vi "Old GUI.vi"() -> (0 "Error Out":errorcluster)   [LabVIEW 2019]
doc: "04/01/2021 Cobra Single Head GUI v1.0 \n\nModule Core. This is the main VI for a new module. This module is self contained in that it can run on it's own without any other top level VIs. Alternatively you can call this VI from a top level VI and use it as an actor. By default the front panel will open.\n\nThe module will initialize itself with a default set of values. You can use the Initialize.VI to change those settings. \n\nIf you would like to use the Rendezvous for syncronization call \"Initialize Rendezvous\". Just pass your rendezvous reference into it."
uses:
  GUI.lvlib
  <vilib>/nisyscfg/nisyscfg.lvlib
  9c9f3542-fc6c-43b1-9b30-f65ac35759b3.vi
  Private Controls/Config Data.ctl
  894b418a-eb83-4c03-97c2-0273c02a970a.vi
  Private Controls/Profile Sequence.ctl
  Private Controls/WebDAV states.ctl
  Private Controls/Messaging Actions.ctl
  <resource>/objmgr/ni.dex.rc
  Private Controls/Timer Mode.ctl
  Private Controls/Module Graphs.ctl
  Private Controls/System Graphs.ctl
  <vilib>/Analysis/NI_AALBase.lvlib
  Private Controls/Dial Gauges.ctl
  <vilib>/regexp/Match Regular Expression.xnode
  Private Controls/NSV States.ctl
  Private Controls/Gauge Graphs/Current.ctl
  Private Controls/Gauge Graphs/Superheat.ctl
  Private Controls/Gauge Graphs/Subcooling.ctl
  Private Controls/Gauge Graphs/Compression Ratio.ctl
  Private Controls/Save Log State.ctl
  f9a46cd7-08d2-4a24-acc7-4cd81866ad12.vi
  Private Controls/System Status.ctl
  4a2a642d-dd71-4e25-967e-5de2f7f56389.vi
  f258c684-4f8c-4311-ae87-074b09a61bd4.vi
  3f6ab150-a0d6-495f-8518-fb864465b894.vi
  <vilib>/Analysis/baseanly.llb/Mean (DBL).vi
  Private Controls/Event.ctl
  <vilib>/WebDAVClient/NI_WebDAV.lvlib
  Private Controls/NS New Data.ctl
  <vilib>/NI/STM/SubVIs/MetaDataElement.ctl
  <vilib>/NI/STM/NI STM.lvlib
  <vilib>/NI/STM/TCP/TCP Connection Info.ctl
  Private Controls/Network Data Down_set back.ctl
  Private Controls/Module Status.ctl
  Private Controls/M2 Status.ctl
  Private Controls/Dataset.ctl
  Private Controls/GUI Variables.ctl
panel:
  in  "Only Installable Systems (F)":bool
  in  "Detect Online Systems (T)":bool=TRUE
  out "M1 AC Load V":dbl
  in  "Include Cached Results (all)":u32(ring) caption="Include Cached Results" items=["none"=0, "only if online"=1, "all"=3]
  in  "Device Class":string
  in  "Session in (localhost)":refnum<k21>="localhost"
  in  "IP Override":bool
  out "AI (V)":dbl[](array[numeric])=[150.19890135042343, 151.86605864041528, 0.9899910143543054, 0.13460744672906727, 0.0, 0.0, 0.0, 0.0, 0.0, 0.0, 5.0, 5.0, 1625.0, 0.0, 0.0, 0.0, 0.0, 0.0, 0.0, 0.0, 0.0, 0.0, 0.0, 0.0, 0.0, 0.0, 0.0, 0.0, 0.0]
  in  "Manual IP":string
  out "Stack light states":T1(ring) caption="Stack Light States"
  in  "error in":errorcluster
  in  "Email Test":bool
  out "Feedback 2":u8(ring)=1 caption="PV Feedback" items=["Evap Temp", "Case Temp", "Intec Temp", "TSD  Temp", "Autotune", "Extra"]
  in  "Refresh Button":bool
  out "Network Connection":bool=TRUE
  in  "Menu Ring":u16(ring)=2 items=["192.168.1.10 (NI-sbRIO-9651-01e6940c)", "192.168.1.10 (NI-sbRIO-9651-01e69419)", "192.168.1.201 (Small-Conduit)", "192.168.1.57 (QC-Test)", "192.168.2.8 (DualCobra108)", "192.168.2.95 (ATE-220V-AIN)"]
  out "Compressor":bool
  out "Force(lbf)":dbl=50.0 format="%4.1f"
  out "Package":string="new_chip"
  out "Case Temp":dbl=22.890625 format="%4.1f"
  out "Set Temp":dbl=24.0 format="%4.0f"
  out "data out":T2={"Condensing Pressure"=150.19890135042343, "Suction Pressure"=151.86605864041528, "Bypass steps"=0, "Operating Time"=0.0, "SubCooling"=-3.2655841445138947, "Superheat"=2.2056690828700596, "M1 Superheat"=1.7837896333833214, "M2 Superheat"=-39.78496036661667, "Autotune output"=0.0, "M1 Testing Elapsed Time"=0.0, "M2 Testing Elapsed Time"=0.0, "M1 Valve Control Mode"=0, "System Amps"=0.13460744672906727, "Compressor Run Time"=0.0, "SD card free Space"=31885.0, "Free Memory"=0.0, "M1 Pressure Feedback"=0.0, "M2 Pressure Feedback"=0.0, "Compression Ratio"=0.9899910143543054, "Serial Number"=0.0, "M1 AC Load V"=0.0, "M1 AC Load W"=0.0, "M1 DC Load W"=0.0, "M1 RH"=-26.085277267486106, "RH Threshold"=100.0}
  out "Stop NSV":bool=TRUE
  in  "Tab Control":T3(tab)=enum."Debug"
  in  "M1 Power Drive":bool=TRUE
  in  "Power On-Off":bool
  out "Play/Pause":bool
  out "AC Load":dbl(graph)
  out "M1 Channels":dbl[](array[numeric])=[24.0, 23.120361328125, 22.899678548177082, nan, 0.0] format="%4.1f"
  in  "Thermal Diode Feedback":bool
  out "Main Chart":waveform(dbl)[](graph)=[{"t0"=timestamp(3699375123.743896 s since 1904-01-01), "dt"=1.0, "Y"=[25.0, 25.0, 25.0, 25.0, 25.0, 25.0, 25.0, 25.0, 25.0, 25.0, 25.0, 25.0, 25.0, 25.0, 25.0, 25.0, 25.0, 25.0, 25.0, 25.0, 25.0, 25.0, 25.0, 25.0, 25.0, 25.0, 25.0, 25.0, 25.0, 25.0, 25.0, 25.0, 25.0, 25.0, 25.0, 25.0, 25.0, 25.0, 25.0, 25.0, 25.0, 25.0, 25.0, 25.0, 25.0, 25.0, 25.0, 25.0, 25.0, 25.0, 25.0, 25.0, 25.0, 25.0, 25.0, 25.0, 25.0, 25.0, 25.0, 25.0, 25.0, 25.0, 25.0, 25.0, 25.0, 25.0, 25.0, 25.0, 25.0, 25.0, 25.0, 25.0, 25.0, 25.0, 25.0, 25.0, 25.0, 25.0, 25.0, 25.0, 25.0, 25.0, 25.0, 25.0, 25.0, 25.0, 25.0, 25.0, 25.0, 25.0, 25.0, 25.0, 25.0, 25.0, 25.0, 25.0, 25.0, 25.0, 25.0, 25.0, 25.0, 25.0, 25.0, 25.0, 25.0, 25.0, 25.0, 25.0, 25.0, 25.0, 25.0, 25.0, 25.0, 25.0, 25.0, 25.0, 25.0, 25.0, 25.0, 25.0, 25.0, 25.0, 25.0, 25.0, 25.0, 25.0, 25.0, 25.0, 25.0, 25.0, 25.0, 25.0, 25.0, 25.0, 25.0, 25.0, 25.0, 25.0, 25.0, 25.0, 25.0, 25.0, 25.0, 24.0, 24.0, 24.0, 24.0, 24.0, 24.0, 24.0, 24.0, 24.0, 24.0, 24.0, 24.0, 24.0, 24.0, 24.0, 24.0, 24.0, 24.0, 24.0, 24.0, 24.0, 24.0, 24.0, 24.0, 24.0, 24.0, 24.0, 24.0, 24.0, 24.0, 24.0, 24.0, 24.0, 24.0, 24.0, 24.0, 24.0, 24.0, 24.0, 24.0, 24.0, 24.0, 24.0, 24.0, 24.0, 24.0, 24.0, 24.0, 24.0, 24.0, 24.0, 24.0, 24.0, 24.0, 24.0, 24.0, 24.0, 24.0, 24.0, 24.0, 24.0, 24.0, 24.0, 24.0, 24.0, 24.0, 24.0, 24.0, 24.0, 24.0, 24.0, 24.0, 24.0, 24.0, 24.0, 24.0, 24.0, 24.0, 24.0, 24.0, 24.0, 24.0, 24.0, 24.0, 24.0, 24.0, 24.0, 24.0, 24.0, 24.0, 24.0, 24.0, 24.0, 24.0, 24.0, 24.0, 24.0, 24.0, 24.0, 24.0, 24.0, 24.0, 24.0, 24.0, 24.0, 24.0, 24.0, 24.0, 24.0, 24.0, 24.0, 24.0, 24.0, 24.0, 24.0, 24.0, 24.0, 24.0, 24.0, 24.0, 24.0, 24.0, 24.0, 24.0, 24.0, 24.0, 24.0, 24.0, 24.0, 24.0, 24.0, 24.0, 24.0, 24.0, 24.0, 24.0, 24.0, 24.0, 24.0, 24.0, 24.0, 24.0, 24.0, 24.0, 24.0, 24.0, 24.0, 24.0, 24.0, 24.0, 24.0, 24.0, 24.0, 24.0, 24.0, 24.0, 24.0, 24.0, 24.0, 24.0, 24.0, 24.0, 24.0, 24.0, 24.0, 24.0, 24.0, 24.0, 24.0, 24.0, 24.0, 24.0, 24.0, 24.0, 24.0, 24.0, 24.0, 24.0, 24.0, 24.0, 24.0, 24.0, 24.0, 24.0, 24.0, 24.0, 24.0, 24.0, 24.0, 24.0, 24.0, 24.0, 24.0, 24.0, 24.0, 24.0, 24.0, 24.0, 24.0, 24.0, 24.0, 24.0, 24.0, 24.0, 24.0, 24.0, 24.0, 24.0, 24.0, 24.0, 24.0, 24.0, 24.0, 24.0, 24.0, 24.0, 24.0, 24.0, 24.0, 24.0, 24.0, 24.0, 24.0, 24.0, 24.0, 24.0, 24.0, 24.0, 24.0, 24.0, 24.0, 24.0, 24.0, 24.0, 24.0, 24.0, 24.0, 24.0, 24.0, 24.0, 24.0]}, {"t0"=timestamp(3699375123.743896 s since 1904-01-01), "dt"=1.0, "Y"=array[384 elements]}, {"t0"=timestamp(3699375123.743896 s since 1904-01-01), "dt"=1.0, "Y"=array[384 elements]}, {"t0"=timestamp(3699375123.743896 s since 1904-01-01), "dt"=1.0, "Y"=[nan, nan, nan, nan, nan, nan, nan, nan, nan, nan, nan, nan, nan, nan, nan, nan, nan, nan, nan, nan, nan, nan, nan, nan, nan, nan, nan, nan, nan, nan, nan, nan, nan, nan, nan, nan, nan, nan, nan, nan, nan, nan, nan, nan, nan, nan, nan, nan, nan, nan, nan, nan, nan, nan, nan, nan, nan, nan, nan, nan, nan, nan, nan, nan, nan, nan, nan, nan, nan, nan, nan, nan, nan, nan, nan, nan, nan, nan, nan, nan, nan, nan, nan, nan, nan, nan, nan, nan, nan, nan, nan, nan, nan, nan, nan, nan, nan, nan, nan, nan, nan, nan, nan, nan, nan, nan, nan, nan, nan, nan, nan, nan, nan, nan, nan, nan, nan, nan, nan, nan, nan, nan, nan, nan, nan, nan, nan, nan, nan, nan, nan, nan, nan, nan, nan, nan, nan, nan, nan, nan, nan, nan, nan, nan, nan, nan, nan, nan, nan, nan, nan, nan, nan, nan, nan, nan, nan, nan, nan, nan, nan, nan, nan, nan, nan, nan, nan, nan, nan, nan, nan, nan, nan, nan, nan, nan, nan, nan, nan, nan, nan, nan, nan, nan, nan, nan, nan, nan, nan, nan, nan, nan, nan, nan, nan, nan, nan, nan, nan, nan, nan, nan, nan, nan, nan, nan, nan, nan, nan, nan, nan, nan, nan, nan, nan, nan, nan, nan, nan, nan, nan, nan, nan, nan, nan, nan, nan, nan, nan, nan, nan, nan, nan, nan, nan, nan, nan, nan, nan, nan, nan, nan, nan, nan, nan, nan, nan, nan, nan, nan, nan, nan, nan, nan, nan, nan, nan, nan, nan, nan, nan, nan, nan, nan, nan, nan, nan, nan, nan, nan, nan, nan, nan, nan, nan, nan, nan, nan, nan, nan, nan, nan, nan, nan, nan, nan, nan, nan, nan, nan, nan, nan, nan, nan, nan, nan, nan, nan, nan, nan, nan, nan, nan, nan, nan, nan, nan, nan, nan, nan, nan, nan, nan, nan, nan, nan, nan, nan, nan, nan, nan, nan, nan, nan, nan, nan, nan, nan, nan, nan, nan, nan, nan, nan, nan, nan, nan, nan, nan, nan, nan, nan, nan, nan, nan, nan, nan, nan, nan, nan, nan, nan, nan, nan, nan, nan, nan, nan, nan, nan, nan, nan, nan, nan, nan, nan, nan, nan, nan, nan, nan, nan, nan, nan, nan, nan, nan, nan, nan, nan, nan, nan, nan, nan]}, {"t0"=timestamp(3699375123.743896 s since 1904-01-01), "dt"=1.0, "Y"=[0.0, 0.0, 0.0, 0.0, 0.0, 0.0, 0.0, 0.0, 0.0, 0.0, 0.0, 0.0, 0.0, 0.0, 0.0, 0.0, 0.0, 0.0, 0.0, 0.0, 0.0, 0.0, 0.0, 0.0, 0.0, 0.0, 0.0, 0.0, 0.0, 0.0, 0.0, 0.0, 0.0, 0.0, 0.0, 0.0, 0.0, 0.0, 0.0, 0.0, 0.0, 0.0, 0.0, 0.0, 0.0, 0.0, 0.0, 0.0, 0.0, 0.0, 0.0, 0.0, 0.0, 0.0, 0.0, 0.0, 0.0, 0.0, 0.0, 0.0, 0.0, 0.0, 0.0, 0.0, 0.0, 0.0, 0.0, 0.0, 0.0, 0.0, 0.0, 0.0, 0.0, 0.0, 0.0, 0.0, 0.0, 0.0, 0.0, 0.0, 0.0, 0.0, 0.0, 0.0, 0.0, 0.0, 0.0, 0.0, 0.0, 0.0, 0.0, 0.0, 0.0, 0.0, 0.0, 0.0, 0.0, 0.0, 0.0, 0.0, 0.0, 0.0, 0.0, 0.0, 0.0, 0.0, 0.0, 0.0, 0.0, 0.0, 0.0, 0.0, 0.0, 0.0, 0.0, 0.0, 0.0, 0.0, 0.0, 0.0, 0.0, 0.0, 0.0, 0.0, 0.0, 0.0, 0.0, 0.0, 0.0, 0.0, 0.0, 0.0, 0.0, 0.0, 0.0, 0.0, 0.0, 0.0, 0.0, 0.0, 0.0, 0.0, 0.0, 0.0, 0.0, 0.0, 0.0, 0.0, 0.0, 0.0, 0.0, 0.0, 0.0, 0.0, 0.0, 0.0, 0.0, 0.0, 0.0, 0.0, 0.0, 0.0, 0.0, 0.0, 0.0, 0.0, 0.0, 0.0, 0.0, 0.0, 0.0, 0.0, 0.0, 0.0, 0.0, 0.0, 0.0, 0.0, 0.0, 0.0, 0.0, 0.0, 0.0, 0.0, 0.0, 0.0, 0.0, 0.0, 0.0, 0.0, 0.0, 0.0, 0.0, 0.0, 0.0, 0.0, 0.0, 0.0, 0.0, 0.0, 0.0, 0.0, 0.0, 0.0, 0.0, 0.0, 0.0, 0.0, 0.0, 0.0, 0.0, 0.0, 0.0, 0.0, 0.0, 0.0, 0.0, 0.0, 0.0, 0.0, 0.0, 0.0, 0.0, 0.0, 0.0, 0.0, 0.0, 0.0, 0.0, 0.0, 0.0, 0.0, 0.0, 0.0, 0.0, 0.0, 0.0, 0.0, 0.0, 0.0, 0.0, 0.0, 0.0, 0.0, 0.0, 0.0, 0.0, 0.0, 0.0, 0.0, 0.0, 0.0, 0.0, 0.0, 0.0, 0.0, 0.0, 0.0, 0.0, 0.0, 0.0, 0.0, 0.0, 0.0, 0.0, 0.0, 0.0, 0.0, 0.0, 0.0, 0.0, 0.0, 0.0, 0.0, 0.0, 0.0, 0.0, 0.0, 0.0, 0.0, 0.0, 0.0, 0.0, 0.0, 0.0, 0.0, 0.0, 0.0, 0.0, 0.0, 0.0, 0.0, 0.0, 0.0, 0.0, 0.0, 0.0, 0.0, 0.0, 0.0, 0.0, 0.0, 0.0, 0.0, 0.0, 0.0, 0.0, 0.0, 0.0, 0.0, 0.0, 0.0, 0.0, 0.0, 0.0, 0.0, 0.0, 0.0, 0.0, 0.0, 0.0, 0.0, 0.0, 0.0, 0.0, 0.0, 0.0, 0.0, 0.0, 0.0, 0.0, 0.0, 0.0, 0.0, 0.0, 0.0, 0.0, 0.0, 0.0, 0.0, 0.0, 0.0, 0.0, 0.0, 0.0, 0.0, 0.0, 0.0, 0.0, 0.0, 0.0, 0.0, 0.0, 0.0, 0.0, 0.0, 0.0, 0.0, 0.0, 0.0, 0.0, 0.0, 0.0, 0.0, 0.0, 0.0, 0.0, 0.0, 0.0, 0.0, 0.0, 0.0, 0.0, 0.0, 0.0, 0.0, 0.0, 0.0, 0.0, 0.0, 0.0, 0.0, 0.0, 0.0]}]
  out "WAITING TO REACH SAFE TEMP":bool
  out "PowerDrive":bool
  out "THERMAL HEAD  DISABLED":bool
  out "Bin String":string
  out "M1 Status":T4={"Case Temp"=22.890625, "Evap Temp"=0.0, "Heater %"=0.0, "EEV Steps"=0, "Set Temp"=24.0, "Feedback"=1, "Power Drive"=FALSE, "Piston Volts"=0.0, "Safe Temp"=FALSE, "Power"=FALSE, "Thermal State"=enum."Ramp Up", "Error"=FALSE, "In tollerance"=FALSE, "Head State"=enum."Disabled", "Piston Force"=0.0, "Package"=""} {"Piston Force" format="%#_1f"; "Feedback" items=["Evap Temp", "Case Temp"]; "Case Temp" format="%4.1f"}
  in  "M1 Commands":T5={"M1 Feedback"=1, "M1 Package"=0, "M1 Enable"=FALSE, "M1 Set Temp"=0.0} {"M1 Set Temp" min=-50.0 max=150.0 step=5.0; "M1 Package" items=["new_chip", "AI_chip", "CPU", "GPU", "300", "350", "", "", "", ""]; "M1 Feedback" items=["Evap Temp", "Case Temp", "Intec", "TSD"]}
  out "M1 Humidity":cluster{"M1 RH":dbl, "RH Threshold":dbl}(graph)
  out "Low Side RPM":dbl
  out "High Side RPM":dbl
  out "Thermal State":T6(ring)=enum."Steady State"
  out "System Graphs":T7={"Ambient Temp"=73.76562942564487, "Suction Temp"=73.93437944352627, "Condensor Temp"=74.25781697779894, "Discharge Temp"=75.15781707316637, "Bypass Steps"=72.0}
  out "M1 Temp Graphs":T8={"Case Temp"=22.890625, "Evap Temp"=23.1640625, "Heater Power (%)"=0.0, "EEV Steps"=3.0, "M1 AC Load(W)"=nan} caption="Temp Graphs"
  out "Gauges":T9={"Condensing Pressure(psi)"=150.28798352025635, "Compression Ratio"=0.9904730236494418, "Subcool"=-3.12361344029253, "Superheat"=2.1933731658321847, "Current(A)"=0.13316212224759566, "Suction Pressure(psi)"=151.87493902494265} {"Suction Pressure(psi)" scale=0.0..100.0; "Current(A)" scale=5.0..15.0 scale format="%_1f"; "Superheat" scale=0.0..100.0; "Subcool" scale=-10.0..20.0 scale format="%#4.1f"; "Compression Ratio" scale=0.0..30.0 scale format="%#.0f"; "Condensing Pressure(psi)" scale=150.0..375.0}
  in  "Login":bool
  out "Serial number":dbl
  in  "Config Data Setting":bool
  in  "Packages Setting":bool
  out "Errors":string[](array[string])=["WARN:Low Amps  (21 02 20 18 55)"]
  in  "Email recipeints":string[](array[string])
  in  "Output (Hostname and IP)":u32(ring)=33 items=["Hostname"=16, "Hostname (IP)"=18, "Hostname (MAC)"=19, "IP"=32, "IP (Hostname)"=33, "IP (MAC)"=35, "MAC"=48, "MAC (Hostname)"=49, "MAC (IP)"=50]
  out "Most Recent Error":string
  out "Event log":T14(array[cluster])=[{"Name"="M1 Setpoint Change", "Time Stamp"=timestamp(3697404441.246959 s since 1904-01-01), "Code"="", "Source"="APP:Send Set Temp", "Value"=24.0, "Boolean"=FALSE, "String"="", "Error"=FALSE, "Warning"=TRUE, " Fault"=FALSE}, {"Name"="M1 Set Point", "Time Stamp"=timestamp(3697404441.212613 s since 1904-01-01), "Code"="", "Source"="GUI Event", "Value"=24.0, "Boolean"=FALSE, "String"="", "Error"=FALSE, "Warning"=FALSE, " Fault"=FALSE}, {"Name"="M1 Setpoint Change", "Time Stamp"=timestamp(3697404407.626065 s since 1904-01-01), "Code"="", "Source"="APP:Send Set Temp", "Value"=25.0, "Boolean"=FALSE, "String"="", "Error"=FALSE, "Warning"=TRUE, " Fault"=FALSE}, {"Name"="M1 Set Point", "Time Stamp"=timestamp(3697404407.582319 s since 1904-01-01), "Code"="", "Source"="GUI Event", "Value"=25.0, "Boolean"=FALSE, "String"="", "Error"=FALSE, "Warning"=FALSE, " Fault"=FALSE}, {"Name"="M1 Setpoint Change", "Time Stamp"=timestamp(3697404402.799341 s since 1904-01-01), "Code"="", "Source"="APP:Send Set Temp", "Value"=2.0, "Boolean"=FALSE, "String"="", "Error"=FALSE, "Warning"=TRUE, " Fault"=FALSE}, {"Name"="M1 Set Point", "Time Stamp"=timestamp(3697404402.767277 s since 1904-01-01), "Code"="", "Source"="GUI Event", "Value"=2.0, "Boolean"=FALSE, "String"="", "Error"=FALSE, "Warning"=FALSE, " Fault"=FALSE}, {"Name"="M1 Setpoint Change", "Time Stamp"=timestamp(3697404393.95497 s since 1904-01-01), "Code"="", "Source"="APP:Send Set Temp", "Value"=24.0, "Boolean"=FALSE, "String"="", "Error"=FALSE, "Warning"=TRUE, " Fault"=FALSE}, {"Name"="M1 Set Point", "Time Stamp"=timestamp(3697404393.921568 s since 1904-01-01), "Code"="", "Source"="GUI Event", "Value"=24.0, "Boolean"=FALSE, "String"="", "Error"=FALSE, "Warning"=FALSE, " Fault"=FALSE}, {"Name"="M1 Set Point", "Time Stamp"=timestamp(3697317947.208045 s since 1904-01-01), "Code"="", "Source"="GUI Event", "Value"=0.0, "Boolean"=FALSE, "String"="", "Error"=FALSE, "Warning"=FALSE, " Fault"=FALSE}, {"Name"="M1 Set Point", "Time Stamp"=timestamp(3697317941.377172 s since 1904-01-01), "Code"="", "Source"="GUI Event", "Value"=0.0, "Boolean"=FALSE, "String"="", "Error"=FALSE, "Warning"=FALSE, " Fault"=FALSE}, {"Name"="Bypass Target Change", "Time Stamp"=timestamp(3696722909.311575 s since 1904-01-01), "Code"="", "Source"="Bypass:Get Target", "Value"=110.0, "Boolean"=FALSE, "String"="", "Error"=FALSE, "Warning"=FALSE, " Fault"=FALSE}, {"Name"="PID Bypassed", "Time Stamp"=timestamp(3696722908.895819 s since 1904-01-01), "Code"="", "Source"="APP:Set/Send PID Bypass", "Value"=0.0, "Boolean"=FALSE, "String"="", "Error"=FALSE, "Warning"=FALSE, " Fault"=FALSE}, {"Name"="Read Saved State", "Time Stamp"=timestamp(3696722908.522525 s since 1904-01-01), "Code"="", "Source"="", "Value"=0.0, "Boolean"=FALSE, "String"="", "Error"=FALSE, "Warning"=FALSE, " Fault"=FALSE}, {"Name"="System Power", "Time Stamp"=timestamp(3696722907.909232 s since 1904-01-01), "Code"="", "Source"="GUI Event", "Value"=nan, "Boolean"=FALSE, "String"="", "Error"=FALSE, "Warning"=FALSE, " Fault"=FALSE}, {"Name"="M1 Setpoint Change", "Time Stamp"=timestamp(3696722840.115096 s since 1904-01-01), "Code"="", "Source"="APP:Send Set Temp", "Value"=25.0, "Boolean"=FALSE, "String"="", "Error"=FALSE, "Warning"=TRUE, " Fault"=FALSE}, {"Name"="M1 Set Point", "Time Stamp"=timestamp(3696722840.083527 s since 1904-01-01), "Code"="", "Source"="GUI Event", "Value"=25.0, "Boolean"=FALSE, "String"="", "Error"=FALSE, "Warning"=FALSE, " Fault"=FALSE}, {"Name"="EEV PID Output", "Time Stamp"=timestamp(3696722832.497274 s since 1904-01-01), "Code"="", "Source"="APP:Send EEV PID Out", "Value"=0.0, "Boolean"=FALSE, "String"="Value Change", "Error"=FALSE, "Warning"=FALSE, " Fault"=FALSE}, {"Name"="EEV PID Output", "Time Stamp"=timestamp(3696722545.942951 s since 1904-01-01), "Code"="", "Source"="APP:Send EEV PID Out", "Value"=20.0, "Boolean"=FALSE, "String"="Value Change", "Error"=FALSE, "Warning"=FALSE, " Fault"=FALSE}, {"Name"="EEV PID Output", "Time Stamp"=timestamp(3696722279.730517 s since 1904-01-01), "Code"="", "Source"="APP:Send EEV PID Out", "Value"=0.0, "Boolean"=FALSE, "String"="Value Change", "Error"=FALSE, "Warning"=FALSE, " Fault"=FALSE}, {"Name"="EEV PID Output", "Time Stamp"=timestamp(3696722270.596302 s since 1904-01-01), "Code"="", "Source"="APP:Send EEV PID Out", "Value"=20.0, "Boolean"=FALSE, "String"="Value Change", "Error"=FALSE, "Warning"=FALSE, " Fault"=FALSE}, {"Name"="EEV PID Output", "Time Stamp"=timestamp(3696722184.927274 s since 1904-01-01), "Code"="", "Source"="APP:Send EEV PID Out", "Value"=0.0, "Boolean"=FALSE, "String"="Value Change", "Error"=FALSE, "Warning"=FALSE, " Fault"=FALSE}, {"Name"="EEV PID Output", "Time Stamp"=timestamp(3696722168.565057 s since 1904-01-01), "Code"="", "Source"="APP:Send EEV PID Out", "Value"=20.0, "Boolean"=FALSE, "String"="Value Change", "Error"=FALSE, "Warning"=FALSE, " Fault"=FALSE}, {"Name"="M1 Setpoint Change", "Time Stamp"=timestamp(3696721334.993426 s since 1904-01-01), "Code"="", "Source"="APP:Send Set Temp", "Value"=0.0, "Boolean"=FALSE, "String"="", "Error"=FALSE, "Warning"=TRUE, " Fault"=FALSE}, {"Name"="M1 Set Point", "Time Stamp"=timestamp(3696721334.958938 s since 1904-01-01), "Code"="", "Source"="GUI Event", "Value"=0.0, "Boolean"=FALSE, "String"="", "Error"=FALSE, "Warning"=FALSE, " Fault"=FALSE}, {"Name"="", "Time Stamp"=timestamp(3696721234.772972 s since 1904-01-01), "Code"="", "Source"="MACRO:Piston Down", "Value"=0.0, "Boolean"=FALSE, "String"="", "Error"=FALSE, "Warning"=FALSE, " Fault"=FALSE}, {"Name"="M1 Power Drive", "Time Stamp"=timestamp(3696721234.729546 s since 1904-01-01), "Code"="", "Source"="GUI Event", "Value"=nan, "Boolean"=TRUE, "String"="", "Error"=FALSE, "Warning"=FALSE, " Fault"=FALSE}, {"Name"="", "Time Stamp"=timestamp(3696721230.831664 s since 1904-01-01), "Code"="", "Source"="MACRO:Piston Up", "Value"=0.0, "Boolean"=FALSE, "String"="", "Error"=FALSE, "Warning"=FALSE, " Fault"=FALSE}, {"Name"="M1 Power Drive", "Time Stamp"=timestamp(3696721230.225435 s since 1904-01-01), "Code"="", "Source"="GUI Event", "Value"=nan, "Boolean"=FALSE, "String"="", "Error"=FALSE, "Warning"=FALSE, " Fault"=FALSE}, {"Name"="", "Time Stamp"=timestamp(3696721223.856889 s since 1904-01-01), "Code"="", "Source"="MACRO:Piston Down", "Value"=0.0, "Boolean"=FALSE, "String"="", "Error"=FALSE, "Warning"=FALSE, " Fault"=FALSE}, {"Name"="M1 Power Drive", "Time Stamp"=timestamp(3696721223.821096 s since 1904-01-01), "Code"="", "Source"="GUI Event", "Value"=nan, "Boolean"=TRUE, "String"="", "Error"=FALSE, "Warning"=FALSE, " Fault"=FALSE}, {"Name"="EEV PID Output", "Time Stamp"=timestamp(3696721076.771943 s since 1904-01-01), "Code"="", "Source"="APP:Send EEV PID Out", "Value"=0.0, "Boolean"=FALSE, "String"="Value Change", "Error"=FALSE, "Warning"=FALSE, " Fault"=FALSE}, {"Name"="WARN:Low Amps", "Time Stamp"=timestamp(3696720959.402056 s since 1904-01-01), "Code"="", "Source"="", "Value"=1.0015844, "Boolean"=FALSE, "String"="", "Error"=TRUE, "Warning"=TRUE, " Fault"=FALSE}, {"Name"="Bypass Reset", "Time Stamp"=timestamp(3696720957.49231 s since 1904-01-01), "Code"="", "Source"="Bypass:Reset Bypass", "Value"=0.0, "Boolean"=FALSE, "String"="", "Error"=FALSE, "Warning"=FALSE, " Fault"=FALSE}, {"Name"="Bypass Reset", "Time Stamp"=timestamp(3696720956.315602 s since 1904-01-01), "Code"="", "Source"="Bypass:Reset Bypass", "Value"=0.0, "Boolean"=TRUE, "String"="", "Error"=FALSE, "Warning"=FALSE, " Fault"=FALSE}, {"Name"="Bypass PID Gains Change", "Time Stamp"=timestamp(3696720956.263541 s since 1904-01-01), "Code"="", "Source"="Bypass:Get Gains", "Value"=0.0, "Boolean"=FALSE, "String"="", "Error"=FALSE, "Warning"=FALSE, " Fault"=FALSE}, {"Name"="Bypass Target Change", "Time Stamp"=timestamp(3696720956.211851 s since 1904-01-01), "Code"="", "Source"="Bypass:Get Target", "Value"=3.0, "Boolean"=FALSE, "String"="", "Error"=FALSE, "Warning"=FALSE, " Fault"=FALSE}, {"Name"="Send EEV PID Target", "Time Stamp"=timestamp(3696720955.840866 s since 1904-01-01), "Code"="", "Source"="APP:Send EEV PID Target", "Value"=50.0, "Boolean"=FALSE, "String"="", "Error"=FALSE, "Warning"=FALSE, " Fault"=FALSE}, {"Name"="EEV Target Change", "Time Stamp"=timestamp(3696720955.797327 s since 1904-01-01), "Code"="", "Source"="APP:Get EEV PID Target", "Value"=50.0, "Boolean"=FALSE, "String"="", "Error"=FALSE, "Warning"=FALSE, " Fault"=FALSE}, {"Name"="EEV PID Output", "Time Stamp"=timestamp(3696720955.738594 s since 1904-01-01), "Code"="", "Source"="APP:Send EEV PID Out", "Value"=20.0, "Boolean"=FALSE, "String"="Value Change", "Error"=FALSE, "Warning"=FALSE, " Fault"=FALSE}, {"Name"="PID Bypassed", "Time Stamp"=timestamp(3696720955.567045 s since 1904-01-01), "Code"="", "Source"="APP:Set/Send PID Bypass", "Value"=0.0, "Boolean"=FALSE, "String"="", "Error"=FALSE, "Warning"=FALSE, " Fault"=FALSE}, {"Name"="Create New Datalog File", "Time Stamp"=timestamp(3696720954.995124 s since 1904-01-01), "Code"="", "Source"="", "Value"=0.0, "Boolean"=FALSE, "String"="", "Error"=FALSE, "Warning"=FALSE, " Fault"=FALSE}, {"Name"="Read Saved State", "Time Stamp"=timestamp(3696720954.777131 s since 1904-01-01), "Code"="", "Source"="", "Value"=0.0, "Boolean"=FALSE, "String"="", "Error"=FALSE, "Warning"=FALSE, " Fault"=FALSE}, {"Name"="Compressor Enable", "Time Stamp"=timestamp(3696720954.737832 s since 1904-01-01), "Code"="", "Source"="Save State", "Value"=0.0, "Boolean"=TRUE, "String"="System Settings", "Error"=FALSE, "Warning"=FALSE, " Fault"=FALSE}, {"Name"="System Power", "Time Stamp"=timestamp(3696720953.433398 s since 1904-01-01), "Code"="", "Source"="GUI Event", "Value"=nan, "Boolean"=TRUE, "String"="", "Error"=FALSE, "Warning"=FALSE, " Fault"=FALSE}, {"Name"="Bypass Target Change", "Time Stamp"=timestamp(3696720910.985179 s since 1904-01-01), "Code"="", "Source"="Bypass:Get Target", "Value"=110.0, "Boolean"=FALSE, "String"="", "Error"=FALSE, "Warning"=FALSE, " Fault"=FALSE}, {"Name"="Mains Frequency", "Time Stamp"=timestamp(3696720910.167106 s since 1904-01-01), "Code"="", "Source"="Init System Module", "Value"=221.59026785399922, "Boolean"=FALSE, "String"="", "Error"=FALSE, "Warning"=FALSE, " Fault"=FALSE}, {"Name"="Fan Amps", "Time Stamp"=timestamp(3696720910.135427 s since 1904-01-01), "Code"="", "Source"="Init System Module", "Value"=0.13293173783945855, "Boolean"=FALSE, "String"="", "Error"=FALSE, "Warning"=FALSE, " Fault"=FALSE}, {"Name"="PID Bypassed", "Time Stamp"=timestamp(3696720904.619165 s since 1904-01-01), "Code"="", "Source"="APP:Set/Send PID Bypass", "Value"=0.0, "Boolean"=FALSE, "String"="", "Error"=FALSE, "Warning"=FALSE, " Fault"=FALSE}, {"Name"="Thermal Status Change", "Time Stamp"=timestamp(3696720904.526545 s since 1904-01-01), "Code"="", "Source"="APP:Thermal Status", "Value"=0.0, "Boolean"=FALSE, "String"="", "Error"=FALSE, "Warning"=FALSE, " Fault"=FALSE}, {"Name"="M1 Setpoint Change", "Time Stamp"=timestamp(3696720904.307311 s since 1904-01-01), "Code"="", "Source"="APP:Send Set Temp", "Value"=25.0, "Boolean"=FALSE, "String"="", "Error"=FALSE, "Warning"=TRUE, " Fault"=FALSE}, {"Name"="M1 EEV Check Position", "Time Stamp"=timestamp(3696720904.25734 s since 1904-01-01), "Code"="", "Source"="", "Value"=0.0, "Boolean"=TRUE, "String"="Complete", "Error"=FALSE, "Warning"=FALSE, " Fault"=FALSE}, {"Name"="Bypass Inintialize", "Time Stamp"=timestamp(3696720903.612567 s since 1904-01-01), "Code"="", "Source"="", "Value"=4506.0, "Boolean"=FALSE, "String"="Complete", "Error"=FALSE, "Warning"=FALSE, " Fault"=FALSE}, {"Name"="Config Loaded", "Time Stamp"=timestamp(3696720894.173367 s since 1904-01-01), "Code"="", "Source"="Config Read Initialize", "Value"=0.0, "Boolean"=FALSE, "String"="", "Error"=FALSE, "Warning"=FALSE, " Fault"=FALSE}, {"Name"="Config Read", "Time Stamp"=timestamp(3696720894.13737 s since 1904-01-01), "Code"="Found", "Source"="M2 TSD", "Value"=0.0, "Boolean"=FALSE, "String"="V Offset", "Error"=FALSE, "Warning"=FALSE, " Fault"=FALSE}, {"Name"="Config Read", "Time Stamp"=timestamp(3696720894.101301 s since 1904-01-01), "Code"="Found", "Source"="M2 TSD", "Value"=0.0, "Boolean"=FALSE, "String"="Offset", "Error"=FALSE, "Warning"=FALSE, " Fault"=FALSE}, {"Name"="Config Read", "Time Stamp"=timestamp(3696720894.069511 s since 1904-01-01), "Code"="Found", "Source"="M2 TSD", "Value"=1.0, "Boolean"=FALSE, "String"="Gain", "Error"=FALSE, "Warning"=FALSE, " Fault"=FALSE}, {"Name"="Config Read", "Time Stamp"=timestamp(3696720894.035389 s since 1904-01-01), "Code"="Found", "Source"="M1 TSD", "Value"=0.0, "Boolean"=FALSE, "String"="V Offset", "Error"=FALSE, "Warning"=FALSE, " Fault"=FALSE}, {"Name"="Config Read", "Time Stamp"=timestamp(3696720894.004982 s since 1904-01-01), "Code"="Found", "Source"="M1 TSD", "Value"=0.0, "Boolean"=FALSE, "String"="Offset", "Error"=FALSE, "Warning"=FALSE, " Fault"=FALSE}, {"Name"="Config Read", "Time Stamp"=timestamp(3696720893.957789 s since 1904-01-01), "Code"="Found", "Source"="M1 TSD", "Value"=1.0, "Boolean"=FALSE, "String"="Gain", "Error"=FALSE, "Warning"=FALSE, " Fault"=FALSE}, {"Name"="M1 EEV Check Position", "Time Stamp"=timestamp(3696720893.92009 s since 1904-01-01), "Code"="", "Source"="EEV:Check Position", "Value"=0.0, "Boolean"=FALSE, "String"="", "Error"=FALSE, "Warning"=FALSE, " Fault"=FALSE}, {"Name"="Config Read", "Time Stamp"=timestamp(3696720893.889076 s since 1904-01-01), "Code"="Found", "Source"="M2 T-Case Calibration", "Value"=0.0, "Boolean"=FALSE, "String"="Offset", "Error"=FALSE, "Warning"=FALSE, " Fault"=FALSE}, {"Name"="EEV PID Output", "Time Stamp"=timestamp(3696720893.86316 s since 1904-01-01), "Code"="", "Source"="APP:Send EEV PID Out", "Value"=0.0, "Boolean"=FALSE, "String"="Value Change", "Error"=FALSE, "Warning"=FALSE, " Fault"=FALSE}, {"Name"="Config Read", "Time Stamp"=timestamp(3696720893.831275 s since 1904-01-01), "Code"="Found", "Source"="M2 T-Case Calibration", "Value"=1.0, "Boolean"=FALSE, "String"="Gain", "Error"=FALSE, "Warning"=FALSE, " Fault"=FALSE}, {"Name"="", "Time Stamp"=timestamp(3696720893.797286 s since 1904-01-01), "Code"="", "Source"="EEV:Set Position", "Value"=0.0, "Boolean"=FALSE, "String"="", "Error"=FALSE, "Warning"=FALSE, " Fault"=FALSE}, {"Name"="Config Read", "Time Stamp"=timestamp(3696720893.767191 s since 1904-01-01), "Code"="Found", "Source"="M1 T-Case Calibration", "Value"=0.0, "Boolean"=FALSE, "String"="Offset", "Error"=FALSE, "Warning"=FALSE, " Fault"=FALSE}, {"Name"="", "Time Stamp"=timestamp(3696720893.717819 s since 1904-01-01), "Code"="", "Source"="EEV:Config", "Value"=0.0, "Boolean"=FALSE, "String"="", "Error"=FALSE, "Warning"=FALSE, " Fault"=FALSE}, {"Name"="Config Read", "Time Stamp"=timestamp(3696720893.68612 s since 1904-01-01), "Code"="Found", "Source"="M1 T-Case Calibration", "Value"=1.0, "Boolean"=FALSE, "String"="Gain", "Error"=FALSE, "Warning"=FALSE, " Fault"=FALSE}, {"Name"="Config Read", "Time Stamp"=timestamp(3696720893.653343 s since 1904-01-01), "Code"="Found", "Source"="Heater PID TSD", "Value"=0.066, "Boolean"=FALSE, "String"="Derivative Value", "Error"=FALSE, "Warning"=FALSE, " Fault"=FALSE}, {"Name"="Config Read", "Time Stamp"=timestamp(3696720893.619191 s since 1904-01-01), "Code"="Found", "Source"="Heater PID TSD", "Value"=0.264, "Boolean"=FALSE, "String"="Integral Value", "Error"=FALSE, "Warning"=FALSE, " Fault"=FALSE}, {"Name"="Config Read", "Time Stamp"=timestamp(3696720893.587827 s since 1904-01-01), "Code"="Found", "Source"="Heater PID TSD", "Value"=4.207, "Boolean"=FALSE, "String"="Proportional Value", "Error"=FALSE, "Warning"=FALSE, " Fault"=FALSE}, {"Name"="Config Read", "Time Stamp"=timestamp(3696720893.561761 s since 1904-01-01), "Code"="Found", "Source"="M2 EEV PID", "Value"=0.0, "Boolean"=FALSE, "String"="Gain D", "Error"=FALSE, "Warning"=FALSE, " Fault"=FALSE}, {"Name"="Config Read", "Time Stamp"=timestamp(3696720893.533947 s since 1904-01-01), "Code"="Found", "Source"="M2 EEV PID", "Value"=0.25, "Boolean"=FALSE, "String"="Gain I", "Error"=FALSE, "Warning"=FALSE, " Fault"=FALSE}, {"Name"="Config Read", "Time Stamp"=timestamp(3696720893.499744 s since 1904-01-01), "Code"="Found", "Source"="M2 EEV PID", "Value"=-1.0, "Boolean"=FALSE, "String"="Gain P", "Error"=FALSE, "Warning"=FALSE, " Fault"=FALSE}, {"Name"="Config Read", "Time Stamp"=timestamp(3696720893.453109 s since 1904-01-01), "Code"="Found", "Source"="EEV PID", "Value"=15.0, "Boolean"=FALSE, "String"="M1 Superheat Setpoint ", "Error"=FALSE, "Warning"=FALSE, " Fault"=FALSE}, {"Name"="Config Read", "Time Stamp"=timestamp(3696720893.407586 s since 1904-01-01), "Code"="Found", "Source"="EEV PID", "Value"=0.0, "Boolean"=FALSE, "String"="Output Low", "Error"=FALSE, "Warning"=FALSE, " Fault"=FALSE}, {"Name"="Config Read", "Time Stamp"=timestamp(3696720893.375381 s since 1904-01-01), "Code"="Found", "Source"="EEV PID", "Value"=155.0, "Boolean"=FALSE, "String"="Output Hi", "Error"=FALSE, "Warning"=FALSE, " Fault"=FALSE}, {"Name"="Config Read", "Time Stamp"=timestamp(3696720893.345284 s since 1904-01-01), "Code"="Found", "Source"="EEV PID", "Value"=0.0, "Boolean"=FALSE, "String"="Gain D", "Error"=FALSE, "Warning"=FALSE, " Fault"=FALSE}, {"Name"="Config Read", "Time Stamp"=timestamp(3696720893.313855 s since 1904-01-01), "Code"="Found", "Source"="EEV PID", "Value"=0.6, "Boolean"=FALSE, "String"="Gain I", "Error"=FALSE, "Warning"=FALSE, " Fault"=FALSE}, {"Name"="Config Read", "Time Stamp"=timestamp(3696720893.282199 s since 1904-01-01), "Code"="Found", "Source"="EEV PID", "Value"=-1.0, "Boolean"=FALSE, "String"="Gain P", "Error"=FALSE, "Warning"=FALSE, " Fault"=FALSE}, {"Name"="Config Read", "Time Stamp"=timestamp(3696720893.253151 s since 1904-01-01), "Code"="Found", "Source"="EEV PID", "Value"=10.0, "Boolean"=FALSE, "String"="Dissabled Target", "Error"=FALSE, "Warning"=FALSE, " Fault"=FALSE}, {"Name"="Config Read", "Time Stamp"=timestamp(3696720893.203999 s since 1904-01-01), "Code"="Found", "Source"="EEV PID", "Value"=30.0, "Boolean"=FALSE, "String"="SS Steps", "Error"=FALSE, "Warning"=FALSE, " Fault"=FALSE}, {"Name"="Config Read", "Time Stamp"=timestamp(3696720893.175068 s since 1904-01-01), "Code"="Found", "Source"="EEV PID", "Value"=60.0, "Boolean"=FALSE, "String"="RD Steps", "Error"=FALSE, "Warning"=FALSE, " Fault"=FALSE}, {"Name"="Config Read", "Time Stamp"=timestamp(3696720893.143394 s since 1904-01-01), "Code"="Found", "Source"="EEV PID", "Value"=20.0, "Boolean"=FALSE, "String"="RU Steps", "Error"=FALSE, "Warning"=FALSE, " Fault"=FALSE}, {"Name"="Config Read", "Time Stamp"=timestamp(3696720893.112236 s since 1904-01-01), "Code"="Found", "Source"="EEV PID", "Value"=85.0, "Boolean"=FALSE, "String"="EBB Steps Closed", "Error"=FALSE, "Warning"=FALSE, " Fault"=FALSE}, {"Name"="Config Read", "Time Stamp"=timestamp(3696720893.081919 s since 1904-01-01), "Code"="Found", "Source"="EEV PID", "Value"=70.0, "Boolean"=FALSE, "String"="EBB Steps Open", "Error"=FALSE, "Warning"=FALSE, " Fault"=FALSE}, {"Name"="Config Read", "Time Stamp"=timestamp(3696720893.055853 s since 1904-01-01), "Code"="Found", "Source"="EEV PID", "Value"=2.0, "Boolean"=FALSE, "String"="EBB Tol", "Error"=FALSE, "Warning"=FALSE, " Fault"=FALSE}, {"Name"="Config Read", "Time Stamp"=timestamp(3696720893.027455 s since 1904-01-01), "Code"="Found", "Source"="EEV PID", "Value"=-60.0, "Boolean"=FALSE, "String"="EBB TH", "Error"=FALSE, "Warning"=FALSE, " Fault"=FALSE}, {"Name"="Config Read", "Time Stamp"=timestamp(3696720892.999011 s since 1904-01-01), "Code"="Found", "Source"="EEV PID", "Value"=50.0, "Boolean"=FALSE, "String"="SS Target", "Error"=FALSE, "Warning"=FALSE, " Fault"=FALSE}, {"Name"="Config Read", "Time Stamp"=timestamp(3696720892.955559 s since 1904-01-01), "Code"="Found", "Source"="EEV PID", "Value"=50.0, "Boolean"=FALSE, "String"="RD Target", "Error"=FALSE, "Warning"=FALSE, " Fault"=FALSE}, {"Name"="Config Read", "Time Stamp"=timestamp(3696720892.927444 s since 1904-01-01), "Code"="Found", "Source"="EEV PID", "Value"=50.0, "Boolean"=FALSE, "String"="RU Target", "Error"=FALSE, "Warning"=FALSE, " Fault"=FALSE}, {"Name"="Config Read", "Time Stamp"=timestamp(3696720892.898945 s since 1904-01-01), "Code"="Found", "Source"="Temp TH", "Value"=3.0, "Boolean"=FALSE, "String"="SS Tol", "Error"=FALSE, "Warning"=FALSE, " Fault"=FALSE}, {"Name"="Config Read", "Time Stamp"=timestamp(3696720892.865717 s since 1904-01-01), "Code"="Found", "Source"="Temp TH", "Value"=10.0, "Boolean"=FALSE, "String"="Ramp-SS Delta T", "Error"=FALSE, "Warning"=FALSE, " Fault"=FALSE}, {"Name"="Config Read", "Time Stamp"=timestamp(3696720892.839071 s since 1904-01-01), "Code"="Found", "Source"="Temp TH", "Value"=10.0, "Boolean"=FALSE, "String"="Ramp Delta T", "Error"=FALSE, "Warning"=FALSE, " Fault"=FALSE}, {"Name"="Config Read", "Time Stamp"=timestamp(3696720892.80532 s since 1904-01-01), "Code"="Found", "Source"="Temp TH", "Value"=75.0, "Boolean"=FALSE, "String"="Pedestal Delta T", "Error"=FALSE, "Warning"=FALSE, " Fault"=FALSE}, {"Name"="Config Read", "Time Stamp"=timestamp(3696720892.777417 s since 1904-01-01), "Code"="Found", "Source"="Set Point Range", "Value"=-50.0, "Boolean"=FALSE, "String"="Min", "Error"=FALSE, "Warning"=FALSE, " Fault"=FALSE}, {"Name"="Config Read", "Time Stamp"=timestamp(3696720892.75149 s since 1904-01-01), "Code"="Found", "Source"="Set Point Range", "Value"=150.0, "Boolean"=FALSE, "String"="Max", "Error"=FALSE, "Warning"=FALSE, " Fault"=FALSE}, {"Name"="Config Read", "Time Stamp"=timestamp(3696720892.705211 s since 1904-01-01), "Code"="Found", "Source"="CryoMode PID Gains", "Value"=0.0, "Boolean"=FALSE, "String"="Derivative Value", "Error"=FALSE, "Warning"=FALSE, " Fault"=FALSE}, {"Name"="Config Read", "Time Stamp"=timestamp(3696720892.676571 s since 1904-01-01), "Code"="Found", "Source"="CryoMode PID Gains", "Value"=0.5, "Boolean"=FALSE, "String"="Integral Value", "Error"=FALSE, "Warning"=FALSE, " Fault"=FALSE}, {"Name"="Config Read", "Time Stamp"=timestamp(3696720892.651484 s since 1904-01-01), "Code"="Found", "Source"="CryoMode PID Gains", "Value"=-1.0, "Boolean"=FALSE, "String"="Proportional Value", "Error"=FALSE, "Warning"=FALSE, " Fault"=FALSE}, {"Name"="Config Read", "Time Stamp"=timestamp(3696720892.623679 s since 1904-01-01), "Code"="Found", "Source"="M2 Heater PID", "Value"=0.0, "Boolean"=FALSE, "String"="Derivative Value", "Error"=FALSE, "Warning"=FALSE, " Fault"=FALSE}, {"Name"="Config Read", "Time Stamp"=timestamp(3696720892.593471 s since 1904-01-01), "Code"="Found", "Source"="M2 Heater PID", "Value"=0.2, "Boolean"=FALSE, "String"="Integral Value", "Error"=FALSE, "Warning"=FALSE, " Fault"=FALSE}, {"Name"="Config Read", "Time Stamp"=timestamp(3696720892.559162 s since 1904-01-01), "Code"="Found", "Source"="M2 Heater PID", "Value"=8.0, "Boolean"=FALSE, "String"="Proportional Value", "Error"=FALSE, "Warning"=FALSE, " Fault"=FALSE}, {"Name"="Config Read", "Time Stamp"=timestamp(3696720892.53134 s since 1904-01-01), "Code"="Found", "Source"="Heater PID", "Value"=0.066, "Boolean"=FALSE, "String"="Derivative Value", "Error"=FALSE, "Warning"=FALSE, " Fault"=FALSE}, {"Name"="Config Read", "Time Stamp"=timestamp(3696720892.502409 s since 1904-01-01), "Code"="Found", "Source"="Heater PID", "Value"=0.264, "Boolean"=FALSE, "String"="Integral Value", "Error"=FALSE, "Warning"=FALSE, " Fault"=FALSE}, {"Name"="Config Read", "Time Stamp"=timestamp(3696720892.465166 s since 1904-01-01), "Code"="Found", "Source"="Heater PID", "Value"=2.207, "Boolean"=FALSE, "String"="Proportional Value", "Error"=FALSE, "Warning"=FALSE, " Fault"=FALSE}, {"Name"="Config Read", "Time Stamp"=timestamp(3696720892.433118 s since 1904-01-01), "Code"="Found", "Source"="Piston Settings", "Value"=500.0, "Boolean"=FALSE, "String"="Pressure Ramp Delay (ms)", "Error"=FALSE, "Warning"=FALSE, " Fault"=FALSE}, {"Name"="Config Read", "Time Stamp"=timestamp(3696720892.393472 s since 1904-01-01), "Code"="Found", "Source"="Piston Settings", "Value"=5000.0, "Boolean"=FALSE, "String"="Delay (ms)", "Error"=FALSE, "Warning"=FALSE, " Fault"=FALSE}, {"Name"="Config Read", "Time Stamp"=timestamp(3696720892.364299 s since 1904-01-01), "Code"="Found", "Source"="Piston Settings", "Value"=51.0, "Boolean"=FALSE, "String"="Piston Diameter (mm)", "Error"=FALSE, "Warning"=FALSE, " Fault"=FALSE}, {"Name"="Config Read", "Time Stamp"=timestamp(3696720892.337039 s since 1904-01-01), "Code"="Found", "Source"="Piston Settings", "Value"=0.4, "Boolean"=FALSE, "String"="Up Force", "Error"=FALSE, "Warning"=FALSE, " Fault"=FALSE}, {"Name"="Config Read", "Time Stamp"=timestamp(3696720892.309436 s since 1904-01-01), "Code"="Found", "Source"="Piston Settings", "Value"=0.4, "Boolean"=FALSE, "String"="Transition Force", "Error"=FALSE, "Warning"=FALSE, " Fault"=FALSE}, {"Name"="Config Read", "Time Stamp"=timestamp(3696720892.282026 s since 1904-01-01), "Code"="Found", "Source"="Piston Settings", "Value"=0.1488, "Boolean"=FALSE, "String"="Forces Intercept", "Error"=FALSE, "Warning"=FALSE, " Fault"=FALSE}, {"Name"="Config Read", "Time Stamp"=timestamp(3696720892.254328 s since 1904-01-01), "Code"="Found", "Source"="Piston Settings", "Value"=0.0127, "Boolean"=FALSE, "String"="Forces Slope", "Error"=FALSE, "Warning"=FALSE, " Fault"=FALSE}, {"Name"="Config Read", "Time Stamp"=timestamp(3696720892.208177 s since 1904-01-01), "Code"="Found", "Source"="Bypass PID", "Value"=0.0, "Boolean"=FALSE, "String"="Derivative Value", "Error"=FALSE, "Warning"=FALSE, " Fault"=FALSE}, {"Name"="Config Read", "Time Stamp"=timestamp(3696720892.181363 s since 1904-01-01), "Code"="Found", "Source"="Bypass PID", "Value"=0.8, "Boolean"=FALSE, "String"="Integral Value", "Error"=FALSE, "Warning"=FALSE, " Fault"=FALSE}, {"Name"="Config Read", "Time Stamp"=timestamp(3696720892.154298 s since 1904-01-01), "Code"="Found", "Source"="Bypass PID", "Value"=1.5, "Boolean"=FALSE, "String"="Proportional Value", "Error"=FALSE, "Warning"=FALSE, " Fault"=FALSE}, {"Name"="Config Value Read", "Time Stamp"=timestamp(3696720892.12076 s since 1904-01-01), "Code"="", "Source"="", "Value"=0.0, "Boolean"=TRUE, "String"="Cascade", "Error"=FALSE, "Warning"=FALSE, " Fault"=FALSE}, {"Name"="Config Value Read", "Time Stamp"=timestamp(3696720892.098045 s since 1904-01-01), "Code"="", "Source"="", "Value"=0.0, "Boolean"=TRUE, "String"="220V", "Error"=FALSE, "Warning"=FALSE, " Fault"=FALSE}, {"Name"="M1 EEV Check Position", "Time Stamp"=timestamp(3696720892.075967 s since 1904-01-01), "Code"="", "Source"="", "Value"=0.0, "Boolean"=TRUE, "String"="Complete", "Error"=FALSE, "Warning"=FALSE, " Fault"=FALSE}, {"Name"="Config Value Read", "Time Stamp"=timestamp(3696720892.053395 s since 1904-01-01), "Code"="", "Source"="", "Value"=0.0, "Boolean"=TRUE, "String"="Shuttle", "Error"=FALSE, "Warning"=FALSE, " Fault"=FALSE}, {"Name"="Config Value Read", "Time Stamp"=timestamp(3696720892.032653 s since 1904-01-01), "Code"="", "Source"="", "Value"=0.0, "Boolean"=TRUE, "String"="Handler", "Error"=FALSE, "Warning"=FALSE, " Fault"=FALSE}, {"Name"="Config Value Read", "Time Stamp"=timestamp(3696720892.012066 s since 1904-01-01), "Code"="", "Source"="", "Value"=0.0, "Boolean"=TRUE, "String"="Production", "Error"=FALSE, "Warning"=FALSE, " Fault"=FALSE}, {"Name"="Config Value Read", "Time Stamp"=timestamp(3696720891.98133 s since 1904-01-01), "Code"="", "Source"="", "Value"=0.0, "Boolean"=TRUE, "String"="Benchtop", "Error"=FALSE, "Warning"=FALSE, " Fault"=FALSE}, {"Name"="Config Value Read", "Time Stamp"=timestamp(3696720891.933658 s since 1904-01-01), "Code"="", "Source"="", "Value"=0.0, "Boolean"=TRUE, "String"="ATE", "Error"=FALSE, "Warning"=FALSE, " Fault"=FALSE}, {"Name"="Config Value Read", "Time Stamp"=timestamp(3696720891.891371 s since 1904-01-01), "Code"="", "Source"="", "Value"=0.0, "Boolean"=TRUE, "String"="HandClamp", "Error"=FALSE, "Warning"=FALSE, " Fault"=FALSE}, {"Name"="Config Value Read", "Time Stamp"=timestamp(3696720891.860102 s since 1904-01-01), "Code"="", "Source"="", "Value"=0.0, "Boolean"=TRUE, "String"="Sensors", "Error"=FALSE, "Warning"=FALSE, " Fault"=FALSE}, {"Name"="Config Value Read", "Time Stamp"=timestamp(3696720891.828709 s since 1904-01-01), "Code"="", "Source"="", "Value"=0.0, "Boolean"=TRUE, "String"="Purge", "Error"=FALSE, "Warning"=FALSE, " Fault"=FALSE}, {"Name"="Config Value Read", "Time Stamp"=timestamp(3696720891.791521 s since 1904-01-01), "Code"="", "Source"="", "Value"=0.0, "Boolean"=TRUE, "String"="Autostartup", "Error"=FALSE, "Warning"=FALSE, " Fault"=FALSE}, {"Name"="Config Value Read", "Time Stamp"=timestamp(3696720891.764417 s since 1904-01-01), "Code"="", "Source"="", "Value"=0.0, "Boolean"=TRUE, "String"="FTC200", "Error"=FALSE, "Warning"=FALSE, " Fault"=FALSE}, {"Name"="M1 EEV Check Position", "Time Stamp"=timestamp(3696720891.738071 s since 1904-01-01), "Code"="", "Source"="EEV:Check Position", "Value"=0.0, "Boolean"=FALSE, "String"="", "Error"=FALSE, "Warning"=FALSE, " Fault"=FALSE}, {"Name"="Config Value Read", "Time Stamp"=timestamp(3696720891.704925 s since 1904-01-01), "Code"="", "Source"="", "Value"=0.0, "Boolean"=TRUE, "String"="60Hz Power", "Error"=FALSE, "Warning"=FALSE, " Fault"=FALSE}, {"Name"="EEV PID Output", "Time Stamp"=timestamp(3696720891.667846 s since 1904-01-01), "Code"="", "Source"="APP:Send EEV PID Out", "Value"=2000.0, "Boolean"=FALSE, "String"="Value Change", "Error"=FALSE, "Warning"=FALSE, " Fault"=FALSE}, {"Name"="", "Time Stamp"=timestamp(3696720891.638331 s since 1904-01-01), "Code"="", "Source"="EEV:Set Position", "Value"=0.0, "Boolean"=TRUE, "String"="", "Error"=FALSE, "Warning"=FALSE, " Fault"=FALSE}, {"Name"="EEV:Set V", "Time Stamp"=timestamp(3696720891.590639 s since 1904-01-01), "Code"="", "Source"="", "Value"=0.0, "Boolean"=FALSE, "String"="", "Error"=FALSE, "Warning"=FALSE, " Fault"=FALSE}, {"Name"="New Extra Settings Loaded", "Time Stamp"=timestamp(3696720891.568061 s since 1904-01-01), "Code"="", "Source"="", "Value"=0.0, "Boolean"=FALSE, "String"="", "Error"=FALSE, "Warning"=FALSE, " Fault"=FALSE}, {"Name"="", "Time Stamp"=timestamp(3696720891.534483 s since 1904-01-01), "Code"="", "Source"="EEV:Config", "Value"=0.0, "Boolean"=FALSE, "String"="", "Error"=FALSE, "Warning"=FALSE, " Fault"=FALSE}, {"Name"="EMO Not Detected", "Time Stamp"=timestamp(3696720891.500666 s since 1904-01-01), "Code"="", "Source"="", "Value"=0.0, "Boolean"=FALSE, "String"="", "Error"=FALSE, "Warning"=FALSE, " Fault"=FALSE}, {"Name"="Read Compressor Minutes", "Time Stamp"=timestamp(3696720891.434006 s since 1904-01-01), "Code"="", "Source"="", "Value"=2930.0, "Boolean"=TRUE, "String"="PASS", "Error"=FALSE, "Warning"=FALSE, " Fault"=FALSE}, {"Name"="High Pressure Switch Detected", "Time Stamp"=timestamp(3696720891.405424 s since 1904-01-01), "Code"="", "Source"="SYS:Initialize", "Value"=0.0, "Boolean"=TRUE, "String"="", "Error"=FALSE, "Warning"=FALSE, " Fault"=FALSE}, {"Name"="Odometer Loaded", "Time Stamp"=timestamp(3696720891.303544 s since 1904-01-01), "Code"="", "Source"="", "Value"=0.0, "Boolean"=FALSE, "String"="", "Error"=FALSE, "Warning"=FALSE, " Fault"=FALSE}, {"Name"="Read Saved State", "Time Stamp"=timestamp(3696720891.269036 s since 1904-01-01), "Code"="", "Source"="", "Value"=0.0, "Boolean"=FALSE, "String"="", "Error"=FALSE, "Warning"=FALSE, " Fault"=FALSE}, {"Name"="FPGA Load Complete", "Time Stamp"=timestamp(3696720891.241224 s since 1904-01-01), "Code"="", "Source"="Init FPGA IO.vi", "Value"=0.0, "Boolean"=FALSE, "String"="", "Error"=FALSE, "Warning"=FALSE, " Fault"=FALSE}, {"Name"="Pressure Test", "Time Stamp"=timestamp(3696720889.221135 s since 1904-01-01), "Code"="", "Source"="Init FPGA IO 2.0.vi", "Value"=0.0, "Boolean"=FALSE, "String"="FAIL", "Error"=FALSE, "Warning"=TRUE, " Fault"=FALSE}, {"Name"="Stop LCD", "Time Stamp"=timestamp(3696720883.988151 s since 1904-01-01), "Code"="", "Source"="Init FPGA IO.vi", "Value"=11.0, "Boolean"=FALSE, "String"="", "Error"=FALSE, "Warning"=FALSE, " Fault"=FALSE}, {"Name"="wait", "Time Stamp"=timestamp(3696720882.969395 s since 1904-01-01), "Code"="", "Source"="Init FPGA IO.vi", "Value"=10.0, "Boolean"=FALSE, "String"="", "Error"=FALSE, "Warning"=FALSE, " Fault"=FALSE}, {"Name"="IP Address", "Time Stamp"=timestamp(3696720881.931437 s since 1904-01-01), "Code"="", "Source"="Init FPGA IO.vi", "Value"=12.0, "Boolean"=FALSE, "String"="þQ", "Error"=FALSE, "Warning"=FALSE, " Fault"=FALSE}, {"Name"="wait", "Time Stamp"=timestamp(3696720880.464476 s since 1904-01-01), "Code"="", "Source"="Init FPGA IO.vi", "Value"=10.0, "Boolean"=FALSE, "String"="", "Error"=FALSE, "Warning"=FALSE, " Fault"=FALSE}, {"Name"="Rev Display", "Time Stamp"=timestamp(3696720879.446471 s since 1904-01-01), "Code"="", "Source"="Init FPGA IO.vi", "Value"=9.0, "Boolean"=FALSE, "String"="Ver: CC 21.2.18.0", "Error"=FALSE, "Warning"=FALSE, " Fault"=FALSE}, {"Name"="wait", "Time Stamp"=timestamp(3696720879.359947 s since 1904-01-01), "Code"="", "Source"="Init FPGA IO.vi", "Value"=10.0, "Boolean"=FALSE, "String"="", "Error"=FALSE, "Warning"=FALSE, " Fault"=FALSE}, {"Name"="Chroma Display", "Time Stamp"=timestamp(3696720878.342291 s since 1904-01-01), "Code"="", "Source"="Init FPGA IO.vi", "Value"=8.0, "Boolean"=FALSE, "String"="Chroma ATE", "Error"=FALSE, "Warning"=FALSE, " Fault"=FALSE}, {"Name"="wait", "Time Stamp"=timestamp(3696720878.2478 s since 1904-01-01), "Code"="", "Source"="Init FPGA IO.vi", "Value"=10.0, "Boolean"=FALSE, "String"="", "Error"=FALSE, "Warning"=FALSE, " Fault"=FALSE}, {"Name"="Clear LCD Text", "Time Stamp"=timestamp(3696720877.219357 s since 1904-01-01), "Code"="", "Source"="Init FPGA IO.vi", "Value"=0.0, "Boolean"=FALSE, "String"="", "Error"=FALSE, "Warning"=FALSE, " Fault"=FALSE}, {"Name"="Mains Frequency", "Time Stamp"=timestamp(3696720877.149534 s since 1904-01-01), "Code"="", "Source"="Init FPGA", "Value"=194.7629520614688, "Boolean"=FALSE, "String"="", "Error"=FALSE, "Warning"=FALSE, " Fault"=FALSE}, {"Name"="Fan Amps", "Time Stamp"=timestamp(3696720877.132159 s since 1904-01-01), "Code"="", "Source"="Init FPGA", "Value"=0.10758788061792209, "Boolean"=FALSE, "String"="", "Error"=FALSE, "Warning"=FALSE, " Fault"=FALSE}, {"Name"="BootLoad", "Time Stamp"=timestamp(3696720866.1065 s since 1904-01-01), "Code"="", "Source"="Init FPGA IO.vi", "Value"=0.0, "Boolean"=FALSE, "String"="", "Error"=FALSE, "Warning"=FALSE, " Fault"=FALSE}, {"Name"="Extra Settings Loaded", "Time Stamp"=timestamp(3696720865.294767 s since 1904-01-01), "Code"="", "Source"="", "Value"=0.0, "Boolean"=FALSE, "String"="", "Error"=FALSE, "Warning"=FALSE, " Fault"=FALSE}, {"Name"="M1 Heater Specs", "Time Stamp"=timestamp(3696720865.276621 s since 1904-01-01), "Code"="", "Source"="Extra Settings", "Value"=0.0, "Boolean"=TRUE, "String"="", "Error"=FALSE, "Warning"=FALSE, " Fault"=FALSE}, {"Name"="Shuttle", "Time Stamp"=timestamp(3696720865.259777 s since 1904-01-01), "Code"="", "Source"="Extra Settings", "Value"=0.0, "Boolean"=TRUE, "String"="", "Error"=FALSE, "Warning"=FALSE, " Fault"=FALSE}, {"Name"="Housing Heater", "Time Stamp"=timestamp(3696720865.242604 s since 1904-01-01), "Code"="", "Source"="Extra Settings", "Value"=0.0, "Boolean"=TRUE, "String"="", "Error"=FALSE, "Warning"=FALSE, " Fault"=FALSE}, {"Name"="Warmup ", "Time Stamp"=timestamp(3696720865.225249 s since 1904-01-01), "Code"="", "Source"="Extra Settings", "Value"=0.0, "Boolean"=FALSE, "String"="", "Error"=FALSE, "Warning"=TRUE, " Fault"=FALSE}, {"Name"="Warmup ", "Time Stamp"=timestamp(3696720865.206102 s since 1904-01-01), "Code"="", "Source"="Extra Settings", "Value"=0.0, "Boolean"=FALSE, "String"="", "Error"=FALSE, "Warning"=TRUE, " Fault"=FALSE}, {"Name"="TSD ", "Time Stamp"=timestamp(3696720865.189469 s since 1904-01-01), "Code"="", "Source"="Extra Settings", "Value"=0.0, "Boolean"=FALSE, "String"="", "Error"=FALSE, "Warning"=FALSE, " Fault"=FALSE}, {"Name"="Flow Curve", "Time Stamp"=timestamp(3696720865.163189 s since 1904-01-01), "Code"="", "Source"="Extra Settings", "Value"=0.0, "Boolean"=FALSE, "String"="", "Error"=FALSE, "Warning"=TRUE, " Fault"=FALSE}, {"Name"="Heads Disabled", "Time Stamp"=timestamp(3696720865.145402 s since 1904-01-01), "Code"="", "Source"="Extra Settings", "Value"=0.0, "Boolean"=TRUE, "String"="", "Error"=FALSE, "Warning"=FALSE, " Fault"=FALSE}, {"Name"="Low Superheat", "Time Stamp"=timestamp(3696720865.128817 s since 1904-01-01), "Code"="", "Source"="Extra Settings", "Value"=0.0, "Boolean"=TRUE, "String"="", "Error"=FALSE, "Warning"=FALSE, " Fault"=FALSE}, {"Name"="High Superheat", "Time Stamp"=timestamp(3696720865.111942 s since 1904-01-01), "Code"="", "Source"="Extra Settings", "Value"=0.0, "Boolean"=TRUE, "String"="", "Error"=FALSE, "Warning"=FALSE, " Fault"=FALSE}, {"Name"="High Subcooling", "Time Stamp"=timestamp(3696720865.093904 s since 1904-01-01), "Code"="", "Source"="Extra Settings", "Value"=0.0, "Boolean"=TRUE, "String"="", "Error"=FALSE, "Warning"=FALSE, " Fault"=FALSE}, {"Name"="Low Subcooling", "Time Stamp"=timestamp(3696720865.077746 s since 1904-01-01), "Code"="", "Source"="Extra Settings", "Value"=0.0, "Boolean"=TRUE, "String"="", "Error"=FALSE, "Warning"=FALSE, " Fault"=FALSE}, {"Name"="Water Sensor", "Time Stamp"=timestamp(3696720865.061704 s since 1904-01-01), "Code"="", "Source"="Extra Settings", "Value"=0.0, "Boolean"=TRUE, "String"="", "Error"=FALSE, "Warning"=FALSE, " Fault"=FALSE}, {"Name"="Flow Sensor", "Time Stamp"=timestamp(3696720865.045559 s since 1904-01-01), "Code"="", "Source"="Extra Settings", "Value"=0.0, "Boolean"=TRUE, "String"="", "Error"=FALSE, "Warning"=FALSE, " Fault"=FALSE}, {"Name"="High Amperage", "Time Stamp"=timestamp(3696720865.029495 s since 1904-01-01), "Code"="", "Source"="Extra Settings", "Value"=0.0, "Boolean"=TRUE, "String"="", "Error"=FALSE, "Warning"=FALSE, " Fault"=FALSE}, {"Name"="Low Amperage", "Time Stamp"=timestamp(3696720865.013499 s since 1904-01-01), "Code"="", "Source"="Extra Settings", "Value"=0.0, "Boolean"=TRUE, "String"="", "Error"=FALSE, "Warning"=FALSE, " Fault"=FALSE}, {"Name"="Relative Humidity", "Time Stamp"=timestamp(3696720864.997521 s since 1904-01-01), "Code"="", "Source"="Extra Settings", "Value"=0.0, "Boolean"=TRUE, "String"="", "Error"=FALSE, "Warning"=FALSE, " Fault"=FALSE}, {"Name"="Warnings/Faults 1", "Time Stamp"=timestamp(3696720864.950962 s since 1904-01-01), "Code"="", "Source"="Extra Settings 3", "Value"=0.0, "Boolean"=TRUE, "String"="", "Error"=FALSE, "Warning"=FALSE, " Fault"=FALSE}, {"Name"="SuperHeat Settings", "Time Stamp"=timestamp(3696720864.933577 s since 1904-01-01), "Code"="", "Source"="Extra Settings 3", "Value"=0.0, "Boolean"=TRUE, "String"="", "Error"=FALSE, "Warning"=FALSE, " Fault"=FALSE}, {"Name"="Read System Settings", "Time Stamp"=timestamp(3696720864.914497 s since 1904-01-01), "Code"="", "Source"="Read Extra Settings", "Value"=0.0, "Boolean"=FALSE, "String"="", "Error"=FALSE, "Warning"=TRUE, " Fault"=FALSE}, {"Name"="Config Loaded", "Time Stamp"=timestamp(3696720864.86972 s since 1904-01-01), "Code"="", "Source"="Config Read Initialize", "Value"=0.0, "Boolean"=FALSE, "String"="", "Error"=FALSE, "Warning"=FALSE, " Fault"=FALSE}, {"Name"="Config Read", "Time Stamp"=timestamp(3696720864.85342 s since 1904-01-01), "Code"="Found", "Source"="M2 TSD", "Value"=0.0, "Boolean"=FALSE, "String"="V Offset", "Error"=FALSE, "Warning"=FALSE, " Fault"=FALSE}, {"Name"="Config Read", "Time Stamp"=timestamp(3696720864.837514 s since 1904-01-01), "Code"="Found", "Source"="M2 TSD", "Value"=0.0, "Boolean"=FALSE, "String"="Offset", "Error"=FALSE, "Warning"=FALSE, " Fault"=FALSE}, {"Name"="Config Read", "Time Stamp"=timestamp(3696720864.821681 s since 1904-01-01), "Code"="Found", "Source"="M2 TSD", "Value"=1.0, "Boolean"=FALSE, "String"="Gain", "Error"=FALSE, "Warning"=FALSE, " Fault"=FALSE}, {"Name"="Config Read", "Time Stamp"=timestamp(3696720864.804834 s since 1904-01-01), "Code"="Found", "Source"="M1 TSD", "Value"=0.0, "Boolean"=FALSE, "String"="V Offset", "Error"=FALSE, "Warning"=FALSE, " Fault"=FALSE}, {"Name"="Config Read", "Time Stamp"=timestamp(3696720864.789486 s since 1904-01-01), "Code"="Found", "Source"="M1 TSD", "Value"=0.0, "Boolean"=FALSE, "String"="Offset", "Error"=FALSE, "Warning"=FALSE, " Fault"=FALSE}, {"Name"="Config Read", "Time Stamp"=timestamp(3696720864.774412 s since 1904-01-01), "Code"="Found", "Source"="M1 TSD", "Value"=1.0, "Boolean"=FALSE, "String"="Gain", "Error"=FALSE, "Warning"=FALSE, " Fault"=FALSE}, {"Name"="Config Read", "Time Stamp"=timestamp(3696720864.759064 s since 1904-01-01), "Code"="Found", "Source"="M2 T-Case Calibration", "Value"=0.0, "Boolean"=FALSE, "String"="Offset", "Error"=FALSE, "Warning"=FALSE, " Fault"=FALSE}, {"Name"="Config Read", "Time Stamp"=timestamp(3696720864.74409 s since 1904-01-01), "Code"="Found", "Source"="M2 T-Case Calibration", "Value"=1.0, "Boolean"=FALSE, "String"="Gain", "Error"=FALSE, "Warning"=FALSE, " Fault"=FALSE}, {"Name"="Config Read", "Time Stamp"=timestamp(3696720864.729025 s since 1904-01-01), "Code"="Found", "Source"="M1 T-Case Calibration", "Value"=0.0, "Boolean"=FALSE, "String"="Offset", "Error"=FALSE, "Warning"=FALSE, " Fault"=FALSE}, {"Name"="Config Read", "Time Stamp"=timestamp(3696720864.714051 s since 1904-01-01), "Code"="Found", "Source"="M1 T-Case Calibration", "Value"=1.0, "Boolean"=FALSE, "String"="Gain", "Error"=FALSE, "Warning"=FALSE, " Fault"=FALSE}, {"Name"="Config Read", "Time Stamp"=timestamp(3696720864.699277 s since 1904-01-01), "Code"="Found", "Source"="Heater PID TSD", "Value"=0.066, "Boolean"=FALSE, "String"="Derivative Value", "Error"=FALSE, "Warning"=FALSE, " Fault"=FALSE}, {"Name"="Config Read", "Time Stamp"=timestamp(3696720864.683881 s since 1904-01-01), "Code"="Found", "Source"="Heater PID TSD", "Value"=0.264, "Boolean"=FALSE, "String"="Integral Value", "Error"=FALSE, "Warning"=FALSE, " Fault"=FALSE}, {"Name"="Config Read", "Time Stamp"=timestamp(3696720864.660618 s since 1904-01-01), "Code"="Found", "Source"="Heater PID TSD", "Value"=4.207, "Boolean"=FALSE, "String"="Proportional Value", "Error"=FALSE, "Warning"=FALSE, " Fault"=FALSE}, {"Name"="Config Read", "Time Stamp"=timestamp(3696720864.644996 s since 1904-01-01), "Code"="Found", "Source"="M2 EEV PID", "Value"=0.0, "Boolean"=FALSE, "String"="Gain D", "Error"=FALSE, "Warning"=FALSE, " Fault"=FALSE}, {"Name"="Config Read", "Time Stamp"=timestamp(3696720864.630353 s since 1904-01-01), "Code"="Found", "Source"="M2 EEV PID", "Value"=0.25, "Boolean"=FALSE, "String"="Gain I", "Error"=FALSE, "Warning"=FALSE, " Fault"=FALSE}, {"Name"="Config Read", "Time Stamp"=timestamp(3696720864.615385 s since 1904-01-01), "Code"="Found", "Source"="M2 EEV PID", "Value"=-1.0, "Boolean"=FALSE, "String"="Gain P", "Error"=FALSE, "Warning"=FALSE, " Fault"=FALSE}, {"Name"="Config Read", "Time Stamp"=timestamp(3696720864.600925 s since 1904-01-01), "Code"="Found", "Source"="EEV PID", "Value"=15.0, "Boolean"=FALSE, "String"="M1 Superheat Setpoint ", "Error"=FALSE, "Warning"=FALSE, " Fault"=FALSE}, {"Name"="Config Read", "Time Stamp"=timestamp(3696720864.572165 s since 1904-01-01), "Code"="Found", "Source"="EEV PID", "Value"=155.0, "Boolean"=FALSE, "String"="Output Hi", "Error"=FALSE, "Warning"=FALSE, " Fault"=FALSE}, {"Name"="Config Read", "Time Stamp"=timestamp(3696720864.557516 s since 1904-01-01), "Code"="Found", "Source"="EEV PID", "Value"=0.0, "Boolean"=FALSE, "String"="Gain D", "Error"=FALSE, "Warning"=FALSE, " Fault"=FALSE}, {"Name"="Config Read", "Time Stamp"=timestamp(3696720864.541891 s since 1904-01-01), "Code"="Found", "Source"="EEV PID", "Value"=0.6, "Boolean"=FALSE, "String"="Gain I", "Error"=FALSE, "Warning"=FALSE, " Fault"=FALSE}, {"Name"="Config Read", "Time Stamp"=timestamp(3696720864.517088 s since 1904-01-01), "Code"="Found", "Source"="EEV PID", "Value"=-1.0, "Boolean"=FALSE, "String"="Gain P", "Error"=FALSE, "Warning"=FALSE, " Fault"=FALSE}, {"Name"="Config Read", "Time Stamp"=timestamp(3696720864.502005 s since 1904-01-01), "Code"="Found", "Source"="EEV PID", "Value"=10.0, "Boolean"=FALSE, "String"="Dissabled Target", "Error"=FALSE, "Warning"=FALSE, " Fault"=FALSE}, {"Name"="Config Read", "Time Stamp"=timestamp(3696720864.486235 s since 1904-01-01), "Code"="Found", "Source"="EEV PID", "Value"=30.0, "Boolean"=FALSE, "String"="SS Steps", "Error"=FALSE, "Warning"=FALSE, " Fault"=FALSE}, {"Name"="Config Read", "Time Stamp"=timestamp(3696720864.470571 s since 1904-01-01), "Code"="Found", "Source"="EEV PID", "Value"=60.0, "Boolean"=FALSE, "String"="RD Steps", "Error"=FALSE, "Warning"=FALSE, " Fault"=FALSE}, {"Name"="Config Read", "Time Stamp"=timestamp(3696720864.454592 s since 1904-01-01), "Code"="Found", "Source"="EEV PID", "Value"=20.0, "Boolean"=FALSE, "String"="RU Steps", "Error"=FALSE, "Warning"=FALSE, " Fault"=FALSE}, {"Name"="Config Read", "Time Stamp"=timestamp(3696720864.438853 s since 1904-01-01), "Code"="Found", "Source"="EEV PID", "Value"=85.0, "Boolean"=FALSE, "String"="EBB Steps Closed", "Error"=FALSE, "Warning"=FALSE, " Fault"=FALSE}, {"Name"="Config Read", "Time Stamp"=timestamp(3696720864.423674 s since 1904-01-01), "Code"="Found", "Source"="EEV PID", "Value"=70.0, "Boolean"=FALSE, "String"="EBB Steps Open", "Error"=FALSE, "Warning"=FALSE, " Fault"=FALSE}, {"Name"="Config Read", "Time Stamp"=timestamp(3696720864.399453 s since 1904-01-01), "Code"="Found", "Source"="EEV PID", "Value"=2.0, "Boolean"=FALSE, "String"="EBB Tol", "Error"=FALSE, "Warning"=FALSE, " Fault"=FALSE}, {"Name"="Config Read", "Time Stamp"=timestamp(3696720864.379651 s since 1904-01-01), "Code"="Found", "Source"="EEV PID", "Value"=-60.0, "Boolean"=FALSE, "String"="EBB TH", "Error"=FALSE, "Warning"=FALSE, " Fault"=FALSE}, {"Name"="Config Read", "Time Stamp"=timestamp(3696720864.364313 s since 1904-01-01), "Code"="Found", "Source"="EEV PID", "Value"=50.0, "Boolean"=FALSE, "String"="SS Target", "Error"=FALSE, "Warning"=FALSE, " Fault"=FALSE}, {"Name"="Config Read", "Time Stamp"=timestamp(3696720864.339973 s since 1904-01-01), "Code"="Found", "Source"="EEV PID", "Value"=50.0, "Boolean"=FALSE, "String"="RD Target", "Error"=FALSE, "Warning"=FALSE, " Fault"=FALSE}, {"Name"="Config Read", "Time Stamp"=timestamp(3696720864.320472 s since 1904-01-01), "Code"="Found", "Source"="EEV PID", "Value"=50.0, "Boolean"=FALSE, "String"="RU Target", "Error"=FALSE, "Warning"=FALSE, " Fault"=FALSE}, {"Name"="Config Read", "Time Stamp"=timestamp(3696720864.299976 s since 1904-01-01), "Code"="Found", "Source"="Temp TH", "Value"=3.0, "Boolean"=FALSE, "String"="SS Tol", "Error"=FALSE, "Warning"=FALSE, " Fault"=FALSE}, {"Name"="Config Read", "Time Stamp"=timestamp(3696720864.274729 s since 1904-01-01), "Code"="Found", "Source"="Temp TH", "Value"=10.0, "Boolean"=FALSE, "String"="Ramp-SS Delta T", "Error"=FALSE, "Warning"=FALSE, " Fault"=FALSE}, {"Name"="Config Read", "Time Stamp"=timestamp(3696720864.259622 s since 1904-01-01), "Code"="Found", "Source"="Temp TH", "Value"=10.0, "Boolean"=FALSE, "String"="Ramp Delta T", "Error"=FALSE, "Warning"=FALSE, " Fault"=FALSE}, {"Name"="Config Read", "Time Stamp"=timestamp(3696720864.243791 s since 1904-01-01), "Code"="Found", "Source"="Temp TH", "Value"=75.0, "Boolean"=FALSE, "String"="Pedestal Delta T", "Error"=FALSE, "Warning"=FALSE, " Fault"=FALSE}, {"Name"="Config Read", "Time Stamp"=timestamp(3696720864.227674 s since 1904-01-01), "Code"="Found", "Source"="Set Point Range", "Value"=-50.0, "Boolean"=FALSE, "String"="Min", "Error"=FALSE, "Warning"=FALSE, " Fault"=FALSE}, {"Name"="Config Read", "Time Stamp"=timestamp(3696720864.211801 s since 1904-01-01), "Code"="Found", "Source"="Set Point Range", "Value"=150.0, "Boolean"=FALSE, "String"="Max", "Error"=FALSE, "Warning"=FALSE, " Fault"=FALSE}, {"Name"="Config Read", "Time Stamp"=timestamp(3696720864.196179 s since 1904-01-01), "Code"="Found", "Source"="CryoMode PID Gains", "Value"=0.0, "Boolean"=FALSE, "String"="Derivative Value", "Error"=FALSE, "Warning"=FALSE, " Fault"=FALSE}, {"Name"="Config Read", "Time Stamp"=timestamp(3696720864.161114 s since 1904-01-01), "Code"="Found", "Source"="CryoMode PID Gains", "Value"=0.5, "Boolean"=FALSE, "String"="Integral Value", "Error"=FALSE, "Warning"=FALSE, " Fault"=FALSE}, {"Name"="Config Read", "Time Stamp"=timestamp(3696720864.144419 s since 1904-01-01), "Code"="Found", "Source"="CryoMode PID Gains", "Value"=-1.0, "Boolean"=FALSE, "String"="Proportional Value", "Error"=FALSE, "Warning"=FALSE, " Fault"=FALSE}, {"Name"="Config Read", "Time Stamp"=timestamp(3696720864.115454 s since 1904-01-01), "Code"="Found", "Source"="M2 Heater PID", "Value"=0.2, "Boolean"=FALSE, "String"="Integral Value", "Error"=FALSE, "Warning"=FALSE, " Fault"=FALSE}, {"Name"="Config Read", "Time Stamp"=timestamp(3696720864.101321 s since 1904-01-01), "Code"="Found", "Source"="M2 Heater PID", "Value"=8.0, "Boolean"=FALSE, "String"="Proportional Value", "Error"=FALSE, "Warning"=FALSE, " Fault"=FALSE}, {"Name"="Config Read", "Time Stamp"=timestamp(3696720864.08568 s since 1904-01-01), "Code"="Found", "Source"="Heater PID", "Value"=0.066, "Boolean"=FALSE, "String"="Derivative Value", "Error"=FALSE, "Warning"=FALSE, " Fault"=FALSE}, {"Name"="Config Read", "Time Stamp"=timestamp(3696720864.070752 s since 1904-01-01), "Code"="Found", "Source"="Heater PID", "Value"=0.264, "Boolean"=FALSE, "String"="Integral Value", "Error"=FALSE, "Warning"=FALSE, " Fault"=FALSE}, {"Name"="Config Read", "Time Stamp"=timestamp(3696720864.053531 s since 1904-01-01), "Code"="Found", "Source"="Heater PID", "Value"=2.207, "Boolean"=FALSE, "String"="Proportional Value", "Error"=FALSE, "Warning"=FALSE, " Fault"=FALSE}, {"Name"="Config Read", "Time Stamp"=timestamp(3696720864.033635 s since 1904-01-01), "Code"="Found", "Source"="Piston Settings", "Value"=500.0, "Boolean"=FALSE, "String"="Pressure Ramp Delay (ms)", "Error"=FALSE, "Warning"=FALSE, " Fault"=FALSE}, {"Name"="Config Read", "Time Stamp"=timestamp(3696720864.018886 s since 1904-01-01), "Code"="Found", "Source"="Piston Settings", "Value"=5000.0, "Boolean"=FALSE, "String"="Delay (ms)", "Error"=FALSE, "Warning"=FALSE, " Fault"=FALSE}, {"Name"="Config Read", "Time Stamp"=timestamp(3696720864.001322 s since 1904-01-01), "Code"="Found", "Source"="Piston Settings", "Value"=51.0, "Boolean"=FALSE, "String"="Piston Diameter (mm)", "Error"=FALSE, "Warning"=FALSE, " Fault"=FALSE}, {"Name"="Config Read", "Time Stamp"=timestamp(3696720863.987963 s since 1904-01-01), "Code"="Found", "Source"="Piston Settings", "Value"=0.4, "Boolean"=FALSE, "String"="Up Force", "Error"=FALSE, "Warning"=FALSE, " Fault"=FALSE}, {"Name"="Config Read", "Time Stamp"=timestamp(3696720863.974054 s since 1904-01-01), "Code"="Found", "Source"="Piston Settings", "Value"=0.4, "Boolean"=FALSE, "String"="Transition Force", "Error"=FALSE, "Warning"=FALSE, " Fault"=FALSE}, {"Name"="Config Read", "Time Stamp"=timestamp(3696720863.960834 s since 1904-01-01), "Code"="Found", "Source"="Piston Settings", "Value"=0.1488, "Boolean"=FALSE, "String"="Forces Intercept", "Error"=FALSE, "Warning"=FALSE, " Fault"=FALSE}, {"Name"="Config Read", "Time Stamp"=timestamp(3696720863.942831 s since 1904-01-01), "Code"="Found", "Source"="Piston Settings", "Value"=0.0127, "Boolean"=FALSE, "String"="Forces Slope", "Error"=FALSE, "Warning"=FALSE, " Fault"=FALSE}, {"Name"="Config Read", "Time Stamp"=timestamp(3696720863.92748 s since 1904-01-01), "Code"="Found", "Source"="Bypass PID", "Value"=0.0, "Boolean"=FALSE, "String"="Derivative Value", "Error"=FALSE, "Warning"=FALSE, " Fault"=FALSE}, {"Name"="Config Read", "Time Stamp"=timestamp(3696720863.90886 s since 1904-01-01), "Code"="Found", "Source"="Bypass PID", "Value"=0.8, "Boolean"=FALSE, "String"="Integral Value", "Error"=FALSE, "Warning"=FALSE, " Fault"=FALSE}, {"Name"="Config Read", "Time Stamp"=timestamp(3696720863.887577 s since 1904-01-01), "Code"="Found", "Source"="Bypass PID", "Value"=1.5, "Boolean"=FALSE, "String"="Proportional Value", "Error"=FALSE, "Warning"=FALSE, " Fault"=FALSE}, {"Name"="Config Value Read", "Time Stamp"=timestamp(3696720863.871581 s since 1904-01-01), "Code"="", "Source"="", "Value"=0.0, "Boolean"=TRUE, "String"="Cascade", "Error"=FALSE, "Warning"=FALSE, " Fault"=FALSE}, {"Name"="Config Value Read", "Time Stamp"=timestamp(3696720863.855367 s since 1904-01-01), "Code"="", "Source"="", "Value"=0.0, "Boolean"=TRUE, "String"="220V", "Error"=FALSE, "Warning"=FALSE, " Fault"=FALSE}, {"Name"="Config Value Read", "Time Stamp"=timestamp(3696720863.840719 s since 1904-01-01), "Code"="", "Source"="", "Value"=0.0, "Boolean"=TRUE, "String"="Shuttle", "Error"=FALSE, "Warning"=FALSE, " Fault"=FALSE}, {"Name"="Config Value Read", "Time Stamp"=timestamp(3696720863.826449 s since 1904-01-01), "Code"="", "Source"="", "Value"=0.0, "Boolean"=TRUE, "String"="Handler", "Error"=FALSE, "Warning"=FALSE, " Fault"=FALSE}, {"Name"="Config Value Read", "Time Stamp"=timestamp(3696720863.812976 s since 1904-01-01), "Code"="", "Source"="", "Value"=0.0, "Boolean"=TRUE, "String"="Production", "Error"=FALSE, "Warning"=FALSE, " Fault"=FALSE}, {"Name"="Config Value Read", "Time Stamp"=timestamp(3696720863.79902 s since 1904-01-01), "Code"="", "Source"="", "Value"=0.0, "Boolean"=TRUE, "String"="Benchtop", "Error"=FALSE, "Warning"=FALSE, " Fault"=FALSE}, {"Name"="Config Value Read", "Time Stamp"=timestamp(3696720863.785258 s since 1904-01-01), "Code"="", "Source"="", "Value"=0.0, "Boolean"=TRUE, "String"="ATE", "Error"=FALSE, "Warning"=FALSE, " Fault"=FALSE}, {"Name"="Config Value Read", "Time Stamp"=timestamp(3696720863.77207 s since 1904-01-01), "Code"="", "Source"="", "Value"=0.0, "Boolean"=TRUE, "String"="HandClamp", "Error"=FALSE, "Warning"=FALSE, " Fault"=FALSE}, {"Name"="Config Value Read", "Time Stamp"=timestamp(3696720863.758603 s since 1904-01-01), "Code"="", "Source"="", "Value"=0.0, "Boolean"=TRUE, "String"="Sensors", "Error"=FALSE, "Warning"=FALSE, " Fault"=FALSE}, {"Name"="Config Value Read", "Time Stamp"=timestamp(3696720863.745397 s since 1904-01-01), "Code"="", "Source"="", "Value"=0.0, "Boolean"=TRUE, "String"="Purge", "Error"=FALSE, "Warning"=FALSE, " Fault"=FALSE}, {"Name"="Config Value Read", "Time Stamp"=timestamp(3696720863.729613 s since 1904-01-01), "Code"="", "Source"="", "Value"=0.0, "Boolean"=TRUE, "String"="Autostartup", "Error"=FALSE, "Warning"=FALSE, " Fault"=FALSE}, {"Name"="Config Value Read", "Time Stamp"=timestamp(3696720863.703458 s since 1904-01-01), "Code"="", "Source"="", "Value"=0.0, "Boolean"=TRUE, "String"="FTC200", "Error"=FALSE, "Warning"=FALSE, " Fault"=FALSE}, {"Name"="Config Loaded", "Time Stamp"=timestamp(3694477265.920138 s since 1904-01-01), "Code"="", "Source"="Config Read Initialize", "Value"=0.0, "Boolean"=FALSE, "String"="", "Error"=FALSE, "Warning"=FALSE, " Fault"=FALSE}, {"Name"="Config Read", "Time Stamp"=timestamp(3694477265.889239 s since 1904-01-01), "Code"="Found", "Source"="M2 TSD", "Value"=0.0, "Boolean"=FALSE, "String"="V Offset", "Error"=FALSE, "Warning"=FALSE, " Fault"=FALSE}, {"Name"="Config Read", "Time Stamp"=timestamp(3694477265.864218 s since 1904-01-01), "Code"="Found", "Source"="M2 TSD", "Value"=0.0, "Boolean"=FALSE, "String"="Offset", "Error"=FALSE, "Warning"=FALSE, " Fault"=FALSE}, {"Name"="Config Read", "Time Stamp"=timestamp(3694477265.817427 s since 1904-01-01), "Code"="Found", "Source"="M2 TSD", "Value"=1.0, "Boolean"=FALSE, "String"="Gain", "Error"=FALSE, "Warning"=FALSE, " Fault"=FALSE}, {"Name"="Config Read", "Time Stamp"=timestamp(3694477265.797822 s since 1904-01-01), "Code"="Found", "Source"="M1 TSD", "Value"=0.0, "Boolean"=FALSE, "String"="V Offset", "Error"=FALSE, "Warning"=FALSE, " Fault"=FALSE}, {"Name"="Config Read", "Time Stamp"=timestamp(3694477265.770337 s since 1904-01-01), "Code"="Found", "Source"="M1 TSD", "Value"=0.0, "Boolean"=FALSE, "String"="Offset", "Error"=FALSE, "Warning"=FALSE, " Fault"=FALSE}, {"Name"="Config Read", "Time Stamp"=timestamp(3694477265.740245 s since 1904-01-01), "Code"="Found", "Source"="M1 TSD", "Value"=1.0, "Boolean"=FALSE, "String"="Gain", "Error"=FALSE, "Warning"=FALSE, " Fault"=FALSE}, {"Name"="Config Read", "Time Stamp"=timestamp(3694477265.712941 s since 1904-01-01), "Code"="Found", "Source"="M2 T-Case Calibration", "Value"=0.0, "Boolean"=FALSE, "String"="Offset", "Error"=FALSE, "Warning"=FALSE, " Fault"=FALSE}, {"Name"="Config Read", "Time Stamp"=timestamp(3694477265.673546 s since 1904-01-01), "Code"="Found", "Source"="M1 T-Case Calibration", "Value"=0.0, "Boolean"=FALSE, "String"="Offset", "Error"=FALSE, "Warning"=FALSE, " Fault"=FALSE}, {"Name"="Config Read", "Time Stamp"=timestamp(3694477265.65254 s since 1904-01-01), "Code"="Found", "Source"="M1 T-Case Calibration", "Value"=1.0, "Boolean"=FALSE, "String"="Gain", "Error"=FALSE, "Warning"=FALSE, " Fault"=FALSE}, {"Name"="Config Read", "Time Stamp"=timestamp(3694477265.634211 s since 1904-01-01), "Code"="Found", "Source"="Heater PID TSD", "Value"=0.066, "Boolean"=FALSE, "String"="Derivative Value", "Error"=FALSE, "Warning"=FALSE, " Fault"=FALSE}, {"Name"="Config Read", "Time Stamp"=timestamp(3694477265.611758 s since 1904-01-01), "Code"="Found", "Source"="Heater PID TSD", "Value"=0.264, "Boolean"=FALSE, "String"="Integral Value", "Error"=FALSE, "Warning"=FALSE, " Fault"=FALSE}, {"Name"="Config Read", "Time Stamp"=timestamp(3694477265.585176 s since 1904-01-01), "Code"="Found", "Source"="Heater PID TSD", "Value"=4.207, "Boolean"=FALSE, "String"="Proportional Value", "Error"=FALSE, "Warning"=FALSE, " Fault"=FALSE}, {"Name"="Config Read", "Time Stamp"=timestamp(3694477265.555232 s since 1904-01-01), "Code"="Found", "Source"="M2 EEV PID", "Value"=0.0, "Boolean"=FALSE, "String"="Gain D", "Error"=FALSE, "Warning"=FALSE, " Fault"=FALSE}, {"Name"="Config Read", "Time Stamp"=timestamp(3694477265.536428 s since 1904-01-01), "Code"="Found", "Source"="M2 EEV PID", "Value"=0.25, "Boolean"=FALSE, "String"="Gain I", "Error"=FALSE, "Warning"=FALSE, " Fault"=FALSE}, {"Name"="Config Read", "Time Stamp"=timestamp(3694477265.512113 s since 1904-01-01), "Code"="Found", "Source"="M2 EEV PID", "Value"=-1.0, "Boolean"=FALSE, "String"="Gain P", "Error"=FALSE, "Warning"=FALSE, " Fault"=FALSE}, {"Name"="Config Read", "Time Stamp"=timestamp(3694477265.489148 s since 1904-01-01), "Code"="Found", "Source"="EEV PID", "Value"=15.0, "Boolean"=FALSE, "String"="M1 Superheat Setpoint ", "Error"=FALSE, "Warning"=FALSE, " Fault"=FALSE}, {"Name"="Config Read", "Time Stamp"=timestamp(3694477265.466779 s since 1904-01-01), "Code"="Found", "Source"="EEV PID", "Value"=0.0, "Boolean"=FALSE, "String"="Output Low", "Error"=FALSE, "Warning"=FALSE, " Fault"=FALSE}, {"Name"="Config Read", "Time Stamp"=timestamp(3694477265.445265 s since 1904-01-01), "Code"="Found", "Source"="EEV PID", "Value"=100.0, "Boolean"=FALSE, "String"="Output Hi", "Error"=FALSE, "Warning"=FALSE, " Fault"=FALSE}, {"Name"="Config Read", "Time Stamp"=timestamp(3694477265.416888 s since 1904-01-01), "Code"="Found", "Source"="EEV PID", "Value"=0.0, "Boolean"=FALSE, "String"="Gain D", "Error"=FALSE, "Warning"=FALSE, " Fault"=FALSE}, {"Name"="Config Read", "Time Stamp"=timestamp(3694477265.386231 s since 1904-01-01), "Code"="Found", "Source"="EEV PID", "Value"=0.5, "Boolean"=FALSE, "String"="Gain I", "Error"=FALSE, "Warning"=FALSE, " Fault"=FALSE}, {"Name"="Config Read", "Time Stamp"=timestamp(3694477265.342894 s since 1904-01-01), "Code"="Found", "Source"="EEV PID", "Value"=-1.0, "Boolean"=FALSE, "String"="Gain P", "Error"=FALSE, "Warning"=FALSE, " Fault"=FALSE}, {"Name"="Config Read", "Time Stamp"=timestamp(3694477265.327449 s since 1904-01-01), "Code"="Found", "Source"="EEV PID", "Value"=10.0, "Boolean"=FALSE, "String"="Dissabled Target", "Error"=FALSE, "Warning"=FALSE, " Fault"=FALSE}, {"Name"="Config Read", "Time Stamp"=timestamp(3694477265.292958 s since 1904-01-01), "Code"="Found", "Source"="EEV PID", "Value"=30.0, "Boolean"=FALSE, "String"="SS Steps", "Error"=FALSE, "Warning"=FALSE, " Fault"=FALSE}, {"Name"="Config Read", "Time Stamp"=timestamp(3694477265.272951 s since 1904-01-01), "Code"="Found", "Source"="EEV PID", "Value"=60.0, "Boolean"=FALSE, "String"="RD Steps", "Error"=FALSE, "Warning"=FALSE, " Fault"=FALSE}, {"Name"="Config Read", "Time Stamp"=timestamp(3694477265.253278 s since 1904-01-01), "Code"="Found", "Source"="EEV PID", "Value"=20.0, "Boolean"=FALSE, "String"="RU Steps", "Error"=FALSE, "Warning"=FALSE, " Fault"=FALSE}, {"Name"="Config Read", "Time Stamp"=timestamp(3694477265.235414 s since 1904-01-01), "Code"="Found", "Source"="EEV PID", "Value"=85.0, "Boolean"=FALSE, "String"="EBB Steps Closed", "Error"=FALSE, "Warning"=FALSE, " Fault"=FALSE}, {"Name"="Config Read", "Time Stamp"=timestamp(3694477265.219115 s since 1904-01-01), "Code"="Found", "Source"="EEV PID", "Value"=70.0, "Boolean"=FALSE, "String"="EBB Steps Open", "Error"=FALSE, "Warning"=FALSE, " Fault"=FALSE}, {"Name"="Config Read", "Time Stamp"=timestamp(3694477265.204931 s since 1904-01-01), "Code"="Found", "Source"="EEV PID", "Value"=2.0, "Boolean"=FALSE, "String"="EBB Tol", "Error"=FALSE, "Warning"=FALSE, " Fault"=FALSE}, {"Name"="Config Read", "Time Stamp"=timestamp(3694477265.19095 s since 1904-01-01), "Code"="Found", "Source"="EEV PID", "Value"=-60.0, "Boolean"=FALSE, "String"="EBB TH", "Error"=FALSE, "Warning"=FALSE, " Fault"=FALSE}, {"Name"="Config Read", "Time Stamp"=timestamp(3694477265.159413 s since 1904-01-01), "Code"="Found", "Source"="EEV PID", "Value"=50.0, "Boolean"=FALSE, "String"="RD Target", "Error"=FALSE, "Warning"=FALSE, " Fault"=FALSE}, {"Name"="Config Read", "Time Stamp"=timestamp(3694477265.142987 s since 1904-01-01), "Code"="Found", "Source"="EEV PID", "Value"=50.0, "Boolean"=FALSE, "String"="RU Target", "Error"=FALSE, "Warning"=FALSE, " Fault"=FALSE}, {"Name"="Config Read", "Time Stamp"=timestamp(3694477265.128078 s since 1904-01-01), "Code"="Found", "Source"="Temp TH", "Value"=3.0, "Boolean"=FALSE, "String"="SS Tol", "Error"=FALSE, "Warning"=FALSE, " Fault"=FALSE}, {"Name"="Config Read", "Time Stamp"=timestamp(3694477265.11145 s since 1904-01-01), "Code"="Found", "Source"="Temp TH", "Value"=10.0, "Boolean"=FALSE, "String"="Ramp-SS Delta T", "Error"=FALSE, "Warning"=FALSE, " Fault"=FALSE}, {"Name"="Config Read", "Time Stamp"=timestamp(3694477265.096049 s since 1904-01-01), "Code"="Found", "Source"="Temp TH", "Value"=10.0, "Boolean"=FALSE, "String"="Ramp Delta T", "Error"=FALSE, "Warning"=FALSE, " Fault"=FALSE}, {"Name"="Config Read", "Time Stamp"=timestamp(3694477265.081999 s since 1904-01-01), "Code"="Found", "Source"="Temp TH", "Value"=50.0, "Boolean"=FALSE, "String"="Pedestal Delta T", "Error"=FALSE, "Warning"=FALSE, " Fault"=FALSE}, {"Name"="Config Read", "Time Stamp"=timestamp(3694477265.056017 s since 1904-01-01), "Code"="Found", "Source"="Set Point Range", "Value"=-50.0, "Boolean"=FALSE, "String"="Min", "Error"=FALSE, "Warning"=FALSE, " Fault"=FALSE}, {"Name"="Config Read", "Time Stamp"=timestamp(3694477265.03829 s since 1904-01-01), "Code"="Found", "Source"="Set Point Range", "Value"=150.0, "Boolean"=FALSE, "String"="Max", "Error"=FALSE, "Warning"=FALSE, " Fault"=FALSE}, {"Name"="Config Read", "Time Stamp"=timestamp(3694477265.026133 s since 1904-01-01), "Code"="Found", "Source"="CryoMode PID Gains", "Value"=0.0, "Boolean"=FALSE, "String"="Derivative Value", "Error"=FALSE, "Warning"=FALSE, " Fault"=FALSE}, {"Name"="Config Read", "Time Stamp"=timestamp(3694477264.994502 s since 1904-01-01), "Code"="Found", "Source"="CryoMode PID Gains", "Value"=-1.0, "Boolean"=FALSE, "String"="Proportional Value", "Error"=FALSE, "Warning"=FALSE, " Fault"=FALSE}, {"Name"="Config Read", "Time Stamp"=timestamp(3694477264.964372 s since 1904-01-01), "Code"="Found", "Source"="M2 Heater PID", "Value"=0.2, "Boolean"=FALSE, "String"="Integral Value", "Error"=FALSE, "Warning"=FALSE, " Fault"=FALSE}, {"Name"="Config Read", "Time Stamp"=timestamp(3694477264.949709 s since 1904-01-01), "Code"="Found", "Source"="M2 Heater PID", "Value"=8.0, "Boolean"=FALSE, "String"="Proportional Value", "Error"=FALSE, "Warning"=FALSE, " Fault"=FALSE}, {"Name"="Config Read", "Time Stamp"=timestamp(3694477264.922364 s since 1904-01-01), "Code"="Found", "Source"="Heater PID", "Value"=0.264, "Boolean"=FALSE, "String"="Integral Value", "Error"=FALSE, "Warning"=FALSE, " Fault"=FALSE}, {"Name"="Config Read", "Time Stamp"=timestamp(3694477264.887045 s since 1904-01-01), "Code"="Found", "Source"="Piston Settings", "Value"=500.0, "Boolean"=FALSE, "String"="Pressure Ramp Delay (ms)", "Error"=FALSE, "Warning"=FALSE, " Fault"=FALSE}, {"Name"="Config Read", "Time Stamp"=timestamp(3694477264.871098 s since 1904-01-01), "Code"="Found", "Source"="Piston Settings", "Value"=5000.0, "Boolean"=FALSE, "String"="Delay (ms)", "Error"=FALSE, "Warning"=FALSE, " Fault"=FALSE}, {"Name"="Config Read", "Time Stamp"=timestamp(3694477264.854315 s since 1904-01-01), "Code"="Found", "Source"="Piston Settings", "Value"=51.0, "Boolean"=FALSE, "String"="Piston Diameter (mm)", "Error"=FALSE, "Warning"=FALSE, " Fault"=FALSE}, {"Name"="Config Read", "Time Stamp"=timestamp(3694477264.842293 s since 1904-01-01), "Code"="Found", "Source"="Piston Settings", "Value"=0.4, "Boolean"=FALSE, "String"="Up Force", "Error"=FALSE, "Warning"=FALSE, " Fault"=FALSE}, {"Name"="Config Read", "Time Stamp"=timestamp(3694477264.827921 s since 1904-01-01), "Code"="Found", "Source"="Piston Settings", "Value"=0.4, "Boolean"=FALSE, "String"="Transition Force", "Error"=FALSE, "Warning"=FALSE, " Fault"=FALSE}, {"Name"="Config Read", "Time Stamp"=timestamp(3694477264.811732 s since 1904-01-01), "Code"="Found", "Source"="Piston Settings", "Value"=0.1488, "Boolean"=FALSE, "String"="Forces Intercept", "Error"=FALSE, "Warning"=FALSE, " Fault"=FALSE}, {"Name"="Config Read", "Time Stamp"=timestamp(3694477264.789925 s since 1904-01-01), "Code"="Found", "Source"="Piston Settings", "Value"=0.0127, "Boolean"=FALSE, "String"="Forces Slope", "Error"=FALSE, "Warning"=FALSE, " Fault"=FALSE}, {"Name"="Config Read", "Time Stamp"=timestamp(3694477264.769342 s since 1904-01-01), "Code"="Found", "Source"="Bypass PID", "Value"=0.0, "Boolean"=FALSE, "String"="Derivative Value", "Error"=FALSE, "Warning"=FALSE, " Fault"=FALSE}, {"Name"="Config Read", "Time Stamp"=timestamp(3694477264.754113 s since 1904-01-01), "Code"="Found", "Source"="Bypass PID", "Value"=0.8, "Boolean"=FALSE, "String"="Integral Value", "Error"=FALSE, "Warning"=FALSE, " Fault"=FALSE}, {"Name"="Config Read", "Time Stamp"=timestamp(3694477264.741082 s since 1904-01-01), "Code"="Found", "Source"="Bypass PID", "Value"=1.5, "Boolean"=FALSE, "String"="Proportional Value", "Error"=FALSE, "Warning"=FALSE, " Fault"=FALSE}, {"Name"="Config Value Read", "Time Stamp"=timestamp(3694477264.726964 s since 1904-01-01), "Code"="", "Source"="", "Value"=0.0, "Boolean"=TRUE, "String"="Cascade", "Error"=FALSE, "Warning"=FALSE, " Fault"=FALSE}, {"Name"="Config Value Read", "Time Stamp"=timestamp(3694477264.696314 s since 1904-01-01), "Code"="", "Source"="", "Value"=0.0, "Boolean"=TRUE, "String"="Shuttle", "Error"=FALSE, "Warning"=FALSE, " Fault"=FALSE}, {"Name"="Config Value Read", "Time Stamp"=timestamp(3694477264.683843 s since 1904-01-01), "Code"="", "Source"="", "Value"=0.0, "Boolean"=TRUE, "String"="Handler", "Error"=FALSE, "Warning"=FALSE, " Fault"=FALSE}, {"Name"="Config Value Read", "Time Stamp"=timestamp(3694477264.658508 s since 1904-01-01), "Code"="", "Source"="", "Value"=0.0, "Boolean"=TRUE, "String"="Benchtop", "Error"=FALSE, "Warning"=FALSE, " Fault"=FALSE}, {"Name"="Config Value Read", "Time Stamp"=timestamp(3694477264.645271 s since 1904-01-01), "Code"="", "Source"="", "Value"=0.0, "Boolean"=TRUE, "String"="ATE", "Error"=FALSE, "Warning"=FALSE, " Fault"=FALSE}, {"Name"="Config Value Read", "Time Stamp"=timestamp(3694477264.620864 s since 1904-01-01), "Code"="", "Source"="", "Value"=0.0, "Boolean"=TRUE, "String"="Sensors", "Error"=FALSE, "Warning"=FALSE, " Fault"=FALSE}, {"Name"="Config Value Read", "Time Stamp"=timestamp(3694477264.605268 s since 1904-01-01), "Code"="", "Source"="", "Value"=0.0, "Boolean"=TRUE, "String"="Purge", "Error"=FALSE, "Warning"=FALSE, " Fault"=FALSE}, {"Name"="Config Value Read", "Time Stamp"=timestamp(3694477264.591463 s since 1904-01-01), "Code"="", "Source"="", "Value"=0.0, "Boolean"=TRUE, "String"="Autostartup", "Error"=FALSE, "Warning"=FALSE, " Fault"=FALSE}, {"Name"="Config Value Read", "Time Stamp"=timestamp(3694477264.578332 s since 1904-01-01), "Code"="", "Source"="", "Value"=0.0, "Boolean"=TRUE, "String"="FTC200", "Error"=FALSE, "Warning"=FALSE, " Fault"=FALSE}, {"Name"="Config Value Read", "Time Stamp"=timestamp(3694477264.566156 s since 1904-01-01), "Code"="", "Source"="", "Value"=0.0, "Boolean"=TRUE, "String"="60Hz Power", "Error"=FALSE, "Warning"=FALSE, " Fault"=FALSE}, {"Name"="All Values Found", "Time Stamp"=timestamp(3694477264.52556 s since 1904-01-01), "Code"="", "Source"="Write Config", "Value"=0.0, "Boolean"=FALSE, "String"="FAIL", "Error"=TRUE, "Warning"=TRUE, " Fault"=FALSE}, {"Name"="Set Point Range", "Time Stamp"=timestamp(3694477264.499372 s since 1904-01-01), "Code"="", "Source"="", "Value"=-50.0, "Boolean"=TRUE, "String"="Min", "Error"=FALSE, "Warning"=FALSE, " Fault"=FALSE}, {"Name"="Set Point Range", "Time Stamp"=timestamp(3694477264.488088 s since 1904-01-01), "Code"="", "Source"="", "Value"=150.0, "Boolean"=TRUE, "String"="Max", "Error"=FALSE, "Warning"=FALSE, " Fault"=FALSE}, {"Name"="Write To Config", "Time Stamp"=timestamp(3694477264.467938 s since 1904-01-01), "Code"="", "Source"="", "Value"=0.0, "Boolean"=TRUE, "String"="", "Error"=FALSE, "Warning"=FALSE, " Fault"=FALSE}, {"Name"="Write To Config", "Time Stamp"=timestamp(3694477264.451984 s since 1904-01-01), "Code"="", "Source"="", "Value"=0.0, "Boolean"=FALSE, "String"="", "Error"=FALSE, "Warning"=FALSE, " Fault"=FALSE}, {"Name"="New Config Data", "Time Stamp"=timestamp(3694477264.126112 s since 1904-01-01), "Code"="", "Source"="GUI Event", "Value"=nan, "Boolean"=TRUE, "String"="", "Error"=FALSE, "Warning"=FALSE, " Fault"=FALSE}, {"Name"="PID Bypassed", "Time Stamp"=timestamp(3694476879.804472 s since 1904-01-01), "Code"="", "Source"="APP:Set/Send PID Bypass", "Value"=0.0, "Boolean"=FALSE, "String"="", "Error"=FALSE, "Warning"=FALSE, " Fault"=FALSE}, {"Name"="Read Saved State", "Time Stamp"=timestamp(3694476879.481245 s since 1904-01-01), "Code"="", "Source"="", "Value"=0.0, "Boolean"=FALSE, "String"="", "Error"=FALSE, "Warning"=FALSE, " Fault"=FALSE}, {"Name"="Bypass Target Change", "Time Stamp"=timestamp(3694476879.273275 s since 1904-01-01), "Code"="", "Source"="Bypass:Get Target", "Value"=110.0, "Boolean"=FALSE, "String"="", "Error"=FALSE, "Warning"=FALSE, " Fault"=FALSE}, {"Name"="FAULT:High Discharge Pressure", "Time Stamp"=timestamp(3694476878.275028 s since 1904-01-01), "Code"="", "Source"="", "Value"=1.0001793333333333, "Boolean"=FALSE, "String"="", "Error"=FALSE, "Warning"=FALSE, " Fault"=TRUE}, {"Name"="Bypass Reset", "Time Stamp"=timestamp(3694476870.703684 s since 1904-01-01), "Code"="", "Source"="Bypass:Reset Bypass", "Value"=0.0, "Boolean"=TRUE, "String"="", "Error"=FALSE, "Warning"=FALSE, " Fault"=FALSE}, {"Name"="WARN:High Suction Temp", "Time Stamp"=timestamp(3694476862.262302 s since 1904-01-01), "Code"="", "Source"="", "Value"=1.0018069, "Boolean"=FALSE, "String"="", "Error"=TRUE, "Warning"=TRUE, " Fault"=FALSE}, {"Name"="Bypass Reset", "Time Stamp"=timestamp(3694476854.516428 s since 1904-01-01), "Code"="", "Source"="Bypass:Reset Bypass", "Value"=0.0, "Boolean"=FALSE, "String"="", "Error"=FALSE, "Warning"=FALSE, " Fault"=FALSE}, {"Name"="Bypass Target Change", "Time Stamp"=timestamp(3694476854.414283 s since 1904-01-01), "Code"="", "Source"="Bypass:Get Target", "Value"=5.0, "Boolean"=FALSE, "String"="", "Error"=FALSE, "Warning"=FALSE, " Fault"=FALSE}, {"Name"="PID Bypassed", "Time Stamp"=timestamp(3694476853.772397 s since 1904-01-01), "Code"="", "Source"="APP:Set/Send PID Bypass", "Value"=0.0, "Boolean"=FALSE, "String"="", "Error"=FALSE, "Warning"=FALSE, " Fault"=FALSE}, {"Name"="Create New Datalog File", "Time Stamp"=timestamp(3694476853.177307 s since 1904-01-01), "Code"="", "Source"="", "Value"=0.0, "Boolean"=FALSE, "String"="", "Error"=FALSE, "Warning"=FALSE, " Fault"=FALSE}, {"Name"="Read Saved State", "Time Stamp"=timestamp(3694476853.071121 s since 1904-01-01), "Code"="", "Source"="", "Value"=0.0, "Boolean"=FALSE, "String"="", "Error"=FALSE, "Warning"=FALSE, " Fault"=FALSE}, {"Name"="Compressor Enable", "Time Stamp"=timestamp(3694476853.05346 s since 1904-01-01), "Code"="", "Source"="Save State", "Value"=0.0, "Boolean"=TRUE, "String"="System Settings", "Error"=FALSE, "Warning"=FALSE, " Fault"=FALSE}, {"Name"="System Power", "Time Stamp"=timestamp(3694476852.047049 s since 1904-01-01), "Code"="", "Source"="GUI Event", "Value"=nan, "Boolean"=TRUE, "String"="", "Error"=FALSE, "Warning"=FALSE, " Fault"=FALSE}, {"Name"="Config Loaded", "Time Stamp"=timestamp(3694476819.482151 s since 1904-01-01), "Code"="", "Source"="Config Read Initialize", "Value"=0.0, "Boolean"=FALSE, "String"="", "Error"=FALSE, "Warning"=FALSE, " Fault"=FALSE}, {"Name"="Config Read", "Time Stamp"=timestamp(3694476819.469165 s since 1904-01-01), "Code"="Found", "Source"="M2 TSD", "Value"=0.0, "Boolean"=FALSE, "String"="V Offset", "Error"=FALSE, "Warning"=FALSE, " Fault"=FALSE}, {"Name"="Config Read", "Time Stamp"=timestamp(3694476819.459801 s since 1904-01-01), "Code"="Found", "Source"="M2 TSD", "Value"=0.0, "Boolean"=FALSE, "String"="Offset", "Error"=FALSE, "Warning"=FALSE, " Fault"=FALSE}, {"Name"="Config Read", "Time Stamp"=timestamp(3694476819.440094 s since 1904-01-01), "Code"="Found", "Source"="M2 TSD", "Value"=1.0, "Boolean"=FALSE, "String"="Gain", "Error"=FALSE, "Warning"=FALSE, " Fault"=FALSE}, {"Name"="Config Read", "Time Stamp"=timestamp(3694476819.415377 s since 1904-01-01), "Code"="Found", "Source"="M1 TSD", "Value"=0.0, "Boolean"=FALSE, "String"="Offset", "Error"=FALSE, "Warning"=FALSE, " Fault"=FALSE}, {"Name"="Config Read", "Time Stamp"=timestamp(3694476819.394966 s since 1904-01-01), "Code"="Found", "Source"="M2 T-Case Calibration", "Value"=0.0, "Boolean"=FALSE, "String"="Offset", "Error"=FALSE, "Warning"=FALSE, " Fault"=FALSE}, {"Name"="Config Read", "Time Stamp"=timestamp(3694476819.384983 s since 1904-01-01), "Code"="Found", "Source"="M2 T-Case Calibration", "Value"=1.0, "Boolean"=FALSE, "String"="Gain", "Error"=FALSE, "Warning"=FALSE, " Fault"=FALSE}, {"Name"="Config Read", "Time Stamp"=timestamp(3694476819.375701 s since 1904-01-01), "Code"="Found", "Source"="M1 T-Case Calibration", "Value"=0.0, "Boolean"=FALSE, "String"="Offset", "Error"=FALSE, "Warning"=FALSE, " Fault"=FALSE}, {"Name"="Config Read", "Time Stamp"=timestamp(3694476819.357495 s since 1904-01-01), "Code"="Found", "Source"="Heater PID TSD", "Value"=0.066, "Boolean"=FALSE, "String"="Derivative Value", "Error"=FALSE, "Warning"=FALSE, " Fault"=FALSE}, {"Name"="Config Read", "Time Stamp"=timestamp(3694476819.346424 s since 1904-01-01), "Code"="Found", "Source"="Heater PID TSD", "Value"=0.264, "Boolean"=FALSE, "String"="Integral Value", "Error"=FALSE, "Warning"=FALSE, " Fault"=FALSE}, {"Name"="Config Read", "Time Stamp"=timestamp(3694476819.32352 s since 1904-01-01), "Code"="Found", "Source"="M2 EEV PID", "Value"=0.0, "Boolean"=FALSE, "String"="Gain D", "Error"=FALSE, "Warning"=FALSE, " Fault"=FALSE}, {"Name"="Config Read", "Time Stamp"=timestamp(3694476819.297595 s since 1904-01-01), "Code"="Found", "Source"="M2 EEV PID", "Value"=-1.0, "Boolean"=FALSE, "String"="Gain P", "Error"=FALSE, "Warning"=FALSE, " Fault"=FALSE}, {"Name"="Config Read", "Time Stamp"=timestamp(3694476819.267418 s since 1904-01-01), "Code"="Found", "Source"="EEV PID", "Value"=100.0, "Boolean"=FALSE, "String"="Output Hi", "Error"=FALSE, "Warning"=FALSE, " Fault"=FALSE}, {"Name"="Config Read", "Time Stamp"=timestamp(3694476819.246136 s since 1904-01-01), "Code"="Found", "Source"="EEV PID", "Value"=0.5, "Boolean"=FALSE, "String"="Gain I", "Error"=FALSE, "Warning"=FALSE, " Fault"=FALSE}, {"Name"="Config Read", "Time Stamp"=timestamp(3694476819.214889 s since 1904-01-01), "Code"="Found", "Source"="EEV PID", "Value"=30.0, "Boolean"=FALSE, "String"="SS Steps", "Error"=FALSE, "Warning"=FALSE, " Fault"=FALSE}, {"Name"="Config Read", "Time Stamp"=timestamp(3694476819.176973 s since 1904-01-01), "Code"="Found", "Source"="EEV PID", "Value"=85.0, "Boolean"=FALSE, "String"="EBB Steps Closed", "Error"=FALSE, "Warning"=FALSE, " Fault"=FALSE}, {"Name"="Config Read", "Time Stamp"=timestamp(3694476819.164415 s since 1904-01-01), "Code"="Found", "Source"="EEV PID", "Value"=70.0, "Boolean"=FALSE, "String"="EBB Steps Open", "Error"=FALSE, "Warning"=FALSE, " Fault"=FALSE}, {"Name"="Config Read", "Time Stamp"=timestamp(3694476819.136318 s since 1904-01-01), "Code"="Found", "Source"="EEV PID", "Value"=50.0, "Boolean"=FALSE, "String"="SS Target", "Error"=FALSE, "Warning"=FALSE, " Fault"=FALSE}, {"Name"="Config Read", "Time Stamp"=timestamp(3694476819.10687 s since 1904-01-01), "Code"="Found", "Source"="Temp TH", "Value"=3.0, "Boolean"=FALSE, "String"="SS Tol", "Error"=FALSE, "Warning"=FALSE, " Fault"=FALSE}, {"Name"="Config Read", "Time Stamp"=timestamp(3694476819.077254 s since 1904-01-01), "Code"="Found", "Source"="Temp TH", "Value"=50.0, "Boolean"=FALSE, "String"="Pedestal Delta T", "Error"=FALSE, "Warning"=FALSE, " Fault"=FALSE}, {"Name"="Config Read", "Time Stamp"=timestamp(3694476819.044423 s since 1904-01-01), "Code"="Found", "Source"="CryoMode PID Gains", "Value"=0.0, "Boolean"=FALSE, "String"="Derivative Value", "Error"=FALSE, "Warning"=FALSE, " Fault"=FALSE}, {"Name"="Config Read", "Time Stamp"=timestamp(3694476819.017483 s since 1904-01-01), "Code"="Found", "Source"="M2 Heater PID", "Value"=0.0, "Boolean"=FALSE, "String"="Derivative Value", "Error"=FALSE, "Warning"=FALSE, " Fault"=FALSE}, {"Name"="Config Read", "Time Stamp"=timestamp(3694476818.989686 s since 1904-01-01), "Code"="Found", "Source"="Heater PID", "Value"=0.0, "Boolean"=FALSE, "String"="Derivative Value", "Error"=FALSE, "Warning"=FALSE, " Fault"=FALSE}, {"Name"="Config Read", "Time Stamp"=timestamp(3694476818.949451 s since 1904-01-01), "Code"="Found", "Source"="Piston Settings", "Value"=500.0, "Boolean"=FALSE, "String"="Pressure Ramp Delay (ms)", "Error"=FALSE, "Warning"=FALSE, " Fault"=FALSE}, {"Name"="Config Read", "Time Stamp"=timestamp(3694476818.924137 s since 1904-01-01), "Code"="Found", "Source"="Piston Settings", "Value"=51.0, "Boolean"=FALSE, "String"="Piston Diameter (mm)", "Error"=FALSE, "Warning"=FALSE, " Fault"=FALSE}, {"Name"="Config Read", "Time Stamp"=timestamp(3694476818.885518 s since 1904-01-01), "Code"="Found", "Source"="Piston Settings", "Value"=0.1488, "Boolean"=FALSE, "String"="Forces Intercept", "Error"=FALSE, "Warning"=FALSE, " Fault"=FALSE}, {"Name"="Config Read", "Time Stamp"=timestamp(3694476818.851494 s since 1904-01-01), "Code"="Found", "Source"="Bypass PID", "Value"=0.0, "Boolean"=FALSE, "String"="Derivative Value", "Error"=FALSE, "Warning"=FALSE, " Fault"=FALSE}, {"Name"="Config Read", "Time Stamp"=timestamp(3694476818.812029 s since 1904-01-01), "Code"="Found", "Source"="Bypass PID", "Value"=1.5, "Boolean"=FALSE, "String"="Proportional Value", "Error"=FALSE, "Warning"=FALSE, " Fault"=FALSE}, {"Name"="Config Value Read", "Time Stamp"=timestamp(3694476818.768437 s since 1904-01-01), "Code"="", "Source"="", "Value"=0.0, "Boolean"=TRUE, "String"="Shuttle", "Error"=FALSE, "Warning"=FALSE, " Fault"=FALSE}, {"Name"="Config Value Read", "Time Stamp"=timestamp(3694476818.722092 s since 1904-01-01), "Code"="", "Source"="", "Value"=0.0, "Boolean"=TRUE, "String"="Benchtop", "Error"=FALSE, "Warning"=FALSE, " Fault"=FALSE}, {"Name"="Config Value Read", "Time Stamp"=timestamp(3694476818.683504 s since 1904-01-01), "Code"="", "Source"="", "Value"=0.0, "Boolean"=TRUE, "String"="Sensors", "Error"=FALSE, "Warning"=FALSE, " Fault"=FALSE}, {"Name"="Config Value Read", "Time Stamp"=timestamp(3694476818.645664 s since 1904-01-01), "Code"="", "Source"="", "Value"=0.0, "Boolean"=TRUE, "String"="FTC200", "Error"=FALSE, "Warning"=FALSE, " Fault"=FALSE}, {"Name"="All Values Found", "Time Stamp"=timestamp(3694476818.409025 s since 1904-01-01), "Code"="", "Source"="Write Config", "Value"=0.0, "Boolean"=FALSE, "String"="FAIL", "Error"=TRUE, "Warning"=TRUE, " Fault"=FALSE}, {"Name"="Set Point Range", "Time Stamp"=timestamp(3694476818.37513 s since 1904-01-01), "Code"="", "Source"="", "Value"=-50.0, "Boolean"=TRUE, "String"="Min", "Error"=FALSE, "Warning"=FALSE, " Fault"=FALSE}, {"Name"="Write To Config", "Time Stamp"=timestamp(3694476818.345342 s since 1904-01-01), "Code"="", "Source"="", "Value"=0.0, "Boolean"=TRUE, "String"="", "Error"=FALSE, "Warning"=FALSE, " Fault"=FALSE}, {"Name"="New Config Data", "Time Stamp"=timestamp(3694476817.62503 s since 1904-01-01), "Code"="", "Source"="GUI Event", "Value"=nan, "Boolean"=TRUE, "String"="", "Error"=FALSE, "Warning"=FALSE, " Fault"=FALSE}, {"Name"="Bypass Target Change", "Time Stamp"=timestamp(3694476692.418108 s since 1904-01-01), "Code"="", "Source"="Bypass:Get Target", "Value"=110.0, "Boolean"=FALSE, "String"="", "Error"=FALSE, "Warning"=FALSE, " Fault"=FALSE}, {"Name"="PID Bypassed", "Time Stamp"=timestamp(3694476691.986481 s since 1904-01-01), "Code"="", "Source"="APP:Set/Send PID Bypass", "Value"=0.0, "Boolean"=FALSE, "String"="", "Error"=FALSE, "Warning"=FALSE, " Fault"=FALSE}, {"Name"="Read Saved State", "Time Stamp"=timestamp(3694476691.616353 s since 1904-01-01), "Code"="", "Source"="", "Value"=0.0, "Boolean"=FALSE, "String"="", "Error"=FALSE, "Warning"=FALSE, " Fault"=FALSE}, {"Name"="System Power", "Time Stamp"=timestamp(3694476690.708352 s since 1904-01-01), "Code"="", "Source"="GUI Event", "Value"=nan, "Boolean"=FALSE, "String"="", "Error"=FALSE, "Warning"=FALSE, " Fault"=FALSE}, {"Name"="WARN:High Discharge Pressure", "Time Stamp"=timestamp(3694476671.084012 s since 1904-01-01), "Code"="", "Source"="", "Value"=1.0008514666666666, "Boolean"=FALSE, "String"="", "Error"=TRUE, "Warning"=TRUE, " Fault"=FALSE}, {"Name"="WARN:High Suction Temp", "Time Stamp"=timestamp(3694476669.080513 s since 1904-01-01), "Code"="", "Source"="", "Value"=1.0009536, "Boolean"=FALSE, "String"="", "Error"=TRUE, "Warning"=TRUE, " Fault"=FALSE}, {"Name"="Bypass Reset", "Time Stamp"=timestamp(3694476604.235173 s since 1904-01-01), "Code"="", "Source"="Bypass:Reset Bypass", "Value"=0.0, "Boolean"=TRUE, "String"="", "Error"=FALSE, "Warning"=FALSE, " Fault"=FALSE}, {"Name"="WARN:High Suction Temp", "Time Stamp"=timestamp(3694476595.015898 s since 1904-01-01), "Code"="", "Source"="", "Value"=1.0013314, "Boolean"=FALSE, "String"="", "Error"=TRUE, "Warning"=TRUE, " Fault"=FALSE}, {"Name"="Bypass Reset", "Time Stamp"=timestamp(3694476587.883497 s since 1904-01-01), "Code"="", "Source"="Bypass:Reset Bypass", "Value"=0.0, "Boolean"=FALSE, "String"="", "Error"=FALSE, "Warning"=FALSE, " Fault"=FALSE}, {"Name"="Bypass Reset", "Time Stamp"=timestamp(3694476586.763591 s since 1904-01-01), "Code"="", "Source"="Bypass:Reset Bypass", "Value"=0.0, "Boolean"=TRUE, "String"="", "Error"=FALSE, "Warning"=FALSE, " Fault"=FALSE}, {"Name"="Bypass PID Gains Change", "Time Stamp"=timestamp(3694476586.713091 s since 1904-01-01), "Code"="", "Source"="Bypass:Get Gains", "Value"=0.0, "Boolean"=FALSE, "String"="", "Error"=FALSE, "Warning"=FALSE, " Fault"=FALSE}, {"Name"="Bypass Target Change", "Time Stamp"=timestamp(3694476586.663417 s since 1904-01-01), "Code"="", "Source"="Bypass:Get Target", "Value"=5.0, "Boolean"=FALSE, "String"="", "Error"=FALSE, "Warning"=FALSE, " Fault"=FALSE}, {"Name"="Send EEV PID Target", "Time Stamp"=timestamp(3694476586.194424 s since 1904-01-01), "Code"="", "Source"="APP:Send EEV PID Target", "Value"=50.0, "Boolean"=FALSE, "String"="", "Error"=FALSE, "Warning"=FALSE, " Fault"=FALSE}, {"Name"="PID Bypassed", "Time Stamp"=timestamp(3694476586.03578 s since 1904-01-01), "Code"="", "Source"="APP:Set/Send PID Bypass", "Value"=0.0, "Boolean"=FALSE, "String"="", "Error"=FALSE, "Warning"=FALSE, " Fault"=FALSE}, {"Name"="Create New Datalog File", "Time Stamp"=timestamp(3694476585.423562 s since 1904-01-01), "Code"="", "Source"="", "Value"=0.0, "Boolean"=FALSE, "String"="", "Error"=FALSE, "Warning"=FALSE, " Fault"=FALSE}, {"Name"="Read Saved State", "Time Stamp"=timestamp(3694476585.225987 s since 1904-01-01), "Code"="", "Source"="", "Value"=0.0, "Boolean"=FALSE, "String"="", "Error"=FALSE, "Warning"=FALSE, " Fault"=FALSE}, {"Name"="System Power", "Time Stamp"=timestamp(3694476584.159032 s since 1904-01-01), "Code"="", "Source"="GUI Event", "Value"=nan, "Boolean"=TRUE, "String"="", "Error"=FALSE, "Warning"=FALSE, " Fault"=FALSE}, {"Name"="Bypass Target Change", "Time Stamp"=timestamp(3694475779.11214 s since 1904-01-01), "Code"="", "Source"="Bypass:Get Target", "Value"=110.0, "Boolean"=FALSE, "String"="", "Error"=FALSE, "Warning"=FALSE, " Fault"=FALSE}, {"Name"="Mains Frequency", "Time Stamp"=timestamp(3694475778.309163 s since 1904-01-01), "Code"="", "Source"="Init System Module", "Value"=222.87822823027352, "Boolean"=FALSE, "String"="", "Error"=FALSE, "Warning"=FALSE, " Fault"=FALSE}, {"Name"="PID Bypassed", "Time Stamp"=timestamp(3694475774.850349 s since 1904-01-01), "Code"="", "Source"="APP:Set/Send PID Bypass", "Value"=0.0, "Boolean"=FALSE, "String"="", "Error"=FALSE, "Warning"=FALSE, " Fault"=FALSE}, {"Name"="M1 Setpoint Change", "Time Stamp"=timestamp(3694475774.709515 s since 1904-01-01), "Code"="", "Source"="APP:Send Set Temp", "Value"=25.0, "Boolean"=FALSE, "String"="", "Error"=FALSE, "Warning"=TRUE, " Fault"=FALSE}, {"Name"="Bypass Inintialize", "Time Stamp"=timestamp(3694475774.61621 s since 1904-01-01), "Code"="", "Source"="", "Value"=4366.0, "Boolean"=FALSE, "String"="Complete", "Error"=FALSE, "Warning"=FALSE, " Fault"=FALSE}, {"Name"="M1 EEV Check Position", "Time Stamp"=timestamp(3694475764.392521 s since 1904-01-01), "Code"="", "Source"="EEV:Check Position", "Value"=0.0, "Boolean"=FALSE, "String"="", "Error"=FALSE, "Warning"=FALSE, " Fault"=FALSE}, {"Name"="", "Time Stamp"=timestamp(3694475764.353422 s since 1904-01-01), "Code"="", "Source"="EEV:Config", "Value"=0.0, "Boolean"=FALSE, "String"="", "Error"=FALSE, "Warning"=FALSE, " Fault"=FALSE}, {"Name"="Config Loaded", "Time Stamp"=timestamp(3694475762.994369 s since 1904-01-01), "Code"="", "Source"="Config Read Initialize", "Value"=0.0, "Boolean"=FALSE, "String"="", "Error"=FALSE, "Warning"=FALSE, " Fault"=FALSE}, {"Name"="Config Read", "Time Stamp"=timestamp(3694475762.988522 s since 1904-01-01), "Code"="Found", "Source"="M2 TSD", "Value"=0.0, "Boolean"=FALSE, "String"="V Offset", "Error"=FALSE, "Warning"=FALSE, " Fault"=FALSE}, {"Name"="Config Read", "Time Stamp"=timestamp(3694475762.97171 s since 1904-01-01), "Code"="Found", "Source"="M1 TSD", "Value"=0.0, "Boolean"=FALSE, "String"="V Offset", "Error"=FALSE, "Warning"=FALSE, " Fault"=FALSE}, {"Name"="Config Read", "Time Stamp"=timestamp(3694475762.953515 s since 1904-01-01), "Code"="Found", "Source"="M2 T-Case Calibration", "Value"=1.0, "Boolean"=FALSE, "String"="Gain", "Error"=FALSE, "Warning"=FALSE, " Fault"=FALSE}, {"Name"="Config Read", "Time Stamp"=timestamp(3694475762.930652 s since 1904-01-01), "Code"="Found", "Source"="Heater PID TSD", "Value"=0.264, "Boolean"=FALSE, "String"="Integral Value", "Error"=FALSE, "Warning"=FALSE, " Fault"=FALSE}, {"Name"="Config Read", "Time Stamp"=timestamp(3694475762.908836 s since 1904-01-01), "Code"="Found", "Source"="M2 EEV PID", "Value"=-1.0, "Boolean"=FALSE, "String"="Gain P", "Error"=FALSE, "Warning"=FALSE, " Fault"=FALSE}, {"Name"="Config Read", "Time Stamp"=timestamp(3694475762.889528 s since 1904-01-01), "Code"="Found", "Source"="EEV PID", "Value"=100.0, "Boolean"=FALSE, "String"="Output Hi", "Error"=FALSE, "Warning"=FALSE, " Fault"=FALSE}, {"Name"="Config Read", "Time Stamp"=timestamp(3694475762.856183 s since 1904-01-01), "Code"="Found", "Source"="EEV PID", "Value"=10.0, "Boolean"=FALSE, "String"="Dissabled Target", "Error"=FALSE, "Warning"=FALSE, " Fault"=FALSE}, {"Name"="Config Read", "Time Stamp"=timestamp(3694475762.827818 s since 1904-01-01), "Code"="Found", "Source"="EEV PID", "Value"=20.0, "Boolean"=FALSE, "String"="RU Steps", "Error"=FALSE, "Warning"=FALSE, " Fault"=FALSE}, {"Name"="Config Read", "Time Stamp"=timestamp(3694475762.792605 s since 1904-01-01), "Code"="Found", "Source"="EEV PID", "Value"=2.0, "Boolean"=FALSE, "String"="EBB Tol", "Error"=FALSE, "Warning"=FALSE, " Fault"=FALSE}, {"Name"="Config Read", "Time Stamp"=timestamp(3694475762.762856 s since 1904-01-01), "Code"="Found", "Source"="Temp TH", "Value"=3.0, "Boolean"=FALSE, "String"="SS Tol", "Error"=FALSE, "Warning"=FALSE, " Fault"=FALSE}, {"Name"="Config Read", "Time Stamp"=timestamp(3694475762.739489 s since 1904-01-01), "Code"="Found", "Source"="Set Point Range", "Value"=-50.0, "Boolean"=FALSE, "String"="Min", "Error"=FALSE, "Warning"=FALSE, " Fault"=FALSE}, {"Name"="Config Read", "Time Stamp"=timestamp(3694475762.706976 s since 1904-01-01), "Code"="Found", "Source"="CryoMode PID Gains", "Value"=-1.0, "Boolean"=FALSE, "String"="Proportional Value", "Error"=FALSE, "Warning"=FALSE, " Fault"=FALSE}, {"Name"="Config Read", "Time Stamp"=timestamp(3694475762.69231 s since 1904-01-01), "Code"="Found", "Source"="M2 Heater PID", "Value"=8.0, "Boolean"=FALSE, "String"="Proportional Value", "Error"=FALSE, "Warning"=FALSE, " Fault"=FALSE}, {"Name"="Config Read", "Time Stamp"=timestamp(3694475762.677565 s since 1904-01-01), "Code"="Found", "Source"="Heater PID", "Value"=8.207, "Boolean"=FALSE, "String"="Proportional Value", "Error"=FALSE, "Warning"=FALSE, " Fault"=FALSE}, {"Name"="Config Read", "Time Stamp"=timestamp(3694475762.650954 s since 1904-01-01), "Code"="Found", "Source"="Piston Settings", "Value"=0.4, "Boolean"=FALSE, "String"="Up Force", "Error"=FALSE, "Warning"=FALSE, " Fault"=FALSE}, {"Name"="Config Read", "Time Stamp"=timestamp(3694475762.61453 s since 1904-01-01), "Code"="Found", "Source"="Bypass PID", "Value"=0.0, "Boolean"=FALSE, "String"="Derivative Value", "Error"=FALSE, "Warning"=FALSE, " Fault"=FALSE}, {"Name"="Config Value Read", "Time Stamp"=timestamp(3694475762.587557 s since 1904-01-01), "Code"="", "Source"="", "Value"=0.0, "Boolean"=TRUE, "String"="Shuttle", "Error"=FALSE, "Warning"=FALSE, " Fault"=FALSE}, {"Name"="Config Value Read", "Time Stamp"=timestamp(3694475762.559864 s since 1904-01-01), "Code"="", "Source"="", "Value"=0.0, "Boolean"=TRUE, "String"="HandClamp", "Error"=FALSE, "Warning"=FALSE, " Fault"=FALSE}, {"Name"="Config Value Read", "Time Stamp"=timestamp(3694475762.539021 s since 1904-01-01), "Code"="", "Source"="", "Value"=0.0, "Boolean"=TRUE, "String"="FTC200", "Error"=FALSE, "Warning"=FALSE, " Fault"=FALSE}, {"Name"="Read Saved State", "Time Stamp"=timestamp(3694475762.483209 s since 1904-01-01), "Code"="", "Source"="", "Value"=0.0, "Boolean"=FALSE, "String"="", "Error"=FALSE, "Warning"=FALSE, " Fault"=FALSE}, {"Name"="EMO Not Detected", "Time Stamp"=timestamp(3694475762.363976 s since 1904-01-01), "Code"="", "Source"="", "Value"=0.0, "Boolean"=FALSE, "String"="", "Error"=FALSE, "Warning"=FALSE, " Fault"=FALSE}, {"Name"="EEV:Set V", "Time Stamp"=timestamp(3694475762.33968 s since 1904-01-01), "Code"="", "Source"="", "Value"=0.0, "Boolean"=FALSE, "String"="", "Error"=FALSE, "Warning"=FALSE, " Fault"=FALSE}, {"Name"="Odometer Loaded", "Time Stamp"=timestamp(3694475762.303858 s since 1904-01-01), "Code"="", "Source"="", "Value"=0.0, "Boolean"=FALSE, "String"="", "Error"=FALSE, "Warning"=FALSE, " Fault"=FALSE}, {"Name"="FPGA Load Complete", "Time Stamp"=timestamp(3694475762.250984 s since 1904-01-01), "Code"="", "Source"="Init FPGA IO.vi", "Value"=0.0, "Boolean"=FALSE, "String"="", "Error"=FALSE, "Warning"=FALSE, " Fault"=FALSE}, {"Name"="Pressure Test", "Time Stamp"=timestamp(3694475760.247373 s since 1904-01-01), "Code"="", "Source"="Init FPGA IO 2.0.vi", "Value"=0.0, "Boolean"=FALSE, "String"="FAIL", "Error"=FALSE, "Warning"=TRUE, " Fault"=FALSE}, {"Name"="Stop LCD", "Time Stamp"=timestamp(3694475755.024133 s since 1904-01-01), "Code"="", "Source"="Init FPGA IO.vi", "Value"=11.0, "Boolean"=FALSE, "String"="", "Error"=FALSE, "Warning"=FALSE, " Fault"=FALSE}, {"Name"="wait", "Time Stamp"=timestamp(3694475754.021457 s since 1904-01-01), "Code"="", "Source"="Init FPGA IO.vi", "Value"=10.0, "Boolean"=FALSE, "String"="", "Error"=FALSE, "Warning"=FALSE, " Fault"=FALSE}, {"Name"="IP Address", "Time Stamp"=timestamp(3694475753.017004 s since 1904-01-01), "Code"="", "Source"="Init FPGA IO.vi", "Value"=12.0, "Boolean"=FALSE, "String"="þQ", "Error"=FALSE, "Warning"=FALSE, " Fault"=FALSE}, {"Name"="wait", "Time Stamp"=timestamp(3694475751.488638 s since 1904-01-01), "Code"="", "Source"="Init FPGA IO.vi", "Value"=10.0, "Boolean"=FALSE, "String"="", "Error"=FALSE, "Warning"=FALSE, " Fault"=FALSE}, {"Name"="Rev Display", "Time Stamp"=timestamp(3694475750.486358 s since 1904-01-01), "Code"="", "Source"="Init FPGA IO.vi", "Value"=9.0, "Boolean"=FALSE, "String"="Ver: CC 21.2.18.0", "Error"=FALSE, "Warning"=FALSE, " Fault"=FALSE}, {"Name"="wait", "Time Stamp"=timestamp(3694475750.438828 s since 1904-01-01), "Code"="", "Source"="Init FPGA IO.vi", "Value"=10.0, "Boolean"=FALSE, "String"="", "Error"=FALSE, "Warning"=FALSE, " Fault"=FALSE}, {"Name"="Chroma Display", "Time Stamp"=timestamp(3694475749.436896 s since 1904-01-01), "Code"="", "Source"="Init FPGA IO.vi", "Value"=8.0, "Boolean"=FALSE, "String"="Chroma ATE", "Error"=FALSE, "Warning"=FALSE, " Fault"=FALSE}, {"Name"="wait", "Time Stamp"=timestamp(3694475749.380093 s since 1904-01-01), "Code"="", "Source"="Init FPGA IO.vi", "Value"=10.0, "Boolean"=FALSE, "String"="", "Error"=FALSE, "Warning"=FALSE, " Fault"=FALSE}, {"Name"="Clear LCD Text", "Time Stamp"=timestamp(3694475748.377216 s since 1904-01-01), "Code"="", "Source"="Init FPGA IO.vi", "Value"=0.0, "Boolean"=FALSE, "String"="", "Error"=FALSE, "Warning"=FALSE, " Fault"=FALSE}, {"Name"="Mains Frequency", "Time Stamp"=timestamp(3694475748.302044 s since 1904-01-01), "Code"="", "Source"="Init FPGA", "Value"=199.09466455673416, "Boolean"=FALSE, "String"="", "Error"=FALSE, "Warning"=FALSE, " Fault"=FALSE}, {"Name"="BootLoad", "Time Stamp"=timestamp(3694475736.292084 s since 1904-01-01), "Code"="", "Source"="Init FPGA IO.vi", "Value"=0.0, "Boolean"=FALSE, "String"="", "Error"=FALSE, "Warning"=FALSE, " Fault"=FALSE}, {"Name"="Extra Settings Loaded", "Time Stamp"=timestamp(3694475735.407776 s since 1904-01-01), "Code"="", "Source"="", "Value"=0.0, "Boolean"=FALSE, "String"="", "Error"=FALSE, "Warning"=FALSE, " Fault"=FALSE}, {"Name"="Warmup ", "Time Stamp"=timestamp(3694475735.377503 s since 1904-01-01), "Code"="", "Source"="Extra Settings", "Value"=0.0, "Boolean"=FALSE, "String"="", "Error"=FALSE, "Warning"=TRUE, " Fault"=FALSE}, {"Name"="Heads Disabled", "Time Stamp"=timestamp(3694475735.35234 s since 1904-01-01), "Code"="", "Source"="Extra Settings", "Value"=0.0, "Boolean"=TRUE, "String"="", "Error"=FALSE, "Warning"=FALSE, " Fault"=FALSE}, {"Name"="Relative Humidity", "Time Stamp"=timestamp(3694475735.320859 s since 1904-01-01), "Code"="", "Source"="Extra Settings", "Value"=0.0, "Boolean"=TRUE, "String"="", "Error"=FALSE, "Warning"=FALSE, " Fault"=FALSE}, {"Name"="Warnings/Faults 1", "Time Stamp"=timestamp(3694475735.28331 s since 1904-01-01), "Code"="", "Source"="Extra Settings 3", "Value"=0.0, "Boolean"=TRUE, "String"="", "Error"=FALSE, "Warning"=FALSE, " Fault"=FALSE}, {"Name"="Read System Settings", "Time Stamp"=timestamp(3694475735.258281 s since 1904-01-01), "Code"="", "Source"="Read Extra Settings", "Value"=0.0, "Boolean"=FALSE, "String"="", "Error"=FALSE, "Warning"=TRUE, " Fault"=FALSE}, {"Name"="Config Loaded", "Time Stamp"=timestamp(3694475735.212652 s since 1904-01-01), "Code"="", "Source"="Config Read Initialize", "Value"=0.0, "Boolean"=FALSE, "String"="", "Error"=FALSE, "Warning"=FALSE, " Fault"=FALSE}, {"Name"="Config Read", "Time Stamp"=timestamp(3694475735.193427 s since 1904-01-01), "Code"="Found", "Source"="M2 T-Case Calibration", "Value"=1.0, "Boolean"=FALSE, "String"="Gain", "Error"=FALSE, "Warning"=FALSE, " Fault"=FALSE}, {"Name"="Config Read", "Time Stamp"=timestamp(3694475735.166672 s since 1904-01-01), "Code"="Found", "Source"="EEV PID", "Value"=100.0, "Boolean"=FALSE, "String"="Output Hi", "Error"=FALSE, "Warning"=FALSE, " Fault"=FALSE}, {"Name"="Config Read", "Time Stamp"=timestamp(3694475735.142093 s since 1904-01-01), "Code"="Found", "Source"="EEV PID", "Value"=50.0, "Boolean"=FALSE, "String"="SS Target", "Error"=FALSE, "Warning"=FALSE, " Fault"=FALSE}, {"Name"="Config Read", "Time Stamp"=timestamp(3694475735.119063 s since 1904-01-01), "Code"="Found", "Source"="M2 Heater PID", "Value"=0.0, "Boolean"=FALSE, "String"="Derivative Value", "Error"=FALSE, "Warning"=FALSE, " Fault"=FALSE}, {"Name"="Config Read", "Time Stamp"=timestamp(3694475735.103096 s since 1904-01-01), "Code"="Found", "Source"="Piston Settings", "Value"=500.0, "Boolean"=FALSE, "String"="Pressure Ramp Delay (ms)", "Error"=FALSE, "Warning"=FALSE, " Fault"=FALSE}, {"Name"="Config Value Read", "Time Stamp"=timestamp(3694475735.080325 s since 1904-01-01), "Code"="", "Source"="", "Value"=0.0, "Boolean"=TRUE, "String"="220V", "Error"=FALSE, "Warning"=FALSE, " Fault"=FALSE}] {"Value" format="%4.1f"; "Time Stamp" format="%<%x %.3X>T"}
  in  "Average Graph":bool
  in  "Pattern Directory":bool=TRUE
  in  "Change TSD":bool
  in  "Graph Temp Unit":bool
  out "M1 Valve Output":dbl(knob)=3.0777211191686598 scale=0.0..100.0
  out "M1 Buffer":dbl(slide)=0.999999999999999 scale=-4.0..4.0
  in  "Cascade Compressor controls":T15 {"Manual Low Stage frequency" min=40.0 max=150.0 step=1.0; "Manual High stage frequency" min=50.0 max=150.0 step=1.0}
  out "Shared Variable Address":string="//192.168.1.49/300"
  out "Detected Systems":string[](array[string])=["192.168.1.109 (NI-sbRIO-9651-Test)", "192.168.1.201 (Small-Conduit)", "192.168.1.49 (SeaCobra)", "192.168.2.15 (KingCobra115)", "192.168.2.16 (KingCobra116)", "192.168.2.5 (Gen3-DualHead)"]
  out "Data Rx Timestamp":timestamp=timestamp(3697404466.410487 s since 1904-01-01)
  out "Errors":string[](array[string])=["WARN:Low Amps  (21 02 20 18 55)"]
  out "Connected IP":string="192.168.1.49"
  out "TCP commands":string[](array[string])=["SOM STATUS()\r\n", "Wed 27 Jan 2021 09:30:06 PM PST"]
  out "bootup time":timestamp
  in  "SV Update Rate":i32=100
  out "CPU%":dbl=34.618222900110524 format="%#.1g"
  out "Free Memory (MB)":dbl=31.884
  out "Compressor Hours":dbl=49.38333333333333 format="%#.1f"
  out "SD card free Space":dbl=31885.0 format="%#.1p"
  out "M1 Superheat":dbl=1.7837896333833214 format="%#.1f"
  out "M1 Testing Elapsed Time":dbl format="%<%H:%M:%S>t"
  out "TSD Data":T16={"TSD Millivolts"=nan, "X factor"=1.0, "Offset"=0.0, "TSD Temp"=nan, "TSD Feedback"=FALSE, "TSD Max"=150.0, "TSD Min"=-60.0}
  in  "Autoscale graph":bool
  in  "Checkbox":bool
  in  "Checkbox 2":bool
  in  "M1 Heater output":dbl caption="M1 Heater PWM"
  in  "M1 EEV Manual":u16 caption="M1 EEV Manual control"
  out "TCP Connections":T17(array[cluster])=[{"port "=1300, "remote address"="", "Connection timeout ms"=100, "Waiting for connection"=TRUE, "Waiting for Command"=FALSE, "timeout ms"=5000}, {"port "=1100, "remote address"="", "Connection timeout ms"=100, "Waiting for connection"=TRUE, "Waiting for Command"=FALSE, "timeout ms"=-1}, {"port "=1000, "remote address"="", "Connection timeout ms"=100, "Waiting for connection"=TRUE, "Waiting for Command"=FALSE, "timeout ms"=60000}, {"port "=1001, "remote address"="", "Connection timeout ms"=100, "Waiting for connection"=TRUE, "Waiting for Command"=FALSE, "timeout ms"=60000}, {"port "=2100, "remote address"="", "Connection timeout ms"=100, "Waiting for connection"=FALSE, "Waiting for Command"=FALSE, "timeout ms"=-1}, {"port "=2001, "remote address"="", "Connection timeout ms"=100, "Waiting for connection"=FALSE, "Waiting for Command"=FALSE, "timeout ms"=60000}, {"port "=2000, "remote address"="", "Connection timeout ms"=100, "Waiting for connection"=FALSE, "Waiting for Command"=FALSE, "timeout ms"=5000}]
  out "M1 Head State":enum16{"Disabled", "Run", "Error"}(ring)
  out "GUI Version":string=" Cobra Single Head GUI V1.0\n\nModule Core.  This is the main VI for a new module. This module is self contained in that it can run on it's own without any other top level VIs. Alternatively you can call this VI from a top level VI and use it as an actor. By default the front panel will open.\n\nThe module will initialize itself with a default set of values. You can use the Initialize.VI to change those settings.  \n\nIf you would like to use the Rendezvous for syncronization call \"Initialize Rendezvous\". Just pass your rendezvous reference into it. \n" caption="Cobra GUI Version :"
  out "System Status":T18={"Power On Off"=FALSE, "Compressor Temp"=75.15781707316637, "Condensor Temp"=74.25781697779894, "Suction Temp"=73.93437944352627, "Ambient Temp"=73.76562942564487, "Sleep"=TRUE, "System Status"=enum."Sleep", "M1 Actuated"=FALSE, "Sleep Timer"=-1.0, "M1 Bin"={"Bin String"="", "Bin Color"=enum."White"}, "SW Version"="SW Version:CC 21.2.18.0"} {"Sleep Timer" format="%.1f"}
  in  "Command":string="VOLTAGE:AC 0"
  out "Response":string
  in  "Custom Command":bool caption="Send"
  in  "Boot Time out(s)":u32=4
  out "Boot Time(s)":u32=8
  in  "Y-axis range":dbl=5.0
  out "Infinite Profile":string caption="Infinite Cycle"
  out "Profile Time":dbl=4.911899089813232 caption="Time(sec)" format="%<%H:%M:%S>t"
  out "M1 Profile Channels":dbl[](array[numeric])=[24.0, 23.120361328125, 22.899678548177082, nan, 0.0] format="%#.1f"
  in  "Channels":T19(array[cluster])=[{"Channel Name"="M1 Setpoint", "Color Box"=0, "Run"=FALSE, "Axis"=1, "Unit"="°C"}, {"Channel Name"="M1 Case Temp", "Color Box"=16860, "Run"=FALSE, "Axis"=1, "Unit"="°C"}, {"Channel Name"="M1 Evap Temp", "Color Box"=16768042, "Run"=FALSE, "Axis"=1, "Unit"="°C"}, {"Channel Name"="M1 TSD", "Color Box"=11809792, "Run"=FALSE, "Axis"=1, "Unit"="°C"}, {"Channel Name"="M1 AC Load", "Color Box"=6618880, "Run"=FALSE, "Axis"=0, "Unit"="W"}] {"Axis" items=["Y1", "Y2"]}
  out "Profile Chart":waveform(dbl)[](graph)=[{"t0"=timestamp(3699375123.743896 s since 1904-01-01), "dt"=1.0, "Y"=[25.0, 25.0, 25.0, 25.0, 25.0, 25.0, 25.0, 25.0, 25.0, 25.0, 25.0, 25.0, 25.0, 25.0, 25.0, 25.0, 25.0, 25.0, 25.0, 25.0, 25.0, 25.0, 25.0, 25.0, 25.0, 25.0, 25.0, 25.0, 25.0, 25.0, 25.0, 25.0, 25.0, 25.0, 25.0, 25.0, 25.0, 25.0, 25.0, 25.0, 25.0, 25.0, 25.0, 25.0, 25.0, 25.0, 25.0, 25.0, 25.0, 25.0, 25.0, 25.0, 25.0, 25.0, 25.0, 25.0, 25.0, 25.0, 25.0, 25.0, 25.0, 25.0, 25.0, 25.0, 25.0, 25.0, 25.0, 25.0, 25.0, 25.0, 25.0, 25.0, 25.0, 25.0, 25.0, 25.0, 25.0, 25.0, 25.0, 25.0, 25.0, 25.0, 25.0, 25.0, 25.0, 25.0, 25.0, 25.0, 25.0, 25.0, 25.0, 25.0, 25.0, 25.0, 25.0, 25.0, 25.0, 25.0, 25.0, 25.0, 25.0, 25.0, 25.0, 25.0, 25.0, 25.0, 25.0, 25.0, 25.0, 25.0, 25.0, 25.0, 25.0, 25.0, 25.0, 25.0, 25.0, 25.0, 25.0, 25.0, 25.0, 25.0, 25.0, 25.0, 25.0, 25.0, 25.0, 25.0, 25.0, 25.0, 25.0, 25.0, 25.0, 25.0, 25.0, 25.0, 25.0, 25.0, 25.0, 25.0, 25.0, 25.0, 25.0, 24.0, 24.0, 24.0, 24.0, 24.0, 24.0, 24.0, 24.0, 24.0, 24.0, 24.0, 24.0, 24.0, 24.0, 24.0, 24.0, 24.0, 24.0, 24.0, 24.0, 24.0, 24.0, 24.0, 24.0, 24.0, 24.0, 24.0, 24.0, 24.0, 24.0, 24.0, 24.0, 24.0, 24.0, 24.0, 24.0, 24.0, 24.0, 24.0, 24.0, 24.0, 24.0, 24.0, 24.0, 24.0, 24.0, 24.0, 24.0, 24.0, 24.0, 24.0, 24.0, 24.0, 24.0, 24.0, 24.0, 24.0, 24.0, 24.0, 24.0, 24.0, 24.0, 24.0, 24.0, 24.0, 24.0, 24.0, 24.0, 24.0, 24.0, 24.0, 24.0, 24.0, 24.0, 24.0, 24.0, 24.0, 24.0, 24.0, 24.0, 24.0, 24.0, 24.0, 24.0, 24.0, 24.0, 24.0, 24.0, 24.0, 24.0, 24.0, 24.0, 24.0, 24.0, 24.0, 24.0, 24.0, 24.0, 24.0, 24.0, 24.0, 24.0, 24.0, 24.0, 24.0, 24.0, 24.0, 24.0, 24.0, 24.0, 24.0, 24.0, 24.0, 24.0, 24.0, 24.0, 24.0, 24.0, 24.0, 24.0, 24.0, 24.0, 24.0, 24.0, 24.0, 24.0, 24.0, 24.0, 24.0, 24.0, 24.0, 24.0, 24.0, 24.0, 24.0, 24.0, 24.0, 24.0, 24.0, 24.0, 24.0, 24.0, 24.0, 24.0, 24.0, 24.0, 24.0, 24.0, 24.0, 24.0, 24.0, 24.0, 24.0, 24.0, 24.0, 24.0, 24.0, 24.0, 24.0, 24.0, 24.0, 24.0, 24.0, 24.0, 24.0, 24.0, 24.0, 24.0, 24.0, 24.0, 24.0, 24.0, 24.0, 24.0, 24.0, 24.0, 24.0, 24.0, 24.0, 24.0, 24.0, 24.0, 24.0, 24.0, 24.0, 24.0, 24.0, 24.0, 24.0, 24.0, 24.0, 24.0, 24.0, 24.0, 24.0, 24.0, 24.0, 24.0, 24.0, 24.0, 24.0, 24.0, 24.0, 24.0, 24.0, 24.0, 24.0, 24.0, 24.0, 24.0, 24.0, 24.0, 24.0, 24.0, 24.0, 24.0, 24.0, 24.0, 24.0, 24.0, 24.0, 24.0, 24.0, 24.0, 24.0, 24.0, 24.0, 24.0, 24.0, 24.0, 24.0, 24.0, 24.0, 24.0, 24.0, 24.0, 24.0, 24.0, 24.0, 24.0, 24.0]}, {"t0"=timestamp(3699375123.743896 s since 1904-01-01), "dt"=1.0, "Y"=array[384 elements]}, {"t0"=timestamp(3699375123.743896 s since 1904-01-01), "dt"=1.0, "Y"=array[384 elements]}, {"t0"=timestamp(3699375123.743896 s since 1904-01-01), "dt"=1.0, "Y"=[nan, nan, nan, nan, nan, nan, nan, nan, nan, nan, nan, nan, nan, nan, nan, nan, nan, nan, nan, nan, nan, nan, nan, nan, nan, nan, nan, nan, nan, nan, nan, nan, nan, nan, nan, nan, nan, nan, nan, nan, nan, nan, nan, nan, nan, nan, nan, nan, nan, nan, nan, nan, nan, nan, nan, nan, nan, nan, nan, nan, nan, nan, nan, nan, nan, nan, nan, nan, nan, nan, nan, nan, nan, nan, nan, nan, nan, nan, nan, nan, nan, nan, nan, nan, nan, nan, nan, nan, nan, nan, nan, nan, nan, nan, nan, nan, nan, nan, nan, nan, nan, nan, nan, nan, nan, nan, nan, nan, nan, nan, nan, nan, nan, nan, nan, nan, nan, nan, nan, nan, nan, nan, nan, nan, nan, nan, nan, nan, nan, nan, nan, nan, nan, nan, nan, nan, nan, nan, nan, nan, nan, nan, nan, nan, nan, nan, nan, nan, nan, nan, nan, nan, nan, nan, nan, nan, nan, nan, nan, nan, nan, nan, nan, nan, nan, nan, nan, nan, nan, nan, nan, nan, nan, nan, nan, nan, nan, nan, nan, nan, nan, nan, nan, nan, nan, nan, nan, nan, nan, nan, nan, nan, nan, nan, nan, nan, nan, nan, nan, nan, nan, nan, nan, nan, nan, nan, nan, nan, nan, nan, nan, nan, nan, nan, nan, nan, nan, nan, nan, nan, nan, nan, nan, nan, nan, nan, nan, nan, nan, nan, nan, nan, nan, nan, nan, nan, nan, nan, nan, nan, nan, nan, nan, nan, nan, nan, nan, nan, nan, nan, nan, nan, nan, nan, nan, nan, nan, nan, nan, nan, nan, nan, nan, nan, nan, nan, nan, nan, nan, nan, nan, nan, nan, nan, nan, nan, nan, nan, nan, nan, nan, nan, nan, nan, nan, nan, nan, nan, nan, nan, nan, nan, nan, nan, nan, nan, nan, nan, nan, nan, nan, nan, nan, nan, nan, nan, nan, nan, nan, nan, nan, nan, nan, nan, nan, nan, nan, nan, nan, nan, nan, nan, nan, nan, nan, nan, nan, nan, nan, nan, nan, nan, nan, nan, nan, nan, nan, nan, nan, nan, nan, nan, nan, nan, nan, nan, nan, nan, nan, nan, nan, nan, nan, nan, nan, nan, nan, nan, nan, nan, nan, nan, nan, nan, nan, nan, nan, nan, nan, nan, nan, nan, nan, nan, nan, nan, nan, nan, nan, nan, nan, nan, nan, nan]}, {"t0"=timestamp(3699375123.743896 s since 1904-01-01), "dt"=1.0, "Y"=[0.0, 0.0, 0.0, 0.0, 0.0, 0.0, 0.0, 0.0, 0.0, 0.0, 0.0, 0.0, 0.0, 0.0, 0.0, 0.0, 0.0, 0.0, 0.0, 0.0, 0.0, 0.0, 0.0, 0.0, 0.0, 0.0, 0.0, 0.0, 0.0, 0.0, 0.0, 0.0, 0.0, 0.0, 0.0, 0.0, 0.0, 0.0, 0.0, 0.0, 0.0, 0.0, 0.0, 0.0, 0.0, 0.0, 0.0, 0.0, 0.0, 0.0, 0.0, 0.0, 0.0, 0.0, 0.0, 0.0, 0.0, 0.0, 0.0, 0.0, 0.0, 0.0, 0.0, 0.0, 0.0, 0.0, 0.0, 0.0, 0.0, 0.0, 0.0, 0.0, 0.0, 0.0, 0.0, 0.0, 0.0, 0.0, 0.0, 0.0, 0.0, 0.0, 0.0, 0.0, 0.0, 0.0, 0.0, 0.0, 0.0, 0.0, 0.0, 0.0, 0.0, 0.0, 0.0, 0.0, 0.0, 0.0, 0.0, 0.0, 0.0, 0.0, 0.0, 0.0, 0.0, 0.0, 0.0, 0.0, 0.0, 0.0, 0.0, 0.0, 0.0, 0.0, 0.0, 0.0, 0.0, 0.0, 0.0, 0.0, 0.0, 0.0, 0.0, 0.0, 0.0, 0.0, 0.0, 0.0, 0.0, 0.0, 0.0, 0.0, 0.0, 0.0, 0.0, 0.0, 0.0, 0.0, 0.0, 0.0, 0.0, 0.0, 0.0, 0.0, 0.0, 0.0, 0.0, 0.0, 0.0, 0.0, 0.0, 0.0, 0.0, 0.0, 0.0, 0.0, 0.0, 0.0, 0.0, 0.0, 0.0, 0.0, 0.0, 0.0, 0.0, 0.0, 0.0, 0.0, 0.0, 0.0, 0.0, 0.0, 0.0, 0.0, 0.0, 0.0, 0.0, 0.0, 0.0, 0.0, 0.0, 0.0, 0.0, 0.0, 0.0, 0.0, 0.0, 0.0, 0.0, 0.0, 0.0, 0.0, 0.0, 0.0, 0.0, 0.0, 0.0, 0.0, 0.0, 0.0, 0.0, 0.0, 0.0, 0.0, 0.0, 0.0, 0.0, 0.0, 0.0, 0.0, 0.0, 0.0, 0.0, 0.0, 0.0, 0.0, 0.0, 0.0, 0.0, 0.0, 0.0, 0.0, 0.0, 0.0, 0.0, 0.0, 0.0, 0.0, 0.0, 0.0, 0.0, 0.0, 0.0, 0.0, 0.0, 0.0, 0.0, 0.0, 0.0, 0.0, 0.0, 0.0, 0.0, 0.0, 0.0, 0.0, 0.0, 0.0, 0.0, 0.0, 0.0, 0.0, 0.0, 0.0, 0.0, 0.0, 0.0, 0.0, 0.0, 0.0, 0.0, 0.0, 0.0, 0.0, 0.0, 0.0, 0.0, 0.0, 0.0, 0.0, 0.0, 0.0, 0.0, 0.0, 0.0, 0.0, 0.0, 0.0, 0.0, 0.0, 0.0, 0.0, 0.0, 0.0, 0.0, 0.0, 0.0, 0.0, 0.0, 0.0, 0.0, 0.0, 0.0, 0.0, 0.0, 0.0, 0.0, 0.0, 0.0, 0.0, 0.0, 0.0, 0.0, 0.0, 0.0, 0.0, 0.0, 0.0, 0.0, 0.0, 0.0, 0.0, 0.0, 0.0, 0.0, 0.0, 0.0, 0.0, 0.0, 0.0, 0.0, 0.0, 0.0, 0.0, 0.0, 0.0, 0.0, 0.0, 0.0, 0.0, 0.0, 0.0, 0.0, 0.0, 0.0, 0.0, 0.0, 0.0, 0.0, 0.0, 0.0, 0.0, 0.0, 0.0, 0.0, 0.0, 0.0, 0.0, 0.0, 0.0, 0.0, 0.0, 0.0, 0.0, 0.0, 0.0, 0.0, 0.0, 0.0, 0.0, 0.0, 0.0, 0.0, 0.0, 0.0, 0.0, 0.0, 0.0, 0.0, 0.0, 0.0, 0.0, 0.0, 0.0, 0.0, 0.0, 0.0, 0.0, 0.0, 0.0, 0.0, 0.0, 0.0, 0.0]}]
  in  "Reset Profile":bool
  in  "Stop Profile":bool
  in  "Start Profile":bool
  in  "Profile Info":T20 {"dt" format="%<%H:%M:%S>t"; "Duration" format="%<%H:%M:%S>t"}
  out "Temp Pattern":waveform(dbl)(graph)
  out "Nv Power":waveform(dbl)[](graph)=[{"t0"=timestamp(3699375123.7807975 s since 1904-01-01), "dt"=1.0, "Y"=[5.0]}, {"t0"=timestamp(3699375123.7807975 s since 1904-01-01), "dt"=1.0, "Y"=[5.0]}, {"t0"=timestamp(3699375123.7807975 s since 1904-01-01), "dt"=1.0, "Y"=[1625.0]}]
  out "Nv Voltage":dbl=5.0
  out "Nv Current":dbl=5.0
  out "Cycle":i32=1
  in  "Iteration No":i32=2 caption="Head Load(W)"
  out "Infinite Test":string caption="Infinite Cycle"
  in  "Reset Test":bool
  in  "Stop Test":bool
  in  "Start Test":bool
  in  "Serial Port":string(combo)="COM5" caption="Default Pattern Folder"
  in  "Power":bool caption="Test/Stop"
  in  "Power Seq":T21=[{"Duration"=0, "Head Load(W)"=0, "Name"="Step1"}, {"Duration"=10, "Head Load(W)"=0, "Name"="Step2"}, {"Duration"=10, "Head Load(W)"=0, "Name"="Step3"}, {"Duration"=20, "Head Load(W)"=0, "Name"="Step4"}, {"Duration"=20, "Head Load(W)"=0, "Name"="Step5"}, {"Duration"=30, "Head Load(W)"=0, "Name"="Step6"}, {"Duration"=30, "Head Load(W)"=0, "Name"="Step7"}, {"Duration"=40, "Head Load(W)"=0, "Name"="Step8"}, {"Duration"=40, "Head Load(W)"=0, "Name"="Step9"}, {"Duration"=50, "Head Load(W)"=0, "Name"="Step10"}]
  in  "Pattern File":string(combo)="S1.ini" caption="Default Pattern Folder"
  in  "Seq Controls":T22
  out "Time":dbl caption="Time(sec)" format="%<%H:%M:%S>t"
  out "TTV Power":dbl=nan format="%.1g"
  out "Test Graph":dbl[](graph)
  out "Step":string
  # "AC PS Serial Protocol"
  # "AC Power Supply"
  # "on"
  # "W"
  # "Step"
  # "Duration"
  # "Heat Load(W)"
  # "off"
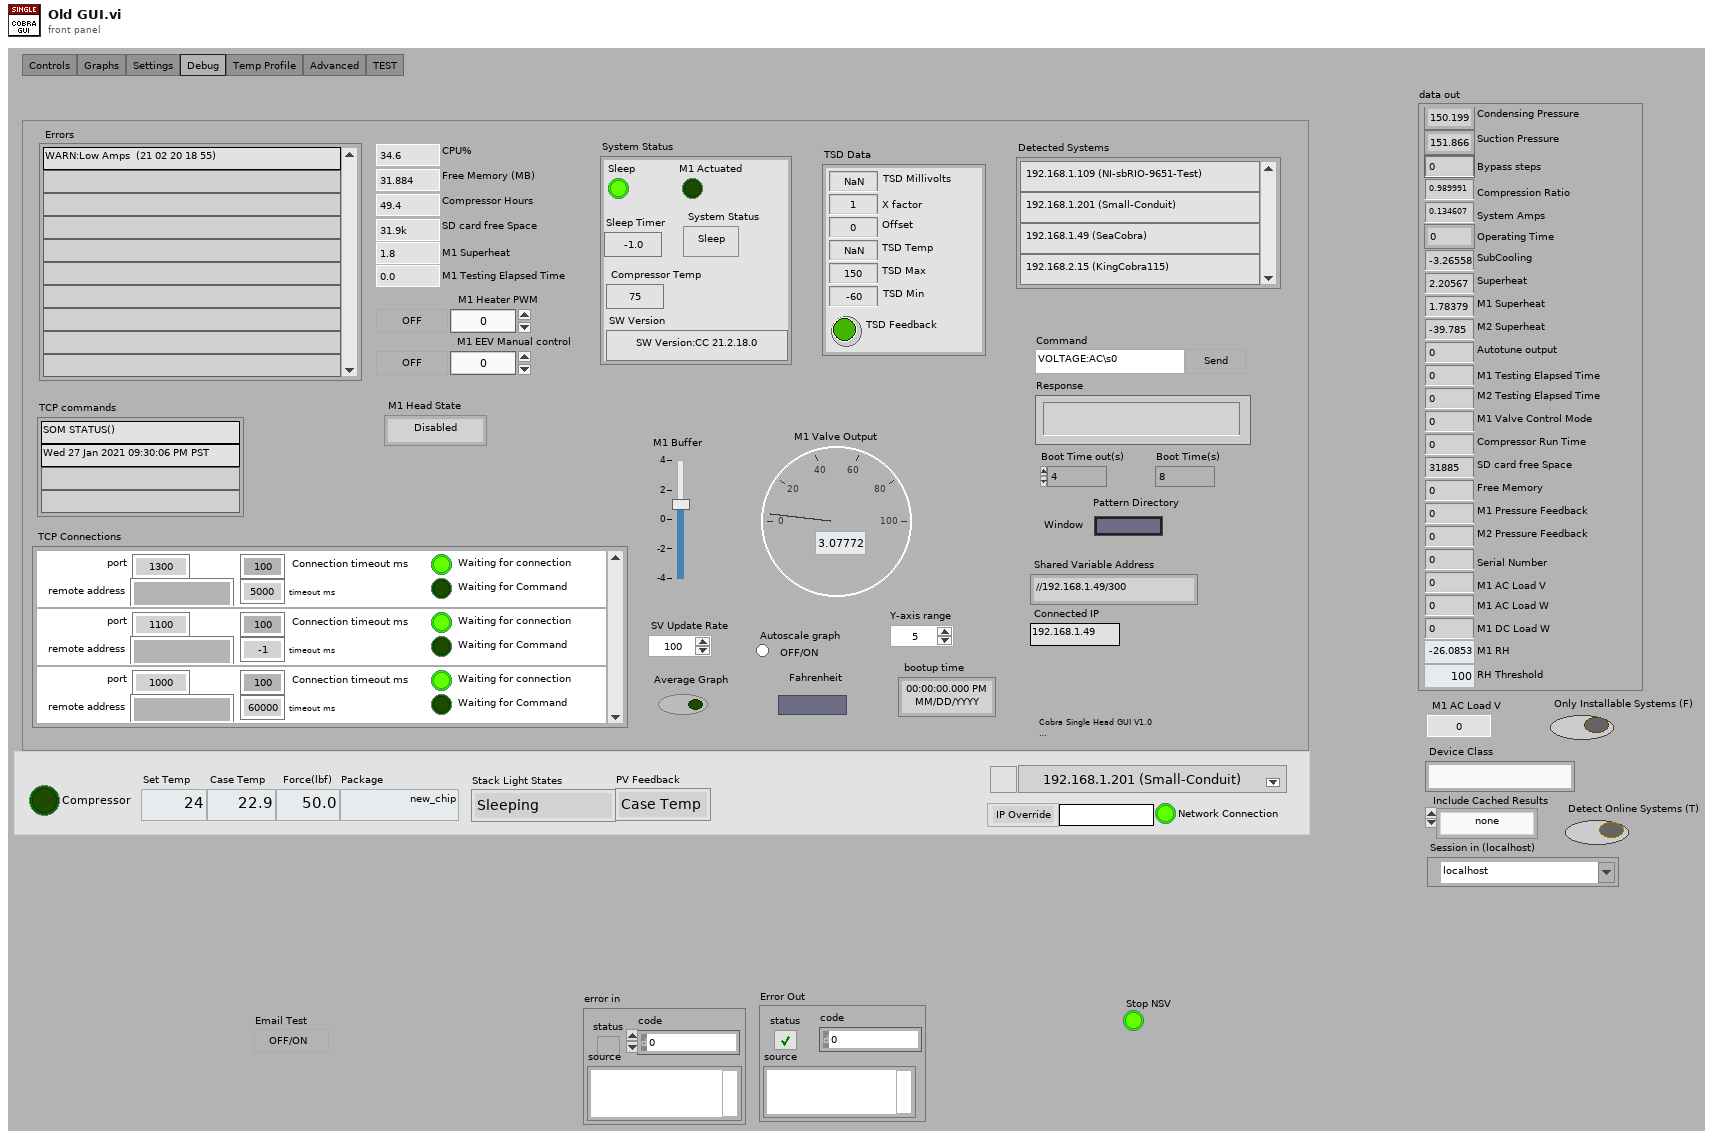
[diagram p1: front panel]
types:
  T1 = enum16{"Sleeping", "Warming up", "Ready", "Testing", "Restless", "Idle", "Sleeping Fault", "warning"}
  T2 = cluster{"Condensing Pressure":dbl, "Suction Pressure":dbl, "Bypass steps":u16, "Operating Time":dbl, "SubCooling":dbl, "Superheat":dbl, "M1 Superheat":dbl, "M2 Superheat":dbl, "Autotune output":dbl, "M1 Testing Elapsed Time":dbl, "M2 Testing Elapsed Time":dbl, "M1 Valve Control Mode":u8, "System Amps":dbl, "Compressor Run Time":dbl, "SD card free Space":dbl, "Free Memory":dbl, "M1 Pressure Feedback":dbl, "M2 Pressure Feedback":dbl, "Compression Ratio":dbl, "Serial Number":dbl, "M1 AC Load V":dbl, "M1 AC Load W":dbl, "M1 DC Load W":dbl, "M1 RH":dbl, "RH Threshold":dbl}
  T3 = enum32{"Controls", "Graphs", "Settings", "Debug", "Temp Profile", "Advanced", "TEST"}
  T4 = cluster{"Case Temp":dbl, "Evap Temp":dbl, "Heater %":dbl, "EEV Steps":u32, "Set Temp":dbl, "Feedback":u8, "Power Drive":bool, "Piston Volts":dbl, "Safe Temp":bool, "Power":bool, "Thermal State":enum16{"Ramp Up", "Ramp Down", "Steady State", "Ebb and Flow"}, "Error":bool, "In tollerance":bool, "Head State":enum16{"Disabled", "Run", "Error"}, "Piston Force":dbl, "Package":string}
  T5 = cluster{"M1 Feedback":u16, "M1 Package":u16, "M1 Enable":bool, "M1 Set Temp":dbl}
  T6 = enum16{"Ramp Up", "Ramp Down", "Steady State", "Ebb and Flow", "Up", "Under Load", "Cryo Mode"}
  T7 = typedef "GUI.lvlib/System Graphs.ctl" = cluster{"Ambient Temp":dbl, "Suction Temp":dbl, "Condensor Temp":dbl, "Discharge Temp":dbl, "Bypass Steps":dbl}
  T8 = typedef "GUI.lvlib/Module Graphs.ctl" = cluster{"Case Temp":dbl, "Evap Temp":dbl, "Heater Power (%)":dbl, "EEV Steps":dbl, "M1 AC Load(W)":dbl}
  T9 = typedef "GUI.lvlib/Dial Gauges.ctl" = cluster{"Condensing Pressure(psi)":dbl, "Compression Ratio":T10, "Subcool":T11, "Superheat":T12, "Current(A)":T13, "Suction Pressure(psi)":dbl}
  T10 = typedef "GUI.lvlib/Compression Ratio.ctl" = dbl
  T11 = typedef "GUI.lvlib/Subcooling.ctl" = dbl
  T12 = typedef "GUI.lvlib/Superheat.ctl" = dbl
  T13 = typedef "GUI.lvlib/Current.ctl" = dbl
  T14 = cluster{"Name":string, "Time Stamp":timestamp, "Code":string, "Source":string, "Value":dbl, "Boolean":bool, "String":string, "Error":bool, "Warning":bool, " Fault":bool}[]
  T15 = cluster{"High Stage manual speed control":bool, "Manual High stage frequency":dbl, "Low Stage manual speed control":bool, "Manual Low Stage frequency":dbl}
  T16 = cluster{"TSD Millivolts":dbl, "X factor":dbl, "Offset":dbl, "TSD Temp":dbl, "TSD Feedback":bool, "TSD Max":dbl, "TSD Min":dbl}
  T17 = cluster{"port ":u16, "remote address":string, "Connection timeout ms":i32, "Waiting for connection":bool, "Waiting for Command":bool, "timeout ms":i32}[]
  T18 = cluster{"Power On Off":bool, "Compressor Temp":dbl, "Condensor Temp":dbl, "Suction Temp":dbl, "Ambient Temp":dbl, "Sleep":bool, "System Status":enum16{"Sleep", "Run"}, "M1 Actuated":bool, "Sleep Timer":dbl, "M1 Bin":cluster{"Bin String":string, "Bin Color":enum16{"Black", "White", "Red", "Green", "Blue", "Cyan", "Amber"}}, "SW Version":string}
  T19 = cluster{"Channel Name":string, "Color Box":u32, "Run":bool, "Axis":u32, "Unit":string}[]
  T20 = cluster{"Start Temp":dbl, "End Temp":dbl, "Duration":dbl, "dt":dbl, "Iteration":i32}
  T21 = typedef "GUI.lvlib/Profile Sequence.ctl" = cluster{"Duration":i32, "Head Load(W)":u32, "Name":string}[]
  T22 = cluster{"Refresh Seq":bool, "Save Seq":bool, "Delete Seq":bool, "Clear Seq":bool}
  T23 = typedef "GUI.lvlib/NSV States.ctl" = enum16{"Init", "Run", "Exit"}
  T24 = typedef "GUI.lvlib/GUI Variables.ctl" = cluster{"Core":cluster{"Current VI":refnum<vi>, "Close Panel on Exit?":bool, "VI Name":string, "VI Path":path}, "Log?":bool, "Current Case":string, "Shared Variable Address":string, "reader endpoint":refnum<k21>, "writer endpoint":refnum<k21>, "Detected Systems":string[], "IP Address":string, "Network Connection":bool, "URI Directory":string, "File list in SoM":string[], "System State":enum16{"Idle", "Running"}, "TTV Test":cluster{"Power Seq":T21, "PS Connection":bool, "OutputState":bool, "Step":i32, "Current Cycle":i32}, "Profile":cluster{"Profile Temp":bool, "Current Cycle":i32}, "M1 History Temps":dbl[][], "M2 History Temps":dbl[][], "M1 Bootup":bool, "M2 Bootup":bool, "Network Data Down":T25, "Event Log":T27[], "Login":bool, "Connected System":string, "TCP connection info":T28, "TCP Connection":bool, "Dataset":T30}
  T25 = typedef "GUI.lvlib/Network Data Down_set back.ctl" = cluster{"M1 Commands":cluster{"Set Temp":dbl, "Power Drive":bool, "Feedback":u8, "Package":u16, "Enable":bool}, "M2 Commands":cluster{"Set Temp":dbl, "Power Drive":bool, "Feedback":u8, "Package ":u16, "Enable":bool}, "Config Data":cluster{"Packages":cluster{"DUT Force lbf":cluster{" 0":u32, " 1":u32, " 2":u32, "3":u32, "4":u32, "5":u32, " 6":u32, "7":u32, "8":u32, "9":u32}, "DUT Names":cluster{"0":string, "1":string, "2":string, "3":string, "4":string, "5":string, "6":string, "7":string, "8":string, "9":string}}, "Heater PID":cluster{"P":dbl, "I":dbl, "D":dbl}, "Piston Settings":cluster{"Forces Slope":dbl, "Forces Intercept":dbl, "Transition Force":dbl, "Up Force":dbl, "Diameter (mm)":dbl, "Delay (ms)":dbl, "Pressure Ramp Delay (ms)":dbl}, "Safe Temps":cluster{"Minimum":i32, "Enabled":bool, "Maximum":i32}, "System Settings":cluster{"Number of Heads":i32, "60Hz Power":bool, "FTC200":bool, "AutoStartup":bool, "Purge":bool, "Sensors":bool, "HandClamp":bool, "ATE":bool, "Benchtop":bool, "Production":bool, "Refrigerant":enum16{"r404a", "r507", "r508", "r410a", "r134a"}, "Handler":bool, "Shuttle":bool, "220V":bool, "Cascade":bool, "Suction Sensor":enum16{"YCQB02H01", "YCQB02L01", "Carel"}, "Discharge Sensor":enum16{"YCQB05H01", "YCQB05L01", "Carel"}}, "Stepper Settings ":cluster{"Microstepping":enum16{"Full", "Half", "Quarter", "1/16th"}, "Velocity":u8}, "Set Point Range":cluster{"Max":dbl, "Min":dbl}, "Pedestal Check DeltaT":dbl, "Ramp Delta T":dbl, "Ramp-SS Threshold":dbl, "SS Tolerance":dbl, "EEV PID":cluster{"Ramp Up Target":dbl, "Ramp Down Target":dbl, "Steady State Target":dbl, "Output":cluster{"Max":dbl, "Min":dbl}, "EBB and Flow Temp TH":dbl, "Cryomode EEV Max":dbl, "Valve minimum opening ":dbl, "Ramp Up EEV Steps":dbl, "Ramp Down EEV Steps":dbl, "SS EEV Steps Reset":dbl, "EBB and Flow Tol":dbl, "Gains":cluster{"P":dbl, "I":dbl, "D":dbl}, "Dissabled Target":dbl, "CryoMode Gains":cluster{"P":dbl, "I":dbl, "D":dbl}, "M1 SuperHeat Setpoint":dbl, "M2 Gains":cluster{"P":dbl, "I":dbl, "D":dbl}, "Flow Curve":enum16{""}}, "Sleep Timeout":dbl, "Bypass Values":cluster{"Bypass Valve":bool, "Flow Curve":enum16{"0", "1"}, "Output":cluster{"Max":u32, "Min":u32}, "Feedback":enum16{"Temperature", "Pressure", "Superheat", "Pressure 2.0"}, "Cyth Bypass":bool, "PID":cluster{"P":dbl, "I":dbl, "D":dbl}, "Pressure setpoint":i16, "Cryo Temp":i16, "Superheat Setpoint":i16, "Cryo Setpoint":i16}, "Default Temp":dbl, "InTEC":cluster{"Enabled":bool, "IP":string, "Port":u16}, "M1 TSD":cluster{"Gain":dbl, "Offset":dbl, "V Offset ":dbl}, "M2 TSD":cluster{"Gain":dbl, "Offset":dbl, "V Offset ":dbl}, "M1 T-Case Calibration":cluster{"Gain":dbl, "Offset":dbl}, "M2 T-Case Calibration":cluster{"Gain":dbl, "Offset":dbl}, "Heater PID TSD":cluster{"P":dbl, "I":dbl, "D":dbl}, "M2 Heater PID":cluster{"P":dbl, "I":dbl, "D":dbl}}, "System Power On Off":bool, "New Data":T26, "Stop RT":bool}
  T26 = typedef "GUI.lvlib/NS New Data.ctl" = enum16{"M1 Set Point", "M1 Power Drive", "M1 Feedback", "M1 Package", "M1 Enable", "M2 Set Point", "M2 Power Drive", "M2 Feedback", "M2 Package", "M2 Enable", "System Power", "Config Data", "Stop RT"}
  T27 = typedef "GUI.lvlib/Event.ctl" = cluster{"Name":string, "Time Stamp":timestamp, "Code":i32, "Source":string, "Value":string, "Boolean":bool, "Description":string, "Error":bool, "Warning":bool, " Fault":bool}
  T28 = typedef "NI STM.lvlib/TCP Connection Info.ctl" = cluster{"connection ID":refnum<k5>, "meta data":T29[]}
  T29 = typedef "NI STM.lvlib/MetaDataElement.ctl" = string
  T30 = typedef "GUI.lvlib/Dataset.ctl" = cluster{"System Status":T31, "M1 Status":T32, "M2 Status":T33, "Config Data":T34}
  T31 = typedef "GUI.lvlib/System Status.ctl" = cluster{"Power On Off":bool, "Discharge Temp":dbl, "Liquid Temp":dbl, "Suction Temp":dbl, "Ambient Temp":dbl, "Sleep":bool, "System Status":u16, "M1 Actuated":bool, "M2 Actuated":bool, "Sleep Timer":dbl, "M1 Bin":cluster{"Bin String":string, "Bin Color":u16}, "M2 Bin":cluster{"Bin String":string, "Bin Color":u16}, "Discharge Pressure":dbl, "Suction Pressure":dbl, "Compression Ratio":dbl, "Compressor Amps":dbl, "Compressor Hours":dbl, "Bypass Steps":u16, "SubCooling":dbl, "SuperHeat":dbl, "Serial Number":string, "EMO detected":bool, "EMO Tripped":bool, "Thermal cutoff":bool, "Thermal cutoff 2":bool, "High Pressure switch":bool, "Running Time":timestamp, "SOM Status":cluster{"Boot Up Time":timestamp, "Software Version":string, "CPU Usage":dbl, "Memory Available":dbl, "SD card free space":dbl, "SOM Storage":dbl}, "Cascade Extra":cluster{"Discharge Temp High Side":dbl, "Suction Temp High Side":dbl, "Liquid Temp High side":dbl, "Discharge Pressure 2":dbl, "Suction Pressure 2":dbl, "Low Side RPM":dbl, "High Side RPM":dbl}}
  T32 = typedef "GUI.lvlib/Module Status.ctl" = cluster{"Case Temp":dbl, "Evap Temp":dbl, "Heater %":dbl, "EEV Steps":u32, "Set Temp":dbl, "Feedback":u8, "Power Drive":bool, "Piston Volts":dbl, "Safe Temp":bool, "Power":bool, "Thermal State":u16, "Error":bool, "In tollerance":bool, "Head State":u16, "Piston Force":dbl, "Package":string, "Dynamic SV":dbl, "PV":dbl, "TSD Temp":dbl, "DC Load Watts":dbl, "AC Load Watts":dbl, "Intec Feedback":dbl}
  T33 = typedef "GUI.lvlib/M2 Status.ctl" = cluster{"Case Temp":dbl, "Evap Temp":dbl, "Heater %":dbl, "EEV Steps":u32, "Set Temp":dbl, "Feedback":u8, "Power Drive":bool, "Piston Volts":dbl, "Safe Temp":bool, "Power":bool, "Thermal State":u16, "Error":bool, "In tollerance":bool, "Head State":u16, "Piston Force":dbl, "Package":string, "PV":dbl, "Dynamic SV":dbl, "TSD":dbl, "AC Load Watts":dbl}
  T34 = typedef "GUI.lvlib/Config Data.ctl" = cluster{"Packages":cluster{"DUT Force lbf":cluster{" 0":u32, " 1":u32, " 2":u32, "3":u32, "4":u32, "5":u32, " 6":u32, "7":u32, "8":u32, "9":u32}, "DUT Names":cluster{"0":string, "1":string, "2":string, "3":string, "4":string, "5":string, "6":string, "7":string, "8":string, "9":string}}, "Heater PID":cluster{"P":dbl, "I":dbl, "D":dbl}, "Piston Settings":cluster{"Forces Slope":dbl, "Forces Intercept":dbl, "Transition Force":dbl, "Up Force":dbl, "Diameter (mm)":dbl, "Delay (ms)":dbl, "Pressure Ramp Delay (ms)":dbl}, "Safe Temps":cluster{"Minimum":i32, "Enabled":bool, "Maximum":i32}, "System Settings":cluster{"Number of Heads":i32, "60Hz Power":bool, "FTC200":bool, "AutoStartup":bool, "Purge":bool, "Sensors":bool, "HandClamp":bool, "ATE":bool, "Benchtop":bool, "Production":bool, "Refrigerant":u16, "Handler":bool, "Shuttle":bool, "220V":bool, "Cascade":bool, "Suction Sensor":u16, "Discharge Sensor":u16}, "Stepper Settings ":cluster{"Microstepping":u16, "Velocity":u8}, "Set Point Range":cluster{"Max":dbl, "Min":dbl}, "Pedestal Check DeltaT":dbl, "Ramp Delta T":dbl, "Ramp-SS Threshold":dbl, "SS Tolerance":dbl, "EEV PID":cluster{"Ramp Up Target":dbl, "Ramp Down Target":dbl, "Steady State Target":dbl, "Output":cluster{"Max":dbl, "Min":dbl}, "EBB and Flow Temp TH":dbl, "Cryomode EEV Max":dbl, "Valve minimum opening ":dbl, "Ramp Up EEV Steps":dbl, "Ramp Down EEV Steps":dbl, "SS EEV Steps Reset":dbl, "EBB and Flow Tol":dbl, "Gains":cluster{"P":dbl, "I":dbl, "D":dbl}, "Dissabled Target":dbl, "CryoMode Gains":cluster{"P":dbl, "I":dbl, "D":dbl}, "M1 SuperHeat Setpoint":dbl, "M2 Gains":cluster{"P":dbl, "I":dbl, "D":dbl}, "Flow Curve":u16}, "Sleep Timeout":dbl, "Bypass Values":cluster{"Bypass Valve":bool, "Flow Curve":u16, "Output":cluster{"Max":u32, "Min":u32}, "Feedback":u16, "Cyth Bypass":bool, "PID":cluster{"P":dbl, "I":dbl, "D":dbl}, "Pressure setpoint":i16, "Cryo Temp":i16, "Superheat Setpoint":i16, "Cryo Setpoint":i16}, "Default Temp":dbl, "InTEC":cluster{"Enabled":bool, "IP":string, "Port":u16}, "M1 TSD":cluster{"Gain":dbl, "Offset":dbl, "V Offset ":dbl}, "M2 TSD":cluster{"Gain":dbl, "Offset":dbl, "V Offset ":dbl}, "M1 T-Case Calibration":cluster{"Gain":dbl, "Offset":dbl}, "M2 T-Case Calibration":cluster{"Gain":dbl, "Offset":dbl}, "Heater PID TSD":cluster{"P":dbl, "I":dbl, "D":dbl}, "M2 Heater PID":cluster{"P":dbl, "I":dbl, "D":dbl}}
  T35 = typedef "GUI.lvlib/Messaging Actions.ctl" = enum16{"Create", "Get", "Destroy"}
  T36 = enum8{"Enabled", "Disabled", "Disabled and Grayed Out"}
  T37 = typedef "GUI.lvlib/Save Log State.ctl" = enum16{"Idle", "Init", "Write", "Exit"}
  T38 = enum32{"Invalid", "Standard", "Closed", "Hidden", "Minimized", "Maximized"}
  T39 = enum32{"Page Enabled", "Page Disabled", "Page Disabled & Grayed"}
  T40 = cluster{"Set Temp":dbl, "Power Drive":bool, "Feedback":u8, "Package":u16, "Enable":bool}
  T41 = typedef "GUI.lvlib/WebDAV states.ctl" = enum16{"Open Sess", "Refresh Dir", "Create Dir", "Upload", "Download", "Delete", "Close Sess"}
  T42 = cluster{"baud rate":u32, "data bits":u16, "parity":enum16{"None", "Odd", "Even", "Mark", "Space"}, "stop bits":u16, "flow control":u16}
  T43 = typedef "GUI.lvlib/Timer Mode.ctl" = enum16{"Start Timer", "Read Time", "Pause", "Resume"}
  T44 = enum16{"Start Timer", "Read Time", "Pause", "Resume"}
  T45 = cluster{"Current VI":refnum<vi>, "Close Panel on Exit?":bool, "VI Name":string, "VI Path":path}
  T46 = cluster{"0":string, "1":string, "2":string, "3":string, "4":string, "5":string, "6":string, "7":string, "8":string, "9":string}
  T47 = enum16{"M1 Set Point", "M1 Power Drive", "M1 Feedback", "M1 Package", "M1 Enable", "M2 Set Point", "M2 Power Drive", "M2 Feedback", "M2 Package", "M2 Enable", "System Power", "Config Data", "Stop RT"}
  T48 = typedef "NI_WebDAV.lvlib/SessionHandle.ctl" = refnum<k1>
  T49 = typedef "NI_WebDAV.lvlib/FileInfo.ctl" = cluster{"type":string, "size":u64, "last modification":timestamp, "display name":string, "uri":string}
  T50 = cluster{"DUT Force lbf":cluster{" 0":u32, " 1":u32, " 2":u32, "3":u32, "4":u32, "5":u32, " 6":u32, "7":u32, "8":u32, "9":u32}, "DUT Names":cluster{"0":string, "1":string, "2":string, "3":string, "4":string, "5":string, "6":string, "7":string, "8":string, "9":string}}
  T51 = cluster{"Force - pounds":cluster{" 0":u32, " 1":u32, " 2":u32, "3":u32, "4":u32, "5":u32, " 6":u32, "7":u32, "8":u32, "9":u32}, "DUT Names":cluster{"0":string, "1":string, "2":string, "3":string, "4":string, "5":string, "6":string, "7":string, "8":string, "9":string}}
  T52 = enum16{"Left Button", "Center Button", "Right Button", "Window Close"}
  T53 = typedef "Power Sequence.ctl" = cluster{"Duration":i32, "Head Load(W)":u32, "Name":string}[]
  T54 = cluster{"Duration":i32, "Head Load(W)":u32, "Name":string}
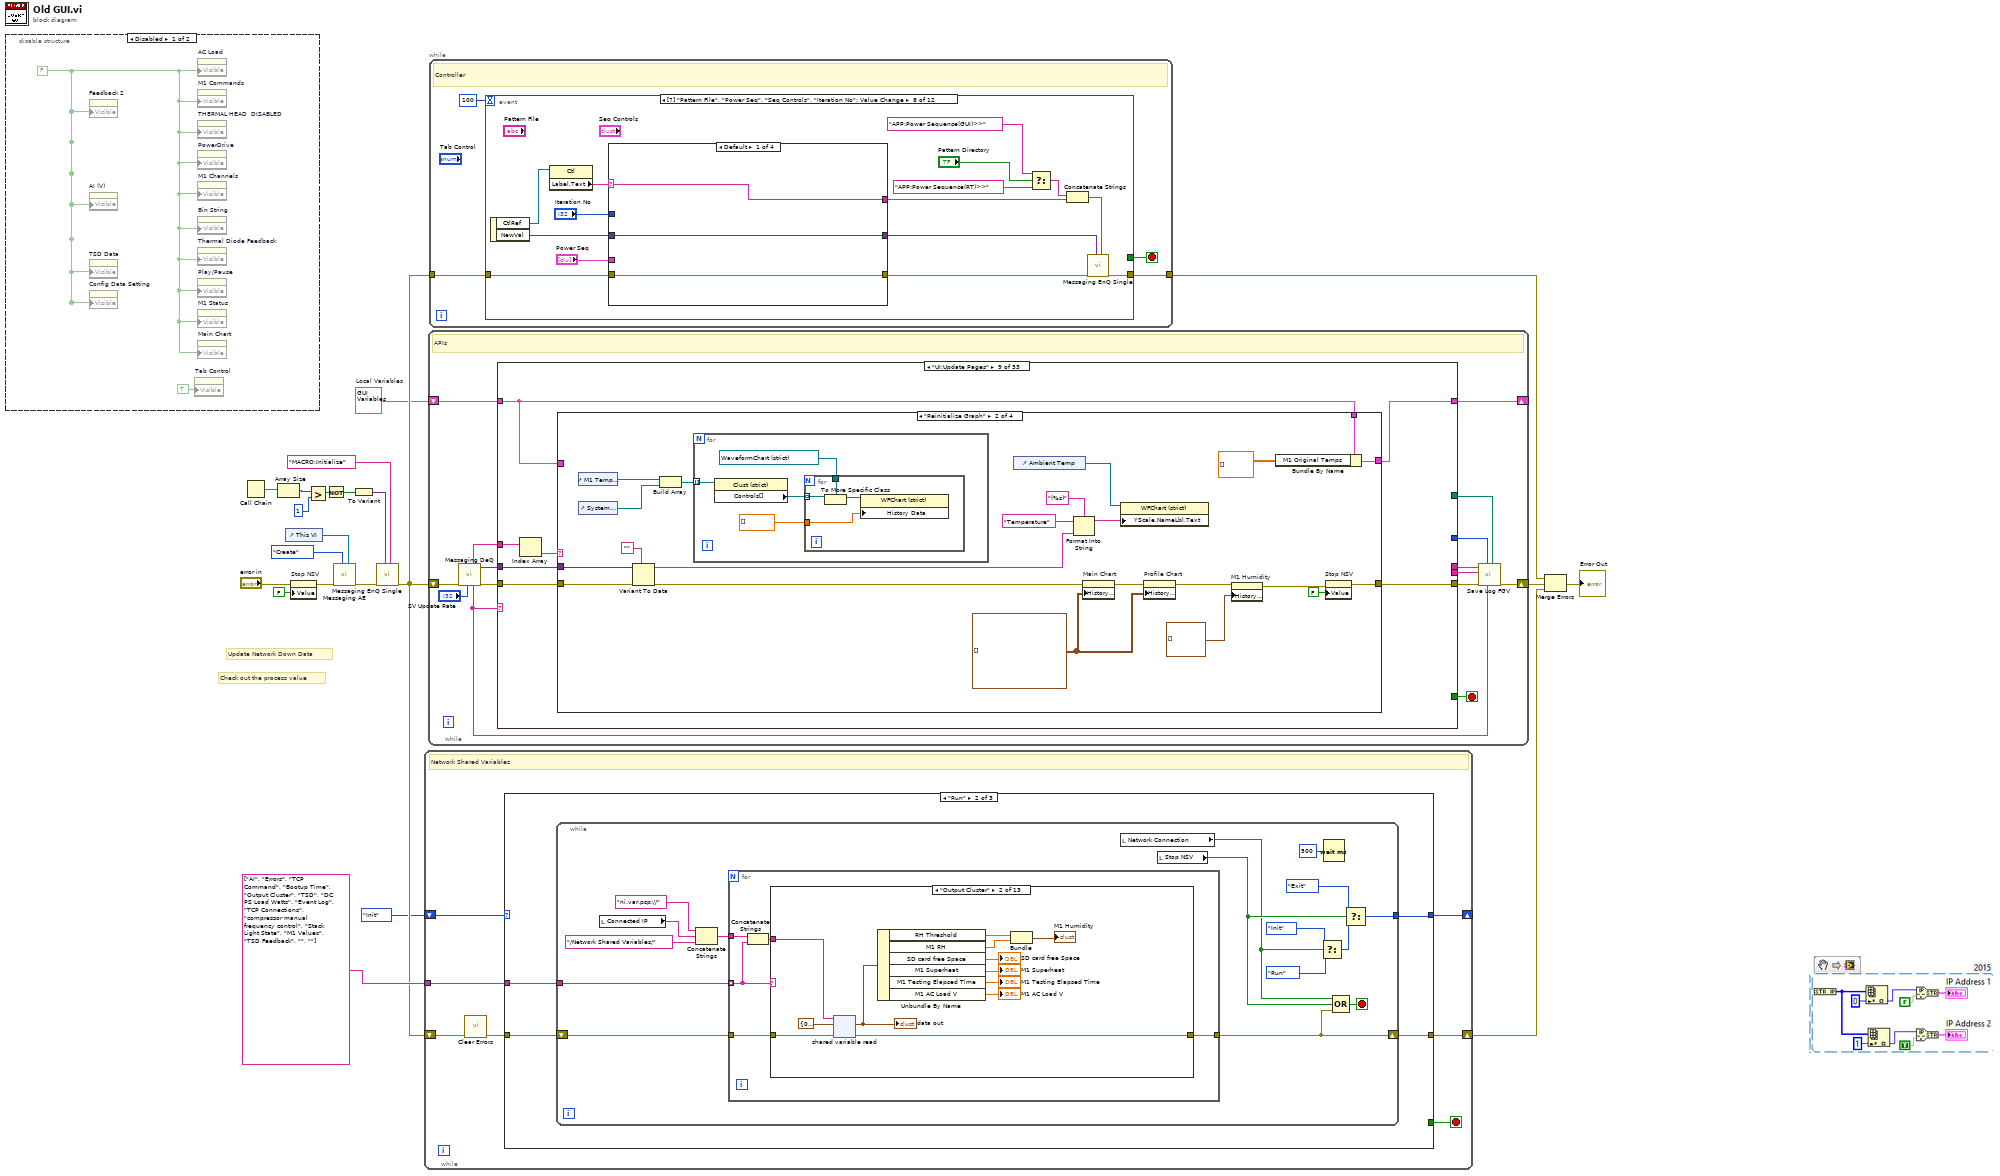
[diagram p0: block diagram]
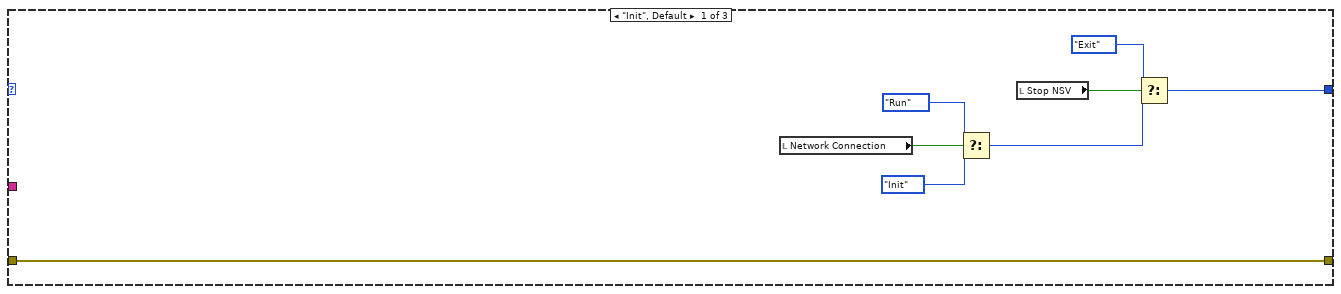
[diagram p3: hidden frame]
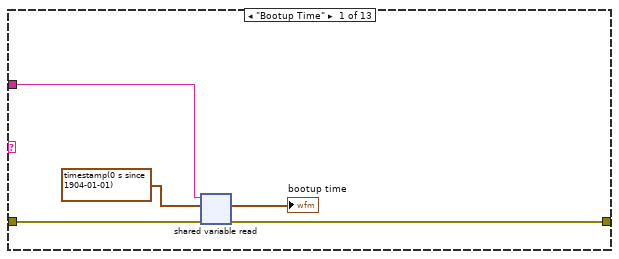
[diagram p4: hidden frame]
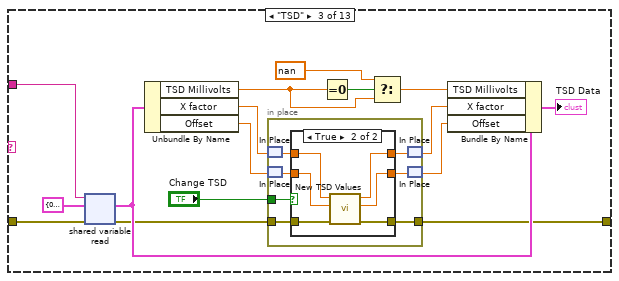
[diagram p5: hidden frame]
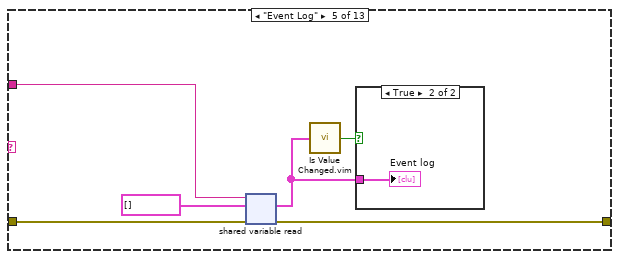
[diagram p8: hidden frame]
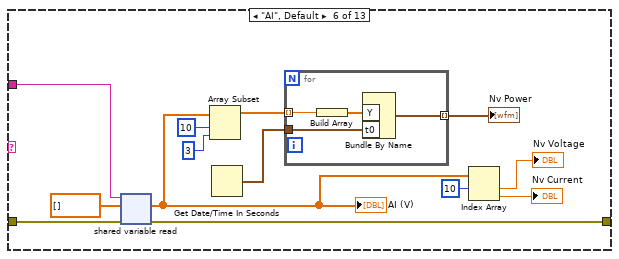
[diagram p10: hidden frame]
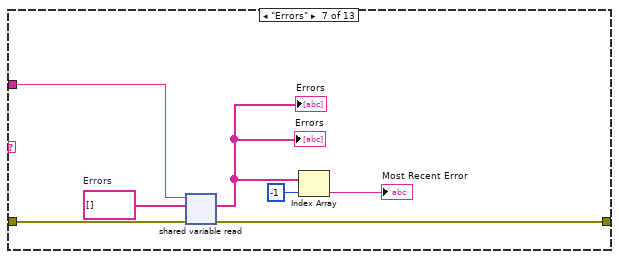
[diagram p11: hidden frame]
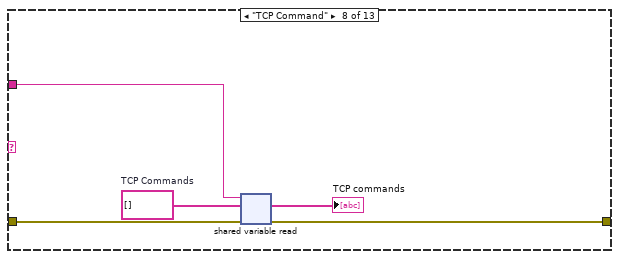
[diagram p12: hidden frame]
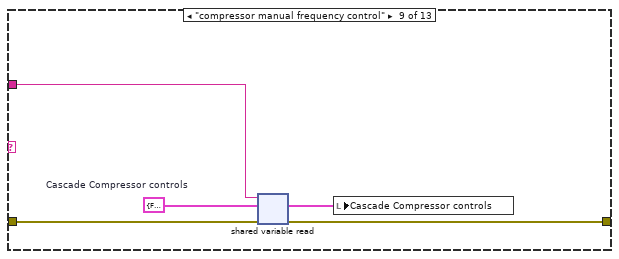
[diagram p13: hidden frame]
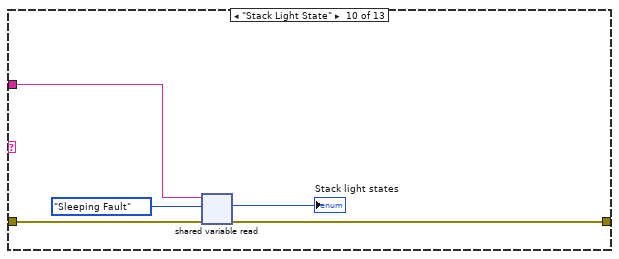
[diagram p14: hidden frame]
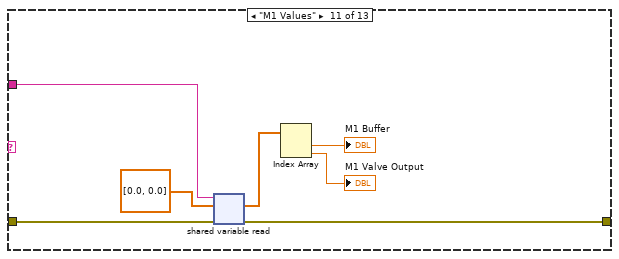
[diagram p15: hidden frame]
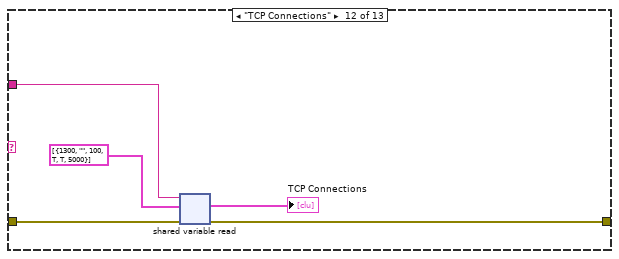
[diagram p16: hidden frame]
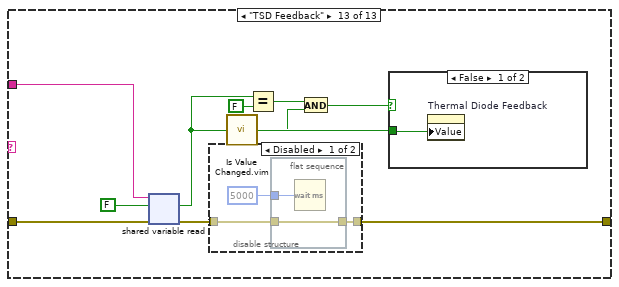
[diagram p17: hidden frame]
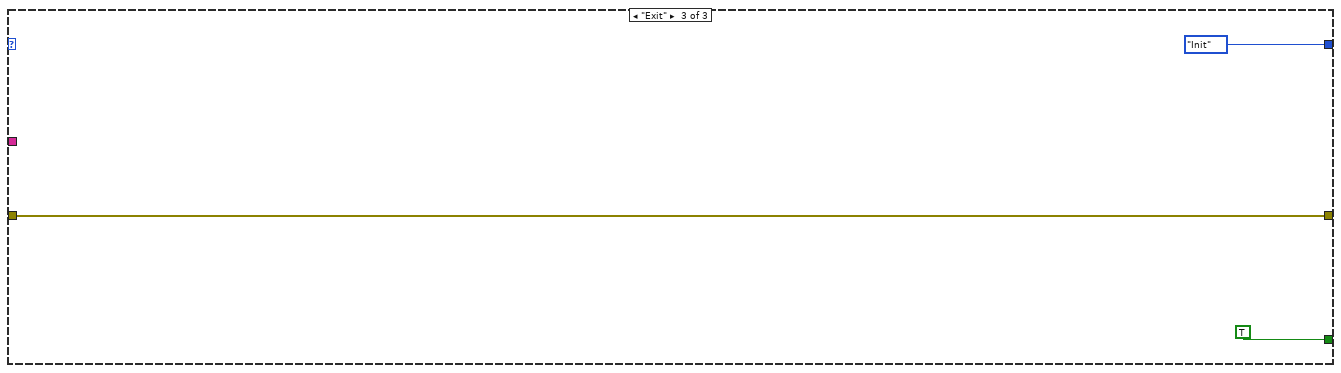
[diagram p20: hidden frame]
diagram:
  w6 = T24 {"Core"={"Current VI"=refnum, "Close Panel on Exit?"=FALSE, "VI Name"="", "VI Path"=path ""}, "Log?"=FALSE, "Current Case"="", "Shared Variable Address"="", "reader endpoint"="", "writer endpoint"="", "Detected Systems"=[], "IP Address"="", "Network Connection"=FALSE, "URI Directory"="", "File list in SoM"=[], "System State"=enum."Idle", "TTV Test"={"Power Seq"=[], "PS Connection"=FALSE, "OutputState"=FALSE, "Step"=0, "Current Cycle"=0}, "Profile"={"Profile Temp"=FALSE, "Current Cycle"=0}, "M1 History Temps"=[], "M2 History Temps"=[], "M1 Bootup"=FALSE, "M2 Bootup"=FALSE, "Network Data Down"={"M1 Commands"={"Set Temp"=20.0, "Power Drive"=FALSE, "Feedback"=1, "Package"=0, "Enable"=FALSE}, "M2 Commands"={"Set Temp"=20.0, "Power Drive"=FALSE, "Feedback"=1, "Package "=0, "Enable"=FALSE}, "Config Data"={"Packages"={"DUT Force lbf"={" 0"=0, " 1"=0, " 2"=0, "3"=0, "4"=0, "5"=0, " 6"=0, "7"=0, "8"=0, "9"=0}, "DUT Names"={"0"="", "1"="", "2"="", "3"="", "4"="", "5"="", "6"="", "7"="", "8"="", "9"=""}}, "Heater PID"={"P"=0.0, "I"=0.0, "D"=0.0}, "Piston Settings"={"Forces Slope"=0.0, "Forces Intercept"=0.0, "Transition Force"=0.0, "Up Force"=0.0, "Diameter (mm)"=0.0, "Delay (ms)"=0.0, "Pressure Ramp Delay (ms)"=0.0}, "Safe Temps"={"Minimum"=17, "Enabled"=TRUE, "Maximum"=95}, "System Settings"={"Number of Heads"=0, "60Hz Power"=TRUE, "FTC200"=TRUE, "AutoStartup"=FALSE, "Purge"=TRUE, "Sensors"=TRUE, "HandClamp"=TRUE, "ATE"=TRUE, "Benchtop"=TRUE, "Production"=TRUE, "Refrigerant"=enum."r404a", "Handler"=TRUE, "Shuttle"=TRUE, "220V"=FALSE, "Cascade"=FALSE, "Suction Sensor"=enum."YCQB02H01", "Discharge Sensor"=enum."YCQB05H01"}, "Stepper Settings "={"Microstepping"=enum."Full", "Velocity"=8}, "Set Point Range"={"Max"=0.0, "Min"=0.0}, "Pedestal Check DeltaT"=0.0, "Ramp Delta T"=0.0, "Ramp-SS Threshold"=0.0, "SS Tolerance"=0.0, "EEV PID"={"Ramp Up Target"=0.0, "Ramp Down Target"=0.0, "Steady State Target"=0.0, "Output"={"Max"=0.0, "Min"=0.0}, "EBB and Flow Temp TH"=0.0, "Cryomode EEV Max"=0.0, "Valve minimum opening "=0.0, "Ramp Up EEV Steps"=0.0, "Ramp Down EEV Steps"=0.0, "SS EEV Steps Reset"=0.0, "EBB and Flow Tol"=0.0, "Gains"={"P"=0.0, "I"=0.0, "D"=0.0}, "Dissabled Target"=0.0, "CryoMode Gains"={"P"=0.0, "I"=0.0, "D"=0.0}, "M1 SuperHeat Setpoint"=0.0, "M2 Gains"={"P"=0.0, "I"=0.0, "D"=0.0}, "Flow Curve"=enum.""}, "Sleep Timeout"=0.0, "Bypass Values"={"Bypass Valve"=TRUE, "Flow Curve"=enum."0", "Output"={"Max"=0, "Min"=0}, "Feedback"=enum."Temperature", "Cyth Bypass"=TRUE, "PID"={"P"=0.0, "I"=0.0, "D"=0.0}, "Pressure setpoint"=0, "Cryo Temp"=0, "Superheat Setpoint"=0, "Cryo Setpoint"=0}, "Default Temp"=0.0, "InTEC"={"Enabled"=FALSE, "IP"="192.168.1.100", "Port"=5000}, "M1 TSD"={"Gain"=0.0, "Offset"=0.0, "V Offset "=0.0}, "M2 TSD"={"Gain"=0.0, "Offset"=0.0, "V Offset "=0.0}, "M1 T-Case Calibration"={"Gain"=0.0, "Offset"=0.0}, "M2 T-Case Calibration"={"Gain"=0.0, "Offset"=0.0}, "Heater PID TSD"={"P"=0.0, "I"=0.0, "D"=0.0}, "M2 Heater PID"={"P"=0.0, "I"=0.0, "D"=0.0}}, "System Power On Off"=FALSE, "New Data"=enum."M1 Set Point", "Stop RT"=FALSE}, "Event Log"=[], "Login"=FALSE, "Connected System"="", "TCP connection info"={"connection ID"=refnum, "meta data"=[]}, "TCP Connection"=FALSE, "Dataset"={"System Status"={"Power On Off"=FALSE, "Discharge Temp"=0.0, "Liquid Temp"=0.0, "Suction Temp"=0.0, "Ambient Temp"=0.0, "Sleep"=FALSE, "System Status"=0, "M1 Actuated"=FALSE, "M2 Actuated"=FALSE, "Sleep Timer"=0.0, "M1 Bin"={"Bin String"="", "Bin Color"=1}, "M2 Bin"={"Bin String"="", "Bin Color"=1}, "Discharge Pressure"=0.0, "Suction Pressure"=0.0, "Compression Ratio"=0.0, "Compressor Amps"=0.0, "Compressor Hours"=0.0, "Bypass Steps"=0, "SubCooling"=0.0, "SuperHeat"=0.0, "Serial Number"="", "EMO detected"=FALSE, "EMO Tripped"=FALSE, "Thermal cutoff"=FALSE, "Thermal cutoff 2"=FALSE, "High Pressure switch"=FALSE, "Running Time"=timestamp(0 s since 1904-01-01), "SOM Status"={"Boot Up Time"=timestamp(0 s since 1904-01-01), "Software Version"="", "CPU Usage"=0.0, "Memory Available"=0.0, "SD card free space"=0.0, "SOM Storage"=0.0}, "Cascade Extra"={"Discharge Temp High Side"=0.0, "Suction Temp High Side"=0.0, "Liquid Temp High side"=0.0, "Discharge Pressure 2"=0.0, "Suction Pressure 2"=0.0, "Low Side RPM"=0.0, "High Side RPM"=0.0}}, "M1 Status"={"Case Temp"=0.0, "Evap Temp"=0.0, "Heater %"=0.0, "EEV Steps"=0, "Set Temp"=0.0, "Feedback"=0, "Power Drive"=FALSE, "Piston Volts"=0.0, "Safe Temp"=FALSE, "Power"=FALSE, "Thermal State"=0, "Error"=FALSE, "In tollerance"=FALSE, "Head State"=0, "Piston Force"=0.0, "Package"="", "Dynamic SV"=0.0, "PV"=0.0, "TSD Temp"=0.0, "DC Load Watts"=0.0, "AC Load Watts"=0.0, "Intec Feedback"=0.0}, "M2 Status"={"Case Temp"=0.0, "Evap Temp"=0.0, "Heater %"=0.0, "EEV Steps"=0, "Set Temp"=0.0, "Feedback"=0, "Power Drive"=FALSE, "Piston Volts"=0.0, "Safe Temp"=FALSE, "Power"=FALSE, "Thermal State"=0, "Error"=FALSE, "In tollerance"=FALSE, "Head State"=0, "Piston Force"=0.0, "Package"="", "PV"=0.0, "Dynamic SV"=0.0, "TSD"=0.0, "AC Load Watts"=0.0}, "Config Data"={"Packages"={"DUT Force lbf"={" 0"=0, " 1"=0, " 2"=0, "3"=0, "4"=0, "5"=0, " 6"=0, "7"=0, "8"=0, "9"=0}, "DUT Names"={"0"="", "1"="", "2"="", "3"="", "4"="", "5"="", "6"="", "7"="", "8"="", "9"=""}}, "Heater PID"={"P"=0.0, "I"=0.0, "D"=0.0}, "Piston Settings"={"Forces Slope"=0.0, "Forces Intercept"=0.0, "Transition Force"=0.0, "Up Force"=0.0, "Diameter (mm)"=0.0, "Delay (ms)"=0.0, "Pressure Ramp Delay (ms)"=0.0}, "Safe Temps"={"Minimum"=17, "Enabled"=TRUE, "Maximum"=95}, "System Settings"={"Number of Heads"=0, "60Hz Power"=TRUE, "FTC200"=TRUE, "AutoStartup"=FALSE, "Purge"=TRUE, "Sensors"=TRUE, "HandClamp"=TRUE, "ATE"=TRUE, "Benchtop"=TRUE, "Production"=TRUE, "Refrigerant"=0, "Handler"=TRUE, "Shuttle"=TRUE, "220V"=FALSE, "Cascade"=FALSE, "Suction Sensor"=0, "Discharge Sensor"=0}, "Stepper Settings "={"Microstepping"=0, "Velocity"=8}, "Set Point Range"={"Max"=0.0, "Min"=0.0}, "Pedestal Check DeltaT"=0.0, "Ramp Delta T"=0.0, "Ramp-SS Threshold"=0.0, "SS Tolerance"=0.0, "EEV PID"={"Ramp Up Target"=0.0, "Ramp Down Target"=0.0, "Steady State Target"=0.0, "Output"={"Max"=0.0, "Min"=0.0}, "EBB and Flow Temp TH"=0.0, "Cryomode EEV Max"=0.0, "Valve minimum opening "=0.0, "Ramp Up EEV Steps"=0.0, "Ramp Down EEV Steps"=0.0, "SS EEV Steps Reset"=0.0, "EBB and Flow Tol"=0.0, "Gains"={"P"=0.0, "I"=0.0, "D"=0.0}, "Dissabled Target"=0.0, "CryoMode Gains"={"P"=0.0, "I"=0.0, "D"=0.0}, "M1 SuperHeat Setpoint"=0.0, "M2 Gains"={"P"=0.0, "I"=0.0, "D"=0.0}, "Flow Curve"=0}, "Sleep Timeout"=0.0, "Bypass Values"={"Bypass Valve"=TRUE, "Flow Curve"=0, "Output"={"Max"=0, "Min"=0}, "Feedback"=0, "Cyth Bypass"=TRUE, "PID"={"P"=0.0, "I"=0.0, "D"=0.0}, "Pressure setpoint"=0, "Cryo Temp"=0, "Superheat Setpoint"=0, "Cryo Setpoint"=0}, "Default Temp"=0.0, "InTEC"={"Enabled"=FALSE, "IP"="192.168.1.100", "Port"=5000}, "M1 TSD"={"Gain"=0.0, "Offset"=0.0, "V Offset "=0.0}, "M2 TSD"={"Gain"=0.0, "Offset"=0.0, "V Offset "=0.0}, "M1 T-Case Calibration"={"Gain"=0.0, "Offset"=0.0}, "M2 T-Case Calibration"={"Gain"=0.0, "Offset"=0.0}, "Heater PID TSD"={"P"=0.0, "I"=0.0, "D"=0.0}, "M2 Heater PID"={"P"=0.0, "I"=0.0, "D"=0.0}}}}  # Local Variables
  # "Update Network Down Data"
  # "Check out the process value"
  n1 = disable-structure shown="Disabled" {
    frame Disabled {
      w22 = FALSE
      n2 = property on="Feedback 2" class="Ring (strict)"("Visible"=w22) -> ()  [unwired: 2 in, 2 out]
      n3 = property on="AI (V)" class="Arr (strict)"("Visible"=w22) -> ()  [unwired: 2 in, 2 out]
      n4 = property on="TSD Data" class="Clust (strict)"("Visible"=w22) -> ()  [unwired: 2 in, 2 out]
      n5 = property on="Config Data Setting" class="Bool"("Visible"=w22) -> ()  [unwired: 2 in, 2 out]
      n6 = property on="Tab Control" class="TabCtl (strict)"("Visible"=TRUE) -> ()  [unwired: 2 in, 2 out]
      n7 = property on="AC Load" class="WFChart (strict)"("Visible"=w22) -> ()  [unwired: 2 in, 2 out]
      n8 = property on="M1 Commands" class="Clust (strict)"("Visible"=w22) -> ()  [unwired: 2 in, 2 out]
      n9 = property on="THERMAL HEAD  DISABLED" class="Bool"("Visible"=w22) -> ()  [unwired: 2 in, 2 out]
      n10 = property on="PowerDrive" class="Bool"("Visible"=w22) -> ()  [unwired: 2 in, 2 out]
      n11 = property on="M1 Channels" class="Arr (strict)"("Visible"=w22) -> ()  [unwired: 2 in, 2 out]
      n12 = property on="Bin String" class="Str"("Visible"=w22) -> ()  [unwired: 2 in, 2 out]
      n13 = property on="Thermal Diode Feedback" class="Bool (strict)"("Visible"=w22) -> ()  [unwired: 2 in, 2 out]
      n14 = property on="Play/Pause" class="Bool"("Visible"=w22) -> ()  [unwired: 2 in, 2 out]
      n15 = property on="M1 Status" class="Clust (strict)"("Visible"=w22) -> ()  [unwired: 2 in, 2 out]
      n16 = property on="Main Chart" class="WFChart (strict)"("Visible"=w22) -> ()  [unwired: 2 in, 2 out]
    }
    frame Enabled {
    }
  }
  n17 = Call Chain() -> (call chain=w14:string[])
  n18 = Array Size(array=w14) -> (size(s)=w11:i32)
  n19 = control-ref of="This VI"() -> (w15:refnum<vi>)
  n20 = property on="Stop NSV" class="Bool (strict)"(error in="error in", "Value"=FALSE ("kill")) -> (error out=w2:errorcluster)  [unwired: 1 in, 1 out]
  n21 = Greater?(x=w11, y=1) -> (0:w12:bool)
  n22 = Not(x=w12) -> (.not. x?=w8:bool)
  n23 = call "Messaging AE.vi"("VI Refnum"=w15, "Action"=Messaging_Actions."Create", "Error In"=w2) -> ("Error Out"=w9:errorcluster)  [unwired: 7 in, 1 out]
  n24 = To Variant(anything=w8) -> (Variant=w16:variant)
  n25 = call "Messaging EnQ Single.vi"("Command"="MACRO:Initialize", "Data"=w16, "error in (no error)"=w9) -> ("error out"=w7:errorcluster)  [unwired: 8 in]
  n26 = while {
    shift-right: [w29] -> w5
    shift-left: w7 -> [w30]
    tunnel: string[] ["AI", "Errors", "TCP Command", "Bootup Time", "Output Cluster", "TSD", "DC PS Load Watts", "Event Log", "TCP Connections", "compressor manual frequency control", "Stack Light State", "M1 Values", "TSD Feedback", "", ""] -> [w27]
    shift-right: [w26] -> _
    shift-left: NSV_States."Init" ("NSV States") -> [w24]
    stop <- w25 stop-if-true
    # "Network Shared Variables"
    n27 = call <vilib>:"Clear Errors.vi"("error in (no error)"=w30) -> ("error out"=w28:errorcluster)  [unwired: 5 in, 1 out]
    n28 = case shown="\"Run\"" w24 {
      tunnel: [w31 w42 w189] -> w29
      tunnel: w28 -> [w31 w41 w189]
      tunnel: w27 -> [_ w40 _]
      tunnel: [w34 w39 NSV_States."Init" ("NSV States")] -> w26
      tunnel: [_ _ TRUE] -> w25
      frame "Init", Default {
        n29 = local read "Network Connection"() -> (w33:bool)
        n30 = Select(t=NSV_States."Run" ("NSV States"), s=w33, f=NSV_States."Init" ("NSV States")) -> (s? t:f=w36:T23)
        n31 = local read "Stop NSV"() -> (w32:bool)
        n32 = Select(t=NSV_States."Exit" ("NSV States"), s=w32, f=w36) -> (s? t:f=w34:T23)
      }
      frame "Run" {
        n33 = while {
          tunnel: w40 -> [w57]
          shift-right: [w45] -> w42
          shift-left: w41 -> [w58]
          tunnel: [w52] -> w39
          stop <- w51 stop-if-true
          n34 = local read "Connected IP"() -> (w47:string)
          n35 = Concatenate Strings("ni.var.psp://", w47, "/Network Shared Variables/") -> (w46:string)
          n36 = for {
            tunnel: w58 -> [w61]
            tunnel: [w62] -> w45
            tunnel: w57 -> [w60] mode=indexing
            tunnel: w46 -> [w59]
            n37 = Concatenate Strings(w59, w60) -> (w63:string)
            n38 = case shown="\"Output Cluster\"" w60 {
              tunnel: w61 -> [w68 w80 w96 w113 w119 w133 w144 w149 w154 w159 w166 w171 w174]
              tunnel: [w65 w77 w81 w113 w118 w132 w142 w147 w153 w157 w165 w170 w172] -> w62
              tunnel: w63 -> [w66 w79 w95 _ w117 w131 w143 w148 w151 w158 w164 w169 w176]
              frame "Bootup Time" {
                n39 = shared-variable-read(w66, w68, timestamp(0 s since 1904-01-01)) -> (w65:errorcluster, →"bootup time":timestamp)  [unwired: 2 out]
              }
              frame "Output Cluster" {
                # "Read the RT Information to debug GUI"
                n40 = shared-variable-read(w79, w80, T2 {"Condensing Pressure"=0.0, "Suction Pressure"=0.0, "Bypass steps"=0, "Operating Time"=0.0, "SubCooling"=0.0, "Superheat"=0.0, "M1 Superheat"=0.0, "M2 Superheat"=0.0, "Autotune output"=0.0, "M1 Testing Elapsed Time"=0.0, "M2 Testing Elapsed Time"=0.0, "M1 Valve Control Mode"=0, "System Amps"=0.0, "Compressor Run Time"=0.0, "SD card free Space"=0.0, "Free Memory"=0.0, "M1 Pressure Feedback"=0.0, "M2 Pressure Feedback"=0.0, "Compression Ratio"=0.0, "Serial Number"=0.0, "M1 AC Load V"=0.0, "M1 AC Load W"=0.0, "M1 DC Load W"=0.0, "M1 RH"=0.0, "RH Threshold"=0.0} ("output cluster")) -> (w77:errorcluster, w76:T2)  [unwired: 2 out]
                "data out" <- w76
                n41 = Unbundle By Name(w76) -> ("RH Threshold"=w70:dbl, "M1 RH"=w71:dbl, "SD card free Space"=→"SD card free Space":dbl, "M1 Superheat"=→"M1 Superheat":dbl, "M1 Testing Elapsed Time"=→"M1 Testing Elapsed Time":dbl, "M1 AC Load V"=→"M1 AC Load V":dbl)
                n42 = Bundle("RH Threshold"=w70, "M1 RH"=w71) -> (→"M1 Humidity":cluster{"RH Threshold":dbl, "M1 RH":dbl})  [unwired: 1 in]
              }
              frame "TSD" {
                n43 = shared-variable-read(w95, w96, T16 {"TSD Millivolts"=0.0, "X factor"=0.0, "Offset"=0.0, "TSD Temp"=0.0, "TSD Feedback"=FALSE, "TSD Max"=0.0, "TSD Min"=0.0} ("TSD Data")) -> (w82:errorcluster, w91:T16)  [unwired: 2 out]
                n44 = Unbundle By Name(w91) -> ("TSD Millivolts"=w93:dbl, "X factor"=w87:dbl, "Offset"=w86:dbl)
                n45 = in-place {
                  in-place-border: "Change TSD" -> [w103]
                  in-place-border: w82 -> [w98]
                  in-place-border: [w97] -> w81
                  n46 = in-place-match #1(w87) -> (w102:dbl)
                  n47 = in-place-match #2(w86) -> (w100:dbl)
                  n48 = case shown="True" w103 {
                    tunnel: w102 -> [w106 w112]
                    tunnel: [w106 w110] -> w101
                    tunnel: w100 -> [w105 w111]
                    tunnel: [w105 w109] -> w99
                    tunnel: w98 -> [w104 w108]
                    tunnel: [w104 w107] -> w97
                    frame False {
                    }
                    frame True {
                      n49 = call "New TSD Values.vi"("Error In"=w108, "Offset"=w111, "X factor"=w112) -> ("Error Out"=w107:errorcluster, "Offset out"=w109:dbl, "X factor out"=w110:dbl)  [unwired: 6 in]
                    }
                  }
                  n50 = in-place-match #1(w101) -> (w85:dbl)
                  n51 = in-place-match #2(w99) -> (w84:dbl)
                }
                n52 = Equal To 0?(x=w93) -> (x = 0?=w92:bool)
                n53 = Select(t=nan, s=w92, f=w93) -> (s? t:f=w90:dbl)
                n54 = Bundle By Name(cluster=w91, "TSD Millivolts"=w90, "X factor"=w85, "Offset"=w84) -> (→"TSD Data":T16)
              }
              frame "DC PS Load Watts" {
                # "We dont use DC power Supply Anymore, now the TTV uses AC programmable power supply.  It tells the cobra exaclty how many watts the TTV is producing"
                # "This is for testing and datalogging purpose"
              }
              frame "Event Log" {
                n55 = shared-variable-read(w117, w119, T14 [] ("Event Log")) -> (w118:errorcluster, w114:T14)  [unwired: 2 out]
                n56 = call "Is Value Changed.vim"("value"=w114) -> ("changed or first call?"=w115:bool)
                n57 = case shown="True" w115 {
                  tunnel: w114 -> [_ w120]
                  frame False {
                  }
                  frame True {
                    "Event log" <- w120
                  }
                }
              }
              frame "AI", Default {
                # "Analog Inputs"
                n58 = shared-variable-read(w131, w133, dbl[] [] ("AI (V) 2")) -> (w132:errorcluster, w124:dbl[])  [unwired: 2 out]
                "AI (V)" <- w124
                n59 = Array Subset(array=w124, index=10, length=3) -> (w128:dbl[])
                n60 = Get Date/Time In Seconds() -> (seconds since 1Jan1904=w129:timestamp)
                n61 = for {
                  tunnel: w128 -> [w136] mode=indexing
                  tunnel: w129 -> [w137]
                  tunnel: [w134] -> w125 mode=indexing
                  n62 = Build Array(w136) -> (w135:dbl[])
                  n63 = Bundle By Name("Y"=w135, "t0"=w137) -> (w134:waveform(dbl))  [unwired: 1 in]
                }
                "Nv Power" <- w125
                n64 = Index Array(array=w124, index #1=10 ("index")) -> (element #1=→"Nv Voltage":dbl, element #2=→"Nv Current":dbl)  [unwired: 1 in]
              }
              frame "Errors" {
                w141 = string[] []  # Errors
                n65 = shared-variable-read(w143, w144, w141) -> (w142:errorcluster, w140:string[])  [unwired: 2 out]
                "Errors" <- w140
                "Errors" <- w140
                n66 = Index Array(array=w140, index=-1) -> (element=→"Most Recent Error":string)
              }
              frame "TCP Command" {
                w146 = string[] []  # TCP Commands
                # "The list of ports with connection status"
                n67 = shared-variable-read(w148, w149, w146) -> (w147:errorcluster, →"TCP commands":string[])  [unwired: 2 out]
              }
              frame "compressor manual frequency control" {
                w152 = T15 {"High Stage manual speed control"=FALSE, "Manual High stage frequency"=0.0, "Low Stage manual speed control"=FALSE, "Manual Low Stage frequency"=0.0}  # Cascade Compressor controls
                # "king cobra compressor RPM"
                n68 = shared-variable-read(w151, w154, w152) -> (w153:errorcluster, w150:T15)  [unwired: 2 out]
                n69 = local write "Cascade Compressor controls"(w150) -> ()
              }
              frame "Stack Light State" {
                # "Monitoring RT Status"
                n70 = shared-variable-read(w158, w159, T1."Sleeping Fault" ("Stack light states")) -> (w157:errorcluster, →"Stack light states":T1)  [unwired: 2 out]
              }
              frame "M1 Values" {
                # "Array that includes EEV PID Output"
                n71 = shared-variable-read(w164, w166, dbl[] [0.0, 0.0]) -> (w165:errorcluster, w162:dbl[])  [unwired: 2 out]
                n72 = Index Array(array=w162) -> (element #1=→"M1 Buffer":dbl, element #2=→"M1 Valve Output":dbl)  [unwired: 2 in]
              }
              frame "TCP Connections" {
                n73 = shared-variable-read(w169, w171, T17 [{"port "=1300, "remote address"="", "Connection timeout ms"=100, "Waiting for connection"=TRUE, "Waiting for Command"=TRUE, "timeout ms"=5000}] ("TCP Connections")) -> (w170:errorcluster, →"TCP Connections":T17)  [unwired: 2 out]
              }
              frame "TSD Feedback" {
                n74 = shared-variable-read(w176, w174, FALSE ("data type")) -> (w173:errorcluster, w180:bool)  [unwired: 2 out]
                n75 = disable-structure shown="Disabled" {
                  disable-tunnel: w173 -> [w184 _]
                  disable-tunnel: [w183 _] -> w172
                  frame Disabled {
                    n76 = flat-sequence {
                      tunnel: w184 -> [w186]
                      tunnel: [w186] -> w183
                      tunnel: u32 5000 ("milliseconds to wait") -> [w185]
                      frame #0 {
                        n77 = Wait (ms)(milliseconds to wait=w185) -> ()  [unwired: 1 out]
                      }
                    }
                  }
                  frame Enabled {
                  }
                }
                n78 = call "Is Value Changed.vim"("value"=w180) -> ("changed or first call?"=w179:bool)
                n79 = Equal?(x=w180, y=FALSE) -> (x = y?=w181:bool)
                n80 = And(x=w181, y=w179) -> (x .and. y?=w175:bool)
                n81 = case shown="False" w175 {
                  tunnel: w180 -> [w187 _]
                  frame False {
                    n82 = property on="Thermal Diode Feedback" class="Bool (strict)"("Value"=w187) -> ()  [unwired: 2 in, 2 out]
                  }
                  frame True {
                  }
                }
              }
            }
          }
          n83 = local read "Network Connection"() -> (w43:bool)
          n84 = local read "Stop NSV"() -> (w44:bool)
          n85 = Select(t=NSV_States."Init" ("NSV States"), s=w43, f=NSV_States."Run" ("NSV States")) -> (s? t:f=w56:T23)
          n86 = Wait (ms)(milliseconds to wait=u32 500) -> ()  [unwired: 1 out]
          n87 = Compound Arithmetic op=OR(w43, w44, w45) -> (w51:bool)
          n88 = Select(t=NSV_States."Exit" ("NSV States"), s=w44, f=w56) -> (s? t:f=w52:T23)
        }
      }
      frame "Exit" {
      }
    }
  }
  n89 = while {
    shift-right: [w196] -> w20
    shift-left: w7 -> [w204]
    shift-right: [w202] -> _
    shift-left: w6 -> [w200]
    stop <- w205 stop-if-true
    # "APIs"
    n90 = call "Messaging DeQ.vi"("Time out"="SV Update Rate", "Error In"=w204) -> ("error out"=w203:errorcluster, "Data"=w199:variant, "Command"=w194:string, "[String Data]"=w198:string[])  [unwired: 6 in]
    n91 = case shown="\"UI:Update Pages\"" w194 {
      selector: w194 -> [w207 _ _ _ _ w289 _ _ _ _ _ _ _ _ _ _ _ _ _ _ w847 _ _ _ _ _ _ _ _ _ _ _ _]
      tunnel: w203 -> [w209 w239 w261 w268 w276 w293 w298 w300 w337 w444 w644 w661 w713 w729 w750 w760 w777 w785 w805 w824 w855 w867 w906 w1032 w1104 w1112 w1135 w1139 w1142 w1178 w1329 w1505 w1816]
      tunnel: [w208 w230 w258 w268 w276 w286 w298 w308 w335 w443 w644 w661 w713 w717 w746 w759 w777 w781 w796 w811 w851 w868 w913 w1030 w1104 w1119 w1134 w1139 w1150 w1179 w1335 w1502 w1810] -> w197
      tunnel: [_ _ _ _ _ TRUE _ _ _ _ _ _ _ _ _ _ _ _ _ _ _ _ _ _ _ _ _ _ _ _ _ _ _] -> w205
      tunnel: [w206 w236 w259 w267 w272 w294 w297 w304 w331 w442 w650 w662 w712 w733 w747 w775 w776 w783 w803 w836 w849 w871 w902 w1037 w1103 w1113 w1137 w1138 w1149 w1171 w1334 w1503 w1814] -> w202
      tunnel: w200 -> [w206 w236 w259 w267 w279 w294 w297 w305 w332 w441 w649 w662 w712 w733 w747 w775 w776 w784 w801 w821 w849 w861 w903 w1037 w1103 w1115 w1137 w1138 w1149 w1170 w1334 w1501 w1808]
      tunnel: w198 -> [_ _ _ _ _ _ _ w307 w334 _ _ _ _ _ _ _ _ _ _ _ _ _ w917 w1034 _ _ _ _ w1148 w1182 w1338 w1507 w1812]
      tunnel: w199 -> [_ _ _ _ _ _ _ _ w336 _ _ _ _ w727 w753 _ _ _ w804 _ _ _ w904 w1031 _ _ _ _ _ w1180 w1336 w1504 w1815]
      tunnel: [_ _ _ _ Save_Log_State."Init" ("State") Save_Log_State."Exit" ("State") _ _ _ _ _ _ _ _ Save_Log_State."Write" ("State") _ _ _ _ w810 w846 _ Save_Log_State."Write" ("State") _ _ _ _ _ w1140 _ _ w1500 w1806] -> w195
      tunnel: [_ _ _ _ w271 _ _ _ _ _ _ _ _ _ _ _ _ _ _ _ _ _ _ _ _ _ _ _ _ _ _ _ _] -> w193
      tunnel: [_ _ _ _ "Start Cobra GUI" ("name or relative path") _ _ _ _ _ _ _ _ _ _ _ _ _ _ w809 w845 _ w907 _ _ _ _ _ _ _ _ _ w1805] -> w192
      tunnel: [_ _ _ _ w269 _ _ _ _ _ _ _ _ _ _ _ _ _ _ _ _ _ _ _ _ _ _ _ _ _ _ _ _] -> w191
      frame Default {
        # "This case will only get called if there is no case that matches the incoming string.  A blank will do nothing, otherwise a popup will display what was sent."
        n92 = Unbundle By Name(w206) -> ("Core.VI Name"=w210:string)
        n93 = Empty String/Path?(string/path=w207) -> (empty?=w211:bool)
        n94 = case shown="False" w211 {
          tunnel: [w219 w226] -> w208
          tunnel: w209 -> [w212 w226]
          tunnel: w207 -> [w214 _]
          tunnel: w210 -> [w213 _]
          frame False {
            n95 = Format Into String(format string="Invalid Case:\n%s\nIn a VI named:\n%s", w214, w213) -> (resulting string=w216:string)  [unwired: 2 in, 1 out]
            n96 = Two Button Dialog(message=w216, 1:"Flush Q" ("T button name (\"OK\")"), 2:"Continue" ("T button name (\"OK\")")) -> (T button?=w220:bool)
            n97 = case shown="True" w220 {
              tunnel: w212 -> [w221 w224]
              tunnel: [w221 w225] -> w219
              frame False {
              }
              frame True {
                n98 = call "Messaging AE.vi"("Error In"=w224) -> ("Error Out"=w223:errorcluster, "queue out"=w222:refnum<queue>)  [unwired: 9 in]
                n99 = Flush Queue(queue=w222, error in (no error)=w223) -> (error out=w225:errorcluster)  [unwired: 2 out]
              }
            }
          }
          frame True {
          }
        }
      }
      frame "Idle" {
        # "Do something when in Idle State"
        n100 = call "Messaging EnQ Multiline String.vi"("Command(s)"="NS:Read\nUI:Update\nUI:Update Network Down Data\nUI:Visibility", "error in (no error)"=w239) -> ("error out"=w237:errorcluster)  [unwired: 9 in]
        n101 = Unbundle By Name(w236) -> ("TTV Test.OutputState"=w228:bool)
        n102 = case shown="True" w228 {
          tunnel: w237 -> [w251 w257]
          tunnel: [w251 w256] -> w229
          tunnel: [T36."Enabled" ("Disabled") T36."Disabled and Grayed Out" ("Disabled")] -> w231
          frame False {
          }
          frame True {
            n103 = Concatenate Strings("APP:TTV Test>>" ("Command(s)"), "Read TTV power" ("Command(s)")) -> (w252:string)
            n104 = call "Messaging EnQ Single.vi"("Command"=w252, "error in (no error)"=w257) -> ("error out"=w256:errorcluster)  [unwired: 9 in]
          }
        }
        n105 = control-ref of="Serial Port"() -> (w227:refnum<vi>)
        n106 = control-ref of="Power"() -> (w234:refnum<vi>)
        n107 = Build Array(w227, w234) -> (w233:refnum<vi>[])
        n108 = Unbundle By Name(w236) -> ("Profile.Profile Temp"=w235:bool)
        n109 = for {
          tunnel: w233 -> [w243] mode=indexing
          tunnel: w229 -> [w242]
          tunnel: [w241] -> w232
          tunnel: w231 -> [w240]
          n110 = property class="Ctl"(reference=w243, error in=w242, "DisabledEnum"=w240) -> (error out=w241:errorcluster)  [unwired: 1 out]
        }
        n111 = case shown="True" w235 {
          tunnel: w232 -> [w244 w249]
          tunnel: [w244 w248] -> w230
          frame False {
          }
          frame True {
            n112 = Concatenate Strings("APP:Temp Profile>>" ("Command"), "Read Temp" ("Command")) -> (w245:string)
            n113 = call "Messaging EnQ Single.vi"("Command"=w245, "error in (no error)"=w249) -> ("error out"=w248:errorcluster)  [unwired: 9 in]
          }
        }
      }
      frame "ERROR" {
        # "Process local ERRORs."
        n114 = Unbundle By Name(w261) -> ("code"=w260:i32)
        n115 = case shown="Default" w260 {
          tunnel: [errorcluster {"status"=FALSE, "code"=0, "source"=""} ("error out") w263] -> w258
          frame Default {
          }
          frame -314004 {
            # "Occurred due to Network Stream Connection and Can not make Reader and Writer Endpoint"
            n116 = disable-structure shown="Disabled" {
              disable-tunnel: [w264 _] -> w263
              frame Disabled {
                # "Retry to connect to RT"
                n117 = call "Messaging EnQ Single.vi"("Command"="NS:Open Connection", "@Front?"=TRUE) -> ("error out"=w264:errorcluster)  [unwired: 9 in]
              }
              frame Enabled {
              }
            }
          }
        }
      }
      frame "-----------System-----------" {
        # "Command Format:\nCAT:Command>>Data1,Data2,DataN"
        # "SYSTEM is used for things that directly effect this module"
      }
      frame "SYS:Initialize" {
        w285 = T45 {"Current VI"=refnum, "Close Panel on Exit?"=FALSE, "VI Name"="", "VI Path"=path ""}  # Core
        # "Initialize the system"
        n118 = control-ref of="This VI"() -> (w284:refnum<vi>)
        n119 = property class="VI"(reference=w284, "Front Panel.Title"="Cobra Single Head GUI" ("Front Panel Window:Title")) -> (reference out=w283:refnum<vi>, "Name"=w282:string, "Path"=w278:path)  [unwired: 1 in, 1 out]
        n120 = Bundle By Name(cluster=w285, "Current VI"=w283, "VI Name"=w282, "VI Path"=w278) -> (w281:T45)
        n121 = Bundle By Name(cluster=w279, "Core"=w281) -> (w272:T24)
        n122 = Unbundle By Name(w272) -> ("Core.VI Path"=w275:path, "Core.VI Name"=w271:string)
        n123 = Strip Path(path=w275) -> (stripped path=w274:path)  [unwired: 1 out]
        n124 = Build Path(base path=w274, name or relative path="Log") -> (appended path=w269:path)
      }
      frame "SYS:Exit" {
        # "Exits this loop and destroys the Queue.  The top loop will exit because the Queue no longer exists."
        n125 = call "Save Log FGV.vi"("Case"=w289, "State"=Save_Log_State."Write", "Error In"=w293) -> ("Error Out"=w292:errorcluster)  [unwired: 8 in]
        n126 = call "Messaging AE.vi"("Action"=Messaging_Actions."Destroy", "Error In"=w292) -> ("Error Out"=w287:errorcluster)  [unwired: 8 in, 1 out]
        n127 = property on="Stop NSV" class="Bool (strict)"(error in=w287, "Value"=TRUE ("Stop NSV")) -> (error out=w286:errorcluster)  [unwired: 1 in, 1 out]
      }
      frame "-----User Interface-----" {
        # "UI is used for things that will change the UI.,"
      }
      frame "UI:Front Panel State" {
        # "Open or Close front penl"
        n128 = Index Array(array=w307) -> (element=w306:string)  [unwired: 1 in]
        n129 = Unbundle By Name(w305) -> ("Core.Current VI"=w302:refnum<vi>)
        n130 = property class="VI"(reference=w302) -> (reference out=w303:refnum<vi>, "Front Panel.Open"=w301:bool)  [unwired: 1 in, 1 out]
        n131 = case shown="\"Close\"" w306 {
          tunnel: w300 -> [w310 w321]
          tunnel: [w313 w324] -> w308
          tunnel: w303 -> [w312 w322]
          tunnel: w301 -> [w311 w323]
          tunnel: [FALSE ("Core.Close Panel on Exit?") w320] -> w299
          frame "Open", Default {
            n132 = case shown="True" w311 {
              tunnel: [w315 w319] -> w313
              tunnel: w310 -> [w314 w319]
              tunnel: w312 -> [w316 _]
              frame False {
                n133 = invoke class="VI" method="FP.Open"(reference=w316, error in=w314, "Activate"=TRUE, "State"=T38."Standard") -> (error out=w315:errorcluster)  [unwired: 1 in, 4 out]
              }
              frame True {
              }
            }
          }
          frame "Close" {
            n134 = case shown="False" w323 {
              tunnel: [w326 w330] -> w324
              tunnel: w322 -> [_ w329]
              tunnel: w321 -> [w326 w328]
              tunnel: [FALSE ("Core.Close Panel on Exit?") TRUE ("Core.Close Panel on Exit?")] -> w320
              frame False {
              }
              frame True {
                n135 = invoke class="VI" method="FP.Close"(reference=w329, error in=w328) -> (error out=w330:errorcluster)  [unwired: 1 in, 2 out]
              }
            }
          }
        }
        n136 = Bundle By Name(cluster=w305, "Core.Close Panel on Exit?"=w299) -> (w304:T24)
      }
      frame "UI:Update Pages" {
        n137 = Index Array(array=w334) -> (element=w333:string)  [unwired: 1 in]
        n138 = case shown="\"Reinitialize Graph\"" w333 {
          tunnel: w337 -> [w351 w386 w411 w430]
          tunnel: w336 -> [w350 w385 _ w429]
          tunnel: [w346 w375 w402 w425] -> w335
          tunnel: w332 -> [_ _ w401 _]
          tunnel: w332 -> [w338 w374 w399 w424]
          tunnel: [w338 w372 w399 w424] -> w331
          frame "Enable Pages", Default {
            n139 = control-ref of="Tab Control"() -> (w342:refnum<vi>)
            n140 = Variant To Data(error in=w351, type=cluster{"Page array":i32[], "Enable":bool} {"Page array"=[], "Enable"=FALSE} ("output cluster"), Variant=w350) -> (data=w345:cluster{"Page array":i32[], "Enable":bool}, error out=w339:errorcluster)
            n141 = Unbundle By Name(w345) -> ("Page array"=w343:i32[], "Enable"=w340:bool)
            n142 = property class="TabCtl (strict)"(reference=w342) -> ("Pages"=w349:refnum<vi>[])  [unwired: 1 in, 2 out]
            n143 = case shown="False" w340 {
              tunnel: [T39."Page Disabled & Grayed" ("Page Enabled State") T39."Page Enabled" ("Page Enabled State")] -> w347
              tunnel: [w360 w366] -> w348
              tunnel: w349 -> [w357 w367]
              tunnel: w343 -> [_ w364]
              tunnel: w342 -> [w356 _]
              frame False {
                n144 = Array Subset(array=w357, index=3, length=4) -> (w360:refnum<vi>[])
                n145 = property class="TabCtl (strict)"(reference=w356, "Value"=T3."Controls") -> ()  [unwired: 1 in, 2 out]
              }
              frame True {
                n146 = Array Size(array=w364) -> (size(s)=w365:i32)
                n147 = Index Array(array=w364) -> (element=w363:i32)  [unwired: 1 in]
                n148 = Array Subset(array=w367, index=w363, length=w365) -> (w366:refnum<vi>[])
              }
            }
            n149 = property on="Config Data Setting" class="Bool"(error in=w339, "Visible"=w340) -> (error out=w341:errorcluster)  [unwired: 1 in, 1 out]
            n150 = for {
              tunnel: w348 -> [w352] mode=indexing
              tunnel: w347 -> [w355]
              tunnel: [w354] -> w346
              tunnel: w341 -> [w353]
              n151 = property class="Page"(reference=w352, error in=w353, "PageEnb"=w355) -> (error out=w354:errorcluster)  [unwired: 1 out]
            }
          }
          frame "Reinitialize Graph" {
            w376 = waveform(dbl)[][] [] ("History Data")
            n152 = control-ref of="M1 Temp Graphs"() -> (w390:refnum<vi>)
            n153 = control-ref of="System Graphs"() -> (w389:refnum<vi>)
            n154 = Variant To Data(error in=w386, type="", Variant=w385) -> (data=w381:string, error out=w378:errorcluster)
            n155 = Build Array(w390, w389) -> (w379:refnum<vi>[])
            n156 = for {
              tunnel: w379 -> [w391] mode=indexing
              n157 = property class="Clust (strict)"(reference=w391) -> ("Controls[]"=w393:refnum<vi>[])  [unwired: 1 in, 2 out]
              n158 = for {
                tunnel: w393 -> [w398] mode=indexing
                tunnel: refnum<vi> refnum ("M1 Heater Power (%)") -> [w396]
                tunnel: dbl[] [] ("History Data") -> [w395]
                n159 = To More Specific Class(target class=w396, reference=w398) -> (specific class reference=w397:refnum<vi>)  [unwired: 1 in, 1 out]
                n160 = property class="WFChart (strict)"(reference=w397, "History Data"=w395) -> ()  [unwired: 1 in, 2 out]
              }
            }
            n161 = control-ref of="Ambient Temp"() -> (w380:refnum<vi>)
            n162 = Format Into String(format string="(%s)", initial string="Temperature" ("Command"), w381) -> (resulting string=w383:string)  [unwired: 1 in, 1 out]
            n163 = property on="Main Chart" class="WFChart (strict)"(error in=w378, "History Data"=w376) -> (error out=w377:errorcluster)  [unwired: 1 in, 1 out]
            n164 = property class="WFChart (strict)"(reference=w380, "YScale.NameLbl.Text"=w383) -> ()  [unwired: 1 in, 2 out]
            n165 = property on="Profile Chart" class="WFChart (strict)"(error in=w377, "History Data"=w376) -> (error out=w371:errorcluster)  [unwired: 1 in, 1 out]
            n166 = property on="M1 Humidity" class="WFChart (strict)"(error in=w371, "History Data"=cluster{"M1 RH":dbl, "RH Threshold":dbl}[] []) -> (error out=w370:errorcluster)  [unwired: 1 in, 1 out]
            n167 = Bundle By Name(cluster=w374, "M1 Original Temps"=dbl[][] []) -> (w372:T24)
            n168 = property on="Stop NSV" class="Bool (strict)"(error in=w370, "Value"=FALSE ("kill")) -> (error out=w375:errorcluster)  [unwired: 1 in, 1 out]
          }
          frame "Initialize Test" {
            n169 = Unbundle By Name(w401) -> ("Core.VI Path"=w400:path)
            n170 = Strip Path(path=w400) -> (stripped path=w417:path)  [unwired: 1 out]
            n171 = Build Path(base path=w417, name or relative path="Power Pattern Configuration") -> (appended path=w415:path)
            n172 = call <vilib>:"Check if File or Folder Exists.vi"("error in (no error)"=w411, "path"=w415) -> ("error out"=w414:errorcluster, "file or folder exists?"=w412:bool, "dup path"=w413:path)  [unwired: 7 in]
            n173 = case shown="False" w412 {
              tunnel: w413 -> [w421 w422]
              tunnel: w414 -> [w420 w423]
              tunnel: [w419 w423] -> w410
              tunnel: [w418 w422] -> w408
              frame False {
                n174 = Create Folder(path (use dialog)=w421, error in=w420) -> (created path=w418:path, error out=w419:errorcluster)  [unwired: 1 in, 1 out]
              }
              frame True {
              }
            }
            n175 = List Folder(path=w408, error in=w410) -> (filenames=w407:string[], error out=w409:errorcluster)  [unwired: 2 in, 2 out]
            n176 = Index Array(array=w407, index=0) -> (element=w406:string)
            n177 = property on="Pattern File" class="CmbBox"(error in=w409, "Strings[]"=w407, "Val(Sgnl)"=w406) -> (error out=w403:errorcluster)  [unwired: 1 in, 1 out]
            n178 = property on="Power" class="Bool (strict)"(error in=w403, "Val(Sgnl)"=FALSE ("Power")) -> (error out=w402:errorcluster)  [unwired: 1 in, 1 out]
          }
          frame "Channels" {
            n179 = Variant To Data(error in=w430, type=T19 [] ("NewVal"), Variant=w429) -> (data=w426:T19, error out=w425:errorcluster)
            n180 = control-ref of="Profile Chart"() -> (w428:refnum<vi>)
            n181 = for {
              tunnel: w428 -> [w434]
              tunnel: w426 -> [w433] mode=indexing
              i -> [w432]
              n182 = Unbundle By Name(w433) -> ("Axis"=w439:u32, "Color Box"=w438:u32, "Run"=w437:bool, "Channel Name"=w431:string)
              n183 = To Unsigned Long Integer(number=w432) -> (unsigned 32bit integer=w435:u32)
              n184 = To Unsigned Long Integer(number=w439) -> (unsigned 32bit integer=w440:u32)
              n185 = property class="WFChart (strict)"(reference=w434, "Plot.YScaleIdx"=w440, "Plot.Plot Color"=w438, "Plot.Visible?"=w437, "Plot.Plot Name"=w431, "Plot.Line Width"=u8 2, "Active Plot"=w435) -> ()  [unwired: 1 in, 2 out]
            }
          }
        }
      }
      frame "UI:Update" {
        n186 = stacked-sequence {
          tunnel: w441 -> [w446 w471 w495 w517 w569 w583 w635]
          tunnel: w444 -> [_ _ _ _ w566 _ _]
          tunnel: [_ _ _ _ w566 _ _] -> w443
          tunnel: w441 -> [_ _ _ w521 _ _ _]
          tunnel: [_ _ _ w520 _ _ _] -> w442
          frame #0 {
            n187 = Unbundle By Name(w446) -> ("Dataset.System Status"=w445:T31)
            n188 = Unbundle By Name(w445) -> ("SOM Status.CPU Usage"=→"CPU%":dbl, "Compressor Hours"=→"Compressor Hours":dbl, "Serial Number"=w464:string, "Cascade Extra.High Side RPM"=w459:dbl, "Cascade Extra.Low Side RPM"=w461:dbl, "SOM Status.SD card free space"=w456:dbl)
            n189 = Unbundle By Name(w445) -> ("Compression Ratio"=w453:dbl, "Compressor Amps"=w452:dbl, "Discharge Pressure"=w451:dbl, "Suction Pressure"=w450:dbl, "SubCooling"=w449:dbl, "SuperHeat"=w448:dbl)
            n190 = Bundle By Name(cluster=T9 {"Condensing Pressure(psi)"=0.0, "Compression Ratio"=0.0, "Subcool"=0.0, "Superheat"=0.0, "Current(A)"=0.0, "Suction Pressure(psi)"=0.0} ("Gauges"), "Compression Ratio"=w453, "Current(A)"=w452, "Condensing Pressure(psi)"=w451, "Suction Pressure(psi)"=w450, "Subcool"=w449, "Superheat"=w448) -> (→"Gauges":T9)
            n191 = Divide(x=w456, y=1000.0) -> (x/y=→"Free Memory (MB)":dbl)
            n192 = Decimal String To Number(string=w464) -> (number=→"Serial number":i32)  [unwired: 2 in, 1 out]
            n193 = Round To Nearest(number=w461) -> (nearest integer value=→"Low Side RPM":dbl)
            n194 = Round To Nearest(number=w459) -> (nearest integer value=→"High Side RPM":dbl)
            n195 = Unbundle By Name(w445) -> ("Power On Off"=→"Play/Pause" →"Compressor":bool)
          }
          frame #1 {
            n196 = Unbundle By Name(w471) -> ("Dataset.M1 Status"=w479:T32, "Dataset.M1 Status.Thermal State"=→"Thermal State":u16, "Dataset.M1 Status.Power Drive"=→"PowerDrive":bool, "Dataset.Config Data.Set Point Range"=w481:cluster{"Max":dbl, "Min":dbl})
            n197 = Unbundle By Name(w471) -> ("Dataset.System Status.M1 Bin.Bin String"=→"Bin String":string, "Dataset.System Status.M1 Bin.Bin Color"=w469:u16)
            n198 = Unbundle By Name(w479) -> ("AC Load Watts"=→"AC Load":dbl, "Case Temp"=w480:dbl, "Set Temp"=w478:dbl, "Power Drive"=w477:bool, "Feedback"=w475:u8)
            "Feedback 2" <- w475
            n199 = case shown="1" w469 {
              tunnel: [u32 14342874 u32 16777215 u32 16712704 u32 56399 u32 1185791 u32 2818010 u32 15701504] -> w472
              frame 0, Default {
              }
              frame 1 {
              }
              frame 2 {
              }
              frame 3 {
              }
              frame 4 {
              }
              frame 5 {
              }
              frame 6 {
              }
            }
            n200 = Unbundle By Name(w481) -> ("Max"=w468:dbl, "Min"=w467:dbl)
            n201 = property on="Bin String" class="Str"("Text.BGColor"=w472) -> ()  [unwired: 2 in, 2 out]
            n202 = Bundle By Name(cluster=T4 {"Case Temp"=0.0, "Evap Temp"=0.0, "Heater %"=0.0, "EEV Steps"=0, "Set Temp"=0.0, "Feedback"=0, "Power Drive"=FALSE, "Piston Volts"=0.0, "Safe Temp"=FALSE, "Power"=FALSE, "Thermal State"=enum."Ramp Up", "Error"=FALSE, "In tollerance"=FALSE, "Head State"=enum."Disabled", "Piston Force"=0.0, "Package"=""} ("M1 Status"), "Case Temp"=w480, "Set Temp"=w478, "Power Drive"=w477, "Feedback"=w475) -> (→"M1 Status":T4)
            n203 = property on="M1 Set Temp" class="DigNum (strict)"("Maximum"=w468, "Minimum"=w467) -> ()  [unwired: 2 in, 2 out]
          }
          frame #2 {
            # "#Jung 1/6/2021"
            n204 = Unbundle By Name(w495) -> ("Core.Current VI"=w494:refnum<vi>)
            n205 = Unbundle By Name(w495) -> ("Dataset.M1 Status.Head State"=→"M1 Head State":u16, "Dataset.System Status.Power On Off"=w509:bool, "Dataset.System Status.Discharge Temp"=w507:dbl, "Dataset.System Status.Liquid Temp"=w506:dbl, "Dataset.System Status.Suction Temp"=w505:dbl, "Dataset.System Status.Ambient Temp"=w504:dbl, "Dataset.System Status.Sleep"=w503:bool, "Dataset.System Status.System Status"=w502:u16, "Dataset.System Status.M1 Actuated"=w501:bool, "Dataset.System Status.Sleep Timer"=w500:dbl, "Dataset.System Status.M1 Bin"=w499:cluster{"Bin String":string, "Bin Color":u16}, "Dataset.System Status.SOM Status.Software Version"=w497:string)
            n206 = property class="VI"(reference=w494) -> ("Description"=w492:string)  [unwired: 1 in, 2 out]
            n207 = Format Into String(format string=" %s\\n", w492) -> (resulting string=→"GUI Version":string)  [unwired: 2 in, 1 out]
            n208 = Bundle By Name(cluster=T18 {"Power On Off"=FALSE, "Compressor Temp"=0.0, "Condensor Temp"=0.0, "Suction Temp"=0.0, "Ambient Temp"=0.0, "Sleep"=FALSE, "System Status"=enum."Sleep", "M1 Actuated"=FALSE, "Sleep Timer"=0.0, "M1 Bin"={"Bin String"="", "Bin Color"=enum."White"}, "SW Version"=""} ("System Status 2"), "Power On Off"=w509, "Compressor Temp"=w507, "Condensor Temp"=w506, "Suction Temp"=w505, "Ambient Temp"=w504, "Sleep"=w503, "System Status"=w502, "M1 Actuated"=w501, "Sleep Timer"=w500, "M1 Bin"=w499, "SW Version"=w497) -> (→"System Status":T18)
          }
          frame #3 {
            n209 = Unbundle By Name(w517) -> ("Dataset.M1 Status"=w526:T32)
            n210 = Unbundle By Name(w526) -> ("Evap Temp"=w522:dbl, "Case Temp"=w516:dbl, "TSD Temp"=w519:dbl, "DC Load Watts"=w518:dbl, "Set Temp"=w510:dbl)
            n211 = Build Array(w522, w516, w519, w518) -> (w512:dbl[])
            n212 = case shown="True" "Average Graph" {
              tunnel: w521 -> [w530 w544]
              tunnel: [w530 w553] -> w520
              tunnel: w517 -> [_ w551]
              tunnel: w512 -> [w532 w548]
              tunnel: w510 -> [w531 w547]
              tunnel: [w528 w545] -> w514
              frame False {
                n213 = Insert Into Array(array=w532, index=0, new element=w531) -> (w527:dbl[])
                n214 = Get Date/Time In Seconds() -> (seconds since 1Jan1904=w529:timestamp)
                n215 = for {
                  tunnel: w529 -> [w537]
                  tunnel: [w536] -> w528 mode=indexing
                  tunnel: w527 -> [w535] mode=indexing
                  n216 = Build Array(w535) -> (w534:dbl[])
                  n217 = Bundle By Name("Y"=w534, "t0"=w537) -> (w536:waveform(dbl))  [unwired: 1 in]
                }
              }
              frame True {
                n218 = Unbundle By Name(w551) -> ("M1 Original Temps"=w552:dbl[][])
                n219 = Build Array (concatenate)(w552, w548) -> (w543:dbl[][])
                n220 = Transpose 2D Array(2D array=w543) -> (transposed array=w540:dbl[][])
                n221 = Array Subset(array=w540, index (row)=0 ("index"), length (row)=1000 ("index")) -> (w539:dbl[][])  [unwired: 2 in]
                n222 = for {
                  tunnel: w539 -> [w559] mode=indexing
                  tunnel: [w558] -> w550 mode=indexing
                  n223 = call-poly <vilib>:"Mean.vi"("X"=w559) -> ("mean"=w558:dbl)  [unwired: 1 out]
                }
                n224 = Insert Into Array(array=w550, index=0, new element=w547) -> (w538:dbl[])
                n225 = Get Date/Time In Seconds() -> (seconds since 1Jan1904=w546:timestamp)
                n226 = for {
                  tunnel: w538 -> [w555] mode=indexing
                  tunnel: w546 -> [w557]
                  tunnel: [w556] -> w545 mode=indexing
                  n227 = Build Array(w555) -> (w554:dbl[])
                  n228 = Bundle By Name("Y"=w554, "t0"=w557) -> (w556:waveform(dbl))  [unwired: 1 in]
                }
                n229 = Bundle By Name(cluster=w544, "M1 Original Temps"=w543) -> (w553:T24)
              }
            }
            "Main Chart" <- w514
            "Profile Chart" <- w514
            n230 = Insert Into Array(array=w512, index=0, new element=w510) -> (→"M1 Channels" →"M1 Profile Channels":dbl[])
            n231 = Array Max & Min(array=w512) -> (max value=w525:dbl, min value=w524:dbl)  [unwired: 2 out]
            n232 = case shown="True" "Autoscale graph" {
              tunnel: w525 -> [_ w560]
              tunnel: w524 -> [_ w561]
              frame False {
              }
              frame True {
                n233 = Add(x=w560, y="Y-axis range") -> (x+y=w563:dbl)
                n234 = Subtract(x=w561, y="Y-axis range") -> (x-y=w564:dbl)
                n235 = property on="Main Chart" class="WFChart (strict)"("YScale.Maximum"=w563, "YScale.Minimum"=w564, "YScale.ScaleFit"=u8 0 ("Y Scale.Scale Fit")) -> ()  [unwired: 2 in, 2 out]
              }
            }
          }
          frame #4 {
            n236 = Unbundle By Name(w569) -> ("Dataset.System Status.Serial Number"=w572:string)
            n237 = local read "Errors"() -> (w575:string[])
            n238 = Array Size(array=w575) -> (size(s)=w578:i32)
            n239 = Index Array(array=w575, index=w578) -> (element=w574:string)
            n240 = Concatenate Strings("Cobra Warning: Serial number", w572, w574) -> (w573:string)
            n241 = call "Is Value Changed.vim"("value"="Email Test") -> ("changed or first call?"=w577:bool)
            n242 = And(x="Email Test", y=w577) -> (x .and. y?=w568:bool)
            n243 = case shown="True" w568 {
              tunnel: "Email recipeints" -> [_ w581]
              tunnel: "Testing" ("Subject") -> [_ w580]
              tunnel: w573 -> [_ w579]
              frame False {
              }
              frame True {
                n244 = call "Send Email to Multiple.vi"("Message"=w579, "Subject"=w580, "To:"=w581) -> ()  [unwired: 9 in]
              }
            }
          }
          frame #5 {
            # "Display module and sytem graphs on Graph tab"
            n245 = Unbundle By Name(w583) -> ("Dataset.M1 Status.Case Temp"=w587:dbl, "Dataset.M1 Status.Evap Temp"=w588:dbl, "Dataset.M1 Status.Heater %"=w589:dbl, "Dataset.M1 Status.EEV Steps"=w585:u32)
            n246 = To Double Precision Float(number=w585) -> (double precision float=w586:dbl)
            n247 = Unbundle By Name(w583) -> ("Dataset.System Status.Bypass Steps"=w595:u16, "Dataset.System Status.Discharge Temp"=w594:dbl, "Dataset.System Status.Liquid Temp"=w593:dbl, "Dataset.System Status.Suction Temp"=w592:dbl, "Dataset.System Status.Ambient Temp"=w591:dbl)
            n248 = Bundle By Name(cluster=T8 {"Case Temp"=0.0, "Evap Temp"=0.0, "Heater Power (%)"=0.0, "EEV Steps"=0.0, "M1 AC Load(W)"=nan} ("M1 Temp Graphs"), "Case Temp"=w587, "Evap Temp"=w588, "Heater Power (%)"=w589, "EEV Steps"=w586) -> (→"M1 Temp Graphs":T8)
            n249 = local read "Graph Temp Unit"() -> (w582:bool)
            n250 = To Double Precision Float(number=w595) -> (double precision float=w597:dbl)
            n251 = case shown="True" w582 {
              tunnel: w594 -> [w606 w616]
              tunnel: w593 -> [w605 w615]
              tunnel: w592 -> [w604 w614]
              tunnel: w591 -> [w603 w613]
              tunnel: [w606 w610] -> w601
              tunnel: [w605 w609] -> w600
              tunnel: [w604 w608] -> w599
              tunnel: [w603 w607] -> w598
              frame False {
              }
              frame True {
                # "(°F - 32) × 5/9 => °C"
                n252 = Build Array(w616, w615, w614, w613) -> (w612:dbl[])
                n253 = for {
                  tunnel: w612 -> [w623] mode=indexing
                  tunnel: [w617] -> w611 mode=indexing
                  n254 = Subtract(x=w623, y=32.0) -> (x-y=w621:dbl)
                  n255 = Divide(x=5.0, y=9.0) -> (x/y=w618:dbl)
                  n256 = Multiply(x=w621, y=w618) -> (x*y=w617:dbl)
                }
                n257 = Index Array(array=w611) -> (element #1=w610:dbl, element #2=w609:dbl, element #3=w608:dbl, element #4=w607:dbl)  [unwired: 4 in]
              }
            }
            n258 = Bundle By Name(cluster=T7 {"Ambient Temp"=0.0, "Suction Temp"=0.0, "Condensor Temp"=0.0, "Discharge Temp"=0.0, "Bypass Steps"=0.0} ("System Graphs"), "Bypass Steps"=w597, "Discharge Temp"=w601, "Condensor Temp"=w600, "Suction Temp"=w599, "Ambient Temp"=w598) -> (→"System Graphs":T7)
          }
          frame #6 {
            n259 = Unbundle By Name(w635) -> ("Dataset.Config Data.Packages.DUT Names"=w629:T46, "IP Address"=w634:string, "Network Connection"=w636:bool)
            n260 = Unbundle By Name(w635) -> ("Dataset.M1 Status"=w637:T32)
            n261 = Unbundle By Name(w637) -> ("Package"=w630:string, "Set Temp"=w626:dbl, "Case Temp"=→"Case Temp":dbl, "Piston Force"=→"Force(lbf)":dbl)
            "Package" <- w630
            "Set Temp" <- w626
            n262 = call "Is Value Changed.vim"("value"=w634) -> ("changed or first call?"=w633:bool)
            n263 = call "Is Value Changed.vim"("value"=w636) -> ("changed or first call?"=w627:bool)
            n264 = Cluster To Array(cluster=w629) -> (array=w628:string[])
            n265 = Or(x=w633, y=w627) -> (x .or. y?=w632:bool)
            n266 = case shown="True" w632 {
              tunnel: w630 -> [_ w643]
              tunnel: w628 -> [_ w642]
              tunnel: w626 -> [_ w639]
              frame False {
              }
              frame True {
                n267 = Search 1D Array(1D array=w642, element=w643) -> (index of element=w640:i32)  [unwired: 1 in]
                n268 = Bundle By Name(cluster=T5 {"M1 Feedback"=1, "M1 Package"=0, "M1 Enable"=FALSE, "M1 Set Temp"=0.0} ("M1 Commands"), "M1 Package"=w640, "M1 Set Temp"=w639) -> (w638:T5)
                n269 = property on="M1 Commands" class="Clust (strict)"("Value"=w638) -> ()  [unwired: 2 in, 2 out]
              }
            }
            n270 = control-ref of="M1 Package"() -> (w631:refnum<vi>)
            n271 = property class="Ring (strict)"(reference=w631, "Strings []"=w628) -> ()  [unwired: 1 in, 2 out]
          }
        }
      }
      frame "UI:Update Network Down Data" {
        # "Keep RT status if not change"
        n272 = Unbundle By Name(w649) -> ("Dataset"=w652:T30)
        n273 = Unbundle By Name(w649) -> ("Dataset.Config Data.Packages.DUT Names"=w647:T46)
        n274 = Unbundle By Name(w652) -> ("System Status.Power On Off"=w654:bool, "Config Data"=w653:T34, "System Status.M1 Actuated"=w659:bool, "M1 Status"=w658:T32)
        n275 = Unbundle By Name(w658) -> ("Set Temp"=w655:dbl, "Power Drive"=w656:bool, "Feedback"=w657:u8, "Package"=w646:string)
        n276 = Cluster To Array(cluster=w647) -> (array=w648:string[])
        n277 = Search 1D Array(1D array=w648, element=w646) -> (index of element=w645:i32)  [unwired: 1 in]
        n278 = Bundle By Name(cluster=T40 {"Set Temp"=0.0, "Power Drive"=FALSE, "Feedback"=0, "Package"=0, "Enable"=FALSE} ("Network Data Down.M1 Commands"), "Enable"=w659, "Set Temp"=w655, "Power Drive"=w656, "Feedback"=w657, "Package"=w645) -> (w660:T40)
        n279 = Bundle By Name(cluster=w649, "Network Data Down.System Power On Off"=w654, "Network Data Down.Config Data"=w653, "Network Data Down.M1 Commands"=w660) -> (w650:T24)
      }
      frame "UI:Visibility" {
        n280 = stacked-sequence {
          tunnel: w662 -> [w681 w695 w711]
          frame #0 {
            # "#Jung 1/4/2021"
            # "#Jung 1/4/2021"
            n281 = Unbundle By Name(w681) -> ("Network Connection"=w670:bool, "Dataset.M1 Status.Case Temp"=w680:dbl, "Dataset.M1 Status.Evap Temp"=w679:dbl, "Dataset.System Status.Power On Off"=w671:bool, "Dataset.M1 Status.AC Load Watts"=w668:dbl)
            n282 = Equal To 0?(x=w679) -> (x = 0?=w677:bool)
            n283 = Not A Number/Path/Refnum?(number/path/refnum=w668) -> (NaN/Path/Refnum?=w667:bool)
            n284 = Equal To 0?(x=w680) -> (x = 0?=w678:bool)
            n285 = local read "M1 Channels"() -> (w675:dbl[])
            n286 = And(x=w678, y=w677) -> (x .and. y?=w676:bool)
            n287 = Not(x=w676) -> (.not. x?=w672:bool)
            n288 = Not(x=w667) -> (.not. x?=w673:bool)
            n289 = Compound Arithmetic op=AND(w670, w672) -> (w663:bool)
            n290 = Index Array(array=w675, index=3) -> (element=w666:dbl)
            n291 = Compound Arithmetic op=AND(w663, w671, w673) -> (w669:bool)
            n292 = Not A Number/Path/Refnum?(number/path/refnum=w666) -> (NaN/Path/Refnum?=w665:bool)
            n293 = Not(x=w665) -> (.not. x?=w664:bool)
            n294 = stacked-sequence {
              tunnel: w663 -> [w682 w684 w685 w686 w688]
              tunnel: w664 -> [_ _ _ _ w689]
              tunnel: w669 -> [w683 _ _ _ _]
              frame #0 {
                n295 = property on="AC Load" class="WFChart (strict)"("Visible"=w683) -> ()  [unwired: 2 in, 2 out]
                n296 = property on="M1 Temp Graphs" class="Clust (strict)"("Visible"=w682) -> ()  [unwired: 2 in, 2 out]
                n297 = property on="Compressor" class="Bool (strict)"("Visible"=w682) -> ()  [unwired: 2 in, 2 out]
                n298 = property on="System Graphs" class="Clust (strict)"("Visible"=w682) -> ()  [unwired: 2 in, 2 out]
              }
              frame #1 {
                n299 = property on="Main Chart" class="WFChart (strict)"("Visible"=w684) -> ()  [unwired: 2 in, 2 out]
                n300 = property on="M1 Status" class="Clust (strict)"("Visible"=w684) -> ()  [unwired: 2 in, 2 out]
                n301 = property on="Bin String" class="Str"("Visible"=w684) -> ()  [unwired: 2 in, 2 out]
                n302 = property on="Play/Pause" class="Bool"("Visible"=w684) -> ()  [unwired: 2 in, 2 out]
                n303 = property on="Power On-Off" class="Bool"("Visible"=w684) -> ()  [unwired: 2 in, 2 out]
              }
              frame #2 {
                n304 = property on="Case Temp" class="DigNum (strict)"("Visible"=w685) -> ()  [unwired: 2 in, 2 out]
                n305 = property on="Package" class="Str"("Visible"=w685) -> ()  [unwired: 2 in, 2 out]
                n306 = property on="M1 Commands" class="Clust (strict)"("Visible"=w685) -> ()  [unwired: 2 in, 2 out]
                n307 = property on="M1 Channels" class="Arr (strict)"("Visible"=w685) -> ()  [unwired: 2 in, 2 out]
                n308 = property on="Force(lbf)" class="DigNum (strict)"("Visible"=w685) -> ()  [unwired: 2 in, 2 out]
                n309 = property on="Feedback 2" class="Ring (strict)"("Visible"=w685) -> ()  [unwired: 2 in, 2 out]
              }
              frame #3 {
                n310 = property on="Set Temp" class="DigNum (strict)"("Visible"=w686) -> ()  [unwired: 2 in, 2 out]
                n311 = property on="Stack light states" class="Enum (strict)"("Visible"=w686) -> ()  [unwired: 2 in, 2 out]
                n312 = property on="Gauges" class="Clust (strict)"("Visible"=w686) -> ()  [unwired: 2 in, 2 out]
                n313 = property on="M1 Humidity" class="WFChart (strict)"("Visible"=w686) -> ()  [unwired: 2 in, 2 out]
              }
              frame #4 {
                n314 = And(x=w689, y=w688) -> (x .and. y?=w687:bool)
                n315 = property on="M1 Heater output" class="DigNum (strict)"("Visible"=w688) -> ()  [unwired: 2 in, 2 out]
                n316 = property on="Checkbox" class="Bool (strict)"("Visible"=w688) -> ()  [unwired: 2 in, 2 out]
                n317 = property on="Checkbox 2" class="Bool (strict)"("Visible"=w688) -> ()  [unwired: 2 in, 2 out]
                n318 = property on="Thermal Diode Feedback" class="Bool (strict)"("Visible"=w687) -> ()  [unwired: 2 in, 2 out]
              }
            }
          }
          frame #1 {
            # "#Jung 1/4/2021"
            n319 = Unbundle By Name(w695) -> ("Dataset.M1 Status.Safe Temp"=w694:bool, "Dataset.Config Data.Piston Settings.Diameter (mm)"=w700:dbl, "Dataset.M1 Status.Head State"=w698:u16)  [unwired: 1 out]
            n320 = Unbundle By Name(w695) -> ("Network Connection"=w692:bool)
            n321 = Compound Arithmetic op=AND(w692, w694) -> (w691:bool)
            n322 = Greater Than 0?(x=w700) -> (x > 0?=w701:bool)
            n323 = Not(x=w691) -> (.not. x?=w693:bool)
            n324 = property on="WAITING TO REACH SAFE TEMP" class="Bool"("Visible"=w691) -> ()  [unwired: 2 in, 2 out]
            n325 = Compound Arithmetic op=AND(w692, w693, w701) -> (w690:bool)
            n326 = property on="PowerDrive" class="Bool"("Visible"=w690) -> ()  [unwired: 2 in, 2 out]
            n327 = property on="M1 Power Drive" class="Bool (strict)"("Visible"=w690) -> ()  [unwired: 2 in, 2 out]
            n328 = Equal?(x=w698, y=enum16{"Disabled", "Run", "Error"}."Disabled" ("x")) -> (x = y?=w696:bool)
            n329 = And(x=w692, y=w696) -> (x .and. y?=w699:bool)
            n330 = property on="THERMAL HEAD  DISABLED" class="Bool"("Visible"=w699) -> ()  [unwired: 2 in, 2 out]
          }
          frame #2 {
            # "#Jung 1/5/2021"
            n331 = Unbundle By Name(w711) -> ("Dataset.System Status.Compressor Amps"=w706:dbl, "Dataset.System Status.Power On Off"=w705:bool, "Dataset.Config Data.System Settings.Cascade"=w708:bool)
            n332 = Round To Nearest(number=w706) -> (nearest integer value=w709:dbl)
            n333 = Not Equal To 0?(x=w709) -> (x != 0?=w707:bool)
            n334 = Or(x=w707, y=w705) -> (x .or. y?=w710:bool)
            n335 = property on="Thermal State" class="Enum (strict)"("Visible"=w710) -> ()  [unwired: 2 in, 2 out]
            n336 = control-ref of="Subcool"() -> (w703:refnum<vi>)
            n337 = And(x=w705, y=w708) -> (x .and. y?=w702:bool)
            n338 = property class="Knob (strict)"(reference=w703, "Visible"=w702) -> ()  [unwired: 1 in, 2 out]
            n339 = property on="High Side RPM" class="DigNum (strict)"("Visible"=w702) -> ()  [unwired: 2 in, 2 out]
            n340 = property on="Low Side RPM" class="DigNum (strict)"("Visible"=w702) -> ()  [unwired: 2 in, 2 out]
            n341 = property on="Cascade Compressor controls" class="Clust (strict)"("Visible"=w702) -> ()  [unwired: 2 in, 2 out]
            n342 = control-ref of="Superheat"() -> (w704:refnum<vi>)
            n343 = property class="Knob (strict)"(reference=w704, "Visible"=w702) -> ()  [unwired: 1 in, 2 out]
          }
        }
      }
      frame "----------MACRO----------" {
        # "MACRO is used for groups of cases that need to be run together."
      }
      frame "MACRO:Initialize" {
        # "1. Initialize Core Data\n2. Set Front Panel State\n3. Detect the available systems"
        # "3."
        # "2."
        # "1."
        # "Send initialize sequence of commands"
        n344 = Variant To Data(error in=w729, type=FALSE ("Log Events?"), Variant=w727) -> (data=w725:bool, error out=w728:errorcluster)
        n345 = call "Messaging EnQ Single.vi"("Command"="SYS:Initialize", "error in (no error)"=w728) -> ("error out"=w721:errorcluster)  [unwired: 9 in]
        n346 = Select(t="Open", s=w725, f="Close") -> (s? t:f=w722:string)
        n347 = Format Into String(format string="UI:Front Panel State>>%s" ("Command"), w722) -> (resulting string=w730:string)  [unwired: 2 in, 1 out]
        n348 = call "Messaging EnQ Single.vi"("Command"=w730, "error in (no error)"=w721) -> ("error out"=w716:errorcluster)  [unwired: 9 in]
        n349 = call "Messaging EnQ Single.vi"("Command"="NS:Detect Systems", "error in (no error)"=w716) -> ("error out"=w715:errorcluster)  [unwired: 9 in]
        n350 = Concatenate Strings("UI:Update Pages>>" ("Command"), "Initialize Test" ("Command")) -> (w718:string)
        n351 = call "Messaging EnQ Single.vi"("Command"=w718, "error in (no error)"=w715) -> ("error out"=w717:errorcluster)  [unwired: 9 in]
      }
      frame "MACRO:NS Update" {
        # "Add the commands of WEB:Open Session and WEB:Close Session if it will be possible to control PS at RT"
        n352 = call "Messaging EnQ Single.vi"("Command"="NS:Close Connection" ("Command(s)"), "error in (no error)"=w750) -> ("error out"=w749:errorcluster)  [unwired: 9 in]
        n353 = call "Messaging EnQ Single.vi"("Command"="NS:Update IP", "Data"=w753, "error in (no error)"=w749) -> ("error out"=w751:errorcluster)  [unwired: 8 in]
        n354 = call "Messaging EnQ Multiline String.vi"("Command(s)"="NS:Open Connection", "error in (no error)"=w751) -> ("error out"=w735:errorcluster)  [unwired: 9 in]
        n355 = Bundle("Page array"=i32[] [], "Visible"=FALSE) -> (w739:cluster{"Page array":i32[], "Visible":bool})  [unwired: 1 in]
        n356 = To Variant(anything=w739) -> (Variant=w742:variant)
        n357 = To Variant(anything="°F" ("Command")) -> (Variant=w737:variant)
        n358 = Build Array(w742, w737) -> (w736:variant[])
        n359 = for {
          tunnel: "UI:Update Pages>>" ("Command") -> [w757]
          tunnel: string[] ["Enable Pages", "Reinitialize Graph", "", "", ""] -> [w756] mode=indexing
          tunnel: [w755] -> w743 mode=indexing
          n360 = Concatenate Strings(w757, w756) -> (w755:string)
        }
        n361 = call "Messaging EnQ Multiple.vi"("[Commands]"=w743, "[Data]"=w736, "error in (no error)"=w735) -> ("error out"=w746:errorcluster)  [unwired: 8 in]
      }
      frame "MACRO:Shutdown" {
        (unwired) "UI:Front Panel State>>Close"
        # "Add later"
        # "Shutdown Process\n1. Stop Event Loop\n2. Stop Test\n    - TTV\n    - Profile\n3. Disconnection of Network Stream\n4. Disconnection of Network Shared Variable\n5. Close Front Panel\n6. Logging, Stop Queue, and Exit"
        # "List of commands to send for shutting down."
        n362 = Unbundle By Name(w775) -> ("TTV Test.OutputState"=w774:bool)
        n363 = Concatenate Strings("APP:TTV Test>>Stop Test" ("Command"), "\r") -> (w768:string)
        n364 = Select(t=w768, s=w774, f="") -> (s? t:f=w763:string)
        n365 = Unbundle By Name(w775) -> ("Profile.Profile Temp"=w772:bool)
        n366 = Concatenate Strings("APP:Temp Profile>>Stop Profile" ("Command"), "\r") -> (w765:string)
        n367 = Select(t=w765, s=w772, f="") -> (s? t:f=w764:string)
        n368 = Concatenate Strings(w764, w763, "NS:Close Connection\nSYS:Exit") -> (w761:string)
        n369 = call "Messaging EnQ Multiline String.vi"("Command(s)"=w761, "error in (no error)"=w760) -> ("error out"=w759:errorcluster)  [unwired: 9 in]
        "Stop NSV" <- TRUE ("Stop NSV")
      }
      frame "-----------Network Stream-----------" {
        # "Deals with the Shared Variable Engine interface (network Streams)"
      }
      frame "NS:Detect Systems" {
        n370 = call <vilib>:"Find Systems.vi"("Only Installable Systems (F)"="Only Installable Systems (F)", "Device Class"="Device Class", "Detect Online Systems (T)"="Detect Online Systems (T)", "error in (no error)"=w785, "Output (Hostname and IP)"="Output (Hostname and IP)", "Include Cached Results (all)"="Include Cached Results (all)", "Session in (localhost)"="Session in (localhost)") -> ("error out"=w782:errorcluster, "Detected Systems"=w780:string[])  [unwired: 2 in, 1 out]
        "Detected Systems" <- w780
        n371 = To Unsigned Word Integer(number=0) -> (unsigned 16bit integer=w778:u16)
        n372 = property on="Menu Ring" class="Ring (strict)"(error in=w782, "Strings []"=w780, "Val(Sgnl)"=w778) -> (error out=w781:errorcluster)  [unwired: 1 in, 1 out]
        n373 = Bundle By Name(cluster=w784, "Detected Systems"=w780) -> (w783:T24)
      }
      frame "NS:Update IP" {
        (unwired) "CFX315" ("format string")
        n374 = Unbundle By Name(w801) -> ("Dataset.M1 Status.Package"=w795:string, "Detected Systems"=w799:string[])
        n375 = Variant To Data(error in=w805, type=0, Variant=w804) -> (data=w800:i32, error out=w797:errorcluster)
        n376 = Index Array(array=w799, index=w800) -> (element=w794:string)
        n377 = call "Update IP Address.vi"("error in"=w797, "Detected System"=w794, "Package Name"=w795) -> ("error out"=w796:errorcluster, "Shared Variable Address"=w792:string, "IP Address"=w793:string)  [unwired: 6 in]
        "Shared Variable Address" <- w792
        "Connected IP" <- w793
        n378 = Bundle By Name(cluster=w801, "IP Address"=w793, "Shared Variable Address"=w792, "URI Directory"="/C/TTV Test Patterns/" ("relative uri")) -> (w803:T24)
      }
      frame "NS:Open Connection" {
        # "Create NS Writer Endpoint"
        # "Create NS Reader Endpoint"
        n379 = Unbundle By Name(w821) -> ("IP Address"=w817:string)
        n380 = Format Into String(format string="%s", initial string="//" ("string"), w817) -> (resulting string=w815:string)  [unwired: 1 in, 1 out]
        n381 = Concatenate Strings(w815, "/CFX315Writer" ("string")) -> (w830:string)
        n382 = Create Network Stream Reader Endpoint(5:1000 ("timeout in ms (-1)"), 7:1 ("reader buffer size"), 8:w824, 9:cluster{"Data":variant, "Timestamp":timestamp} {"Data"=variant, "Timestamp"=timestamp(0 s since 1904-01-01)} ("Dataset"), 10:w830, 11:"GUIReader1" ("reader name")) -> (0:w823:errorcluster, 3:w820:refnum<k21>)  [unwired: 1 in]
        n383 = Bundle By Name(cluster=w821, "reader endpoint"=w820) -> (w819:T24)
        n384 = Concatenate Strings(w815, "/CFX315Reader" ("writer name")) -> (w825:string)
        n385 = Create Network Stream Writer Endpoint(5:1000 ("timeout in ms (-1)"), 7:1 ("writer buffer size"), 8:w823, 9:variant, 10:w825, 11:"GUIWriter1" ("writer name")) -> (0:w813:errorcluster, 3:w814:refnum<k21>)  [unwired: 1 in]
        n386 = Bundle By Name(cluster=w819, "writer endpoint"=w814) -> (w808:T24)
        n387 = property class="Network Stream Endpoint"(reference=w814, error in=w813) -> (error out=w812:errorcluster, "Connected"=w806:bool)  [unwired: 1 out]
        "Network Connection" <- w806
        n388 = Unbundle By Name(w808) -> ("IP Address"=w807:string)
        n389 = Not(x=w806) -> (.not. x?=w835:bool)
        n390 = case shown="True" w806 {
          tunnel: w812 -> [w839 w840]
          tunnel: [w839 w840] -> w811
          tunnel: [Save_Log_State."Idle" ("State") Save_Log_State."Write" ("State")] -> w810
          tunnel: [_ w841] -> w809
          tunnel: w807 -> [_ w843]
          frame False {
          }
          frame True {
            n391 = Concatenate Strings(w843, " Connected" ("Command")) -> (w841:string)
          }
        }
        n392 = property on="Network Connection" class="Bool (strict)"("Blinking"=w835) -> ()  [unwired: 2 in, 2 out]
        n393 = Bundle By Name(cluster=w808, "Network Connection"=w806) -> (w836:T24)
      }
      frame "NS:Close Connection" {
        n394 = Unbundle By Name(w849) -> ("reader endpoint"=w853:refnum<k21>, "writer endpoint"=w852:refnum<k21>)
        n395 = Destroy Stream Endpoint(8:w855, 11:w852) -> (0:w854:errorcluster)
        n396 = Destroy Stream Endpoint(8:w854, 11:w853) -> (0:w851:errorcluster)
        n397 = Unbundle By Name(w849) -> ("Network Connection"=w850:bool)
        n398 = call "Is Value Changed.vim"("value"=w850) -> ("changed or first call?"=w848:bool)
        n399 = case shown="True" w848 {
          tunnel: w847 -> [_ _]
          tunnel: ["" "NS Disconnection" ("Descripition")] -> w845
          tunnel: [Save_Log_State."Idle" ("State") Save_Log_State."Write" ("State")] -> w846
          frame False {
          }
          frame True {
          }
        }
      }
      frame "NS:Read" {
        n400 = Unbundle By Name(w861) -> ("reader endpoint"=w860:refnum<k21>)
        n401 = shared-variable-read(w860, w867, 1000 ("timeout ms (-1)"), cluster{"Data":variant, "Timestamp":timestamp} {"Data"=variant, "Timestamp"=timestamp(0 s since 1904-01-01)} ("Dataset")) -> (w866:errorcluster, w865:bool, w864:cluster{"Data":variant, "Timestamp":timestamp})  [unwired: 1 out]
        n402 = Unbundle By Name(w861) -> ("Dataset"=w869:T30)
        n403 = Or(x=w865, y=w866) -> (x .or. y?=w870:bool)
        n404 = case shown="False" w870 {
          tunnel: [w877 w888] -> w871
          tunnel: w861 -> [w878 w889]
          tunnel: [w874 w886] -> w868
          tunnel: w869 -> [w882 _]
          tunnel: w866 -> [w880 w891]
          tunnel: w864 -> [w881 _]
          tunnel: w860 -> [_ w890]
          frame False {
            n405 = Unbundle By Name(w881) -> ("Timestamp"=→"Data Rx Timestamp":timestamp, "Data"=w879:variant)
            n406 = Variant To Data(error in=w880, type=w882, Variant=w879) -> (data=w876:T30, error out=w875:errorcluster)
            n407 = Bundle By Name(cluster=w878, "Dataset"=w876) -> (w877:T24)
            n408 = call "Messaging EnQ Single.vi"("Command"="UI:Update Network Down Data", "@Front?"=TRUE, "error in (no error)"=w875) -> ("error out"=w874:errorcluster)  [unwired: 8 in]
          }
          frame True {
            n409 = property class="Network Stream Endpoint"(reference=w890, error in=w891) -> (error out=w887:errorcluster, "Connected"=w884:bool)  [unwired: 1 out]
            n410 = Not(x=w884) -> (.not. x?=w885:bool)
            n411 = property on="Network Connection" class="Bool (strict)"("Value"=w884, "Blinking"=w885) -> ()  [unwired: 2 in, 2 out]
            n412 = case shown="False" w884 {
              tunnel: w887 -> [w896 w897]
              tunnel: [w894 w897] -> w886
              frame False {
                n413 = call <vilib>:"Clear Errors.vi"("error in (no error)"=w896) -> ("error out"=w895:errorcluster)  [unwired: 5 in, 1 out]
                n414 = call "Messaging EnQ Multiline String.vi"("Command(s)"="NS:Close Connection\nNS:Open Connection" ("Command"), "@Front?"=TRUE, "error in (no error)"=w895) -> ("error out"=w894:errorcluster)  [unwired: 8 in]
              }
              frame True {
              }
            }
            n415 = Bundle By Name(cluster=w889, "Network Connection"=w884) -> (w888:T24)
          }
        }
      }
      frame "NS:Write" {
        n416 = Index Array(array=w917) -> (element=w905:string)  [unwired: 1 in]
        n417 = case shown="\"Update Config\"" w905 {
          tunnel: w904 -> [_ w927 w936 w945 w956 w965 w974 w983 w992 w1001 w1007 w1016 w1025]
          tunnel: w906 -> [w919 w928 w935 w944 w955 w964 w975 w984 w993 w1002 w1010 w1019 w1028]
          tunnel: [w918 w925 w933 w942 w953 w962 w972 w981 w990 w1000 w1011 w1020 w1029] -> w902
          tunnel: [w919 w926 w934 w943 w952 w963 w973 w982 w991 w999 w1009 w1018 w1027] -> w898
          tunnel: w903 -> [w918 w923 w932 w941 w951 w961 w971 w980 w989 w998 w1006 w1015 w1024]
          tunnel: [_ w921 w930 w939 w949 w960 w968 w977 w986 w995 w1004 w1013 "Download"] -> w901
          tunnel: [_ w920 w929 w938 w947 w957 w967 w976 w985 w994 w1003 w1012 w1021] -> w900
          frame Default {
          }
          frame "Power On-Off" {
            w920 = T47."System Power" ("Network Data Down.New Data")
            n418 = Variant To Data(error in=w928, type=TRUE, Variant=w927) -> (data=w922:bool, error out=w926:errorcluster)
            n419 = Bundle By Name(cluster=w923, "Network Data Down.System Power On Off"=w922, "Network Data Down.New Data"=w920) -> (w925:T24)
            n420 = Format Into String(w922) -> (resulting string=w921:string)  [unwired: 3 in, 1 out]
          }
          frame "M1 Power Drive" {
            w929 = T47."M1 Power Drive" ("Network Data Down.New Data")
            n421 = Variant To Data(error in=w935, type=TRUE, Variant=w936) -> (data=w931:bool, error out=w934:errorcluster)
            n422 = Bundle By Name(cluster=w932, "Network Data Down.M1 Commands.Power Drive"=w931, "Network Data Down.New Data"=w929) -> (w933:T24)
            n423 = Format Into String(w931) -> (resulting string=w930:string)  [unwired: 3 in, 1 out]
          }
          frame "M2 Power Drive" {
            w938 = T47."M2 Power Drive" ("Network Data Down.New Data")
            n424 = Variant To Data(error in=w944, type=TRUE, Variant=w945) -> (data=w940:bool, error out=w943:errorcluster)
            n425 = Bundle By Name(cluster=w941, "Network Data Down.M2 Commands.Power Drive"=w940, "Network Data Down.New Data"=w938) -> (w942:T24)
            n426 = Format Into String(w940) -> (resulting string=w939:string)  [unwired: 3 in, 1 out]
          }
          frame "M1 Set Temp" {
            w947 = T47."M1 Set Point" ("Network Data Down.New Data")
            n427 = Variant To Data(error in=w955, type=20.0 ("SET TEMP 1"), Variant=w956) -> (data=w950:dbl, error out=w952:errorcluster)
            n428 = Bundle By Name(cluster=w951, "Network Data Down.M1 Commands.Set Temp"=w950, "Network Data Down.New Data"=w947) -> (w953:T24)
            n429 = Format Into String(format string="%5.1f", w950) -> (resulting string=w949:string)  [unwired: 2 in, 1 out]
          }
          frame "M2 Set Temp" {
            w957 = T47."M2 Set Point" ("Network Data Down.New Data")
            n430 = Variant To Data(error in=w964, type=0.0 ("SET TEMP 1"), Variant=w965) -> (data=w959:dbl, error out=w963:errorcluster)
            n431 = Bundle By Name(cluster=w961, "Network Data Down.M2 Commands.Set Temp"=w959, "Network Data Down.New Data"=w957) -> (w962:T24)
            n432 = Format Into String(format string="%5.1f", w959) -> (resulting string=w960:string)  [unwired: 2 in, 1 out]
          }
          frame "M1 Feedback" {
            w967 = T47."M1 Feedback" ("Network Data Down.New Data")
            n433 = Variant To Data(error in=w975, type=u8 0 ("Network Data Down.M1 Commands.Feedback"), Variant=w974) -> (data=w969:u8, error out=w973:errorcluster)
            n434 = Bundle By Name(cluster=w971, "Network Data Down.M1 Commands.Feedback"=w969, "Network Data Down.New Data"=w967) -> (w972:T24)
            n435 = Format Into String(w969) -> (resulting string=w968:string)  [unwired: 3 in, 1 out]
          }
          frame "M2 Feedback" {
            w976 = T47."M2 Feedback" ("Network Data Down.New Data")
            n436 = Variant To Data(error in=w984, type=u8 0 ("Network Data Down.M2 Commands.Feedback"), Variant=w983) -> (data=w978:u8, error out=w982:errorcluster)
            n437 = Bundle By Name(cluster=w980, "Network Data Down.M2 Commands.Feedback"=w978, "Network Data Down.New Data"=w976) -> (w981:T24)
            n438 = Format Into String(w978) -> (resulting string=w977:string)  [unwired: 3 in, 1 out]
          }
          frame "M1 Package" {
            w985 = T47."M1 Package" ("Network Data Down.New Data")
            n439 = Variant To Data(error in=w993, type=u16 0 ("Network Data Down.M1 Commands.Package"), Variant=w992) -> (data=w987:u16, error out=w991:errorcluster)
            n440 = Bundle By Name(cluster=w989, "Network Data Down.M1 Commands.Package"=w987, "Network Data Down.New Data"=w985) -> (w990:T24)
            n441 = Format Into String(w987) -> (resulting string=w986:string)  [unwired: 3 in, 1 out]
          }
          frame "M2 Package" {
            w994 = T47."M2 Package" ("Network Data Down.New Data")
            n442 = Variant To Data(error in=w1002, type=u16 0 ("Network Data Down.M2 Commands.Package"), Variant=w1001) -> (data=w996:u16, error out=w999:errorcluster)
            n443 = Bundle By Name(cluster=w998, "Network Data Down.M2 Commands.Package"=w996, "Network Data Down.New Data"=w994) -> (w1000:T24)
            n444 = Format Into String(w996) -> (resulting string=w995:string)  [unwired: 3 in, 1 out]
          }
          frame "M1 Enable" {
            w1003 = T47."M1 Enable" ("Network Data Down.New Data")
            n445 = Variant To Data(error in=w1010, type=TRUE, Variant=w1007) -> (data=w1005:bool, error out=w1009:errorcluster)
            n446 = Bundle By Name(cluster=w1006, "Network Data Down.M1 Commands.Enable"=w1005, "Network Data Down.New Data"=w1003) -> (w1011:T24)
            n447 = Format Into String(w1005) -> (resulting string=w1004:string)  [unwired: 3 in, 1 out]
          }
          frame "M2 Enable" {
            w1012 = T47."M2 Enable" ("Network Data Down.New Data")
            n448 = Variant To Data(error in=w1019, type=TRUE, Variant=w1016) -> (data=w1014:bool, error out=w1018:errorcluster)
            n449 = Bundle By Name(cluster=w1015, "Network Data Down.M2 Commands.Enable"=w1014, "Network Data Down.New Data"=w1012) -> (w1020:T24)
            n450 = Format Into String(w1014) -> (resulting string=w1013:string)  [unwired: 3 in, 1 out]
          }
          frame "Update Config" {
            w1021 = T47."Config Data" ("Network Data Down.New Data")
            w1023 = T34 {"Packages"={"DUT Force lbf"={" 0"=0, " 1"=0, " 2"=0, "3"=0, "4"=0, "5"=0, " 6"=0, "7"=0, "8"=0, "9"=0}, "DUT Names"={"0"="", "1"="", "2"="", "3"="", "4"="", "5"="", "6"="", "7"="", "8"="", "9"=""}}, "Heater PID"={"P"=0.0, "I"=0.0, "D"=0.0}, "Piston Settings"={"Forces Slope"=0.0, "Forces Intercept"=0.0, "Transition Force"=0.0, "Up Force"=0.0, "Diameter (mm)"=0.0, "Delay (ms)"=0.0, "Pressure Ramp Delay (ms)"=0.0}, "Safe Temps"={"Minimum"=17, "Enabled"=TRUE, "Maximum"=95}, "System Settings"={"Number of Heads"=0, "60Hz Power"=TRUE, "FTC200"=TRUE, "AutoStartup"=FALSE, "Purge"=TRUE, "Sensors"=TRUE, "HandClamp"=TRUE, "ATE"=TRUE, "Benchtop"=TRUE, "Production"=TRUE, "Refrigerant"=0, "Handler"=TRUE, "Shuttle"=TRUE, "220V"=FALSE, "Cascade"=FALSE, "Suction Sensor"=0, "Discharge Sensor"=0}, "Stepper Settings "={"Microstepping"=0, "Velocity"=8}, "Set Point Range"={"Max"=0.0, "Min"=0.0}, "Pedestal Check DeltaT"=0.0, "Ramp Delta T"=0.0, "Ramp-SS Threshold"=0.0, "SS Tolerance"=0.0, "EEV PID"={"Ramp Up Target"=0.0, "Ramp Down Target"=0.0, "Steady State Target"=0.0, "Output"={"Max"=0.0, "Min"=0.0}, "EBB and Flow Temp TH"=0.0, "Cryomode EEV Max"=0.0, "Valve minimum opening "=0.0, "Ramp Up EEV Steps"=0.0, "Ramp Down EEV Steps"=0.0, "SS EEV Steps Reset"=0.0, "EBB and Flow Tol"=0.0, "Gains"={"P"=0.0, "I"=0.0, "D"=0.0}, "Dissabled Target"=0.0, "CryoMode Gains"={"P"=0.0, "I"=0.0, "D"=0.0}, "M1 SuperHeat Setpoint"=0.0, "M2 Gains"={"P"=0.0, "I"=0.0, "D"=0.0}, "Flow Curve"=0}, "Sleep Timeout"=0.0, "Bypass Values"={"Bypass Valve"=TRUE, "Flow Curve"=0, "Output"={"Max"=0, "Min"=0}, "Feedback"=0, "Cyth Bypass"=TRUE, "PID"={"P"=0.0, "I"=0.0, "D"=0.0}, "Pressure setpoint"=0, "Cryo Temp"=0, "Superheat Setpoint"=0, "Cryo Setpoint"=0}, "Default Temp"=0.0, "InTEC"={"Enabled"=FALSE, "IP"="192.168.1.100", "Port"=5000}, "M1 TSD"={"Gain"=0.0, "Offset"=0.0, "V Offset "=0.0}, "M2 TSD"={"Gain"=0.0, "Offset"=0.0, "V Offset "=0.0}, "M1 T-Case Calibration"={"Gain"=0.0, "Offset"=0.0}, "M2 T-Case Calibration"={"Gain"=0.0, "Offset"=0.0}, "Heater PID TSD"={"P"=0.0, "I"=0.0, "D"=0.0}, "M2 Heater PID"={"P"=0.0, "I"=0.0, "D"=0.0}}  # Config Data
            n451 = Variant To Data(error in=w1028, type=w1023, Variant=w1025) -> (data=w1026:T34, error out=w1027:errorcluster)
            n452 = Bundle By Name(cluster=w1024, "Network Data Down.Config Data"=w1026, "Network Data Down.New Data"=w1021) -> (w1029:T24)
          }
        }
        n453 = Format Into String(w900) -> (resulting string=w908:string)  [unwired: 3 in, 1 out]
        n454 = call <vilib>:"Space Constant.vi"() -> ("String"=w909:string)
        n455 = Unbundle By Name(w902) -> ("writer endpoint"=w915:refnum<k21>, "Network Data Down"=w912:T25)
        n456 = Concatenate Strings(w908, w909, w901) -> (w907:string)
        n457 = To Variant(anything=w912) -> (Variant=w911:variant)
        n458 = shared-variable-write(w915, w898, w911) -> (w914:refnum<k21>, w916:errorcluster)  [unwired: 1 in, 1 out]
        n459 = Flush Stream(8:w916, 9:0 ("timeout in ms (-1)"), 11:w914) -> (0:w913:errorcluster)  [unwired: 1 in, 2 out]
      }
      frame "NS:Update Shared Variable" {
        n460 = Unbundle By Name(w1037) -> ("IP Address"=w1036:string)
        n461 = Index Array(array=w1034) -> (element=w1033:string)  [unwired: 1 in]
        n462 = Concatenate Strings("ni.var.psp://", w1036, "/Network Shared Variables/") -> (w1035:string)
        n463 = case shown="\"M1 Heater output\"" w1033 {
          selector: w1033 -> [w1041 w1055 w1061 _ w1085 w1094]
          tunnel: w1035 -> [w1042 w1056 w1062 w1070 w1086 w1095]
          tunnel: w1032 -> [w1049 w1059 w1069 w1082 w1092 w1102]
          tunnel: w1031 -> [w1048 w1058 w1068 w1081 w1091 w1101]
          tunnel: [w1044 w1051 w1066 w1076 w1089 w1099] -> w1030
          frame "M1 EEV Manual", Default {
            n464 = Variant To Data(error in=w1049, type=u16 0 ("M1 EEV Manual"), Variant=w1048) -> (data=w1045:u16, error out=w1046:errorcluster)
            n465 = Format Into String(format string="%s", initial string=w1042, w1041) -> (resulting string=w1040:string)  [unwired: 1 in, 1 out]
            n466 = shared-variable-write(w1040, w1046, w1045) -> (w1044:errorcluster)  [unwired: 1 out]
          }
          frame "Cascade Compressor controls" {
            n467 = Variant To Data(error in=w1059, type=T15 {"High Stage manual speed control"=FALSE, "Manual High stage frequency"=0.0, "Low Stage manual speed control"=FALSE, "Manual Low Stage frequency"=0.0} ("Cascade Compressor controls"), Variant=w1058) -> (data=w1053:T15, error out=w1054:errorcluster)
            n468 = Format Into String(format string="%s", initial string=w1056, w1055) -> (resulting string=w1052:string)  [unwired: 1 in, 1 out]
            n469 = shared-variable-write(w1052, w1054, w1053) -> (w1051:errorcluster)  [unwired: 1 out]
          }
          frame "M1 Heater output" {
            n470 = Variant To Data(error in=w1069, type=0.0 ("Numeric"), Variant=w1068) -> (data=w1064:dbl, error out=w1067:errorcluster)
            n471 = Format Into String(format string="%s", initial string=w1062, w1061) -> (resulting string=w1060:string)  [unwired: 1 in, 1 out]
            n472 = shared-variable-write(w1060, w1067, w1064) -> (w1066:errorcluster)  [unwired: 1 out]
          }
          frame "Thermal Load" {
            n473 = Variant To Data(error in=w1082, type=0.0 ("Numeric"), Variant=w1081) -> (data=w1077:dbl, error out=w1075:errorcluster)
            n474 = Replace Array Subset(array=dbl[] [0.0, 0.0], new element=w1077, index=0) -> (w1074:dbl[])
            n475 = Format Into String(format string="%s", initial string=w1070, "Network Inputs" ("input 1")) -> (resulting string=w1071:string)  [unwired: 1 in, 1 out]
            n476 = shared-variable-write(w1071, w1075, w1074) -> (w1076:errorcluster)  [unwired: 1 out]
          }
          frame "Manual Bypass Mode" {
            n477 = Variant To Data(error in=w1092, type=bool[] [] ("appended array"), Variant=w1091) -> (data=w1083:bool[], error out=w1088:errorcluster)
            n478 = Format Into String(format string="%s", initial string=w1086, w1085) -> (resulting string=w1084:string)  [unwired: 1 in, 1 out]
            n479 = shared-variable-write(w1084, w1088, w1083) -> (w1089:errorcluster)  [unwired: 1 out]
          }
          frame "Thermal Diode Feedback" {
            n480 = Variant To Data(error in=w1102, type=FALSE ("TSD Feedback"), Variant=w1101) -> (data=w1097:bool, error out=w1098:errorcluster)
            n481 = Format Into String(format string="%s", initial string=w1095, w1094) -> (resulting string=w1093:string)  [unwired: 1 in, 1 out]
            n482 = shared-variable-write(w1093, w1098, w1097) -> (w1099:errorcluster)  [unwired: 1 out]
          }
        }
      }
      frame "-----------WebDAV-----------" {
      }
      frame "WEB:Open Session" {
        n483 = Unbundle By Name(w1115) -> ("IP Address"=w1116:string)
        n484 = Unbundle By Name(w1115) -> ("URI Directory"=w1105:string)
        n485 = Format Into String(format string="%s/files", initial string="http://" ("host uri prefix"), w1116) -> (resulting string=w1110:string)  [unwired: 1 in, 1 out]
        n486 = call "WebDAV FGV.vi"("WebDAV States"=WebDAV_states."Open Sess", "error in (no error)"=w1112, "host uri prefix"=w1110, "relative uri"=w1105) -> ("error out"=w1108:errorcluster, "session handle out"=w1106:T48)  [unwired: 5 in, 1 out]
        n487 = call <vilib>:"Path Info.vi"("session handle"=w1106, "relative uri"=w1105, "error in (no error)"=w1108) -> ("is directory?"=w1107:bool, "error out"=w1109:errorcluster)  [unwired: 9 in, 2 out]
        n488 = case shown="True" w1107 {
          tunnel: w1109 -> [_ w1127]
          tunnel: w1105 -> [w1122 w1126]
          tunnel: [w1121 w1130] -> w1119
          tunnel: [string[] [] w1129] -> w1114
          frame False {
            # "Don't connect the error in"
            n489 = call "WebDAV FGV.vi"("WebDAV States"=WebDAV_states."Create Dir", "relative uri"=w1122) -> ("error out"=w1121:errorcluster)  [unwired: 7 in, 2 out]
          }
          frame True {
            n490 = call "WebDAV FGV.vi"("WebDAV States"=WebDAV_states."Refresh Dir", "error in (no error)"=w1127, "relative uri"=w1126) -> ("error out"=w1128:errorcluster, "file list"=w1124:T49[])  [unwired: 6 in, 1 out]
            n491 = for {
              tunnel: w1124 -> [w1133] mode=indexing
              tunnel: [w1132] -> w1129 mode=indexing
              n492 = Unbundle By Name(w1133) -> ("display name"=w1132:string)
            }
            n493 = Index Array(array=w1129) -> (element=w1131:string)  [unwired: 1 in]
            n494 = property on="Pattern File" class="CmbBox"(error in=w1128, "Val(Sgnl)"=w1131, "Strings[]"=w1129) -> (error out=w1130:errorcluster)  [unwired: 1 in, 1 out]
          }
        }
        n495 = Bundle By Name(cluster=w1115, "File list in SoM"=w1114) -> (w1113:T24)
      }
      frame "WEB:Close Session" {
        n496 = call "WebDAV FGV.vi"("WebDAV States"=WebDAV_states."Close Sess", "error in (no error)"=w1135) -> ("error out"=w1134:errorcluster)  [unwired: 7 in, 2 out]
      }
      frame "----------- Application----------" {
      }
      frame "APP:Update Config" {
        # "Confirm Config Data modified"
        n497 = Unbundle By Name(w1149) -> ("Dataset.Config Data"=w1146:T34)
        n498 = Index Array(array=w1148) -> (element=w1147:string)  [unwired: 1 in]
        n499 = case shown="\"Config Data Setting\", Default" w1147 {
          tunnel: w1146 -> [w1155 w1159]
          tunnel: [w1151 w1162] -> w1145
          tunnel: [w1152 w1161] -> w1144
          tunnel: [w1153 w1160] -> w1143
          tunnel: w1142 -> [w1157 w1158]
          frame "Packages Setting" {
            n500 = Unbundle By Name(w1155) -> ("Packages"=w1156:T50)
            n501 = call "Modified Packages.vi"("error in"=w1157, "Pagckages in"=w1156) -> ("error out"=w1151:errorcluster, "Cancel?"=w1152:bool, "Modified Packages"=w1154:T51)  [unwired: 6 in]
            n502 = Bundle By Name(cluster=w1155, "Packages"=w1154) -> (w1153:T34)
          }
          frame "Config Data Setting", Default {
            n503 = call "Update Config Data.vi"("error in (no error)"=w1158, "Config Data Current"=w1159) -> ("error out"=w1162:errorcluster, "Canceled"=w1161:bool, "Modified Config Data"=w1160:T34)  [unwired: 7 in]
          }
        }
        n504 = case shown="False" w1144 {
          tunnel: [w1166 w1169] -> w1150
          tunnel: w1145 -> [w1167 w1169]
          tunnel: w1143 -> [w1165 _]
          tunnel: "NS:Write>>Update Config" ("Command(s)") -> [w1164 _]
          tunnel: [Save_Log_State."Write" ("State") Save_Log_State."Idle" ("State")] -> w1140
          frame False {
            n505 = call "Messaging EnQ Single.vi"("Command"=w1164, "Data"=w1165, "error in (no error)"=w1167) -> ("error out"=w1166:errorcluster)  [unwired: 8 in]
          }
          frame True {
          }
        }
      }
      frame "APP:Power Sequence(GUI)" {
        n506 = Unbundle By Name(w1170) -> ("Core.VI Path"=w1174:path)
        n507 = Strip Path(path=w1174) -> (stripped path=w1175:path)  [unwired: 1 out]
        n508 = property on="Pattern File" class="CmbBox"(error in=w1178) -> (error out=w1177:errorcluster, "Value"=w1176:string)  [unwired: 1 in, 1 out]
        n509 = Index Array(array=w1182) -> (element=w1181:string)  [unwired: 1 in]
        n510 = Build Path(base path=w1175, name or relative path="Power Pattern Configuration") -> (appended path=w1172:path)
        n511 = case shown="\"Refresh Seq\"" w1181 {
          tunnel: w1177 -> [w1199 w1232 w1239 w1248 w1308 w1320]
          tunnel: w1180 -> [w1198 w1231 _ _ _ _]
          tunnel: [w1187 w1229 w1240 w1247 w1299 w1318] -> w1179
          tunnel: w1176 -> [_ _ _ w1246 w1309 _]
          tunnel: w1172 -> [w1188 _ w1238 w1249 w1310 _]
          tunnel: w1170 -> [w1184 w1225 w1237 w1245 w1298 w1316]
          tunnel: [w1183 w1226 w1237 w1245 w1297 w1315] -> w1171
          tunnel: w1170 -> [_ _ _ w1244 _ _]
          frame "Pattern File", Default {
            n512 = Variant To Data(error in=w1199, type="", Variant=w1198) -> (data=w1190:string, error out=w1191:errorcluster)
            n513 = Build Path(base path=w1188, name or relative path=w1190) -> (appended path=w1189:path)
            n514 = Empty String/Path?(string/path=w1190) -> (empty?=w1192:bool)
            n515 = case shown="True" w1192 {
              tunnel: [w1205 T21 [] ("Power Seq out")] -> w1185
              tunnel: [w1204 w1207] -> w1193
              tunnel: [T36."Enabled" ("Disabled") T36."Disabled and Grayed Out" ("Disabled")] -> w1194
              tunnel: w1191 -> [w1202 w1207]
              tunnel: w1189 -> [w1201 _]
              frame False {
                n516 = call "Config Power Sequence.vi"("Get/Update"=enum16{"Get Seq", "Update Seq"}."Get Seq", "Error In"=w1202, "Seq file path"=w1201) -> ("Error Out"=w1204:errorcluster, "Power Seq out"=w1205:T21)  [unwired: 6 in, 1 out]
              }
              frame True {
              }
            }
            n517 = property on="Power Seq" class="Arr (strict)"(error in=w1193, "Val(Sgnl)"=w1185) -> (error out=w1186:errorcluster)  [unwired: 1 in, 1 out]
            n518 = control-ref of="Save Seq"() -> (w1197:refnum<vi>)
            n519 = property class="Bool"(reference=w1197, error in=w1186, "DisabledEnum"=w1194) -> (error out=w1195:errorcluster)  [unwired: 1 out]
            n520 = control-ref of="Delete Seq"() -> (w1196:refnum<vi>)
            n521 = Bundle By Name(cluster=w1184, "TTV Test.Power Seq"=w1185) -> (w1183:T24)
            n522 = property class="Bool"(reference=w1196, error in=w1195, "DisabledEnum"=w1194) -> (error out=w1187:errorcluster)  [unwired: 1 out]
          }
          frame "Power Sequence" {
            n523 = Variant To Data(error in=w1232, type=cluster{"Iteration No":i32, "Power Seq":T21} {"Iteration No"=0, "Power Seq"=[]} ("output cluster"), Variant=w1231) -> (data=w1217:cluster{"Iteration No":i32, "Power Seq":T21}, error out=w1215:errorcluster)
            n524 = Unbundle By Name(w1217) -> ("Iteration No"=w1216:i32, "Power Seq"=w1214:T21)
            n525 = Variant To Data(error in=w1215, type=T21 [] ("Power Seq out"), Variant=w1214) -> (data=w1212:T21, error out=w1211:errorcluster)
            n526 = Less Than 0?(x=w1216) -> (x < 0?=w1221:bool)
            n527 = case shown="True" w1221 {
              tunnel: ["" "Infinite Cycle" ("Command")] -> w1220
              tunnel: w1216 -> [w1233 _]
              tunnel: [w1233 1 ("Plot.Plot Interpolation")] -> w1219
              frame False {
              }
              frame True {
              }
            }
            "Infinite Test" <- w1220
            n528 = property on="Test Graph" class="WFChart (strict)"("History Data"=dbl[] [], "Plot.Plot Interpolation"=u8 3) -> ()  [unwired: 2 in, 2 out]
            n529 = call "Set Seqence.vi"("Error In"=w1211, "Iteration"=w1219, "Power Seq"=w1212) -> ("Error Out"=w1223:errorcluster, "Waveform Graph"=w1227:u32[])  [unwired: 7 in]
            n530 = To Double Precision Float(number=w1227) -> (double precision float=→"Test Graph":dbl[])
            n531 = Bundle By Name(cluster=w1225, "TTV Test.Power Seq"=w1212) -> (w1226:T24)
            n532 = control-ref of="Save Seq"() -> (w1228:refnum<vi>)
            n533 = property class="Bool"(reference=w1228, error in=w1223, "DisabledEnum"=T36."Enabled" ("Disabled")) -> (error out=w1229:errorcluster)  [unwired: 1 out]
          }
          frame "Refresh Seq" {
            n534 = List Folder(path=w1238, error in=w1239) -> (filenames=w1241:string[], error out=w1242:errorcluster)  [unwired: 2 in, 2 out]
            n535 = property on="Pattern File" class="CmbBox"(error in=w1242, "Strings[]"=w1241) -> (error out=w1240:errorcluster)  [unwired: 1 in, 1 out]
          }
          frame "Save Seq" {
            n536 = Unbundle By Name(w1244) -> ("TTV Test.Power Seq"=w1243:T21)
            n537 = Format Into String(format string="Overwrite it to %s", w1246) -> (resulting string=w1255:string)  [unwired: 2 in, 1 out]
            n538 = call <vilib>:"Three Button Dialog.vi"("Window Title (\"\")"="Save file (.ini)" ("Window Title (\"\")"), "Center Button Text (\"No\")"="Save as" ("Center Button Text (\"No\")"), "message"=w1255) -> ("Which Button?"=w1251:T52)  [unwired: 8 in]
            n539 = case shown="\"Center Button\"" w1251 {
              tunnel: "Enter the filename(.ini)" ("Message title") -> [_ w1284 _ _]
              tunnel: w1249 -> [w1264 w1276 _ _]
              tunnel: w1248 -> [w1261 w1278 w1294 w1295]
              tunnel: [w1257 w1274 w1294 w1295] -> w1247
              tunnel: w1246 -> [w1263 _ _ _]
              tunnel: w1243 -> [w1256 w1273 _ _]
              frame "Left Button", Default {
                n540 = Build Path(base path=w1264, name or relative path=w1263) -> (appended path=w1262:path)
                n541 = Empty String/Path?(string/path=w1263) -> (empty?=w1265:bool)
                n542 = case shown="False" w1265 {
                  tunnel: w1262 -> [w1269 w1270]
                  tunnel: w1261 -> [w1268 w1271]
                  tunnel: [w1267 w1270] -> w1258
                  tunnel: [w1266 w1271] -> w1259
                  frame False {
                    n543 = Delete(path (use dialog)=w1269, error in=w1268) -> (deleted path=w1267:path, error out=w1266:errorcluster)  [unwired: 3 in, 1 out]
                  }
                  frame True {
                  }
                }
                n544 = call "Config Power Sequence.vi"("Get/Update"=enum16{"Get Seq", "Update Seq"}."Update Seq", "Error In"=w1259, "Power Seq"=w1256, "Seq file path"=w1258) -> ("Error Out"=w1257:errorcluster)  [unwired: 5 in, 2 out]
              }
              frame "Center Button" {
                w1281 = ".ini" ("regular expression")
                n545 = call "User Input Dialog.vi"("Message title"=w1284) -> ("OK?"=w1280:bool, "Message out"=w1277:string)  [unwired: 7 in, 1 out]
                n546 = Match Pattern(string=w1277, regular expression=w1281) -> (match substring=w1283:string)  [unwired: 1 in, 3 out]
                n547 = Build Path(base path=w1276, name or relative path=w1277) -> (appended path=w1275:path)
                n548 = Equal?(x=w1283, y=w1281) -> (x = y?=w1282:bool)
                n549 = And(x=w1280, y=w1282) -> (x .and. y?=w1279:bool)
                n550 = case shown="True" w1279 {
                  tunnel: w1275 -> [_ w1293]
                  tunnel: w1278 -> [w1285 w1292]
                  tunnel: [w1285 w1290] -> w1274
                  tunnel: w1273 -> [_ w1287]
                  tunnel: enum16{"Get Seq", "Update Seq"}."Update Seq" ("Get/Update") -> [_ w1286]
                  frame False {
                  }
                  frame True {
                    n551 = call "Config Power Sequence.vi"("Get/Update"=w1286, "Error In"=w1292, "Power Seq"=w1287, "Seq file path"=w1293) -> ("Error Out"=w1291:errorcluster, "Seq path out"=w1289:path)  [unwired: 5 in, 1 out]
                    n552 = Strip Path(path=w1289) -> (name=w1288:string)  [unwired: 1 out]
                    n553 = property on="Pattern File" class="CmbBox"(error in=w1291, "Value"=w1288) -> (error out=w1290:errorcluster)  [unwired: 1 in, 1 out]
                  }
                }
              }
              frame "Right Button" {
              }
              frame "Window Close" {
              }
            }
          }
          frame "Delete Seq" {
            w1296 = T21 [] ("Power Seq out")
            n554 = Build Path(base path=w1310, name or relative path=w1309) -> (appended path=w1307:path)
            n555 = Delete(path (use dialog)=w1307, confirm (F)=TRUE, error in=w1308) -> (deleted path=w1303:path, error out=w1306:errorcluster)  [unwired: 2 in, 1 out]
            n556 = Strip Path(path=w1303) -> (stripped path=w1302:path)  [unwired: 1 out]
            n557 = List Folder(path=w1302, error in=w1306) -> (filenames=w1305:string[], error out=w1304:errorcluster)  [unwired: 2 in, 2 out]
            n558 = property on="Pattern File" class="CmbBox"(error in=w1304, "Strings[]"=w1305, "Val(Sgnl)"="") -> (error out=w1313:errorcluster)  [unwired: 1 in, 1 out]
            n559 = property on="Power Seq" class="Arr (strict)"(error in=w1313, "Value"=w1296) -> (error out=w1300:errorcluster)  [unwired: 1 in, 1 out]
            n560 = Bundle By Name(cluster=w1298, "TTV Test.Power Seq"=w1296) -> (w1297:T24)
            n561 = property on="Test Graph" class="WFChart (strict)"(error in=w1300, "Value"=dbl[] [] ("Power Pattern Graph")) -> (error out=w1299:errorcluster)  [unwired: 1 in, 1 out]
          }
          frame "Clear Seq" {
            w1314 = T21 [] ("Power Seq out")
            w1322 = T36."Disabled and Grayed Out" ("Disabled")
            n562 = property on="Power Seq" class="Arr (strict)"(error in=w1320, "Value"=w1314) -> (error out=w1323:errorcluster)  [unwired: 1 in, 1 out]
            n563 = property on="Pattern File" class="CmbBox"(error in=w1323, "Value"="") -> (error out=w1325:errorcluster)  [unwired: 1 in, 1 out]
            n564 = control-ref of="Save Seq"() -> (w1324:refnum<vi>)
            n565 = property class="Bool"(reference=w1324, error in=w1325, "DisabledEnum"=w1322) -> (error out=w1326:errorcluster)  [unwired: 1 out]
            n566 = control-ref of="Delete Seq"() -> (w1327:refnum<vi>)
            n567 = property class="Bool"(reference=w1327, error in=w1326, "DisabledEnum"=w1322) -> (error out=w1319:errorcluster)  [unwired: 1 out]
            n568 = Bundle By Name(cluster=w1316, "TTV Test.Power Seq"=w1314) -> (w1315:T24)
            n569 = property on="Test Graph" class="WFChart (strict)"(error in=w1319, "Value"=dbl[] [] ("Power Pattern Graph")) -> (error out=w1318:errorcluster)  [unwired: 1 in, 1 out]
          }
        }
      }
      frame "APP:Power Sequence(RT)" {
        n570 = Index Array(array=w1338) -> (element=w1337:string)  [unwired: 1 in]
        n571 = Unbundle By Name(w1334) -> ("URI Directory"=w1333:string)
        n572 = property on="Pattern File" class="CmbBox"(error in=w1329) -> (error out=w1330:errorcluster, "Value"=w1331:string)  [unwired: 1 in, 1 out]
        n573 = local read "Iteration No"() -> (w1328:i32)
        n574 = call <vilib>:"Application Directory.vi"() -> ("Application Directory"=w1332:path)
        n575 = case shown="\"Pattern File\", Default" w1337 {
          tunnel: w1330 -> [w1356 w1386 w1393 w1399 w1463 w1492]
          tunnel: w1336 -> [w1355 w1385 _ _ _ _]
          tunnel: [w1340 w1384 w1392 w1405 w1468 w1490] -> w1335
          tunnel: w1333 -> [w1345 _ _ w1401 w1471 _]
          tunnel: w1332 -> [w1343 _ _ w1402 w1469 _]
          tunnel: w1331 -> [_ _ _ w1400 w1470 _]
          tunnel: w1328 -> [_ w1375 _ _ _ _]
          frame "Pattern File", Default {
            n576 = Variant To Data(error in=w1356, type="", Variant=w1355) -> (data=w1351:string, error out=w1352:errorcluster)
            n577 = Empty String/Path?(string/path=w1351) -> (empty?=w1353:bool)
            n578 = Concatenate Strings(w1345, w1351) -> (w1344:string)
            n579 = Build Path(base path=w1343, name or relative path=w1351) -> (appended path=w1342:path)
            n580 = case shown="False" w1353 {
              tunnel: w1352 -> [w1362 w1367]
              tunnel: [w1364 w1367] -> w1347
              tunnel: [w1358 T21 [] ("Power Seq out")] -> w1341
              tunnel: [T36."Enabled" ("Disabled") T36."Disabled and Grayed Out" ("Disabled")] -> w1346
              tunnel: w1344 -> [w1359 _]
              tunnel: w1342 -> [w1357 _]
              frame False {
                n581 = call "WebDAV FGV.vi"("WebDAV States"=WebDAV_states."Upload", "error in (no error)"=w1362, "local file path"=w1357, "relative uri"=w1359) -> ("error out"=w1361:errorcluster)  [unwired: 5 in, 2 out]
                n582 = call "Config Power Sequence.vi"("Get/Update"=enum16{"Get Seq", "Update Seq"}."Get Seq", "Error In"=w1361, "Seq file path"=w1357) -> ("Error Out"=w1364:errorcluster, "Power Seq out"=w1358:T21)  [unwired: 6 in, 1 out]
              }
              frame True {
              }
            }
            n583 = property on="Power Seq" class="Arr (strict)"(error in=w1347, "Val(Sgnl)"=w1341) -> (error out=w1339:errorcluster)  [unwired: 1 in, 1 out]
            n584 = control-ref of="Save Seq"() -> (w1348:refnum<vi>)
            n585 = property class="Bool"(reference=w1348, error in=w1339, "DisabledEnum"=w1346) -> (error out=w1350:errorcluster)  [unwired: 1 out]
            n586 = control-ref of="Delete Seq"() -> (w1349:refnum<vi>)
            n587 = property class="Bool"(reference=w1349, error in=w1350, "DisabledEnum"=w1346) -> (error out=w1340:errorcluster)  [unwired: 1 out]
          }
          frame "Power Seq" {
            n588 = Less Than 0?(x=w1375) -> (x < 0?=w1374:bool)
            n589 = case shown="True" w1374 {
              tunnel: ["" "Infinite Cycle" ("Command")] -> w1370
              tunnel: w1375 -> [w1387 _]
              tunnel: [w1387 1 ("Plot.Plot Interpolation")] -> w1376
              frame False {
              }
              frame True {
              }
            }
            n590 = Variant To Data(error in=w1386, type=T21 [] ("Power Seq out"), Variant=w1385) -> (data=w1380:T21, error out=w1381:errorcluster)
            n591 = call "Set Seqence.vi"("Error In"=w1381, "Iteration"=w1376, "Power Seq"=w1380) -> ("Error Out"=w1373:errorcluster, "Waveform Graph"=w1379:u32[])  [unwired: 7 in]
            n592 = To Double Precision Float(number=w1379) -> (double precision float=w1369:dbl[])
            n593 = property on="Test Graph" class="WFChart (strict)"(error in=w1373, "Value"=w1369, "Plot.Plot Interpolation"=u8 3) -> (error out=w1372:errorcluster)  [unwired: 1 in, 1 out]
            n594 = property on="Infinite Test" class="Str"(error in=w1372, "Value"=w1370) -> (error out=w1371:errorcluster)  [unwired: 1 in, 1 out]
            n595 = control-ref of="Save Seq"() -> (w1383:refnum<vi>)
            n596 = property class="Bool"(reference=w1383, error in=w1371, "DisabledEnum"=T36."Enabled" ("Disabled")) -> (error out=w1384:errorcluster)  [unwired: 1 out]
          }
          frame "Refresh Seq" {
            n597 = call "WebDAV FGV.vi"("WebDAV States"=WebDAV_states."Refresh Dir", "error in (no error)"=w1393) -> ("error out"=w1396:errorcluster, "file list"=w1391:T49[])  [unwired: 7 in, 1 out]
            n598 = for {
              tunnel: w1391 -> [w1398] mode=indexing
              tunnel: [w1397] -> w1395 mode=indexing
              n599 = Unbundle By Name(w1398) -> ("display name"=w1397:string)
            }
            n600 = property on="Pattern File" class="CmbBox"(error in=w1396, "Strings[]"=w1395) -> (error out=w1392:errorcluster)  [unwired: 1 in, 1 out]
          }
          frame "Save Seq" {
            n601 = Format Into String(format string="Overwrite it to %s", w1400) -> (resulting string=w1409:string)  [unwired: 2 in, 1 out]
            n602 = call <vilib>:"Three Button Dialog.vi"("Window Title (\"\")"="Save file (.ini)" ("Window Title (\"\")"), "Center Button Text (\"No\")"="Save as" ("Center Button Text (\"No\")"), "message"=w1409) -> ("Which Button?"=w1403:T52)  [unwired: 8 in]
            n603 = case shown="\"Center Button\"" w1403 {
              tunnel: w1399 -> [w1416 w1447 w1461 w1462]
              tunnel: w1401 -> [w1421 w1442 _ _]
              tunnel: "Enter the filename(.ini)" ("Message title") -> [_ w1445 _ _]
              tunnel: w1402 -> [w1419 w1435 _ _]
              tunnel: [w1418 w1434 w1461 w1462] -> w1405
              tunnel: w1400 -> [w1414 _ _ _]
              frame "Left Button", Default {
                n604 = Concatenate Strings(w1421, w1414) -> (w1410:string)
                n605 = Build Path(base path=w1419, name or relative path=w1414) -> (appended path=w1413:path)
                n606 = Empty String/Path?(string/path=w1414) -> (empty?=w1417:bool)
                n607 = case shown="False" w1417 {
                  tunnel: w1416 -> [w1427 w1433]
                  tunnel: [w1429 w1433] -> w1415
                  tunnel: w1413 -> [w1431 w1432]
                  tunnel: [w1430 w1432] -> w1412
                  tunnel: w1410 -> [w1425 _]
                  frame False {
                    n608 = call "WebDAV FGV.vi"("WebDAV States"=WebDAV_states."Delete", "error in (no error)"=w1427, "relative uri"=w1425) -> ("error out"=w1426:errorcluster)  [unwired: 6 in, 2 out]
                    n609 = Delete(path (use dialog)=w1431, error in=w1426) -> (deleted path=w1430:path, error out=w1429:errorcluster)  [unwired: 3 in, 1 out]
                  }
                  frame True {
                  }
                }
                n610 = property on="Power Seq" class="Arr (strict)"(error in=w1415) -> (error out=w1422:errorcluster, "Value"=w1423:T53)  [unwired: 1 in, 1 out]
                n611 = call "Config Power Sequence.vi"("Get/Update"=enum16{"Get Seq", "Update Seq"}."Update Seq", "Error In"=w1422, "Power Seq"=w1423, "Seq file path"=w1412) -> ("Error Out"=w1411:errorcluster)  [unwired: 5 in, 2 out]
                n612 = call "WebDAV FGV.vi"("WebDAV States"=WebDAV_states."Download", "error in (no error)"=w1411, "local file path"=w1412, "relative uri"=w1410) -> ("error out"=w1418:errorcluster)  [unwired: 5 in, 2 out]
              }
              frame "Center Button" {
                w1439 = ".ini" ("regular expression")
                n613 = call "User Input Dialog.vi"("error in (no error)"=w1447, "Message title"=w1445) -> ("error out"=w1446:errorcluster, "OK?"=w1438:bool, "Message out"=w1441:string)  [unwired: 6 in]
                n614 = Match Pattern(string=w1441, regular expression=w1439) -> (match substring=w1440:string)  [unwired: 1 in, 3 out]
                n615 = Equal?(x=w1440, y=w1439) -> (x = y?=w1437:bool)
                n616 = Concatenate Strings(w1442, w1441) -> (w1443:string)
                n617 = Build Path(base path=w1435, name or relative path=w1441) -> (appended path=w1444:path)
                n618 = And(x=w1438, y=w1437) -> (x .and. y?=w1436:bool)
                n619 = case shown="True" w1436 {
                  tunnel: [w1448 w1455] -> w1434
                  tunnel: w1446 -> [w1448 w1454]
                  tunnel: w1444 -> [_ w1453]
                  tunnel: w1443 -> [_ w1452]
                  frame False {
                  }
                  frame True {
                    n620 = property on="Power Seq" class="Arr (strict)"(error in=w1454) -> (error out=w1458:errorcluster, "Value"=w1459:T53)  [unwired: 1 in, 1 out]
                    n621 = call "Config Power Sequence.vi"("Get/Update"=enum16{"Get Seq", "Update Seq"}."Update Seq", "Error In"=w1458, "Power Seq"=w1459, "Seq file path"=w1453) -> ("Error Out"=w1456:errorcluster, "Seq path out"=w1449:path)  [unwired: 5 in, 1 out]
                    n622 = Strip Path(path=w1449) -> (name=w1451:string)  [unwired: 1 out]
                    n623 = call "WebDAV FGV.vi"("WebDAV States"=WebDAV_states."Download", "error in (no error)"=w1456, "relative uri"=w1452) -> ("error out"=w1450:errorcluster)  [unwired: 6 in, 2 out]
                    n624 = property on="Pattern File" class="CmbBox"(error in=w1450, "Value"=w1451) -> (error out=w1455:errorcluster)  [unwired: 1 in, 1 out]
                  }
                }
              }
              frame "Right Button" {
              }
              frame "Window Close" {
              }
            }
          }
          frame "Delete Seq" {
            n625 = Build Path(base path=w1469, name or relative path=w1470) -> (appended path=w1466:path)
            n626 = Concatenate Strings(w1471, w1470) -> (w1472:string)
            n627 = Delete(path (use dialog)=w1466, confirm (F)=TRUE, error in=w1463) -> (cancelled=w1464:bool, error out=w1467:errorcluster)  [unwired: 2 in, 1 out]
            n628 = case shown="False" w1464 {
              tunnel: [w1476 w1487] -> w1468
              tunnel: w1467 -> [w1478 w1487]
              tunnel: w1472 -> [w1479 _]
              frame False {
                n629 = call "WebDAV FGV.vi"("WebDAV States"=WebDAV_states."Delete", "error in (no error)"=w1478, "relative uri"=w1479) -> ("error out"=w1482:errorcluster, "file list"=w1473:T49[])  [unwired: 6 in, 1 out]
                n630 = for {
                  tunnel: w1473 -> [w1486] mode=indexing
                  tunnel: [w1485] -> w1480 mode=indexing
                  n631 = Unbundle By Name(w1486) -> ("display name"=w1485:string)
                }
                n632 = property on="Pattern File" class="CmbBox"(error in=w1482, "Strings[]"=w1480, "Val(Sgnl)"="") -> (error out=w1481:errorcluster)  [unwired: 1 in, 1 out]
                n633 = property on="Power Seq" class="Arr (strict)"(error in=w1481, "Value"=T21 [] ("Power Seq out")) -> (error out=w1477:errorcluster)  [unwired: 1 in, 1 out]
                n634 = property on="Test Graph" class="WFChart (strict)"(error in=w1477, "Value"=dbl[] [] ("Power Pattern Graph")) -> (error out=w1476:errorcluster)  [unwired: 1 in, 1 out]
              }
              frame True {
              }
            }
          }
          frame "Clear Seq" {
            w1494 = T36."Disabled and Grayed Out" ("Disabled")
            n635 = property on="Power Seq" class="Arr (strict)"(error in=w1492, "Value"=T21 [] ("Power Seq out")) -> (error out=w1495:errorcluster)  [unwired: 1 in, 1 out]
            n636 = property on="Pattern File" class="CmbBox"(error in=w1495, "Value"="") -> (error out=w1497:errorcluster)  [unwired: 1 in, 1 out]
            n637 = control-ref of="Save Seq"() -> (w1496:refnum<vi>)
            n638 = property class="Bool"(reference=w1496, error in=w1497, "DisabledEnum"=w1494) -> (error out=w1498:errorcluster)  [unwired: 1 out]
            n639 = control-ref of="Delete Seq"() -> (w1499:refnum<vi>)
            n640 = property class="Bool"(reference=w1499, error in=w1498, "DisabledEnum"=w1494) -> (error out=w1491:errorcluster)  [unwired: 1 out]
            n641 = property on="Test Graph" class="WFChart (strict)"(error in=w1491, "Value"=dbl[] [] ("Power Pattern Graph")) -> (error out=w1490:errorcluster)  [unwired: 1 in, 1 out]
          }
        }
      }
      frame "APP:TTV Test" {
        # "Control the power on/off and voltage to Chroma AC Power Supply"
        n642 = Index Array(array=w1507) -> (element=w1506:string)  [unwired: 1 in]
        n643 = case shown="\"Reset Test\"" w1506 {
          tunnel: w1505 -> [w1524 w1562 w1654 w1682 w1694 w1804]
          tunnel: w1504 -> [w1521 _ _ _ _ _]
          tunnel: [w1514 w1580 w1662 w1673 w1700 w1802] -> w1502
          tunnel: w1501 -> [w1519 w1582 w1664 w1680 w1703 w1796]
          tunnel: [w1518 w1581 w1663 w1679 w1702 w1796] -> w1503
          tunnel: w1501 -> [_ w1578 w1651 _ w1699 _]
          tunnel: [_ w1558 Save_Log_State."Write" ("State") Save_Log_State."Write" ("State") _ _] -> w1500
          frame "Power", Default {
            w1513 = u16 19200 items=["4800"=4800, "9600"=9600, "19200"=19200, "38400"=38400, "57600"=57600] ("Baud Rate")
            # "Power on/off for Power Supply"
            n644 = Variant To Data(error in=w1524, type=FALSE ("Output"), Variant=w1521) -> (data=w1520:bool, error out=w1523:errorcluster)
            n645 = case shown="False" w1520 {
              tunnel: [w1525 w1540] -> w1514
              tunnel: w1523 -> [w1531 w1551]
              tunnel: w1513 -> [_ w1552]
              tunnel: [FALSE w1541] -> w1517
              tunnel: [T36."Enabled" ("Disabled") T36."Disabled and Grayed Out" ("Disabled")] -> w1508
              tunnel: [T36."Disabled and Grayed Out" ("Disabled") T36."Enabled" ("Disabled")] -> w1516
              frame False {
                # "Power off to disconnect PS and switch the mode to edit the power sequence"
                n646 = call "Serial FGV.vi"("Status"=enum16{"Config", "Read", "Write", "Close"}."Write", "Error In"=w1531, "Command"="OUTPUT OFF\n") -> ("Error Out"=w1534:errorcluster)  [unwired: 5 in, 3 out]
                n647 = call "Serial FGV.vi"("Status"=enum16{"Config", "Read", "Write", "Close"}."Close", "Error In"=w1534) -> ("Error Out"=w1526:errorcluster)  [unwired: 6 in, 3 out]
                n648 = property on="Test Graph" class="WFChart (strict)"(error in=w1526, "History Data"=dbl[] [], "Plot.Plot Interpolation"=u8 3) -> (error out=w1525:errorcluster)  [unwired: 1 in, 1 out]
              }
              frame True {
                # "Check out the connection to PS"
                # "Power on and check out the system error"
                n649 = To Unsigned Long Integer(number=w1552) -> (unsigned 32bit integer=w1556:u32)
                n650 = local read "Serial Port"() -> (w1537:string)
                n651 = Bundle By Name(cluster=T42 {"baud rate"=19200, "data bits"=8, "parity"=enum."None", "stop bits"=10, "flow control"=0} ("Serial Settings"), "baud rate"=w1556) -> (w1555:T42)
                n652 = Type Cast(type=refnum<visa-resource-name> refnum ("VISA resource name"), x=w1537) -> (*(type *) &x=w1554:refnum<visa-resource-name>)
                n653 = call "Serial FGV.vi"("Status"=enum16{"Config", "Read", "Write", "Close"}."Config", "Error In"=w1551, "Serial Settings"=w1555, "VISA resource name"=w1554) -> ("Error Out"=w1549:errorcluster)  [unwired: 4 in, 3 out]
                n654 = call "Serial FGV.vi"("Status"=enum16{"Config", "Read", "Write", "Close"}."Write", "Error In"=w1549, "Command"="SYSTEM:ERROR?\n") -> ("Error Out"=w1545:errorcluster)  [unwired: 5 in, 3 out]
                n655 = call "Serial FGV.vi"("delay before read (ms)"=u32 10, "Status"=enum16{"Config", "Read", "Write", "Close"}."Read", "Error In"=w1545) -> ("Error Out"=w1540:errorcluster, "Response"=w1543:string)  [unwired: 5 in, 2 out]
                n656 = Equal?(x="NO", y=w1543) -> (x = y?=w1541:bool)
              }
            }
            n657 = property on="Start Test" class="Bool"("DisabledEnum"=w1516) -> ()  [unwired: 2 in, 2 out]
            n658 = property on="Stop Test" class="Bool"("DisabledEnum"=w1516) -> ()  [unwired: 2 in, 2 out]
            n659 = property on="Reset Test" class="Bool"("DisabledEnum"=w1516) -> ()  [unwired: 2 in, 2 out]
            n660 = property on="TTV Power" class="DigNum (strict)"("Value"=nan) -> ()  [unwired: 2 in, 2 out]
            n661 = property on="Manual IP" class="Str"("DisabledEnum"=w1508) -> ()  [unwired: 2 in, 2 out]
            n662 = property on="Iteration No" class="DigNum (strict)"("DisabledEnum"=w1508) -> ()  [unwired: 2 in, 2 out]
            n663 = property on="Menu Ring" class="Ring (strict)"("DisabledEnum"=w1508) -> ()  [unwired: 2 in, 2 out]
            n664 = Bundle By Name(cluster=w1519, "TTV Test.Current Cycle"=1 ("Current Cycle"), "TTV Test.Step"=0 ("Step"), "TTV Test.PS Connection"=w1517) -> (w1518:T24)
            n665 = property on="Time" class="DigNum (strict)"("Value"=0.0 ("Time")) -> ()  [unwired: 2 in, 2 out]
            n666 = property on="Pattern File" class="CmbBox"("DisabledEnum"=w1508) -> ()  [unwired: 2 in, 2 out]
            n667 = property on="Power Seq" class="Arr (strict)"("DisabledEnum"=w1508) -> ()  [unwired: 2 in, 2 out]
            n668 = property on="Seq Controls" class="Clust"("DisabledEnum"=w1508) -> ()  [unwired: 2 in, 2 out]
            n669 = property on="Cycle" class="DigNum (strict)"("Value"=1 ("Cycle")) -> ()  [unwired: 2 in, 2 out]
          }
          frame "Start Test" {
            (unwired) FALSE ("Start Stop Test")
            # "Start 1 not 0"
            # "Check out the \nStack Light States \nfrom RT"
            # "Send command to RT to check booting"
            n670 = Unbundle By Name(w1578) -> ("TTV Test.Current Cycle"=w1560:i32, "TTV Test.Step"=w1570:i32, "TTV Test.Power Seq"=w1569:T21, "TTV Test.PS Connection"=w1566:bool)
            n671 = property on="Iteration No" class="DigNum (strict)"() -> ("Value"=w1565:i32)  [unwired: 2 in, 2 out]
            n672 = property on="Stack light states" class="Enum (strict)"() -> ("Value"=w1568:T1)  [unwired: 2 in, 2 out]
            n673 = Not Equal To 0?(x=w1565) -> (x != 0?=w1564:bool)
            n674 = Equal?(x=w1568, y=T1."Ready" ("Stack light states")) -> (x = y?=w1563:bool)
            n675 = Compound Arithmetic op=AND(w1566, w1564, w1563) -> ()  [unwired: 1 out]
            n676 = case shown="True" TRUE {
              tunnel: w1562 -> [w1604 w1611]
              tunnel: [w1600 w1629] -> w1579
              tunnel: w1569 -> [_ w1632]
              tunnel: w1570 -> [w1597 w1633]
              tunnel: [FALSE TRUE] -> w1576
              tunnel: [FALSE TRUE] -> w1575
              tunnel: [w1597 w1627] -> w1574
              tunnel: [w1595 w1626] -> w1573
              tunnel: [T36."Enabled" ("Disabled") T36."Disabled and Grayed Out" ("Disabled")] -> w1572
              tunnel: [T36."Disabled and Grayed Out" ("Disabled") T36."Enabled" ("Disabled")] -> w1571
              tunnel: [w1588 w1615] -> w1561
              tunnel: w1560 -> [w1588 w1616]
              tunnel: [Save_Log_State."Idle" ("State") Save_Log_State."Write" ("State")] -> w1558
              frame False {
                # "Try to connect to the power supply until the boot time set up"
                # "Set up Time out"
                n677 = property on="Boot Time(s)" class="DigNum (strict)"(error in=w1604) -> (error out=w1600:errorcluster, "Value"=w1603:u32)  [unwired: 1 in, 1 out]
                n678 = Increment(x=w1603) -> (x+1=w1602:u32)
                "Boot Time(s)" <- w1602
                n679 = Greater Or Equal?(x=w1602, y="Boot Time out(s)") -> (x >= y?=w1596:bool)
                n680 = Wait (ms)(milliseconds to wait=u32 1000) -> ()  [unwired: 1 out]
                n681 = Select(t="Stop Test" ("Command"), s=w1596, f="Start Test" ("Command")) -> (s? t:f=w1591:string)
                n682 = Concatenate Strings("APP:TTV Test>>" ("Command"), w1591) -> (w1595:string)
              }
              frame True {
                n683 = First Call?() -> (First Call?: T/F=w1635:bool)
                n684 = case shown="True" w1635 {
                  tunnel: [Timer_Mode."Resume" ("Timer Mode") Timer_Mode."Start Timer" ("Timer Mode")] -> w1634
                  tunnel: w1633 -> [w1639 _]
                  tunnel: w1632 -> [w1641 w1646]
                  tunnel: [w1640 w1645] -> w1631
                  tunnel: [w1639 w1644] -> w1627
                  tunnel: w1616 -> [w1638 _]
                  tunnel: [w1638 1 ("Current Cycle")] -> w1615
                  frame False {
                    n685 = Index Array(array=w1641, index=w1639) -> (element=w1640:T54)
                  }
                  frame True {
                    w1644 = 0 ("Step No")
                    n686 = Index Array(array=w1646, index=w1644) -> (element=w1645:T54)
                  }
                }
                n687 = Unbundle By Name(w1631) -> ("Name"=→"Step":string, "Head Load(W)"=w1637:u32, "Duration"=w1606:i32)
                n688 = property on="Test Graph" class="WFChart (strict)"(error in=w1611, "History Data"=dbl[] [] ("Test Graph"), "Plot.Plot Interpolation"=u8 2) -> (error out=w1610:errorcluster)  [unwired: 1 in, 1 out]
                n689 = call "Timing FGV.vi"("Time Target (s)"=w1606, "Timer Mode"=w1634, "Error In"=w1610) -> ("Error Out"=w1630:errorcluster)  [unwired: 6 in, 2 out]
                n690 = Number To Fractional String(number=w1637, precision (6)=3) -> (F-format string=w1623:string)  [unwired: 1 in, 1 out]
                n691 = Concatenate Strings("VOLTAGE:AC " ("Command"), w1623, "\n" ("Command"), "OUTPUT ON\n" ("Command")) -> (w1608:string)
                n692 = call "Serial FGV.vi"("Status"=enum16{"Config", "Read", "Write", "Close"}."Write", "Error In"=w1630, "Command"=w1608) -> ("Error Out"=w1629:errorcluster)  [unwired: 5 in, 3 out]
                n693 = Concatenate Strings("NS:Write>>" ("Command"), "TTV Test" ("Command")) -> (w1626:string)
              }
            }
            n694 = property on="Reset Test" class="Bool"("DisabledEnum"=w1572) -> ()  [unwired: 2 in, 2 out]
            n695 = property on="Start Test" class="Bool"("DisabledEnum"=w1572) -> ()  [unwired: 2 in, 2 out]
            n696 = property on="Stop Test" class="Bool"("DisabledEnum"=w1571) -> ()  [unwired: 2 in, 2 out]
            n697 = Bundle By Name(cluster=w1582, "TTV Test.Current Cycle"=w1561, "TTV Test.Step"=w1574, "TTV Test.OutputState"=w1575) -> (w1581:T24)
            n698 = To Variant(anything=w1576) -> (Variant=w1577:variant)
            n699 = disable-structure shown="Disabled" {
              disable-tunnel: [w1586 _] -> w1580
              disable-tunnel: w1579 -> [w1585 _]
              disable-tunnel: w1577 -> [w1584 _]
              disable-tunnel: w1573 -> [w1583 _]
              frame Disabled {
                n700 = call "Messaging EnQ Single.vi"("Command"=w1583, "Data"=w1584, "error in (no error)"=w1585) -> ("error out"=w1586:errorcluster)  [unwired: 8 in]
              }
              frame Enabled {
              }
            }
          }
          frame "Reset Test" {
            n701 = property on="Cycle" class="DigNum (strict)"(error in=w1654, "Value"=1 ("Cycle")) -> (error out=w1653:errorcluster)  [unwired: 1 in, 1 out]
            n702 = property on="TTV Power" class="DigNum (strict)"(error in=w1653, "Value"=nan) -> (error out=w1656:errorcluster)  [unwired: 1 in, 1 out]
            n703 = property on="Step" class="Str"(error in=w1656, "Value"="") -> (error out=w1657:errorcluster)  [unwired: 1 in, 1 out]
            n704 = property on="Time" class="DigNum (strict)"(error in=w1657, "Value"=0.0 ("Time")) -> (error out=w1669:errorcluster)  [unwired: 1 in, 1 out]
            n705 = Unbundle By Name(w1651) -> ("TTV Test.Power Seq"=w1650:T21)
            n706 = property on="Test Graph" class="WFChart (strict)"(error in=w1669, "History Data"=dbl[] []) -> (error out=w1652:errorcluster)  [unwired: 1 in, 1 out]
            n707 = Index Array(array=w1650, index=0) -> (element=w1670:T54)
            n708 = Unbundle By Name(w1670) -> ("Duration"=w1648:i32)
            n709 = call "Timing FGV.vi"("Time Target (s)"=w1648, "Timer Mode"=Timer_Mode."Start Timer", "Error In"=w1652) -> ("Error Out"=w1662:errorcluster)  [unwired: 6 in, 2 out]
            n710 = Bundle By Name(cluster=w1664, "TTV Test.Current Cycle"=1 ("Current Cycle"), "TTV Test.Step"=0 ("Step")) -> (w1663:T24)
          }
          frame "Stop Test" {
            # "Stop testing and pause with current step and iteration"
            n711 = call "Serial FGV.vi"("Status"=enum16{"Config", "Read", "Write", "Close"}."Write", "Error In"=w1682, "Command"="OUTPUT OFF\n") -> ("Error Out"=w1687:errorcluster)  [unwired: 5 in, 3 out]
            n712 = To Variant(anything=FALSE ("Start Stop Test")) -> (Variant=w1675:variant)
            n713 = call "Messaging EnQ Single.vi"("Command"="NS:Write>>TTV Test", "Data"=w1675, "error in (no error)"=w1687) -> ("error out"=w1674:errorcluster)  [unwired: 8 in]
            n714 = call "Timing FGV.vi"("Timer Mode"=Timer_Mode."Pause", "Error In"=w1674) -> ("Error Out"=w1673:errorcluster)  [unwired: 7 in, 2 out]
            n715 = Bundle By Name(cluster=w1680, "TTV Test.OutputState"=FALSE ("Start Stop Test")) -> (w1679:T24)
            n716 = property on="Reset Test" class="Bool"("DisabledEnum"=T36."Enabled" ("Disabled")) -> ()  [unwired: 2 in, 2 out]
            n717 = property on="Stop Test" class="Bool"("DisabledEnum"=T36."Disabled and Grayed Out" ("Disabled")) -> ()  [unwired: 2 in, 2 out]
            n718 = property on="Start Test" class="Bool"("DisabledEnum"=T36."Enabled" ("Disabled")) -> ()  [unwired: 2 in, 2 out]
          }
          frame "Read TTV power" {
            # "Create Message at IDLE case"
            n719 = Unbundle By Name(w1699) -> ("TTV Test.Step"=w1690:i32, "TTV Test.Power Seq"=w1692:T21, "TTV Test.Current Cycle"=w1689:i32)
            n720 = call "Timing FGV.vi"("Timer Mode"=Timer_Mode."Read Time", "Error In"=w1694) -> ("Error Out"=w1697:errorcluster, "Elapsed Time (s.ms)"=w1693:dbl, "Has Time Elapsed"=w1698:bool)  [unwired: 7 in]
            n721 = case shown="True" w1698 {
              tunnel: [w1708 w1740] -> w1691
              tunnel: w1697 -> [w1712 w1739]
              tunnel: [w1722 w1739] -> w1696
              tunnel: [TRUE w1744] -> w1695
              tunnel: w1693 -> [w1710 _]
              tunnel: w1692 -> [_ w1743]
              tunnel: w1690 -> [w1708 w1741]
              tunnel: w1689 -> [w1709 w1738]
              tunnel: [w1709 w1745] -> w1688
              frame False {
                # "timing equation : \n\nidle    delay   read  \n100 +  250 + 640+10 = 1000 ( one second)"
                # "Then, make timing a second"
                # "Make sure the connection"
                # "Time delay = 250 ms"
                # "Read power from the power supply"
                n722 = disable-structure shown="Enabled" {
                  disable-tunnel: [w1728 _] -> w1706
                  frame Enabled {
                    # "Create signal simulated"
                    n723 = for {
                      N: 1 -> [_]
                      tunnel: [w1731] -> w1728
                      n724 = Random Number (0-1)() -> (number: 0 to 1=w1733:dbl)
                      n725 = Multiply(x=w1733, y=100.0) -> (x*y=w1731:dbl)
                      n726 = Wait (ms)(milliseconds to wait=u32 1) -> ()  [unwired: 1 out]
                    }
                  }
                  frame Disabled {
                  }
                }
                n727 = call "Serial FGV.vi"("Status"=enum16{"Config", "Read", "Write", "Close"}."Write", "Error In"=w1712, "Command"="FETCH:POWER:AC:APPARENT?\n") -> ("Error Out"=w1719:errorcluster)  [unwired: 5 in, 3 out]
                n728 = call "Serial FGV.vi"("delay before read (ms)"=u32 640, "Status"=enum16{"Config", "Read", "Write", "Close"}."Read", "Error In"=w1719) -> ("Error Out"=w1711:errorcluster, "return count"=w1718:u32, "Response"=w1717:string)  [unwired: 5 in, 1 out]
                n729 = Fract/Exp String To Number(string=w1717) -> ()  [unwired: 3 in, 2 out]
                n730 = To Unsigned Byte Integer(number=w1718) -> (unsigned 8bit integer=w1705:u8)
                n731 = Build Array(w1706) -> (w1704:dbl[])
                n732 = property on="TTV Power" class="DigNum (strict)"("Value"=w1706, "Precision"=w1705) -> ()  [unwired: 2 in, 2 out]
                n733 = property on="Test Graph" class="WFChart (strict)"("Value"=w1704) -> ()  [unwired: 2 in, 2 out]
                n734 = call "Serial FGV.vi"("Status"=enum16{"Config", "Read", "Write", "Close"}."Write", "Error In"=w1711, "Command"="OUTPUT?\n") -> ("Error Out"=w1727:errorcluster)  [unwired: 5 in, 3 out]
                n735 = call "Serial FGV.vi"("delay before read (ms)"=u32 10, "Status"=enum16{"Config", "Read", "Write", "Close"}."Read", "Error In"=w1727) -> ("Error Out"=w1722:errorcluster, "Response"=w1726:string)  [unwired: 5 in, 2 out]
                n736 = Equal?(x="ON" ("Command"), y=w1726) -> ()  [unwired: 1 out]
                "Time" <- w1710
              }
              frame True {
                # "When done for a step, check out if the current step reach out the end of step and iteration"
                n737 = property on="Iteration No" class="DigNum (strict)"() -> ("Value"=w1736:i32)  [unwired: 2 in, 2 out]
                n738 = Array Size(array=w1743) -> (size(s)=w1747:i32)
                n739 = Equal?(x=w1741, y=w1747) -> (x = y?=w1746:bool)
                n740 = Greater Or Equal?(x=w1738, y=w1736) -> (x >= y?=w1737:bool)
                n741 = case shown="True" w1746 {
                  tunnel: w1737 -> [_ w1767]
                  tunnel: w1738 -> [w1752 w1766]
                  tunnel: [w1752 w1765] -> w1745
                  tunnel: [TRUE w1764] -> w1744
                  tunnel: w1743 -> [w1755 w1763]
                  tunnel: [w1753 w1762] -> w1742
                  tunnel: [w1751 w1761] -> w1735
                  tunnel: w1741 -> [w1750 w1759]
                  tunnel: [w1749 w1760] -> w1740
                  frame False {
                    n742 = Increment(x=w1750) -> (x+1=w1749:i32)
                    n743 = Index Array(array=w1755, index=w1749) -> (element=w1754:T54)
                    n744 = Unbundle By Name(w1754) -> ("Name"=w1751:string, "Duration"=w1753:i32)
                  }
                  frame True {
                    n745 = Index Array(array=w1763, index=0) -> (element=w1757:T54)
                    n746 = case shown="True" w1767 {
                      tunnel: w1766 -> [w1774 w1779]
                      tunnel: [w1773 w1779] -> w1765
                      tunnel: [TRUE FALSE] -> w1764
                      tunnel: [w1772 0 ("Duration")] -> w1762
                      tunnel: [w1770 w1778] -> w1761
                      tunnel: [0 w1776] -> w1760
                      tunnel: w1759 -> [_ w1776]
                      tunnel: w1757 -> [w1768 w1775]
                      frame False {
                        n747 = Increment(x=w1774) -> (x+1=w1773:i32)
                        n748 = Unbundle By Name(w1768) -> ("Name"=w1770:string, "Duration"=w1772:i32)
                      }
                      frame True {
                        n749 = Unbundle By Name(w1775) -> ("Name"=w1778:string)
                      }
                    }
                  }
                }
                n750 = property on="Step" class="Str"("Value"=w1735) -> ()  [unwired: 2 in, 2 out]
                n751 = To Double Precision Float(number=w1742) -> (double precision float=w1734:dbl)
                n752 = call "Timing FGV.vi"("Time Target (s)"=w1734, "Timer Mode"=Timer_Mode."Start Timer") -> ()  [unwired: 7 in, 3 out]
              }
            }
            "Cycle" <- w1688
            n753 = case shown="False" w1695 {
              tunnel: w1696 -> [w1782 w1793]
              tunnel: [w1786 w1793] -> w1700
              frame False {
                n754 = disable-structure shown="Enabled" {
                  disable-tunnel: w1782 -> [w1791 w1792]
                  disable-tunnel: [w1790 w1792] -> w1781
                  frame Enabled {
                    n755 = call <vilib>:"Clear Errors.vi"("error in (no error)"=w1791) -> ("error out"=w1790:errorcluster)  [unwired: 5 in, 1 out]
                  }
                  frame Disabled {
                  }
                }
                n756 = Concatenate Strings("APP:TTV Test>>" ("Command"), "Stop Test" ("Command")) -> (w1783:string)
                n757 = disable-structure shown="Disabled" {
                  disable-tunnel: [w1789 _] -> w1786
                  disable-tunnel: w1783 -> [w1788 _]
                  disable-tunnel: w1781 -> [w1787 _]
                  frame Disabled {
                    n758 = call "Messaging EnQ Single.vi"("Command"=w1788, "error in (no error)"=w1787) -> ("error out"=w1789:errorcluster)  [unwired: 9 in]
                  }
                  frame Enabled {
                  }
                }
              }
              frame True {
              }
            }
            n759 = Bundle By Name(cluster=w1703, "TTV Test.Step"=w1691, "TTV Test.Current Cycle"=w1688) -> (w1702:T24)
          }
          frame "Custom Command" {
            # "Check out the communication of RS232 for debugging"
            n760 = Concatenate Strings("Command", "\n" ("Command")) -> (w1799:string)
            n761 = call "Serial FGV.vi"("Status"=enum16{"Config", "Read", "Write", "Close"}."Write", "Error In"=w1804, "Command"=w1799) -> ("Error Out"=w1803:errorcluster)  [unwired: 5 in, 3 out]
            n762 = call "Serial FGV.vi"("delay before read (ms)"=u32 10, "Status"=enum16{"Config", "Read", "Write", "Close"}."Read", "Error In"=w1803) -> ("Error Out"=w1802:errorcluster, "Response"=→"Response":string)  [unwired: 5 in, 2 out]
          }
        }
      }
      frame "APP:Temp Profile" {
        n763 = Index Array(array=w1812) -> (element=w1811:string)  [unwired: 1 in]
        n764 = case shown="\"Stop Profile\"" w1811 {
          tunnel: w1816 -> [w1839 w1909 w1933]
          tunnel: w1815 -> [w1840 _ _]
          tunnel: [w1835 w1903 w1938] -> w1810
          tunnel: [w1837 FALSE ("Start Profile Test") w1939] -> w1813
          tunnel: w1808 -> [w1820 _ w1919]
          tunnel: [w1829 0 ("Profile.Current Cycle") w1922] -> w1809
          tunnel: w1808 -> [w1828 w1898 w1928]
          tunnel: [w1827 w1898 w1928] -> w1807
          tunnel: [w1817 Save_Log_State."Write" ("State") _] -> w1806
          tunnel: [w1818 "Stop Profile Test" ("Descripition") _] -> w1805
          frame "Start Profile", Default {
            n765 = Variant To Data(error in=w1839, type=T20 {"Start Temp"=0.0, "End Temp"=0.0, "Duration"=0.0, "dt"=0.0, "Iteration"=0} ("Profile Info"), Variant=w1840) -> (data=w1826:T20, error out=w1838:errorcluster)
            n766 = Unbundle By Name(w1820) -> ("Network Connection"=w1819:bool)
            n767 = property on="Stack light states" class="Enum (strict)"() -> ("Value"=w1822:T1)  [unwired: 2 in, 2 out]
            n768 = Unbundle By Name(w1826) -> ("Iteration"=w1825:i32)
            n769 = Equal?(x=w1822, y=T1."Ready" ("Stack light states")) -> (x = y?=w1824:bool)
            n770 = Not Equal To 0?(x=w1825) -> (x != 0?=w1823:bool)
            n771 = Compound Arithmetic op=AND(w1819, w1824, w1823) -> ()  [unwired: 1 out]
            n772 = case shown="True" TRUE {
              tunnel: [FALSE ("Start Stop Test") TRUE ("Start Stop Test")] -> w1837
              tunnel: w1838 -> [w1856 w1878]
              tunnel: [w1856 w1872] -> w1836
              tunnel: [T36."Enabled" ("Disabled") T36."Disabled and Grayed Out" ("Disabled")] -> w1833
              tunnel: [T36."Enabled" ("Disabled") T36."Disabled and Grayed Out" ("Disabled")] -> w1831
              tunnel: [T36."Disabled and Grayed Out" ("Disabled") T36."Enabled" ("Disabled")] -> w1832
              tunnel: w1826 -> [_ w1858]
              tunnel: [w1850 w1863] -> w1818
              tunnel: [FALSE ("Start Stop Test") TRUE ("Start Stop Test")] -> w1834
              tunnel: [0 ("Profile.Current Cycle") 1 ("Profile.Current Cycle")] -> w1829
              tunnel: w1828 -> [w1846 w1860]
              tunnel: [w1846 w1859] -> w1827
              tunnel: [_ Save_Log_State."Write" ("State")] -> w1817
              frame False {
                n773 = Concatenate Strings("NS:Write>>" ("Command"), "Profile Test" ("Command")) -> (w1850:string)
              }
              frame True {
                n774 = Unbundle By Name(w1858) -> ("dt"=w1870:dbl, "Start Temp"=w1871:dbl)
                n775 = Concatenate Strings("NS:Write>>" ("Command"), "M1 Set Temp" ("Command")) -> (w1867:string)
                n776 = First Call?() -> (First Call?: T/F=w1879:bool)
                n777 = case shown="True" w1879 {
                  tunnel: [T44."Resume" ("Timer Mode") T44."Start Timer" ("Timer Mode")] -> w1877
                  tunnel: w1878 -> [w1882 w1887]
                  tunnel: [w1882 w1884] -> w1876
                  tunnel: w1871 -> [_ w1890]
                  tunnel: w1870 -> [_ w1888]
                  tunnel: w1867 -> [_ w1889]
                  tunnel: [nan w1888] -> w1866
                  frame False {
                  }
                  frame True {
                    n778 = disable-structure shown="Disabled" {
                      disable-tunnel: w1890 -> [w1895 _]
                      disable-tunnel: w1889 -> [w1894 _]
                      disable-tunnel: w1887 -> [w1893 _]
                      disable-tunnel: [w1892 _] -> w1885
                      frame Disabled {
                        n779 = call "Messaging EnQ Single.vi"("Command"=w1894, "Data"=w1895, "error in (no error)"=w1893) -> ("error out"=w1892:errorcluster)  [unwired: 8 in]
                      }
                      frame Enabled {
                      }
                    }
                    n780 = property on="Profile Chart" class="WFChart (strict)"(error in=w1885, "History Data"=waveform(dbl)[][] []) -> (error out=w1884:errorcluster)  [unwired: 1 in, 1 out]
                  }
                }
                n781 = Bundle By Name(cluster=w1860, "Profile Info"=w1858) -> (w1859:T24)
                n782 = call "Profile Timing FGV.vi"("Timer Mode"=w1877, "Error In"=w1876, "Time Target (s)"=w1866) -> ("Error Out"=w1872:errorcluster)  [unwired: 6 in, 2 out]
                n783 = Concatenate Strings("NS:Write>>" ("Command"), "Profile Test" ("Command")) -> (w1863:string)
              }
            }
            n784 = disable-structure shown="Disabled" {
              disable-tunnel: w1836 -> [w1845 _]
              disable-tunnel: [w1844 _] -> w1835
              disable-tunnel: w1834 -> [w1843 _]
              disable-tunnel: w1818 -> [w1842 _]
              frame Disabled {
                n785 = call "Messaging EnQ Single.vi"("Command"=w1842, "Data"=w1843, "error in (no error)"=w1845) -> ("error out"=w1844:errorcluster)  [unwired: 8 in]
              }
              frame Enabled {
              }
            }
            n786 = property on="Stop Profile" class="Bool"("DisabledEnum"=w1832) -> ()  [unwired: 2 in, 2 out]
            n787 = property on="Reset Profile" class="Bool"("DisabledEnum"=w1831) -> ()  [unwired: 2 in, 2 out]
            n788 = property on="Start Profile" class="Bool"("DisabledEnum"=w1833) -> ()  [unwired: 2 in, 2 out]
          }
          frame "Stop Profile" {
            n789 = call "Profile Timing FGV.vi"("Timer Mode"=Timer_Mode."Pause", "Error In"=w1909) -> ("Error Out"=w1904:errorcluster)  [unwired: 7 in, 2 out]
            n790 = Concatenate Strings("NS:Write>>" ("Command"), "Profile Test" ("Command")) -> (w1906:string)
            n791 = disable-structure shown="Disabled" {
              disable-tunnel: w1906 -> [w1915 _]
              disable-tunnel: FALSE ("Start Stop Test") -> [w1914 _]
              disable-tunnel: w1904 -> [w1913 _]
              disable-tunnel: [w1912 _] -> w1903
              frame Disabled {
                n792 = call "Messaging EnQ Single.vi"("Command"=w1915, "Data"=w1914, "error in (no error)"=w1913) -> ("error out"=w1912:errorcluster)  [unwired: 8 in]
              }
              frame Enabled {
              }
            }
            n793 = property on="Stop Profile" class="Bool"("DisabledEnum"=T36."Disabled and Grayed Out" ("Disabled")) -> ()  [unwired: 2 in, 2 out]
            n794 = property on="Reset Profile" class="Bool"("DisabledEnum"=T36."Enabled" ("Disabled")) -> ()  [unwired: 2 in, 2 out]
            n795 = property on="Start Profile" class="Bool"("DisabledEnum"=T36."Enabled" ("Disabled")) -> ()  [unwired: 2 in, 2 out]
          }
          frame "Read Temp" {
            # "Create Message at IDLE case"
            n796 = Unbundle By Name(w1919) -> ("Dataset.M1 Status.Case Temp"=w1935:dbl, "Dataset.M1 Status.Evap Temp"=w1936:dbl, "Dataset.M1 Status.Feedback"=w1937:u8)
            n797 = Unbundle By Name(w1919) -> ("Dataset.M1 Status.Set Temp"=w1931:dbl)
            n798 = Unbundle By Name(w1919) -> ("Profile.Current Cycle"=w1927:i32)
            n799 = Unbundle By Name(w1919) -> ("Dataset.Config Data.SS Tolerance"=w1918:dbl)
            n800 = Unbundle By Name(w1919) -> ("Profile Info"=w1924:T20)
            n801 = case shown="1" w1937 {
              tunnel: [w2017 w2018] -> w1934
              tunnel: w1936 -> [w2017 _]
              tunnel: w1935 -> [_ w2018]
              frame 0, Default {
              }
              frame 1 {
              }
            }
            n802 = Unbundle By Name(w1924) -> ("Iteration"=w1923:i32)
            n803 = Unbundle By Name(w1924) -> ("End Temp"=w1925:dbl, "dt"=w1929:dbl, "Start Temp"=w1921:dbl)
            n804 = call "Set Profile.vi"("Profile Info"=w1924, "Error In"=w1933) -> ("Error Out"=w1932:errorcluster, "dT"=w1930:dbl)  [unwired: 6 in, 2 out]
            n805 = Subtract(x=w1934, y=w1931) -> (x-y=w1917:dbl)
            n806 = Add(x=w1931, y=w1930) -> (x+y=w1926:dbl)
            n807 = Greater?(x=w1918, y=w1917) -> (0:w1916:bool)
            n808 = Equal?(x=w1926, y=w1925) -> (x = y?=w1920:bool)
            n809 = case shown="True" w1916 {
              tunnel: [TRUE ("Start Profile Test") w1947] -> w1939
              tunnel: [w1940 w1956] -> w1938
              tunnel: w1932 -> [w1946 w1953]
              tunnel: w1929 -> [_ w1955]
              tunnel: w1926 -> [_ w1954]
              tunnel: w1927 -> [w1941 w1950]
              tunnel: w1923 -> [_ w1951]
              tunnel: [w1941 w1948] -> w1922
              tunnel: w1921 -> [_ w1949]
              tunnel: w1920 -> [_ w1952]
              frame False {
                n810 = call "Profile Timing FGV.vi"("Timer Mode"=T44."Read Time", "Error In"=w1946) -> ("Error Out"=w1943:errorcluster, "Elapsed Time (s.ms)"=w1944:dbl)  [unwired: 7 in, 1 out]
                n811 = property on="Profile Time" class="DigNum (strict)"(error in=w1943, "Value"=w1944) -> (error out=w1940:errorcluster)  [unwired: 1 in, 1 out]
              }
              frame True {
                n812 = case shown="False" w1952 {
                  tunnel: w1953 -> [w1962 w1985]
                  tunnel: [w1966 w1983] -> w1956
                  tunnel: w1954 -> [w1964 _]
                  tunnel: w1955 -> [w1965 w1984]
                  tunnel: w1951 -> [_ w1989]
                  tunnel: w1950 -> [w1957 w1987]
                  tunnel: w1949 -> [_ w1988]
                  tunnel: [w1957 w1986] -> w1948
                  tunnel: [TRUE ("Start Profile Test") w1982] -> w1947
                  frame False {
                    n813 = call "Profile Timing FGV.vi"("Timer Mode"=Timer_Mode."Read Time", "Error In"=w1962) -> ("Error Out"=w1961:errorcluster, "Elapsed Time (s.ms)"=w1959:dbl, "Has Time Elapsed"=w1960:bool)  [unwired: 7 in]
                    n814 = case shown="False" w1960 {
                      tunnel: w1961 -> [w1967 w1972]
                      tunnel: w1959 -> [w1968 _]
                      tunnel: [w1967 w1977] -> w1966
                      tunnel: w1964 -> [_ w1970]
                      tunnel: w1965 -> [_ w1969]
                      frame False {
                        "Profile Time" <- w1968
                      }
                      frame True {
                        n815 = call "Profile Timing FGV.vi"("Timer Mode"=T44."Start Timer", "Error In"=w1972, "Time Target (s)"=w1969) -> ("Error Out"=w1971:errorcluster)  [unwired: 6 in, 2 out]
                        n816 = Concatenate Strings("NS:Write>>" ("Command"), "M1 Set Temp" ("Command")) -> (w1974:string)
                        n817 = disable-structure shown="Disabled" {
                          disable-tunnel: [w1981 _] -> w1977
                          disable-tunnel: w1974 -> [w1980 _]
                          disable-tunnel: w1971 -> [w1979 _]
                          disable-tunnel: w1970 -> [w1978 _]
                          frame Disabled {
                            n818 = call "Messaging EnQ Single.vi"("Command"=w1980, "Data"=w1978, "error in (no error)"=w1979) -> ("error out"=w1981:errorcluster)  [unwired: 8 in]
                          }
                          frame Enabled {
                          }
                        }
                      }
                    }
                  }
                  frame True {
                    n819 = Greater Or Equal?(x=w1987, y=w1989) -> (x >= y?=w1990:bool)
                    n820 = case shown="True" w1990 {
                      tunnel: [w1997 w2013] -> w1983
                      tunnel: w1985 -> [w1994 w2012]
                      tunnel: w1984 -> [w1996 _]
                      tunnel: w1988 -> [w1995 _]
                      tunnel: w1987 -> [w1993 w2008]
                      tunnel: [w1992 w2008] -> w1986
                      tunnel: [TRUE ("Start Profile Test") FALSE ("Start Profile Test")] -> w1982
                      frame False {
                        n821 = call "Profile Timing FGV.vi"("Timer Mode"=T44."Start Timer", "Error In"=w1994, "Time Target (s)"=w1996) -> ("Error Out"=w2002:errorcluster)  [unwired: 6 in, 2 out]
                        n822 = Concatenate Strings("NS:Write>>" ("Command"), "M1 Set Temp" ("Command")) -> (w2001:string)
                        n823 = disable-structure shown="Disabled" {
                          disable-tunnel: w2002 -> [w2006 _]
                          disable-tunnel: w2001 -> [w2005 _]
                          disable-tunnel: [w2004 _] -> w1997
                          disable-tunnel: w1995 -> [w2003 _]
                          frame Disabled {
                            n824 = call "Messaging EnQ Single.vi"("Command"=w2005, "Data"=w2003, "error in (no error)"=w2006) -> ("error out"=w2004:errorcluster)  [unwired: 8 in]
                          }
                          frame Enabled {
                          }
                        }
                        n825 = Increment(x=w1993) -> (x+1=w1992:i32)
                      }
                      frame True {
                        n826 = Concatenate Strings("APP:Temp Profile>>" ("Command"), "Stop Profile" ("Command")) -> (w2009:string)
                        n827 = disable-structure shown="Disabled" {
                          disable-tunnel: [w2016 _] -> w2013
                          disable-tunnel: w2012 -> [w2015 _]
                          disable-tunnel: w2009 -> [w2014 _]
                          frame Disabled {
                            n828 = call "Messaging EnQ Single.vi"("Command"=w2014, "error in (no error)"=w2015) -> ("error out"=w2016:errorcluster)  [unwired: 9 in]
                          }
                          frame Enabled {
                          }
                        }
                      }
                    }
                  }
                }
              }
            }
          }
        }
        n829 = Bundle By Name(cluster=w1807, "Profile.Profile Temp"=w1813, "Profile.Current Cycle"=w1809) -> (w1814:T24)
      }
    }
    n830 = call "Save Log FGV.vi"("Log Path"=w191, "Case"=w194, "State"=w195, "Error In"=w197, "Descripition"=w193, "VI Name"=w192) -> ("Error Out"=w196:errorcluster)  [unwired: 5 in]
  }
  n831 = while {
    tunnel: w7 -> [w2020]
    tunnel: [w2019] -> w21
    stop <- w2021 stop-if-true
    # "Controller"
    n832 = event shown="[7] \"Pattern File\", \"Power Seq\", \"Seq Controls\", \"Iteration No\": Value Change" {
      selector: _ -> [_ _ _ _ _ _ _ _ _ _ _ _]
      dyn-events: _ -> [_ _ _ _ _ _ _ _ _ _ _ _]
      timeout: 100 -> [_ _ _ _ _ _ _ _ _ _ _ _]
      tunnel: [w2023 _ _ _ _ _ _ _ _ _ _ w2370] -> w2021
      tunnel: [w2025 w2033 w2051 w2058 w2069 w2224 w2245 w2287 w2318 w2340 w2365 w2375] -> w2019
      tunnel: w2020 -> [w2026 w2035 w2056 w2059 w2068 w2225 w2246 w2282 w2319 w2341 w2366 w2376]
      event Timeout {
        n833 = event-data() -> ()  [unwired: 1 in, 1 out]
        n834 = call "Messaging AE.vi"("Error In"=w2026) -> ("Error Out"=w2025:errorcluster, "queue out"=w2024:refnum<queue>)  [unwired: 9 in]
        n835 = Not A Number/Path/Refnum?(number/path/refnum=w2024) -> (NaN/Path/Refnum?=w2023:bool)
      }
      event "M1 Power Drive", "Power On-Off", "M1 Commands.M1 Feedback", "M1 Commands.M1 Package", "M1 Commands.M1 Enable", "M1 Commands.M1 Set Temp": Value Change {
        n836 = event-data() -> ("CtlRef"=w2037:refnum<vi>, "NewVal"=w2028:variant)  [unwired: 1 in]
        n837 = property class="Ctl"(reference=w2037) -> ("Caption.Text"=w2036:string)  [unwired: 1 in, 2 out]
        n838 = case shown="Default" w2036 {
          selector: w2036 -> [w2040 w2046]
          tunnel: [w2040 w2046] -> w2030
          tunnel: [w2038 w2047] -> w2029
          tunnel: w2028 -> [w2038 _]
          tunnel: w2035 -> [w2039 w2041]
          tunnel: [w2039 w2041] -> w2034
          frame Default {
          }
          frame "Power On-Off" {
            # "This is a Latch When release button. Is used to change the power state of the system. If system is on will turn off and if system is off will turn on."
            n839 = local read "Play/Pause"() -> (w2045:bool)
            n840 = case shown="False" w2045 {
              selector: w2045 -> [w2048 _]
              tunnel: "Are you sure you want to pause the system?" ("message") -> [_ w2050]
              tunnel: [w2048 w2049] -> w2043
              frame False {
              }
              frame True {
                n841 = Two Button Dialog(message=w2050) -> (T button?=w2049:bool)  [unwired: 2 in]
              }
            }
            n842 = Not(x=w2043) -> (.not. x?=w2042:bool)
            n843 = To Variant(anything=w2042) -> (Variant=w2047:variant)
          }
        }
        n844 = Concatenate Strings("NS:Write>>" ("Command"), w2030) -> (w2031:string)
        n845 = call "Messaging EnQ Single.vi"("Command"=w2031, "@Front?"=TRUE, "Data"=w2029, "error in (no error)"=w2034) -> ("error out"=w2033:errorcluster)  [unwired: 7 in]
      }
      event "Thermal Diode Feedback", "M1 Heater output", "M1 EEV Manual", "Cascade Compressor controls": Value Change {
        n846 = event-data() -> ("NewVal"=w2052:variant, "CtlRef"=w2057:refnum<vi>)  [unwired: 1 in]
        n847 = property class="Ctl"(reference=w2057) -> ("Label.Text"=w2054:string)  [unwired: 1 in, 2 out]
        n848 = Concatenate Strings("NS:Update Shared Variable>>" ("DNL_Message"), w2054) -> (w2053:string)
        n849 = call "Messaging EnQ Single.vi"("Command"=w2053, "Data"=w2052, "error in (no error)"=w2056) -> ("error out"=w2051:errorcluster)  [unwired: 8 in]
      }
      event "Checkbox", "Checkbox 2": Value Change {
        w2065 = FALSE ("element")
        n850 = event-data() -> ()  [unwired: 1 in, 1 out]
        n851 = Build Array("Checkbox", "Checkbox 2", w2065, w2065) -> (w2061:bool[])
        n852 = To Variant(anything=w2061) -> (Variant=w2060:variant)
        n853 = Concatenate Strings("NS:Update Shared Variable>>" ("DNL_Message"), "Manual Bypass Mode") -> (w2062:string)
        n854 = call "Messaging EnQ Single.vi"("Command"=w2062, "Data"=w2060, "error in (no error)"=w2059) -> ("error out"=w2058:errorcluster)  [unwired: 8 in]
      }
      event "Menu Ring", "IP Override": Value Change {
        n855 = event-data() -> ("NewVal"=w2075:variant, "CtlRef"=w2077:refnum<vi>)  [unwired: 1 in]
        n856 = property class="Ctl"(reference=w2077) -> ("Label.Text"=w2076:string)  [unwired: 1 in, 2 out]
        n857 = property on="Menu Ring" class="Ring (strict)"() -> ("Strings []"=w2071:string[])  [unwired: 2 in, 2 out]
        n858 = for {
          tunnel: "\\b[0-9]+\\.[0-9]+\\.[0-9]+\\.[0-9]+" ("regular expression") -> [w2080]
          tunnel: w2071 -> [w2079] mode=indexing
          tunnel: [w2078] -> w2070 mode=indexing
          n859 = xnode ("Match Regular Expression")("input string"=w2079, "regular expression"=w2080) -> ("whole match"=w2078:string)  [unwired: 4 in, 4 out]
        }
        n860 = case shown="\"Menu Ring\", Default" w2076 {
          tunnel: w2075 -> [_ w2214]
          tunnel: "Menu Ring" -> [w2199 _]
          tunnel: w2070 -> [w2198 _]
          tunnel: "Manual IP" -> [w2197 _]
          tunnel: [w2196 w2216] -> w2069
          tunnel: w2068 -> [w2195 w2215]
          frame "IP Override" {
            n861 = Empty String/Path?(string/path=w2197) -> (empty?=w2200:bool)
            n862 = case shown="False" w2200 {
              tunnel: w2199 -> [w2209 _]
              tunnel: w2197 -> [w2211 _]
              tunnel: w2198 -> [w2212 _]
              tunnel: [w2204 w2213] -> w2196
              tunnel: w2195 -> [w2203 w2213]
              frame False {
                n863 = Search 1D Array(1D array=w2212, element=w2211) -> (index of element=w2207:i32)  [unwired: 1 in]
                n864 = To Unsigned Word Integer(number=w2207) -> (unsigned 16bit integer=w2206:u16)
                n865 = Equal?(x=w2207, y=-1) -> (x = y?=w2210:bool)
                n866 = Select(t=w2209, s=w2210, f=w2206) -> (s? t:f=w2201:u16)
                n867 = To Variant(anything=w2201) -> (Variant=w2202:variant)
                n868 = property on="Menu Ring" class="Ring (strict)"("Value"=w2201) -> ()  [unwired: 2 in, 2 out]
                n869 = call "Messaging EnQ Single.vi"("Command"="MACRO:NS Update", "Data"=w2202, "error in (no error)"=w2203) -> ("error out"=w2204:errorcluster)  [unwired: 8 in]
              }
              frame True {
              }
            }
          }
          frame "Menu Ring", Default {
            n870 = call "Messaging EnQ Single.vi"("Command"="MACRO:NS Update", "Data"=w2214, "error in (no error)"=w2215) -> ("error out"=w2216:errorcluster)  [unwired: 8 in]
          }
        }
      }
      event "Config Data Setting", "Refresh Button", "Packages Setting", "Graph Temp Unit": Value Change {
        n871 = event-data() -> ("CtlRef"=w2223:refnum<vi>, "NewVal"=w2219:bool)  [unwired: 1 in]
        n872 = property class="Bool"(reference=w2223) -> ("Label.Text"=w2222:string)  [unwired: 1 in, 2 out]
        n873 = case shown="\"Config Data Setting\"" w2222 {
          selector: w2222 -> [_ _ w2237 w2240]
          tunnel: ["NS:Detect Systems" ("Command(s)") w2233 w2236 w2239] -> w2221
          tunnel: [TRUE ("@Front?") _ _ _] -> w2220
          tunnel: w2219 -> [_ w2229 _ _]
          tunnel: [_ w2228 _ _] -> w2218
          frame "Refresh Button", Default {
          }
          frame "Graph Temp Unit" {
            n874 = Concatenate Strings("UI:Update Pages>>" ("Command(s)"), "Reinitialize Graph" ("Command")) -> (w2233:string)
            n875 = Select(t="°C" ("Command"), s=w2229, f="°F" ("Command")) -> (s? t:f=w2232:string)
            n876 = To Variant(anything=w2232) -> (Variant=w2228:variant)
          }
          frame "Config Data Setting" {
            n877 = Concatenate Strings("APP:Update Config>>" ("Command(s)"), w2237) -> (w2236:string)
          }
          frame "Packages Setting" {
            n878 = Concatenate Strings("APP:Update Config>>" ("Command(s)"), w2240) -> (w2239:string)
          }
        }
        n879 = call "Messaging EnQ Single.vi"("Command"=w2221, "@Front?"=w2220, "Data"=w2218, "error in (no error)"=w2225) -> ("error out"=w2224:errorcluster)  [unwired: 7 in]
      }
      event "Login": Value Change {
        n880 = event-data() -> ("CtlRef"=w2244:refnum<vi>, "NewVal"=w2242:bool)  [unwired: 1 in]
        n881 = property class="Bool"(reference=w2244) -> ("Label.Text"=w2243:string)  [unwired: 1 in, 2 out]
        n882 = case shown="\"Login\"" w2243 {
          tunnel: w2242 -> [_ w2250]
          tunnel: w2246 -> [w2247 w2254]
          tunnel: [w2247 w2249] -> w2245
          frame Default {
          }
          frame "Login" {
            n883 = call "User Input Dialog.vi"("error in (no error)"=w2254, "Message title"="Enter the password", "Enable"=w2250) -> ("error out"=w2252:errorcluster, "OK?"=w2256:bool, "Message out"=w2253:string)  [unwired: 5 in]
            n884 = case shown="True" w2256 {
              tunnel: w2253 -> [_ w2263]
              tunnel: w2252 -> [w2257 w2260]
              tunnel: [w2257 w2262] -> w2249
              tunnel: "Password" ("y") -> [_ w2261]
              tunnel: i32[] [0, 1, 2, 3] ("Page array") -> [_ w2258]
              frame False {
              }
              frame True {
                n885 = Equal?(x=w2261, y=w2263) -> (x = y?=w2259:bool)
                n886 = case shown="True" w2259 {
                  selector: w2259 -> [_ w2267]
                  tunnel: [w2264 w2274] -> w2262
                  tunnel: w2260 -> [w2264 w2268]
                  tunnel: w2258 -> [_ w2266]
                  frame False {
                    n887 = One Button Dialog(message="Password is incorrect") -> ()  [unwired: 1 in, 1 out]
                  }
                  frame True {
                    n888 = Bundle("Page array"=w2266, w2267) -> (w2269:cluster{"Page array":i32[], bool})  [unwired: 1 in]
                    n889 = To Variant(anything=w2269) -> (Variant=w2273:variant)
                    n890 = Concatenate Strings("UI:Update Pages>>" ("Command"), "Enable Pages" ("Command")) -> (w2270:string)
                    n891 = call "Messaging EnQ Single.vi"("Command"=w2270, "Data"=w2273, "error in (no error)"=w2268) -> ("error out"=w2274:errorcluster)  [unwired: 8 in]
                  }
                }
              }
            }
          }
        }
      }
      event "Pattern File", "Seq Controls", "Iteration No": Value Change {
        n892 = event-data() -> ("CtlRef"=w2289:refnum<vi>, "NewVal"=w2283:variant)  [unwired: 1 in]
        n893 = property class="Ctl"(reference=w2289) -> ("Label.Text"=w2286:string)  [unwired: 1 in, 2 out]
        n894 = case shown="Default" w2286 {
          selector: w2286 -> [w2290 _ _ _]
          tunnel: [w2292 w2296 w2299 _] -> w2285
          tunnel: [w2291 w2295 w2300 w2305] -> w2284
          tunnel: w2283 -> [w2292 _ _ w2311]
          tunnel: w2282 -> [w2291 w2295 w2300 w2312]
          tunnel: [w2290 "Power Sequence" ("Command") "Power Sequence" ("Command") w2306] -> w2281
          tunnel: "Iteration No" -> [_ w2298 w2304 _]
          tunnel: "Power Seq" -> [_ w2294 w2303 _]
          frame Default {
          }
          frame "Power Seq" {
            n895 = Bundle("Iteration No"=w2298, "Power Seq"=w2294) -> (w2297:cluster{"Iteration No":i32, "Power Seq":T21})  [unwired: 1 in]
            n896 = To Variant(anything=w2297) -> (Variant=w2296:variant)
          }
          frame "Iteration No" {
            n897 = Bundle("Iteration No"=w2304, "Power Seq"=w2303) -> (w2302:cluster{"Iteration No":i32, "Power Seq":T21})  [unwired: 1 in]
            n898 = To Variant(anything=w2302) -> (Variant=w2299:variant)
          }
          frame "Seq Controls" {
            n899 = Variant To Data(error in=w2312, type=T22 {"Refresh Seq"=FALSE, "Save Seq"=FALSE, "Delete Seq"=FALSE, "Clear Seq"=FALSE} ("Seq Controls"), Variant=w2311) -> (data=w2309:T22, error out=w2305:errorcluster)
            n900 = Cluster To Array(cluster=w2309) -> (array=w2308:bool[])
            n901 = Search 1D Array(1D array=w2308, element=TRUE) -> (index of element=w2307:i32)  [unwired: 1 in]
            n902 = case shown="0, Default" w2307 {
              tunnel: ["Refresh Seq" ("Command") "Save Seq" ("Command") "Delete Seq" ("Command") "Clear Seq" ("Command")] -> w2306
              frame 0, Default {
              }
              frame 1 {
              }
              frame 2 {
              }
              frame 3 {
              }
            }
          }
        }
        n903 = Select(t="APP:Power Sequence(GUI)>>" ("Command"), s="Pattern Directory", f="APP:Power Sequence(RT)>>" ("Command")) -> (s? t:f=w2277:string)
        n904 = Concatenate Strings(w2277, w2281) -> (w2288:string)
        n905 = call "Messaging EnQ Single.vi"("Command"=w2288, "Data"=w2285, "error in (no error)"=w2284) -> ("error out"=w2287:errorcluster)  [unwired: 8 in]
      }
      event "Serial Port", "Custom Command", "Start Test", "Power", "Stop Test", "Reset Test": Value Change {
        n906 = event-data() -> ("CtlRef"=w2320:refnum<vi>, "NewVal"=w2321:variant)  [unwired: 1 in]
        n907 = property class="Ctl"(reference=w2320) -> ("Label.Text"=w2323:string)  [unwired: 1 in, 2 out]
        n908 = case shown="\"Serial Port\"" w2323 {
          selector: w2323 -> [w2328 _]
          tunnel: "APP:TTV Test>>" ("Command") -> [w2329 _]
          tunnel: w2321 -> [w2326 _]
          tunnel: w2319 -> [w2325 w2331]
          tunnel: [w2324 w2330] -> w2318
          frame Default {
            n909 = Concatenate Strings(w2329, w2328) -> (w2327:string)
            n910 = call "Messaging EnQ Single.vi"("Command"=w2327, "Data"=w2326, "error in (no error)"=w2325) -> ("error out"=w2324:errorcluster)  [unwired: 8 in]
          }
          frame "Serial Port" {
            n911 = constructor class="SerialPort"(error in=w2331) -> (reference out=w2332:refnum<k24>, error out=w2333:errorcluster)  [unwired: 2 in, 1 out]
            n912 = invoke on="牢焊农 畴靛" class="SerialPort" method="GetPortNames"(reference=w2332, error in=w2333) -> (error out=w2335:errorcluster, "GetPortNames"=w2334:string[])  [unwired: 1 in, 1 out]
            n913 = property on="Serial Port" class="CmbBox"(error in=w2335, "Strings[]"=w2334) -> (error out=w2330:errorcluster)  [unwired: 1 in, 1 out]
          }
        }
      }
      event "Start Profile", "Stop Profile", "Reset Profile", "Profile Info": Value Change {
        n914 = event-data() -> ("CtlRef"=w2339:refnum<vi>)  [unwired: 1 in]
        n915 = property class="Ctl"(reference=w2339) -> ("Label.Text"=w2338:string)  [unwired: 1 in, 2 out]
        n916 = case shown="\"Reset Profile\"" w2338 {
          selector: w2338 -> [_ _ w2361]
          tunnel: w2341 -> [w2346 w2356 w2360]
          tunnel: [w2344 w2351 w2358] -> w2340
          tunnel: "APP:Temp Profile>>" ("Command") -> [_ _ w2362]
          tunnel: "Profile Info" -> [w2343 w2349 w2357]
          frame "Reset Profile" {
            n917 = Unbundle By Name(w2343) -> ("dt"=w2342:dbl)
            n918 = property on="Profile Time" class="DigNum (strict)"(error in=w2346, "Value"=0.0 ("Time")) -> (error out=w2345:errorcluster)  [unwired: 1 in, 1 out]
            n919 = call "Timing FGV.vi"("Time Target (s)"=w2342, "Timer Mode"=T44."Start Timer", "Error In"=w2345) -> ("Error Out"=w2344:errorcluster)  [unwired: 6 in, 2 out]
          }
          frame "Profile Info" {
            n920 = call "Set Profile.vi"("Profile Info"=w2349, "Error In"=w2356) -> ("Error Out"=w2351:errorcluster, "Infinite?"=w2352:bool, "Waveform Graph"=w2350:waveform(dbl))  [unwired: 6 in, 1 out]
            "Temp Pattern" <- w2350
            n921 = Unbundle By Name(w2350) -> ()  [unwired: 2 out]
            n922 = Select(t="Infinite Cycle" ("Command"), s=w2352, f="") -> (s? t:f=→"Infinite Profile":string)
          }
          frame Default {
            n923 = Concatenate Strings(w2362, w2361) -> (w2359:string)
            n924 = call "Messaging EnQ Single.vi"("Command"=w2359, "Data"=w2357, "error in (no error)"=w2360) -> ("error out"=w2358:errorcluster)  [unwired: 8 in]
          }
        }
      }
      event "Channels": Value Change {
        n925 = event-data() -> ("CtlRef"=w2364:refnum<vi>, "NewVal"=w2363:T19)  [unwired: 1 in]
        n926 = property class="Arr (strict)"(reference=w2364) -> ("Label.Text"=w2368:string)  [unwired: 1 in, 2 out]
        n927 = Concatenate Strings("UI:Update Pages>>" ("Label.Text"), w2368) -> (w2367:string)
        n928 = call "Messaging EnQ Single.vi"("Command"=w2367, "Data"=w2363, "error in (no error)"=w2366) -> ("error out"=w2365:errorcluster)  [unwired: 8 in]
      }
      event Panel Close? {
        n929 = event-data() -> ()  [unwired: 1 in, 1 out]
        n930 = Two Button Dialog(message="Are you sure you want to Stop the Application?") -> (T button?=w2373:bool)  [unwired: 2 in]
        n931 = case shown="True" w2373 {
          tunnel: w2376 -> [w2377 w2381]
          tunnel: [w2377 w2380] -> w2375
          tunnel: [FALSE ("Discard?") TRUE ("Discard?")] -> w2370
          tunnel: "MACRO:Shutdown" ("Command") -> [_ w2379]
          frame False {
          }
          frame True {
            n932 = call "Messaging EnQ Single.vi"("Command"=w2379, "error in (no error)"=w2381) -> ("error out"=w2380:errorcluster)  [unwired: 9 in]
          }
        }
        n933 = event-data("Discard?"=FALSE) -> ()  [unwired: 1 in, 1 out]
      }
    }
  }
  n934 = Merge Errors(w21, w20, w5) -> (→"Error Out":errorcluster)
